vi "UHR-Fleezers Control (host) - 10.8MV_trial5.vi"() -> ()   [LabVIEW 2012]
uses:
  <vilib>/Utility/miscctls.llb/LVPoint32TypeDef.ctl
  <vilib>/Utility/miscctls.llb/LVMinMaxIncTypeDef.ctl
  <vilib>/userdefined/High Color/nirio_resource_hc.ctl
  <vilib>/Platform/TimedLoop/XDataNode/timing_clust.ctl
  <vilib>/Platform/TimedLoop/XDataNode/nitl_modes.ctl
  <vilib>/Platform/TimedLoop/XDataNode/wakeup.ctl
  <vilib>/FPGAPlugInAG/PCIe-7852R/niLvFpga_Open_PCIe-7852R.vi
  <vilib>/FPGAPlugInAG/PCIe-7852R/niLvFpga_Reset_PCIe-7852R.vi
  <vilib>/Utility/error.llb/Error Cluster From Error Code.vi
  <vilib>/rvi/errors/niLvFpgaAdjustHostInterfaceError.vi
  <vilib>/FPGAPlugInAG/PCIe-7852R/niLvFpga_Run_PCIe-7852R.vi
  <vilib>/Analysis/baseanly.llb/Mean (DBL).vi
  <vilib>/express/express analysis/Spectral/Block/exnSpectralBlock spectral measurements PSD poly.vi
  <vilib>/express/express analysis/Spectral/Block/exnSpectralBlock spectral measurements PSD WFM.vi
  <vilib>/Waveform/WDTOps.llb/WDT Append Waveforms DBL.vi
  <vilib>/FPGAPlugInAG/PCIe-7852R/niLvFpga_Abort_PCIe-7852R.vi
  <vilib>/FPGAPlugInAG/PCIe-7852R/niLvFpga_Close_PCIe-7852R.vi
  openfpgaref.8.6.ctl
  <vilib>/Platform/TimedLoop/XDataNode/XDataNode.xnode
  <vilib>/rvi/interface/nirviOpenFPGA/nirviOpenFPGA.xnode
  FPGA Bitfiles/UHR-FleezersInst_FPGATarget_UHR-FleezersCont_0F5B06C4.lvbitx
  UHR-Fleezers Control (fpga) - 10.3.vi
  <vilib>/rvi/interface/nirviMethod/nirviMethod.xnode
  <vilib>/rvi/interface/nirviReadWriteControl/nirviReadWriteControl.xnode
  <vilib>/express/express analysis/Spectral/XNode/ExpressSpectralMeasurementsBlockNode.xnode
  <vilib>/rvi/interface/nirviCloseFPGA/nirviCloseFPGA.xnode
  <vilib>/Analysis/NI_AALBase.lvlib
  <vilib>/Platform/TimedLoop/XDataNode/XDNodeRunTimeDep.lvlib
  <vilib>/vision/NI_Vision_Development_Module.lvlib
  NiFpgaLv.dll
  <vilib>/FPGAPlugInAG/PCIe-7852R/niLvFpga_ConfigureFifo_PCIe-7852R.vi
  <vilib>/rvi/errors/niLvFpgaMergeErrorWithErrorCode.vi
  <vilib>/FPGAPlugInAG/PCIe-7852R/niLvFpga_ReadFifo_PCIe-7852R.vi
panel:
  out "Location path":path=path "D:/UnifiedHighRes_VIs/Locations.txt"
  out "Location Matrix":string[][](array[string])=[["N.D.\r\n", "N.D.\r\n", "N.D.\r\n"], ["0.19233\r\n", "0.00156\r\n", "0.20615\r\n"], ["N.D.\r\n", "N.D.\r\n", "N.D.\r\n"], ["N.D.\r\n", "N.D.\r\n", "N.D.\r\n"]]
  in  "radius":i32=10 min=1 max=20
  in  "clear markers":bool
  in  "trap\nmarkers?":bool
  in  "Sample Channel Flow":bool
  in  "Pump 3 contents":string="Bottom: ADig beads" caption="contents"
  in  "Pump 1 contents":string="Top: DNA beads" caption="contents"
  in  "Scripts":T1(tab)
  in  "Take Stepping Data":bool
  in  "Got DNA bead":bool
  in  "Got ADig bead":bool
  in  "Cap 1 Flow ON":bool=TRUE
  in  "Move Cap. 1 (DNA Top)":bool
  in  "Cal/Data Acq. Spot":bool
  in  "Dump Beads":bool
  in  "Cap 1 T ON":bool=TRUE
  in  "Cap 1 Samp Flow ON":bool=TRUE
  in  "Offset 2 Set":dbl=2.0
  in  "Offset 1 Set":dbl=1.0
  in  "Cal @ (MHz)":dbl=20.0
  in  "W/ Offset 1":bool=TRUE
  in  "Offset 1 Start (MHz)":dbl=13.0
  in  "W/ Offset 2":bool
  in  "Offset 2 Start (MHz)":dbl=16.0
  in  "Pause at Closest Delta (s)":dbl
  in  "Move to Delta 2 (MHz)":dbl=41.0
  in  "Attempt Limit":dbl=30.0 caption="Limit"
  out "Attempts":dbl=1.0
  in  "Wait Before Save (s)":u32=1
  in  "Fish for Tether":bool
  in  "Closest Delta (MHz)":dbl=13.0 step=0.25
  in  "Stop F (pN)":dbl=10.0
  in  "Then...":string(combo)="2"
  in  "Move to Delta 1 (MHz)":dbl=15.0
  in  "Tether Alarm?":bool=TRUE
  out "Tether":bool
  in  "TA Cancel Save?":bool=TRUE
  in  "TA Green Off?":bool=TRUE
  in  "Raster Set Upon Tether":u32=1
  in  "Save at end (5, 6)":bool
  in  "N Steps":dbl=20.0
  in  "Step Size (nm)":dbl=0.34
  in  "Save ave factor":dbl=1.0
  in  "Dip Trap Delta 1 (MHz)":dbl=15.0
  in  "Move Trap Before?":bool
  in  "Save Data After?":bool
  in  "Green ON After?":bool
  in  "Dip Trap Delta 2 (MHz)":dbl=15.0
  in  "Move Trap After?":bool
  in  "Duration (s)":dbl=1.0
  in  "Dip for Protein":bool
  in  "APD to Watch":bool
  out "Duration (s)":dbl
  in  "Action":string(combo)="Yank"
  in  "Fl. Triggered...":bool
  in  "Fl. Delta Thresh. (kHz)":dbl=0.6
  out "Waiting":bool
  out "Fl. High":bool
  in  "N pts to average":u16=6
  in  "Yank Delay (s)":dbl=3.5
  in  "Yank to Delta Array (MHz)":dbl[](array[numeric])=[16.3, 15.85, 14.85]
  in  "N Array El":u8=3 min=1 step=1
  in  "Random Choice":bool=TRUE
  in  "Force Yank":bool
  in  "Force Reset":bool
  in  "Y change (mm)":dbl
  in  "Profile":bool
  out "Sigma/Mean 2":dbl=nan caption="Sigma/Mean" format="%#_2g"
  out "Rate sigma (Hz) 2":dbl caption="Sigma (Hz)" format="%0.2f"
  out "APD 2 Rate (Hz)":dbl format="%#_3p"
  out "Primary Video Display":T2(plugin-control)
  out "Waveform Graph":dbl[](graph) caption="APD Line Scan"
  in  "Inject Top":bool caption="Inject Pump 3"
  in  "Inject Bottom":bool caption="Inject Pump 1"
  out "Messages":string="7:59 AM\tUHR-Fleezers ready.\r"
  in  "APD Ave N":dbl=10.0
  out "Int. Time (s)":dbl=3.0
  in  "Stop All":bool=TRUE
  out "Sigma/Mean":dbl=nan format="%#_2g"
  out "Rate sigma (Hz)":dbl caption="Sigma (Hz)" format="%0.2f"
  in  "Tab Control 6":T3(tab)
  in  "APD 2 Offset":dbl
  in  "APD 1 Offset":dbl
  out "RMS (Ang)":dbl=nan format="%_2g"
  in  "Bead Sep. Int. Time (s)":dbl=5.0 caption="Int. Time (s)"
  in  "Below (kHz)":dbl=0.5
  in  "Above (kHz)":dbl=2.0
  in  "Adjust Scale\nto Mean":bool
  in  "Rescale on Mean":bool
  in  "Offset (nm)":dbl
  out "Mean":dbl=nan caption="Mean (V)" format="%#_3g"
  out "Force":waveform(dbl)[](graph)=[{"t0"=timestamp(12.90000000000001 s since 1904-01-01), "dt"=0.15, "Y"=[nan, nan], "attributes"=variant("NI_ChannelName"=variant(string "T1 X"))}, {"t0"=timestamp(12.90000000000001 s since 1904-01-01), "dt"=0.15, "Y"=[nan, nan], "attributes"=variant("NI_ChannelName"=variant(string "T2 X"))}]
  out "APD Chart":waveform(dbl)[](graph)=[{"t0"=timestamp(12.90000000000001 s since 1904-01-01), "dt"=0.02, "Y"=[0.0, 0.0, 0.0, 0.0, 0.0, 0.0, 0.0, 0.0, 0.0, 0.0, 0.0, 0.0, 0.0, 0.0, 0.0], "attributes"=variant("NI_ChannelName"=variant(string "APD 1"))}, {"t0"=timestamp(12.90000000000001 s since 1904-01-01), "dt"=0.02, "Y"=[0.0, 0.0, 0.0, 0.0, 0.0, 0.0, 0.0, 0.0, 0.0, 0.0, 0.0, 0.0, 0.0, 0.0, 0.0], "attributes"=variant("NI_ChannelName"=variant(string "APD 2"))}]
  in  "Calibration":u16(ring) items=["None", "Position", "Force"]
  out "T1 X":dbl=nan caption="T1 X (V)" format="%0.2f"
  out "T2 X":dbl=nan caption="T2 X (V)" format="%0.2f"
  out "Bead Separation":waveform(dbl)(graph)={"t0"=timestamp(12.90000000000001 s since 1904-01-01), "dt"=0.15, "Y"=[nan, nan], "attributes"=variant("NI_ChannelName"=variant(string "T1 X"))}
  in  "Amplitude (nm)":dbl=3.0
  out "Bead Mean (nm)":dbl=nan caption="Mean (nm)" format="%0.2f"
  out "Difference":dbl=nan caption="Difference (V)" format="%.2g"
  in  "Take Detection Laser\nImage":bool
  out "APD 2":T2(plugin-control) caption="APD 2 (Cy5)"
  in  "Flip Green Filter":bool
  in  "Set X Only":bool
  in  "Set Y Only":bool
  out "APD 1":T2(plugin-control) caption="APD 1 (Cy3)"
  out "Detection Laser Y":T2(plugin-control)
  out "Pointer Y (V)":dbl format="%_3g"
  out "Pointer X (V)":dbl format="%_3g"
  in  "Set Confocal Spot (X-Y)":bool
  out "Detection Laser X":T2(plugin-control)
  out "Saved APD":dbl[][](graph) caption="Most Recent Time Trace"
  out "Trap Delta Graph":dbl[](graph) caption="Most Recent Time Trace"
  out "Save APD Deriv":dbl[][](graph) caption="Most Recent Time Trace"
  out "Delta Fl. 1":dbl
  out "Delta Fl. 2":dbl
  out "All Signals":waveform(dbl)[](graph)=[{"t0"=timestamp(12.90000000000001 s since 1904-01-01), "dt"=0.02, "Y"=[0.0, 0.0, 0.0, 0.0, 0.0, 0.0, 0.0, 0.0, 0.0, 0.0, 0.0, 0.0, 0.0, 0.0, 0.0], "attributes"=variant("NI_ChannelName"=variant(string "APD 1"))}, {"t0"=timestamp(12.90000000000001 s since 1904-01-01), "dt"=0.02, "Y"=[0.0, 0.0, 0.0, 0.0, 0.0, 0.0, 0.0, 0.0, 0.0, 0.0, 0.0, 0.0, 0.0, 0.0, 0.0], "attributes"=variant("NI_ChannelName"=variant(string "APD 2"))}, {"t0"=timestamp(12.90000000000001 s since 1904-01-01), "dt"=0.15, "Y"=[nan, nan], "attributes"=variant("NI_ChannelName"=variant(string "T1 Y"))}, {"t0"=timestamp(12.90000000000001 s since 1904-01-01), "dt"=0.15, "Y"=[nan, nan], "attributes"=variant("NI_ChannelName"=variant(string "T1 X"))}, {"t0"=timestamp(12.90000000000001 s since 1904-01-01), "dt"=0.15, "Y"=[-0.0004235663930173644, -0.0004722739341410556], "attributes"=variant("NI_ChannelName"=variant(string "T1 Sum"))}, {"t0"=timestamp(12.90000000000001 s since 1904-01-01), "dt"=0.15, "Y"=[nan, nan], "attributes"=variant("NI_ChannelName"=variant(string "T2 Y"))}, {"t0"=timestamp(12.90000000000001 s since 1904-01-01), "dt"=0.15, "Y"=[nan, nan], "attributes"=variant("NI_ChannelName"=variant(string "T2 X"))}, {"t0"=timestamp(12.90000000000001 s since 1904-01-01), "dt"=0.15, "Y"=[-0.0005883053071687949, -0.0006281319620349712], "attributes"=variant("NI_ChannelName"=variant(string "T2 Sum"))}, {"t0"=timestamp(12.90000000000001 s since 1904-01-01), "dt"=0.15, "Y"=[nan, nan], "attributes"=variant("NI_ChannelName"=variant(string "T1 FB X"))}, {"t0"=timestamp(12.90000000000001 s since 1904-01-01), "dt"=0.15, "Y"=[-0.0004680013428144157, -0.0005167699209570592], "attributes"=variant("NI_ChannelName"=variant(string "T2 FB Sum"))}, {"t0"=timestamp(12.90000000000001 s since 1904-01-01), "dt"=0.15, "Y"=[nan, nan], "attributes"=variant("NI_ChannelName"=variant(string "T2 FB X"))}, {"t0"=timestamp(12.90000000000001 s since 1904-01-01), "dt"=0.15, "Y"=[-0.0006226691488387671, -0.0006504715109714008], "attributes"=variant("NI_ChannelName"=variant(string "T2 FB Sum"))}, {"t0"=timestamp(12.90000000000001 s since 1904-01-01), "dt"=0.15, "Y"=[-0.0007901852473525123, -0.0008601641895809732], "attributes"=variant("NI_ChannelName"=variant(string "PSD Y"))}, {"t0"=timestamp(12.90000000000001 s since 1904-01-01), "dt"=0.15, "Y"=[0.00031556138798181086, 0.0002525101474044007], "attributes"=variant("NI_ChannelName"=variant(string "PSD X"))}, {"t0"=timestamp(12.90000000000001 s since 1904-01-01), "dt"=0.15, "Y"=[-0.00019678334910122974, -0.0002453993346964931], "attributes"=variant("NI_ChannelName"=variant(string "PSD Sum"))}]
  in  "Signals to Plot":i32(listbox)
  out "Trap Disp. Freq. (Hz)":dbl=6.666666666666667 caption="Freq. (Hz)" format="%#_6p"
  out "Display Period (s)":dbl=0.15 caption="Period (s)" format="%#_6p"
  in  "Trap Disp. Downsample":dbl=10000.0 caption="Downsample" max=20000.0
  in  "APD Disp. Scale":dbl=0.1 caption="Scale (Divide,\nfor above plot only)"
  in  "APD Disp. Downsample":dbl=2.0 caption="Integrate" min=1.0 max=30.0 step=1.0
  out "APD Display Freq. (Hz)":dbl=50.0 caption="Freq. (Hz)"
  out "APD Display Period (s)":dbl=0.02 caption="Period (s)"
  out "FFT 1":cluster{"f0":dbl, "df":dbl, "magnitude":dbl[]}[](graph)=[{"f0"=0.0, "df"=16.666666666666668, "magnitude"=[-331.1367572010275, -79.05506245821404, -86.61411242440559, -88.4728176091699, -90.3181253945935, -94.12566333707997, -92.52740723119955, -94.92192587982518, -99.60936585245742, -96.87568627870715, -94.02570383337763, -83.8058550151726, -97.57441397235512, -101.59968530846606, -101.523049255742, -103.35038532190343, -101.58594091014982, -102.96098031851216, -91.39759462745924, -103.75019963279499, -104.45030075054324, -103.04245334279298, -104.0720279134107, -106.06482372394834, -103.69131867828104, -104.40395035115309, -105.96420043276396, -107.6735556337804, -106.673030006608, -107.34889066208132, -108.05626565233933, -106.25659018850432, -105.29934513380842, -105.43096056709592, -108.3728498841465, -106.0555440144992, -105.78001282181421, -107.48741857324953, -108.67624970548897, -105.39976667156175, -105.91413119232612, -109.4222808198164, -107.0898971593174, -107.91164191890915, -108.26032038855709, -107.58332347164534, -108.23559688234297, -108.01271040303237, -107.66511723652701, -106.51901583170391, -109.27249501469946, -108.55647681594805, -107.93499259231463, -107.05068166453935, -109.13641475410455, -109.29679733781423, -108.19360835527803, -109.57747591546632, -109.58364591011674, -110.47061433372711, -109.8144340420426, -108.79067462293897, -107.54887553357234, -107.99559866705923, -108.85023923652685, -109.68733225238618, -108.51101278437793, -108.51620475114115, -108.22212402200637, -104.63726950302143, -110.2989919678048, -107.61796444414897, -108.68882962798736, -104.79193983043893, -103.59504263746938, -93.64633660288543, -101.9191640501395, -105.73717393151816, -108.92572458793902, -107.43962662800902, -107.79595323081325, -107.0923101993207, -108.17603277205289, -107.87074270713183, -109.20899066381877, -108.61832060412445, -109.10072003106593, -105.76480632823524, -108.60877649218978, -109.67541158970121, -110.2286232768028, -109.84952155309578, -109.33772024076384, -109.95251642394683, -110.14777282585466, -109.13825677905699, -110.05989365698167, -109.39359990189426, -110.56255614635295, -109.66477183197163, -108.9397158528824, -110.26529907650465, -109.20049464984628, -108.20183857013548, -109.09752250184418, -108.00440442238454, -108.35465963524055, -111.16774134451799, -110.34812550238405, -108.94506763426756, -108.72845542102493, -109.41512344014713, -112.44661664432377, -110.35437330889101, -111.32939440655925, -109.42989530434981, -110.98084669076195, -111.92160561143541, -108.57755551751093, -111.40042616180912, -110.15284955891853, -112.21455132279115, -111.40787773511747, -108.82949641635288, -110.13442122547907, -111.42229298204664, -112.06314940885191, -110.6015308813694, -109.51144097251623, -111.15989713761475, -110.25535755335385, -109.65868178057926, -110.51649885452997, -109.77194745285269, -108.4234206864394, -109.50892632093968, -109.46471287444389, -107.92241289271415, -109.72283805386196, -108.63426821579918, -110.37316681536255, -111.09713996884652, -110.32903619589223, -105.32012665515045, -107.36858557554393, -108.00382215905725, -110.06430686942338, -108.81666625979916, -110.01277074453823, -110.94194741225512, -109.65934609082873, -107.80979136006962, -112.81333866824724, -111.61474300955487, -109.83998277184975, -109.45953946904639, -109.79640584952526, -108.19172301667324, -109.28894656674316, -107.61471301278785, -108.83814006090513, -109.08866847726084, -108.20250571862371, -107.96222236861584, -107.03811197900873, -108.93533000393974, -107.74482548035408, -110.79811544577694, -111.1387476496877, -107.42970105883512, -109.18442281176472, -108.73546184641192, -108.71800246690864, -108.51945944378063, -108.06825856571285, -107.27210712368412, -108.12304695877637, -107.84933283677306, -109.73682373154998, -109.32284761503395, -109.31328817453769, -106.68762108642842, -109.79203616876461, -109.9020278896408, -110.27080024357275, -108.54152101558762, -111.00464391726017, -112.42244020766577, -110.82707315747889, -111.00344011890857, -109.90461839395674, -109.42877207451863, -109.73549298167016, -111.67494793393293, -108.85799077901427, -108.5348443278263, -109.803781083881, -108.30644755543659, -108.5079527456017, -111.2055351312823, -108.53089994340155, -108.01739789012176, -108.70360662855235, -107.95873456794631, -109.58297170693093, -108.9372401694271, -110.15921663527153, -109.22399119911955, -110.89883651739237, -108.92840112258382, -110.0545300523626, -109.05961065387005, -109.45831398589371, -108.61239387653227, -110.13001256174265, -108.80060224137931, -109.46327400696283, -108.0177965824709, -109.29727944627197, -110.3237255895986, -109.03258262543821, -110.97880178489321, -109.70034895077919, -111.16405638194153, -109.17324451464711, -109.65698250854277, -108.96750235822178, -112.00534231585624, -108.69274607723942, -108.98110446396657, -108.40723795464795, -111.44459094807324, -111.74799245277113, -111.1601960491512, -108.92048232753773, -110.30506377784799, -111.33145973979093, -110.91850998672503, -110.33684985776448, -108.90206518366908, -109.28458878227542, -108.98773986023751, -110.85813863075646, -109.00041591105906, -110.84543686681204, -109.84382395806176, -109.69722434763266, -108.50915601095721, -107.80829925826895, -110.59736107582401, -109.75377770317087, -109.3992084496136, -110.51151565846742, -112.49753959826434, -109.7299632589479, -109.54070743868353, -109.90314341132164, -111.05974202976806, -109.03766862152392, -109.46667095459878, -109.52800799036197, -111.3163121356807, -110.07817134522178, -108.69251657453547, -109.40472158898045, -109.71400709815576, -110.60534468715097, -109.46937396724682, -107.70342491418788, -109.86331122597839, -108.64971387994616, -110.90117371097081, -108.34928840565928, -110.04172889660904, -111.52979926554961, -110.34759300823305, -109.62712781837159, -109.24131154553284, -110.23196152450447, -108.68509612326807, -108.0246905483419, -106.61876139289784, -101.5519630114271, -80.57695480953835, -102.03744443354402, -107.1449217193017, -110.0695213407169, -106.61597783999268, -110.79221011808191, -109.58974545931426, -109.1149802216988, -109.20993813088597, -109.63768480465863, -110.10428394219181, -109.08445084271477, -108.83472375362581, -109.69508502050168, -108.05588796178941, -110.62586360101581, -109.95315261676905, -107.52208264977473, -108.80708007514875, -110.43484881098874, -110.45942171588936, -107.83804717866751, -109.98973910294193, -109.3496496054193, -108.425252911127, -110.94579264380809, -108.54181722177951, -108.67696070083541, -108.4150202151644, -109.24973583101504, -112.0454922608961, -111.29046597340738, -110.75018248960077, -109.38326363603683, -109.2033340336957, -109.45076170874889, -109.52878049853727, -109.32340869724774, -110.98123395128233, -110.75736340635505, -109.7218385823809, -107.97422606064993, -109.77313701758703, -110.95948744392717, -110.08996774172691, -108.51011830110778, -109.78063140243836, -110.65996628628228, -109.83684298615616, -110.33329049188029, -110.13755118968292, -110.3717925645783, -108.55302219178951, -106.86811628734195, -108.6302156589162, -108.75341391045045, -108.32589578384841, -108.70061474734084, -112.30742263527534, -109.16842570592085, -109.29767035534508, -108.87829025017463, -108.2255616391397, -108.4316108616088, -108.82995906929271, -110.40135575415563, -109.51623498946435, -109.79409808792403, -107.03832759632121, -108.36534528684132, -109.72010868372905, -107.90933028179892, -106.95643597294047, -111.29929166165778, -110.23001135794706, -108.98838015381585, -109.79115357104436, -108.18627479511115, -108.14988122174307, -109.12074063466532, -109.41904850488358, -111.40409873721113, -108.83156790193294, -108.77032248953847, -108.88363158686694, -108.47515048290681, -105.94172147874599, -109.38146940214403, -109.21277078848794, -108.11309390545507, -110.70840012427504, -109.5504457849329, -109.52330684534209, -110.06776026911132, -108.21949434182314, -111.21266686269992, -108.78581501170974, -108.43115799297222, -109.63260325780062, -109.84070220619535, -109.72041980780126, -110.29615941882527, -110.60316734262464, -108.79165446414692, -110.95840439895592, -109.64926233107009, -109.16526769544322, -108.65292362430982, -109.56113898129935, -109.85693046339026, -108.92316027325207, -109.79492493553914, -109.38157962945887, -110.24545136266825, -109.30031463492487, -109.0795429936869, -111.4091719525013, -108.63499083917162, -108.43863465339358, -109.23207864880891, -111.21947487191643, -109.24525201480154, -109.56842406077318, -109.46711940800672, -111.91389548262572, -108.15655736690546, -108.71882059966947, -111.26328503478568, -110.95027143873176, -108.4853106242357, -110.36902802777546, -109.9314203579182, -108.77686164101732, -108.71871020068312, -111.04829661168574, -109.95072655339462, -109.88221342875462, -109.53241732756136, -108.2625005404823, -108.00677030040697, -110.19659317581693, -108.93858924796267, -109.46817875483995, -110.78063992017232, -111.11066570318451, -110.78774336696706, -109.19199744617812, -108.54914256407436, -109.28414960420909, -110.64143585101183, -110.5855350821307, -109.47578632252726, -108.89705360836223, -109.89214013612292, -107.93271261027171, -109.32631601340563, -108.60274611341092, -109.40110159872573, -110.889237682208, -110.01391165813328, -109.99747108785071, -108.65542819213674, -110.37211847668736, -110.44656500845738, -110.8128133834973, -108.8909299260433, -110.19551227077532, -111.37647266643523, -110.83802189730321, -109.98519377913681, -110.52378970770522, -108.16970420057817, -110.70974729773344, -110.76836765494402, -110.26884275594577, -109.22041044268806, -109.87809744746195, -107.76823252107832, -109.12119474042969, -110.28066108731146, -108.55000033509207, -110.18152097767907, -110.73030521152278, -111.49470908029893, -110.2320929919509, -110.03370979233021, -109.79181668155233, -108.6673501209991, -109.86695766650877, -107.88926518046961, -110.95525003776572, -109.18130359755742, -110.42618009658618, -107.90341931158893, -111.44736855661769, -110.72634267386593, -109.29945988519303, -107.67889101961411, -108.81148059987765, -109.13375212757057, -109.8122873383549, -109.80176697684155, -109.96342275204768, -109.90406635707086, -108.75674342748256, -110.12362902701081, -109.82151095527837, -108.62543344241836, -110.09171852771195, -110.21434637862887, -109.97254504855631, -109.27043209093468, -111.35149588204125, -110.12399876776051, -111.65983675538546, -109.28788875768564, -110.86554069990251, -111.26990906470603, -108.60956517491746, -111.49613890850938, -111.79685722966795, -109.26269485364045, -110.38555615546439, -109.40641023162068, -110.966136593156, -108.78892524584494, -110.29340727375603, -111.44032043281035, -109.95212021173755, -109.79233511584334, -112.41184021118175, -109.73687851881148, -108.65493879781806, -110.76132988919045, -108.43230346094671, -110.32968175895853, -110.29890782023821, -108.77609076424456, -110.3298662333555, -109.47734504217333, -108.2677295732245, -109.21234363352882, -107.83278941978479, -108.85136784424789, -108.43241251530755, -109.76609391460555, -108.53204373005357, -110.9660641972934, -110.3152512161094, -110.72570499399905, -109.23877906286317, -111.72407743101837, -109.20311421918561, -108.06021800233717, -109.29288625761943, -108.78395253409145, -111.85250172876302, -108.78827588901797, -109.79775055719482, -109.12089297455859, -109.49896359356035, -110.34432647103819, -107.94700097960238, -109.30489238477631, -108.89170290869342, -108.82574563272509, -110.11024077194833, -107.37946433552314, -109.60167933458756, -107.80625057819019, -110.11489057210264, -107.35436859378505, -105.69819484613895, -109.11280625683739, -109.27770293057978, -107.7053735252589, -109.75022444894368, -109.3310543596577, -107.87683693707739, -108.19931495338068, -109.26462246191564, -106.71885779297867, -100.00018022217961, -92.54434511397295, -107.20472143807373, -107.39203415155283, -110.04461177268398, -108.48860496315312, -109.0057168110333, -108.37627790492552, -108.4108380728248, -109.65509454313073, -109.64243000632982, -97.04219069306761, -109.0928856629964, -107.9760697315632, -107.52611064047497, -108.87702814778996, -109.08437599027614, -110.70097118837974, -109.00969860961283, -110.38275386163214, -110.0699155421545, -106.91498895181175, -106.22178738309017, -109.36827866896039, -107.59953130968307, -109.19516217272808, -108.31502495393616, -109.384158926223, -107.11670654202719, -108.09436312738853, -110.14559230873704, -109.84997663447679, -107.83465335309926, -108.60947100624459, -108.9932479423645, -109.17174810371898, -108.79457339828916, -109.40909327982367, -109.6328723628302, -109.51081854476179, -107.63054408568418, -109.63728404010122, -108.51163794839918, -107.55002282725216, -108.97796212764939, -107.24648164623483, -112.21470452291085, -108.74294024554423, -109.62070777514892, -108.05768666239368, -109.8224946685739, -109.34575507446003, -108.53536952609525, -109.60789300457671, -107.56681538208278, -109.22777325016398, -108.79047910308894, -110.10332477250668, -108.00206387955672, -108.45604004720035, -109.00645795765472, -109.81039564269616, -108.92785144634745, -108.3978471520567, -107.94411095685999, -110.53486519304262, -108.8773780319227, -109.03345093296107, -107.30746693745031, -108.54277704832029, -108.77629108166091, -108.91111762599647, -107.74965195880401, -109.97375370738439, -109.76326492689246, -107.91717581777407, -109.0730556927617, -107.66804873204664, -110.40438871064791, -108.05794247751498, -108.80206615156494, -107.51329354700796, -108.83687012994949, -107.57713176895379, -107.94774159581414, -109.41894615439651, -107.10869425078764, -110.51480854078629, -108.92221367099775, -109.91358786461535, -110.1744263092835, -109.30795472883494, -107.91359710691006, -109.77888185049835, -109.52060975706438, -108.66686651982212, -108.71041801553639, -110.13619546359467, -108.87957097273856, -109.72150387215271, -109.00776068810654, -109.70251113927438, -110.75769213896399, -108.53234896741436, -109.69439526582246, -110.15412541604617, -108.25183374628219, -107.97402569656481, -110.34920156998648, -108.45106995186384, -108.82031145748209, -111.38690005057539, -107.01968459818563, -110.3044500039584, -110.8755481852125, -111.08915057663255, -107.94824988655199, -110.21669144934839, -109.90539774633154, -109.58985438756767, -110.12258796623348, -109.41689951612143, -109.31128210476795, -109.00258476567323, -109.11093063041056, -108.83347064311234, -108.32685287566952, -109.44770946560935, -108.40145063144861, -109.68448193892085, -108.76525439243828, -107.62837139034596, -107.39300298848994, -109.36993934990318, -109.2465218489418, -106.66307369796812, -110.15891092764934, -109.57151745419041, -108.92425698310808, -109.8036704717834, -108.79751146756549, -109.25926431818017, -108.46260574057584, -109.1967554647261, -110.63319560262356, -109.02343067385144, -111.22073171487528, -109.4731095097105, -109.69335000085164, -109.48782989577005, -107.95204227683271, -108.19468255763758, -111.36195112053247, -109.55696116543685, -110.3130767640534, -108.9621824253354, -109.99735074896789, -109.20198058456344, -108.12100614259485, -111.27227490807289, -110.09248554008288, -109.14395535060149, -110.80882692379708, -109.22632926901655, -108.64497210802793, -111.00030482190711, -111.1317849358033, -107.43140429257826, -107.9783302193555, -109.2639893652291, -108.97008485446163, -108.66556668859064, -108.12995785876932, -109.73001061107855, -108.09691302413727, -110.68391499215569, -112.78583642012705, -108.7093037763389, -110.67868795924797, -109.0190959349128, -108.36247198231372, -109.82829353258869, -108.24916379311045, -109.84154533905823, -108.55470160833775, -109.75438989348815, -108.82865632118325, -107.63622268162582, -111.00943492886312, -110.81824358463759, -109.46028423652966, -107.52479398900992, -108.99087806823736, -109.94494831750349, -110.26788355564504, -109.8954055022304, -106.9478122391182, -108.91705388158901, -107.76095584490312, -109.28456723055147, -109.7982307261767, -108.98552661346622, -109.98937979783426, -110.57907422426224, -108.68113463944836, -108.06257240208589, -110.0707224529617, -109.19515280354733, -109.35868842818849, -110.37311467065695, -109.0404734478992, -108.16686395270187, -108.61859220485148, -109.19986437876149, -108.19707189725302, -110.06564239663074, -108.87850403465154, -110.63824157544798, -107.36918104067212, -108.7008736325543, -110.9359398265406, -111.08529123080929, -108.44209934821818, -109.79529621208783, -108.38917887958179, -108.169117639508, -109.24332926356216, -110.50584058811704, -109.63592524002665, -109.32261039377495, -109.16720880524552, -109.3084314664462, -109.5812223978583, -107.70213196487856, -108.0557884982431, -110.67058020007828, -111.68459781023608, -109.66270627185824, -110.52536245663693, -109.70208409132103, -108.78645420809342, -109.23122088059863, -109.24601474121832, -111.25604763816514, -109.50225851581177, -107.32434217163818, -109.28548556764925, -107.59972621660836, -110.46928774723048, -109.25950101547609, -110.32016453935465, -107.78482761561703, -107.89462895091089, -107.51366154391481, -108.08036891159172, -109.53371809947035, -101.2452927166745, -109.32763325689056, -107.52166868423687, -109.89648659445174, -109.11350200980485, -109.81336712738089, -110.02799517445062, -108.02767143538516, -107.97850220501483, -109.50772934896838, -109.31069875721964, -108.49991657749598, -105.60880911233095, -109.79128597340213, -106.91084537903113, -107.84880087118997, -109.63628170511824, -109.03203967193224, -110.64186113413658, -110.98027990365594, -112.33841002907062, -111.01793075565425, -108.58025797022215, -110.4259296883756, -110.38643255981424, -108.93051671115133, -110.97544177116494, -108.63883100482677, -108.37581711765226, -108.90240163126536, -107.94688047875466, -109.9482937437732, -110.09097112364414, -110.09805032265376, -111.44307114024532, -109.15483789122554, -110.9713708217832, -107.8548737634672, -111.41418477109195, -109.45699779859628, -97.03595099331734, -109.16746744169623, -109.66209204485918, -112.57048704774604, -109.73989735035725, -108.16252575067017, -110.7546980664636, -108.91536673403449, -109.20509151422344, -111.0260632167785, -109.62924582406518, -110.45466277291722, -110.2973970018937, -109.67550222925419, -108.84481022020094, -107.23686414357573, -111.79004633370906, -109.85453094194085, -109.45617270081004, -110.73920606732504, -108.90879956851099, -109.67774425528265, -109.4745715721361, -110.18080454693559, -109.26079184315502, -109.41692499885505, -109.02240975088358, -107.80833423058168, -109.32657361431549, -107.87138278655101, -110.910364670719, -109.70067156846706, -108.55301754282077, -109.4243252157005, -109.77567725161107, -107.83737232063925, -110.36509412773016, -109.6371048811367, -109.49430894422814, -108.55509251499753, -108.03996302911446, -110.4385715838736, -110.08864436068788, -109.48922484379962, -109.90865554258562, -109.7491963238264, -110.04796094537969, -107.413043439116, -108.54229076126079, -108.2522516728666, -109.75464941327974, -110.26795832300996, -109.28073673851144, -108.62990200974927, -109.89408067552287, -109.09160284731726, -109.90740624925795, -109.92534708896517, -109.79578862362752, -109.97278346890566, -107.80679350393824, -112.81728446281548, -108.09689504419987, -109.89549991422173, -108.43930976031248, -109.95153099843282, -108.18277483720716, -111.89607792605433, -109.52567003805, -109.17125106979698, -109.64300739407085, -108.21045178846524, -109.64036472149706, -109.02324448538845, -109.039163008889, -110.41006510134076, -109.50289952116489, -110.4732620447796, -110.08777181504614, -110.15589511434341, -109.55705089158471, -109.2547682932589, -110.86823885471617, -109.96330502176939, -109.85995369810554, -110.63211290903473, -112.08007783432191, -110.24725218052279, -107.62861148917592, -110.08691795849435, -108.89793794632287, -111.07702220466341, -109.46946126482341, -109.19747345337464, -110.70018609416007, -109.66366205691908, -110.78032312133551, -108.05724200456513, -108.195661625627, -110.90724508408255, -110.08307674771669, -110.76863516643007, -110.46620425061583, -109.16986788877276, -109.61921294239114, -108.51159432329543, -109.96308336765689, -107.38178944242856, -111.95930944846394, -109.3329826827624, -109.59119636368249, -108.83148571828912, -110.46194288788257, -105.87694286145472, -107.985886302892, -109.2975019660806, -111.05138725716857, -109.60005889204612, -110.92871351729086, -110.73480546964537, -108.41587420326718, -109.84275465824477, -108.8249071047676, -107.65358887817105, -108.3254150042995, -111.47362100321767, -112.7287536850025, -108.8217125660507, -109.50232320231771, -110.29587061625348, -109.30644535112089, -107.69178032077258, -110.84522325672016, -109.3735891463141, -109.12506388923123, -109.65582307934665, -111.11427272192576, -112.19827973435466, -109.11306367925813, -108.19203577968261, -107.89831568266465, -108.85805249169313, -109.51100049661844, -111.71546684086955, -109.53880495724334, -107.07739286222231, -110.66836728754211, -111.5415170557177, -110.16051267940297, -110.6107546662698, -111.36389129556191, -107.77888179117923, -110.34160392509817, -109.61287125994414, -110.23791773883013, -111.00669159903549, -110.97165069538953, -109.43965413392434, -110.6813161690388, -110.31441293654314, -111.96129906273796, -108.15998218707462, -110.08095912053633, -109.41084567452768, -109.28774416263552, -110.80159950384204, -110.41956747809755, -108.85005186267244, -107.9069227847757, -108.84249369063123, -109.92569208845894, -109.34109797584448, -109.41334788055491, -108.76462023086997, -108.22069272136177, -107.0786679601274, -108.30206755098202, -108.57613406368954, -110.83330887636482, -111.93966942736989, -109.76373713473264, -108.25782074884941, -108.16490627215555, -109.93351470267982, -110.75525684428368, -108.22814762283093, -109.73442331991602, -107.53145627482685, -108.27195221226805, -110.33032779278457, -109.48951857415828, -108.12599093700939, -107.97627415508097, -108.81426859968796, -111.21764717894752, -109.80856212352333, -110.92658779118501, -109.71551885834796, -110.38682741010847, -108.87671328341361, -109.68368600774755, -108.35359806351899, -111.7519400010676, -109.89407081573103, -108.24301180922755, -110.00646944788126, -108.6685299083706, -107.52856885980722, -111.7622363038509, -111.0025144494897, -108.64719599357296, -110.62968467177518, -108.821509935539, -107.94915453463719, -111.53070432277694, -109.87282048586256, -110.71167589371663, -109.79225006081626, -109.96203471712074, -110.29921092232489, -110.10644439440416, -111.28815007382043, -111.19165661703703, -108.46024117100558, -110.22528296512183, -110.32184972386672, -110.05120383416072, -109.78792549362107, -109.00355659956696, -108.85989369286315, -113.00899556732638, -110.91756826567867, -111.25016866167897, -111.84225040552181, -110.54451635944174, -110.72722829912917, -109.60759702177283, -110.49362602516815, -108.74419542915284, -110.3379671069179, -109.66259088220754, -110.45956400953156, -109.13956157147233, -109.27130155486806, -110.83015602667983, -109.17970724944131, -109.09662765889193, -108.0447366108107, -108.9536269357457, -110.35663108940085, -108.73418835472056, -113.42965806805827, -111.81270536656905, -110.06155590173537, -108.76582224646269, -106.7488061675813, -108.5700320158723, -111.11038264410035, -110.41435767488723, -109.12763443489911, -109.30517580756394, -111.61251165371237, -109.8116632664339, -109.36845864976851, -109.00390009629231, -110.54359197165573, -109.52629258465976, -110.75932197632896, -109.50903215359567, -107.42652056246085, -107.81146496533543, -103.22224383145215, -108.53803076819163, -109.78623360072066, -109.66306634612869, -110.80245829141279, -111.87835085452016, -102.27372781471168, -111.27763038431458, -108.45838423437681, -108.79077917058028, -109.31951755762685, -110.05415097017186, -109.5535934823387, -111.62732254641111, -110.73478247119641, -109.9468722686683, -110.39698367573979, -109.30612942398305, -109.7578384694043, -109.34817295524313, -105.56944757301993, -110.1940418750125, -109.27076023513962, -111.03491935225027, -112.2980497521063, -110.65725497955563, -109.0567530102422, -110.31700596563523, -109.64508026365678, -109.6190471404421, -110.52566833759428, -109.68595899227789, -109.7431160985074, -110.4798230300751, -109.45506977604765, -110.69504157940786, -110.63067849573177, -108.06456949500138, -107.99354148885966, -108.11349194720599, -109.15944121207349, -110.61766925164031, -110.14145801314527, -110.67420842201165, -111.91532881806512, -112.15901550030345, -109.94774413630104, -109.2819568305201, -110.94623189179737, -110.17685430287735, -110.39082916961016, -109.53953238698966, -110.76940623620611, -109.89327922318515, -109.10275695043765, -110.21445972656734, -110.58968777252528, -110.57016757660259, -109.59208496373341, -109.07946946465374, -109.10762003745964, -110.36892993974607, -109.81864495218393, -112.12972189864566, -109.26185849434863, -111.56305819991357, -111.36019621828058, -110.3397604159226, -109.58675612753163, -110.58041217474447, -106.34739062044932, -108.6722699609389, -110.03906060709869, -109.16794717548382, -109.65012481802809, -109.35377624077988, -110.51889143862303, -110.03397458059777, -110.7981307056636, -110.56653507062292, -107.61367005067231, -109.99279736988825, -111.79875182878175, -108.60382315996031, -109.71381533228038, -108.60388131505613, -107.0933685540362, -107.86037690830757, -108.40980028847238, -108.83869602763895, -110.76921375395764, -109.96766364716046, -110.8256171465781, -110.13805084291067, -108.5349140035878, -110.57158437465219, -110.8920694413417, -108.71646695477324, -108.33274238445665, -108.96152108305608, -111.03750932994224, -109.48915027983756, -110.29725207211165, -110.79527247268442, -109.47969936716117, -109.79306701834035, -110.16840035577498, -110.29840230783668, -109.15306387075587, -110.72651274964761, -109.08881658764956, -110.8349724030761, -110.64653625576447, -111.40392562616867, -109.94581588927414, -108.85136340231294, -109.77228546607624, -111.48297395390018, -109.7334001251941, -109.30537415590783, -109.63937411233408, -109.69785848648013, -109.3523781030017, -112.04667421182404, -111.56311816195343, -108.18548447362308, -110.63388993686104, -111.39768634137992, -109.87157345395542, -108.6734208287271, -109.46213300216168, -111.75774769437145, -110.10245994173216, -109.52385139033495, -110.96513097775451, -111.8709319163154, -111.54948269614047, -110.29760900080463, -108.52168175904663, -111.09033925738258, -111.14752744054172, -108.83074523709202, -109.05704141259113, -111.74377805749482, -109.57200906899736, -108.84121318623825, -110.86657990204343, -109.54363603755047, -110.89448416316372, -109.58965570570145, -110.21012263847972, -110.4063470702923, -109.5021950342969, -110.33648801598177, -110.90551031296536, -109.69205870504638, -109.8648503154861, -110.28183391384131, -109.65970942950766, -108.43615680946908, -111.11790511866548, -110.89043476451553, -113.64898442872548, -113.08004494963895, -110.81525412051718, -113.91009875719509, -110.95802128672312, -110.40944585634135, -110.33464695414992, -109.98984645778987, -110.18795067005652, -110.62364351231234, -110.44029833291248, -109.01598585569788, -110.95430216511514, -109.77987141110621, -108.54452361812068, -111.41780266439777, -110.47172771858405, -109.06084635984516, -109.30794593246578, -108.8764083815745, -108.18222749506985, -110.31330487887435, -109.04176821738014, -108.8558386035048, -109.47888284507395, -110.01459604573937, -110.48596659065309, -112.6781342298378, -109.85522803775775, -109.0569534499285, -109.08991286548698, -110.89485727880403, -109.18715778948663, -111.50381433568144, -111.3545424730884, -110.07710926239977, -111.99977850157067, -109.47444853853723, -109.81605328527645, -110.74995213151195, -112.56834665925544, -108.52052472391404, -110.89121213995557, -112.02004142355113, -108.66413739656008, -111.10053848695652, -110.41241079991636, -111.80152991764473, -110.21746151515111, -110.63265128607344, -109.483042128511, -112.78639954059729, -109.47114195846122, -109.23309637902875, -108.97133643967169, -110.08909147812822, -111.01105271457081, -111.18602432128249, -110.04633990216801, -109.53453538673071, -108.81939452082017, -111.13486114285661, -111.65877073200598, -111.63763706753498, -112.14107810664572, -113.6231865196724, -109.31743865878806, -109.18551713085722, -108.74951309653638, -109.28206426212142, -112.36687029711229, -110.10933061193728, -111.29501093502684, -108.19021080564794, -109.34497312126749, -110.37228033937312, -108.63277512903049, -110.61033993911002, -111.2975761598062, -111.49780004751436, -109.91019436685814, -109.32789992989028, -111.4482538110117, -110.1538439123475, -110.66347034043578, -110.05055133068794, -108.53002033538341, -111.7522199783972, -113.49108651193104, -108.03793940563418, -110.07108694011555, -110.83958739865201, -109.62805629409038, -112.69637731014087, -109.57996950503268, -110.104850643722, -108.83376203949506, -108.69400304840181, -110.59434352922563, -110.69121011800921, -110.18694553784364, -111.90598571547098, -110.30230802494223, -109.66810649416752, -112.6017099000434, -111.00296745333219, -110.64462650261785, -111.4775358707403, -111.98753241268494, -112.26574909791167, -112.04796822399412, -110.65853064447325, -109.6623218025264, -109.40559579075378, -110.42174451813142, -109.18991987957241, -111.02050178263048, -112.77950487440032, -110.42443751566815, -111.35440372400903, -108.5263524245987, -105.07498063939795, -107.15444425741984, -110.4508720018025, -110.25163264819463, -111.1383261104107, -109.91171620173931, -110.52200560606038, -110.5299174299573, -109.34628087255733, -110.26101817411786, -109.65071853372183, -109.66953335961068, -110.83590602054682, -110.980546313788, -109.4110066989163, -111.47223607390256, -110.00281523859483, -109.4088722967626, -109.00401922839337, -109.59655302543185, -109.7359970854586, -111.46016206343049, -110.23478747568004, -109.29441275295858, -109.82941912510167, -110.43088525283673, -108.21649744751299, -108.70220592702613, -105.2334473604296, -110.60620657984927, -107.97533820921146, -110.7664079806058, -110.56406610911355, -111.76465470250328, -108.84172809688911, -111.03661078143631, -109.85351980370237, -110.70091167176791, -109.52380717508088, -108.4356492672842, -112.25498760397127, -110.69648730540193, -110.36748838594507, -109.99090797924349, -111.2678642544111, -110.42541694325627, -111.4575545259775, -109.3211175669008, -112.7465573314208, -109.56208667784249, -111.59733497772172, -109.42295730962105, -108.55804089331346, -108.71397903286748, -110.09188290952392, -108.90810063278326, -110.31333217069538, -109.69794714542728, -109.06210020835357, -112.42465112160288, -111.74630553904855, -109.99304310093493, -108.93867687355595, -113.1669287525049, -109.09193568851137, -109.27500368450697, -108.99643325722404, -110.53962759110647, -111.2052088429852, -110.05855563908841, -110.30763723153481, -110.03411001268613, -109.6161415052669, -110.6304714466923, -110.17116005754627, -109.0753171640551, -110.92564270851628, -109.60831770517053, -110.25913363817017, -107.76644895378317, -109.2619309023068, -107.64198246311884, -107.37056168314048, -107.31978563121643, -107.68171928702894, -104.57515288104209, -104.75187637758803, -105.27246893266054, -106.96524396060869, -105.93920355631757, -103.66449995825586, -104.08476660009461, -104.53081578265315, -103.0148493379086, -106.74751670818362, -104.92309629919443, -103.98320340724693, -104.81633219413234, -105.77996356028235, -107.12559309216644, -107.28196039053535, -108.84583578337953, -109.4494696919565, -109.15525441177898, -109.7634811359225, -110.79433338587495, -108.44440079452527, -108.79597700117748, -109.98590735173822, -110.72144284267539, -109.30550753718086, -109.70072152916897, -109.65801130162137, -109.65949265997646, -109.82238573025273, -110.30669821947491, -109.83394128869384, -108.90433312205332, -110.664046708231, -110.39926453734134, -110.37725911098757, -112.12508639032839, -110.26795666332589, -108.98741993218054, -107.76168841100478, -109.82334992872889, -110.83516363498563, -112.60649745671253, -111.1960726449926, -111.03919163866381, -112.05129034965563, -108.83187987662883, -109.57240688505179, -109.32857861150738, -109.54934849013647, -108.29359879300195, -111.5179112931669, -109.52702486426027, -109.95429980789645, -110.7011078611564, -109.43204524997455, -105.56031249677113, -107.70609254346495, -108.78303653454363, -108.11457060956113, -110.44215460317537, -110.78267897406572, -110.33119812901934, -109.34449539666907, -108.82636558484161, -107.1834151347969, -108.83808254322192, -108.2542825327446, -108.80298057862501, -107.59922121598055, -108.9131916496929, -109.51519107961856, -107.7704986323755, -108.79678029009878, -111.13791068210752, -110.402746275919, -111.31702623823912, -108.49812727557243, -110.63723264798182, -109.32890666586829, -110.29721723278237, -111.66560929315017, -111.04227698307153, -111.36927505376269, -112.5203298417673, -109.93967930487354, -110.14533835678606, -110.3868348991775, -110.85413569165249, -108.44519725537315, -107.93391978795047, -109.82778679299085, -109.79311153223738, -109.25261055399044, -111.47738679135526, -111.11775495397512, -108.65898844492045, -110.26505495390529, -111.02017977446526, -110.34817965403467, -107.55161094495372, -110.21667403085983, -112.43970497917284, -110.70535338255132, -110.79438078890512, -109.81809822502822, -108.99167960596515, -106.5556893069368, -97.51736665041192, -105.29926513345109, -108.72453297392224, -108.23203912463346, -109.50324111400698, -110.9939986929772, -108.05367524487318, -108.37339392211176, -109.8553291283933, -110.46179639493138, -112.48795697163695, -111.88145079973545, -110.8678969738583, -110.62677605624849, -111.83824818603244, -109.76798658735359, -109.6654742351465, -112.58543522753767, -110.3406716250781, -109.55013159400883, -108.00481229232405, -109.90793236599207, -111.28597960985334, -110.54144527494444, -110.14704702870655, -111.2652554338908, -110.97520848958668, -108.63647576273343, -110.52472680617548, -113.16137826273847, -109.62457037485827, -109.53869420402964, -110.71399284283449, -108.55435337782664, -108.09492728294455, -112.2373886856363, -110.3693019226993, -111.65116752865308, -111.3223986412311, -109.67734725401074, -111.36420709226297, -109.14293108556625, -110.5982939020188, -110.29596476096043, -112.69847120697035, -108.39052787054206, -109.06205229490357, -110.00045399262885, -110.71775009467346, -110.69530760167493, -112.54144940754935, -109.55755373438097, -107.88943697845929, -109.98578587243783, -110.14202980613851, -110.80051915904802, -109.11327182471621, -109.50637030500913, -109.77023677605327, -109.98552825925917, -110.40235854896, -109.37603004890141, -111.36989177909379, -110.8399811877331, -109.30394670937987, -112.2769814990538, -109.10893172594731, -109.17733972841754, -108.35968166480572, -112.64492569586005, -110.13779257328873, -110.64439690778532, -108.45446935516622, -108.97325006911116, -110.54637968933774, -110.66412364132371, -111.38627695224784, -109.8942998516069, -110.36392017322382, -109.92355133054227, -109.61886697310419, -109.71969465343778, -109.85627196259388, -112.1407808286419, -111.1013489416651, -110.70428953307596, -109.3454280179969, -110.22984684615578, -109.53826801613613, -107.83673208330934, -108.72742563398342, -109.5745872123195, -108.83031823548816, -110.89059911076627, -109.87842545384129, -109.21980161063786, -109.07140273870678, -109.04628915564135, -108.79255665097845, -105.20875397856382, -110.0838008881032, -109.68293832806683, -111.24644641302518, -110.01257579497496, -110.99281477454484, -108.99296184719546, -110.96495665514604, -110.70404386182749, -108.25078498739035, -100.77667501455139, -107.61479263900088, -110.06600976399395, -110.02035637581871, -111.45524052052504, -109.975541184397, -111.07333860975358, -108.4808974233161, -109.59513524582242, -110.74711589861774, -109.50005300854993, -105.23071652566294, -111.81094849223531, -109.0168079712372, -111.89029991620679, -109.90672274216391, -109.30959446424889, -108.23718655264584, -110.10868108588909, -109.21139771899594, -110.33333323577992, -110.25792318324204, -110.67825932924109, -112.33148517950511, -108.9724848367048, -110.78371843797613, -111.40913868573313, -110.2930522718577, -111.9538408094371, -108.63639312641844, -112.4462941079034, -110.40266356498321, -108.66617580940074, -109.44306834729083, -111.08962916641603, -110.52132608161017, -110.53757698855654, -111.5587344449704, -109.77722315102946, -110.40060629757771, -109.45395807961631, -108.77558572395142, -109.0151938598724, -109.80739619986889, -108.9332873172888, -112.49933978358132, -111.28667321897437, -110.40629082858706, -109.9829216820938, -108.85102919990373, -110.84179127037925, -110.27309817549309, -109.88857884367955, -112.24517967927224, -110.23377125710859, -111.26951227953063, -110.09782138347559, -109.77508406986834, -110.55359722398646, -110.09534729906368, -109.96333904888587, -110.29372855476366, -111.36651812163072, -109.97141184588116, -110.16701683369045, -112.8562627359291, -110.66651146857079, -108.78873821095968, -108.59208174618087, -110.31784275318834, -109.43177042415276, -112.80272887161644, -111.79874205007107, -111.08216899537892, -110.73699224045636, -111.04738767291953, -110.43395896705012, -111.62106163510778, -111.32599933330843, -110.29360981749807, -109.66562228449096, -109.21316193790335, -110.06363162177448, -110.54480468587292, -109.31791670875509, -112.65386492377107, -109.91857609999171, -110.57233605624137, -110.7597333064856, -111.49767138733276, -109.36548654843229, -112.34145274183716, -110.52831153822652, -111.55802243871352, -111.81399803046556, -110.17680125962372, -111.23811621944807, -110.48042049674514, -112.43786993562033, -109.56507357271987, -110.67030752598993, -110.86377249100713, -109.06001892813467, -111.37023727930494, -109.52881096984436, -112.95107295160436, -110.49467818026214, -109.29804210589607, -109.89270706931751, -109.46354468058833, -112.10350702955014, -111.06083529077077, -110.49996587015904, -111.1617248913634, -108.84725633199014, -111.42852695852422, -110.01433866707184, -109.11616968390972, -110.76961079765468, -111.80403513904453, -109.84442686379181, -109.65447921666167, -111.3378640555306, -110.8882647652338, -112.58014202075226, -109.67128881545659, -111.73429980763389, -110.82258070774773, -110.71895931098041, -112.5117489008152, -109.16182299471309, -109.71651258790612, -109.7770618808562, -111.94294809571427, -111.1629115541574, -109.57489224865171, -109.8402445779754, -111.17931450307283, -110.09045865447595, -109.23658206733491, -112.54929616847242, -110.5150381158864, -111.32296447909377, -111.64472156295191, -111.65832771066007, -111.03359562742956, -110.85303206770837, -110.80655337650862, -109.3712696310075, -110.57313454785879, -111.18525355670417, -111.67423695430561, -112.00829831274282, -111.08915434609605, -110.3298290221436, -108.68552957386795, -112.11377370993225, -110.80288297661977, -110.33640536217185, -109.5907971201988, -107.9195263775506, -108.50223113159429, -111.91191347156142, -110.29585599512956, -109.50902788911351, -110.76819145749467, -108.86899533416589, -112.09963049260891, -110.13374376572433, -110.15881393584463, -110.87392107947531, -109.18658540731009, -109.72734703956934, -110.18732487568724, -108.76554115185057, -109.94122289815374, -110.39583285609643, -111.09540935727229, -110.6618176357367, -111.6281345666718, -109.69686483639367, -110.31633402076315, -110.61246951748903, -111.73300235294965, -111.34221378834899, -109.46708370903485, -110.70412671997354, -110.7007891485379, -110.31685483435038, -111.03016917417074, -110.94517365625376, -109.46580797053619, -111.20935248224806, -109.20661126636224, -109.50147037097533, -110.14241781654353, -109.8510950344643, -111.3794198224028, -111.28966889207122, -110.43347441663424, -109.86759980279523, -111.92101892013198, -109.31594011390644, -112.92253433794441, -110.74000829597605, -110.3690783911604, -111.9386136764295, -111.04196305034188, -110.41800427558245, -110.94287511448232, -111.66035388807579, -107.53723747644062, -110.68014818358719, -111.86628806511304, -110.12097497430523, -109.69880468221378, -111.4312783987915, -109.18240866486639, -111.45649839248873, -110.1242345454651, -113.75911576151633, -112.71747598882953, -110.9614554157337, -110.92294419716129, -110.87229098694876, -111.09943759113875, -109.48107247947176, -108.62783006742795, -110.8108025857779, -111.63342408317932, -112.0221522906341, -109.96411229549527, -111.29821085030613, -110.04566676239914, -108.41674583097112, -107.50256474992416, -108.68086611003493, -110.3738906060137, -108.86763212826641, -109.81681043446049, -111.04539822346567, -111.73290882980949, -109.75238769150758, -110.55268275367449, -110.48423701377924, -112.1116140908134, -109.53952175199518, -108.538611608547, -111.3788321484912, -110.36378736224961, -110.37712171023523, -109.82150687920334, -109.17046632238393, -105.1169578108227, -110.84067642540583, -112.91626789016587, -111.32030958133453, -108.93375913686056, -112.44450956563915, -111.1596840012794, -110.17380444915341, -109.634859036508, -110.68819277718731, -110.0648098825346, -108.87385575091399, -111.99676414571755, -111.32585405719519, -110.59892045991457, -110.32589048340424, -111.1172696292077, -109.79946399891651, -110.10030723919304, -110.71841081343656, -112.23013150012054, -108.94400401141407, -109.71044551701596, -111.77560214164039, -109.68779520039777, -110.96119601299907, -113.66477058855787, -110.17794649102234, -110.30159876509862, -110.11953836266514]}, ...(2 in all)]
  out "FFT 2":cluster{"f0":dbl, "df":dbl, "magnitude":dbl[]}[](graph)=[{"f0"=0.0, "df"=16.666666666666668, "magnitude"=[-324.19011195451765, -78.1272953812706, -85.85545438627958, -89.30587144190069, -92.90590394398903, -93.63083388385274, -91.8644929119412, -95.26924857401164, -97.0710469181336, -98.01148078956652, -99.33043660296804, -95.58776817681839, -99.9570097527269, -101.45494093095093, -101.51838334751548, -101.00386616525799, -103.01963069818913, -103.20223925731209, -103.53783076500916, -103.48065647812659, -103.97797518531912, -104.58942778240602, -104.46991277190502, -104.59813972158683, -104.56685024229951, -104.69893799348945, -105.05669000016238, -106.17061117835001, -106.43303821862656, -107.39468286383597, -106.2899368267905, -105.7863846168199, -105.17170638885071, -104.53818172761852, -106.70340956723133, -106.55444321137247, -106.67654843051936, -107.79888413750199, -107.86424326005849, -106.09722609215336, -107.71648639013972, -107.79500725395155, -106.17330953637067, -105.43663624517525, -108.04970689199158, -109.92106271611999, -106.2505251183406, -110.60221373795562, -107.11377887451098, -108.4126937286195, -108.37794745021417, -113.22457316369011, -106.38281814065472, -107.55385617652075, -108.93026538982782, -106.19334142366085, -108.90462602264525, -107.63084712174981, -109.12192537022624, -107.90627042480016, -109.44472079190832, -108.91731458372392, -105.74102972706788, -105.74407510394178, -107.5989477192235, -106.2838630137392, -107.46190542725505, -107.38881299750702, -109.08024783239452, -104.97871836903269, -106.65424712290651, -107.04966019632134, -106.16202578092883, -102.98374199247179, -99.1568704142098, -87.07383781389657, -96.41471411313154, -102.65176579899618, -107.65674867775193, -102.85397890306213, -107.58658613411464, -104.79044898833125, -106.65282019869865, -108.65027966345534, -109.46169054950127, -108.69969979291741, -110.4048706652988, -108.81020193837274, -109.42808902484134, -108.85398463561398, -108.3849716744813, -109.1844457168716, -109.32787859535676, -111.01992124870878, -106.64843449415699, -108.9926343573667, -111.59837822080355, -110.57121677672183, -111.17280164669164, -110.68901970586144, -111.69013245592781, -109.90200577018311, -109.3554172126163, -110.7515368822992, -109.2863324212524, -109.66209701262974, -108.50795548698007, -110.58126481096504, -112.36093896766921, -109.78612141282203, -108.85120530917233, -109.91424431080952, -109.84698632196245, -110.93960894966105, -109.77214706089354, -110.30762971422381, -108.77791302937449, -110.79522659679036, -108.47242514643455, -111.20629758187835, -109.05996769621125, -111.13574821570619, -107.79388178889101, -111.5768481279296, -110.52058839597171, -111.58729762739313, -108.99000864386126, -111.6585121505227, -110.50715371958135, -108.87151956974363, -110.30486244367107, -108.32392040018144, -108.1769507919999, -110.43198471512189, -109.81454097966842, -110.26717009815644, -110.82924135076777, -110.34103661156989, -110.0692667126265, -109.34555682020833, -109.1694484721415, -109.9940980324044, -110.81940616215803, -108.21162003366862, -107.97087538330561, -107.55312461506225, -110.60339321606872, -110.09004629292225, -109.05860430198882, -113.1412749514818, -109.81628200948371, -108.62343219429849, -109.48172424209761, -110.85978755785311, -109.47778611557064, -108.81728552967951, -107.47864241666747, -107.61735128422292, -109.62511618983821, -110.32417726356636, -108.24287897478176, -108.60460879530194, -110.2181558494026, -107.95550802888957, -110.80234484950323, -111.09955733353904, -109.43923052503506, -108.98949130235951, -110.05778199870154, -110.36224432927585, -108.13523430027999, -110.681114579241, -110.49106131529867, -108.73493328004297, -110.07663907252234, -109.9968931372618, -112.10715231091008, -108.80994125105168, -111.63774865669372, -111.54355694032755, -111.64024217585788, -109.34986300492378, -108.88053713185408, -111.14370830146245, -111.17327416167232, -110.36311492990576, -109.99414559884396, -112.96912007380595, -111.43191437097785, -111.71327312809349, -108.77202323682606, -110.25970374932486, -112.59574277180732, -109.77247894866957, -110.09219852365874, -111.7197662726775, -109.85454092697009, -110.06789440397942, -110.38055758638309, -111.04251386932805, -111.54279434240568, -109.74385329575985, -110.98924544863415, -111.17898077762852, -110.98364252730245, -110.75024385843372, -109.24766708578407, -109.67753987004863, -110.6537235844391, -111.84436313010086, -109.12654337292446, -109.65519521121124, -111.1845162935778, -110.5009101465602, -110.22980642268818, -110.88540043278346, -110.29249073109453, -108.80459864528464, -107.49372141121728, -108.50353962704821, -110.00730069533373, -112.012876492648, -109.01283702976382, -109.07442203290057, -108.2961442983685, -111.60962842680907, -108.84312815413224, -108.6276642979969, -108.75132871638827, -109.30004903844721, -107.20359872252604, -109.12175943862074, -110.43914247337625, -109.55954680842791, -110.37116786618797, -108.55907813251434, -110.19249995041955, -106.95269845697632, -111.07027929458712, -110.1073996792702, -110.61729280468039, -109.6419175310234, -109.47995019876329, -109.66602827275211, -110.01953864498805, -108.45989120418268, -109.79778555296474, -109.94663827736616, -109.52410616839379, -110.58014441463794, -110.09182359045897, -111.0487262011397, -110.49609187214915, -110.6114701312941, -111.17752423063314, -109.74965389041003, -108.58973724447526, -108.84292130035902, -108.90689510645983, -110.69840140049361, -111.30494362640982, -111.00224390075273, -110.50848328538423, -111.59232911931113, -109.30826761863756, -108.44510893127558, -109.63744704504391, -108.95037574307332, -111.36486409910674, -112.74508631930381, -111.03952454593811, -110.57133212903979, -110.59969855145111, -108.25570461975128, -110.44617635200193, -110.32190307214704, -110.95204704643322, -112.0595421753479, -110.45342552693265, -112.50183987758867, -110.08217804938009, -108.90353583389084, -107.02032313792242, -88.3334978919524, -107.92027625495886, -109.83148570028482, -110.30427997450572, -110.92855407802753, -109.67404674397338, -111.03606345823586, -110.58277018943096, -109.77692362669393, -109.39170901729935, -110.20711662408928, -109.41601946806779, -110.34213214925832, -111.2283900972803, -111.51682597931386, -110.47069117801351, -110.93808974285523, -111.11277478000933, -112.50698886748012, -112.12918507523611, -110.46316790252011, -109.9387334819968, -109.78723249688426, -107.13037722044297, -108.16132376075751, -109.07255491017162, -108.85068428558272, -110.28038153100799, -107.77611023481016, -110.69754506886444, -110.09495581837979, -109.21214884561816, -112.62718526248648, -109.22048725312992, -109.17793923163308, -110.87372121410577, -109.71902632604333, -112.61041177225496, -109.6374750969677, -110.74738952366951, -108.93404661877067, -109.84938675700889, -112.25316361679832, -110.30788094875312, -109.26929069321925, -111.20853536783942, -110.05212566057608, -111.72448131932816, -111.55474439772887, -111.81988954424324, -108.44452452934028, -109.21897824914645, -109.55634869894358, -111.36318572800242, -110.05777399011298, -109.64458567712875, -108.73315084760529, -108.93332091319675, -108.4816455312154, -108.80120578498936, -108.1804470361839, -109.7177707524778, -109.31977709844544, -109.33603116022124, -111.46120546572519, -111.7480378245176, -109.17907150677627, -110.47970652472505, -109.73718750984082, -109.7935026884937, -110.40458408612054, -110.91781389491092, -108.39352075861481, -108.27512197925346, -109.59155075404814, -110.40183121737397, -109.25423373270381, -108.37769008625712, -107.91335995938509, -109.5576520703013, -107.27392145737491, -110.98592762117059, -108.41809950647861, -111.48163889400448, -109.70961684769624, -109.22952568656495, -109.76504719131209, -108.86928627177666, -107.97855299877004, -109.8412204399902, -109.6690048999326, -112.28329030175193, -111.54977099314607, -109.55689540119126, -107.93716711232997, -109.84247640855929, -111.5098351445789, -109.14317615215809, -110.28319116384824, -110.57901069942578, -107.2890252845352, -109.66754569546274, -110.15708115946433, -108.83782190109405, -111.60783857760667, -111.46884385151185, -109.21985333366634, -109.63605494317056, -110.87999187262697, -112.26992029775087, -111.05491095860552, -109.22795442529183, -108.99135781712076, -110.46475190704264, -109.35746113713218, -109.29125989270668, -107.40922407684049, -109.24391685563656, -110.41554602144217, -110.68952735085914, -110.62457364102458, -110.39856310555466, -108.84256124354566, -110.01614601335088, -109.8071306678428, -110.2804500736802, -108.76205061238203, -110.3962440297242, -108.98253716257014, -109.32990745926702, -111.17276766165281, -110.41113652364085, -110.36616199963426, -112.09767002991742, -108.43599666470733, -110.91876588140981, -109.05329272502944, -107.07198690769708, -108.72934463903034, -108.6666471996132, -108.97529973794413, -109.68895260146817, -109.2658844652487, -109.75690097249196, -109.38585024123027, -110.17593039468063, -107.87223111061134, -108.15261097418302, -110.09277437980633, -110.8665497655964, -108.43061614348413, -110.3052458526819, -109.22446919161898, -110.51909692711594, -110.06620699121913, -109.53439413051383, -110.31952463872884, -111.4732125902982, -110.41443606663168, -109.9579358088152, -109.930778061577, -108.5473214465574, -109.34719220288939, -109.16964653934396, -110.04824158176345, -109.42616539603762, -108.3556027482992, -110.62331917617789, -111.3652147859356, -110.12362012120938, -110.13175448595814, -111.20110099151856, -111.50643914621541, -108.11659117128028, -111.06037600347967, -109.03822892917451, -108.25678204604324, -110.82608024151122, -109.15887945314851, -109.88255674562845, -111.18322672526185, -110.95836040044516, -107.91535345885436, -110.66285812468733, -109.61906549925033, -109.58059721670746, -109.65198009505977, -109.65950565672951, -108.95264505276342, -109.23343669003113, -110.74308548011575, -106.39170014998685, -109.61471203101753, -108.24258770956924, -109.84609566640096, -107.83834185503922, -108.93052854090027, -107.55568820082641, -109.758551082242, -110.65892780872205, -111.99907420485852, -110.71043004141137, -110.62257237494617, -109.15610413532767, -106.87403836327807, -108.19175324576331, -110.27819583792918, -110.23918003777561, -108.29703377268754, -110.07182881114713, -109.60256111108491, -111.00394752430006, -110.30750337485472, -108.78309624082331, -109.24103013025798, -108.76979253891403, -109.91618737478264, -108.83915940855513, -110.92536150834754, -109.72250903746432, -108.96533939688658, -111.08949280651164, -109.20335070860871, -109.37826578362439, -109.77953166722301, -110.1867310744785, -110.07114559821346, -110.7003631567182, -107.86455899696074, -108.94113264174617, -109.35999427135138, -109.33627364788704, -108.96588828808375, -109.08716536982254, -108.73575375369026, -109.47770132070654, -109.83726171472907, -110.73516506891792, -110.56827134787686, -107.65667508354096, -109.30200115708924, -109.28406803847896, -110.55374624323233, -111.2017766725333, -108.50851279608973, -109.79494403619485, -109.08320018013063, -110.21850624918747, -108.4652936555984, -108.74837610538873, -108.81326140648238, -108.83830180036702, -108.785270477003, -110.01845876259073, -108.76030368637825, -108.57879884880157, -110.6610608456059, -108.74669367794318, -111.55956030460833, -110.22906685783455, -110.48411613865359, -109.48060880085136, -112.77556331479562, -108.2676071206087, -108.8571136162698, -108.56944905160177, -109.16406757131058, -111.42259299295839, -108.25216316582294, -110.48487127684025, -109.69532331373831, -108.13992755196784, -109.2987762526628, -109.82536192480795, -111.28650061088359, -109.12820736404241, -109.37960655471406, -108.96014976926716, -107.97535047619023, -112.31953123574708, -109.06198330523004, -107.52722515967098, -107.31555373665437, -99.89671790804692, -107.44442600896275, -110.6549218761941, -108.02265794322076, -109.63582761762919, -110.00574746987859, -109.51565124961209, -109.3550083591902, -110.4541529175301, -107.85799722437162, -105.1197113090786, -110.25038075579738, -110.39710812865657, -109.3618876098789, -107.6131301952152, -109.21529527621463, -108.7995754403799, -108.48347353145697, -106.45678488065816, -109.60427918561142, -110.81194387812535, -109.52215044127382, -109.88751598659705, -109.30205143590227, -110.74984456751768, -109.03952092986351, -110.69170786328897, -110.39236248162467, -108.65456161733339, -107.60439764386904, -109.97367926606955, -110.2754359970249, -108.81546418006434, -106.99691398176165, -108.42047325825182, -107.24499915944605, -109.28116135603187, -108.70650358781573, -108.05516916105047, -107.20893100196241, -112.07029265690055, -109.38099990478445, -111.53461820465232, -108.11312509555277, -108.76714028655223, -109.89565008459624, -107.71879172001115, -108.08434857420214, -108.79142773619792, -107.25153085963885, -110.05595039449301, -109.31604222314259, -109.94405791565286, -109.04715370361387, -108.89278831045846, -108.84682466376424, -110.0067927716526, -107.63768959294084, -108.98109382020348, -111.4720219575084, -110.76023788797733, -108.78599647633777, -106.59726674064618, -108.66715709719243, -107.99134359630926, -110.11396713841884, -107.21091759882775, -108.08576824949941, -108.80217666857972, -111.72949572713338, -107.33126296136014, -107.33731660097102, -108.04470462977443, -109.42963925921418, -111.03517778720736, -109.55293581015796, -107.99948151285162, -106.59480934999681, -107.63777243313498, -108.96490626068824, -108.8948210299064, -108.30870516747477, -109.13612869658097, -109.59971429402015, -110.2571461001396, -108.7655464686992, -109.81144209568883, -109.80796806645141, -109.20948481699544, -108.68653880881129, -109.26329796696166, -109.22428132233863, -110.12571678351438, -109.14615461144786, -107.08261621308327, -109.11338327144382, -107.75421565039201, -107.45291780756361, -109.00477000647248, -107.41031480478154, -109.98948062864928, -107.45953654921264, -106.37522884807879, -107.7786128523167, -108.03610987358499, -108.05926797128022, -108.59400205554164, -109.89620453365603, -109.03811240487515, -109.96909236705363, -109.28212981785472, -109.6772152101994, -108.26493868190678, -110.55558039199732, -106.6252818398841, -110.19075011176416, -109.56520012524705, -109.8023423576176, -111.2697570480663, -108.26752571816566, -112.00337375484828, -109.85709226796116, -109.36922081321148, -108.8424844298318, -111.2512302139209, -110.61775974680471, -110.22501328999012, -107.76874906708105, -110.71023653476604, -109.4025656165291, -107.66667684986125, -107.59759854092948, -107.94763263251238, -107.3888591871119, -108.62692803125044, -109.18012867988286, -107.78662871481455, -108.5072814073944, -109.50348958982907, -109.95177634938378, -107.78756251182895, -108.03865042797304, -110.1814993556385, -109.34937567548833, -109.52162025123161, -109.50819015441117, -108.20953105254624, -110.52154040214435, -109.3324404469266, -109.2696617050831, -109.54675609195674, -108.5940367000989, -109.40184828664549, -108.2518305610941, -108.55972691669434, -109.03647225394408, -108.48166656251695, -107.42023429066523, -109.42453054302521, -110.09532345960083, -108.78315822119662, -109.97508586102265, -108.22687406536997, -109.17110028890058, -110.15390449992647, -107.88577458651508, -108.28851074361447, -108.52030295163331, -110.03496861709483, -109.40014319167584, -107.73048113044877, -108.17571683963915, -110.34839852994926, -108.55894048192191, -108.74107339998285, -111.17734138993401, -110.22946440841412, -109.45511941802884, -108.0657300641843, -109.33797363184166, -106.95974095511333, -107.93068343723691, -109.78867669512647, -107.2087297624043, -109.542665021243, -110.05035859052961, -110.30235238883523, -109.20586170783808, -109.2796396673401, -109.14260673746566, -108.22019460542734, -109.99011886871159, -109.89103038547285, -110.36964772493243, -108.62340319923602, -109.06779821699769, -109.21830861066148, -107.7402395759509, -107.7178850938205, -113.45665085929117, -109.24039191621704, -109.30387033426037, -107.61849760982835, -109.41430582703529, -109.11482836392241, -111.89328423764577, -111.84653367963301, -109.00674896486915, -109.84488648739638, -109.41914760797953, -108.53442910169935, -109.66883322968232, -107.68762956301386, -109.82583101109167, -107.83405397804887, -108.78052031141966, -107.37842078941692, -105.40843158543845, -108.81430898189338, -109.57374640194516, -109.41111270322058, -108.82621700188898, -110.2552502368822, -110.23903890097205, -110.52171662278697, -108.21249857906324, -109.97268479379733, -108.20088823960992, -108.85682002802234, -110.11642849164285, -109.94087886999255, -111.63180946270296, -108.20899499456195, -106.73341567332112, -109.90003508676807, -110.14688274481229, -109.62259307329889, -107.57811196819495, -106.88584597822792, -109.16132624528932, -109.78677836397806, -108.59319344451784, -108.55877448618652, -109.46883711353044, -108.47309455543844, -108.09487065732198, -109.82219079158135, -109.63780237877428, -109.28348848877269, -107.62893405379826, -109.46986737961593, -108.03089712610223, -110.3931917410696, -106.06970126043262, -109.41866550703786, -105.31710372440419, -109.20218082282653, -108.28467118008108, -108.80026326744611, -107.40729224715713, -111.07322915141532, -107.1057186510818, -107.98286374205958, -108.51298722989311, -108.69632670891366, -107.96509231988331, -108.15882223414738, -106.85862416470376, -109.70705792539056, -108.64519930633055, -106.78708421443504, -109.43552377900174, -109.4474526498122, -109.10135248755788, -111.43316642580763, -109.33457343739448, -110.23547887071898, -108.95690647379442, -109.21159903769149, -108.12969562680841, -110.82751409340537, -108.55724349027832, -109.8796329603075, -108.50369978374582, -107.43145467247209, -108.60003323209516, -108.77155705999647, -109.33806063660796, -108.37500858898439, -109.65641721611547, -109.81905873737344, -108.03483220769625, -110.48028107566635, -108.60527372219985, -109.28768201151478, -99.8804125587218, -108.8913334544964, -108.23534920737794, -111.07646463287153, -108.59029790589766, -110.3405916586831, -107.66387718565608, -108.73793152614131, -110.61440166477816, -108.76211382544581, -110.23236978486065, -109.10669297094852, -109.15247609779597, -109.00539004923506, -110.14424353412238, -110.55445060661157, -109.48721312920799, -108.17040942305823, -108.77592227268228, -108.77130256578067, -107.82494496098512, -109.57266989523707, -108.75767497229612, -108.13688624150026, -107.8280716764963, -105.676279602552, -107.6370316684844, -109.73508547021689, -109.25365178573009, -108.86767843317584, -109.70969944273735, -108.91917504090888, -109.97734866522867, -112.17308993943783, -110.28356299479682, -110.7927103729386, -110.30837645846702, -107.56364161860179, -109.50188349731121, -109.36065627483853, -109.75389877587511, -109.81713476007774, -108.14524057525358, -109.43832376796216, -110.89342891210596, -108.15657882822792, -106.84106061627887, -107.83091759905821, -108.61794662682962, -109.57142366843581, -109.85402645528154, -110.12877022469837, -109.19414429724044, -110.56168468006764, -108.74720588273881, -107.90448559921305, -108.54421401507743, -105.06700039841249, -109.17937358052484, -108.94317576365822, -107.79410219455083, -109.24955437598658, -108.23334395173994, -108.98759227946937, -107.05986359444529, -107.20956512998849, -109.00295831471958, -109.43119556916457, -108.93348410522628, -108.99932477701081, -106.6448790859128, -109.06877251308666, -107.67053918439544, -109.15052780608639, -110.16878033319385, -106.55101141640301, -108.02811045752685, -111.52173447126572, -110.16854119242062, -110.93164036911654, -111.25979320890855, -108.82629030379024, -108.52004501839738, -107.09697056562636, -108.94233383169858, -107.37962568194772, -109.1239201710643, -108.93949898577122, -110.62573772949195, -110.09592372075662, -107.56136391005947, -110.45600430869621, -108.79481000016084, -109.41462449554598, -109.30248158488335, -108.70735295493108, -109.9174743694956, -109.94232543385962, -110.71725446170196, -110.0346196158573, -110.34814317845934, -110.6651078322521, -107.55409880424479, -108.71734776861287, -109.50902203986271, -110.40207542979611, -108.7847687630861, -111.10599488129682, -109.30824728923263, -108.20134064331717, -110.55959112431609, -107.77099734327174, -110.23862843385446, -108.48520797666865, -108.54205896654946, -107.79288769037599, -109.84022250170581, -108.02758364115576, -109.35132492327935, -108.87009749667932, -109.86905123364855, -109.19826752168308, -106.835240323691, -109.37910022114056, -110.80633973102931, -109.12703823829597, -111.07432699570984, -111.8064506085314, -110.09349947650527, -108.66467295777367, -108.75119108236053, -112.63983351316729, -110.90940743670113, -110.27973159222081, -109.57141664526549, -108.61645363771719, -109.31742355616147, -109.5839599160637, -110.01188998365383, -110.01923429741011, -108.94779759137936, -108.26169431000017, -109.24553201026085, -109.95709526422822, -110.68677343596859, -108.7678734483002, -110.47090469179284, -110.31604700116512, -110.10256600741997, -109.76634647265719, -110.8830805828562, -109.94609564072982, -109.20662382740542, -108.12492970530919, -110.5274435478767, -108.02351960398035, -110.6264936805739, -107.14559226383577, -109.13821777857531, -111.05324489472586, -110.15190797512811, -107.96366234783144, -110.03950681967147, -109.17476300510336, -110.41251816187909, -111.39219865477246, -111.32530426869943, -109.97369363558423, -108.98666403063845, -109.62049358645565, -109.58130494498671, -111.72738873188874, -110.39825891106616, -108.57430325757545, -111.28625510212446, -108.77421250595326, -109.75025415031793, -109.51948456745635, -108.82129398637998, -109.81362137198361, -107.86292494316123, -107.49318292857053, -109.66948564589373, -109.54288390056654, -107.99912445612077, -110.3497559614379, -108.00549349666127, -110.01361420523357, -108.4977916421456, -109.67078387286976, -109.85678367732866, -112.01237658746248, -108.4855625950998, -110.84880875737286, -110.9178674382154, -110.44187536727453, -108.75076921971127, -110.04946286646651, -109.99780941000827, -110.14242932305507, -109.56343773672316, -109.6278993388131, -108.77419573790174, -109.10543670530926, -109.7801848627463, -110.30733124104881, -113.13440550301436, -109.32709134514755, -109.74136656933283, -110.01525283266193, -109.43924662938396, -110.25325289253, -107.75460576671303, -110.60057027395933, -110.71458404922404, -110.15788509050662, -110.69167485018224, -110.96006652476157, -111.01156633983031, -111.6058448010008, -109.51364005052672, -109.76058205940885, -108.43421621088261, -109.47973949170208, -109.25533250208288, -109.47422603921065, -111.36411644613841, -107.27566171102698, -110.45098686173688, -109.93589296291184, -109.03803734663714, -110.53118128434016, -110.2408872254969, -110.0532234862915, -109.94185495614619, -110.2662004220774, -109.51094016962288, -108.5210104215432, -108.13691752270934, -110.18460088390265, -108.32609309150783, -109.89652230508281, -109.80923900768477, -109.01917388968883, -110.01248300968739, -109.43415605440147, -108.09823485138017, -107.40637725320931, -109.40632232658412, -111.97981999127656, -111.16609811629485, -111.64500793960192, -110.99793748693381, -109.55531276386903, -110.2535662621666, -108.17429802469516, -109.09425673355422, -110.23187110421917, -110.55358397926925, -109.93461124753053, -109.55604345832225, -109.44569510408274, -109.72185151080762, -109.52963702944834, -109.2303630328152, -109.74819502244243, -109.3932530349457, -109.17096788339686, -110.46153727064616, -113.1073731246639, -109.43753070459397, -108.13332547768168, -109.42294574929969, -108.45798401969856, -110.29453435046327, -112.66249403705643, -108.78314667434937, -105.9634478773668, -109.14327524669528, -108.50645190860273, -100.81571594994128, -104.4482859840643, -110.68926237051092, -109.12362553230196, -109.45234390564677, -107.91461416156068, -110.67788819353727, -110.05744935668449, -111.78333392154664, -106.83628914455993, -110.11115457346548, -109.13434608275826, -110.80006861194663, -110.35323502651462, -112.29149906501372, -109.01656376530778, -109.30871662948859, -109.79736315392456, -109.17848983603582, -108.09752397056482, -111.6039030763455, -109.27008844877828, -110.84475733314184, -109.72393917557073, -111.31060762894991, -110.78858793807466, -107.12841545099752, -109.54510865218204, -105.2805426080281, -106.28514149354733, -109.50656759582803, -110.14700878401054, -110.49737016725709, -109.19811547071924, -109.92527399676051, -110.7961615015146, -109.7447227818197, -109.49432012009893, -108.714081576733, -110.09766801550917, -109.08448507943001, -110.36154838733857, -109.86328656267403, -109.21144237434696, -112.4145136888034, -108.57567151011159, -109.66748589540896, -109.72985837578446, -109.29989238126763, -109.85868902806475, -111.01778182304162, -111.23625326328558, -110.01270868104203, -109.27067928081415, -109.71171312410247, -109.28697459293629, -110.67868067201007, -110.91353786857455, -111.21479955051575, -109.11315965407708, -109.40418681804496, -107.80511819596003, -107.37201025889816, -111.81969609169838, -109.89875624306032, -110.29328043898657, -109.74853280072202, -111.39527865400605, -109.47746221101964, -111.75141177452517, -109.31325306583483, -109.30117448911659, -109.3997781364162, -109.45356931295724, -109.60585285774386, -111.33951689512735, -107.74187210470228, -109.62706021606415, -108.72139655505221, -109.79552836110567, -110.64354037499807, -110.96138240913136, -110.02215059889615, -110.92978442698893, -110.0620778287114, -110.85019647293322, -111.77397403227091, -109.81257196800128, -109.15643451383403, -110.72777566469594, -108.7463769025616, -109.80959395914073, -111.24500986151126, -110.48863498350322, -110.30863780110901, -109.79331354195703, -110.34087081762074, -109.45183222569266, -109.6440990067103, -111.15034876658994, -112.14912485578341, -111.8886180186196, -110.57054820211916, -111.07556239924551, -110.5872832735073, -110.28912501038172, -108.91501133754849, -111.44575118962761, -109.90799859177967, -109.74421995550023, -108.70941446115883, -110.28822893097275, -109.70039554000401, -110.33701797570251, -110.79445894683306, -109.57694314608153, -108.816904416038, -109.66517126767175, -109.39501469321644, -110.85775022889956, -109.3689402795614, -112.09107318723095, -110.67985626248422, -110.32971146814747, -112.08166943494875, -109.93955548712543, -109.31722953035252, -110.2062913031861, -108.22565380081006, -110.680898028151, -111.95386604441454, -110.83354130587097, -108.5873626748948, -111.97536144124408, -109.23944159551515, -111.57859477689586, -110.80135186615524, -110.4800953731021, -110.14040729648133, -109.25873050390551, -108.87000960474569, -110.97091597211167, -110.15787270199012, -111.62434537618091, -108.5421625277294, -110.42258666403919, -110.96896115868603, -108.98253068925274, -109.54245055160168, -110.28051096122468, -109.48060498658319, -109.77618362117276, -111.64513838754992, -111.13945484239875, -110.18094280356001, -110.43757222770748, -110.81588360154201, -110.11656805555333, -108.47936291282355, -109.16476249859961, -109.3549985917136, -110.77753190334253, -111.46065694661178, -110.40387985996301, -109.95673803226478, -111.58660981285446, -108.59894875229345, -109.37333363882607, -110.26849699991793, -109.30500469266264, -109.23789020998296, -110.82000706486865, -109.25927538839868, -111.03285659417519, -111.08899832832414, -110.69361682858042, -109.45187168573815, -109.9614018482838, -109.70209527974106, -112.11903952100165, -109.59713611623246, -110.70292028698111, -110.12743849746808, -110.63315585514292, -108.60450276298175, -109.32832664986026, -109.99753023477764, -109.46644696130294, -109.1781290160558, -111.58830180575129, -111.67229040267557, -111.3750024136205, -108.33616679452298, -109.99797067800029, -110.50892429124391, -108.66074740829372, -111.17094662568759, -109.87538933985836, -109.152526628291, -110.44623159817101, -110.21603106403009, -110.64376935639365, -109.36897426842583, -108.67303022227141, -109.89327693080823, -111.50442955563923, -111.37532237834381, -109.38132821290205, -109.73509680539144, -110.53918379735906, -111.22869870340647, -109.39977573957616, -110.3674665334106, -110.5366125953241, -109.99025356764304, -109.97300035646616, -109.87631077033762, -109.64608829594286, -113.02486102973394, -108.26250283140733, -109.62234918138763, -111.18766216512655, -110.33666026406992, -110.5808115327039, -108.2971671321189, -110.10964334161903, -110.61254021379767, -109.89852549557533, -110.16562049054073, -109.41433790018287, -111.2453823439446, -110.45554802599901, -113.11454453784393, -110.7333866145056, -110.00858191882439, -108.54745315874294, -110.08430415376903, -111.9006972727596, -110.3031506154679, -110.26331790366497, -109.36797925566673, -109.04860552478912, -111.83514212681175, -111.38960737633833, -109.01429665187288, -110.96404839103826, -108.95488871107163, -109.09652004914592, -111.884304581971, -110.57566691021339, -111.95113404442795, -110.13677174050159, -108.10078686353354, -107.69442565416006, -112.42676605669463, -109.12681161784135, -109.23120766087519, -110.57649395555585, -110.22143082743162, -108.40065951773644, -109.46923168308618, -111.39095086729745, -110.46375658526013, -111.45145283328486, -112.22610823637353, -110.61090190564383, -112.22250292674809, -111.7379343196361, -110.18530386733481, -108.93867365671692, -111.89304844956082, -109.06146134986984, -110.98405731832798, -109.76366821333497, -108.08326795663608, -109.95041147835065, -112.94140614324155, -111.79814935135965, -108.07337559063119, -109.13733403265212, -111.74906646037496, -111.12228668433455, -110.02899450462209, -110.22237716929811, -109.0224776891049, -110.18135850497721, -113.32516073881047, -111.3576490243877, -110.60510094465171, -109.6935518470342, -110.36313473154901, -111.95933240129618, -109.49625308071019, -109.18827910216122, -110.54311407822692, -108.4811035913567, -112.81280225723607, -108.86530665787413, -110.85796435061886, -110.40059714639627, -108.19250716343407, -108.96956521802292, -108.61281798886506, -109.78061525370413, -111.58885511891798, -109.06279169160345, -111.43043988466789, -111.63169336321079, -109.54702536206447, -109.62860636296405, -109.47865811135546, -108.02265793654806, -109.97461304995515, -110.72549884050886, -111.57309413919933, -110.03317891949746, -110.39570411598524, -110.27606115470397, -110.63294457306095, -110.71821689302902, -110.38076268941819, -111.51223508887897, -110.40703572670697, -112.24933273737743, -109.74954300082398, -108.46020292937696, -111.05315219575881, -110.38635148390118, -109.58268303790976, -112.34211536832117, -108.45894118755307, -108.96463982695337, -110.56040438523046, -110.67803313671729, -111.07349872375121, -110.42184162876096, -111.82081126435692, -108.85923651136297, -112.57723799596502, -113.65690874668172, -112.62314325834605, -110.70357529341362, -110.959925221544, -111.26336183001875, -108.1350700630152, -107.94545932312926, -111.17610778209841, -110.20386728310686, -108.55646511121591, -109.8400922569145, -111.73466587035968, -110.47272877573613, -108.33011124048193, -107.93042857580332, -108.60928277989103, -109.25240966798974, -108.96403833602028, -106.94222615757475, -109.37086694261907, -106.72743097285155, -109.03160193412796, -107.3549903889451, -106.8543848510082, -107.83503929060929, -106.30745467433752, -108.36915807168845, -107.13065938379303, -107.84769200880969, -106.08004345082777, -108.15244601930225, -108.37254117816573, -106.57863034819223, -108.1283698227614, -108.19776505569902, -107.58283412238643, -108.17365133196301, -108.6794309781181, -107.91552140588759, -111.60122989270022, -107.04360635941174, -111.55535949001795, -109.39870426166594, -109.55937904851662, -111.81389508925734, -109.88957041098786, -110.84764586896561, -110.59130246272693, -111.15944135223884, -110.19496154041607, -111.51861903129362, -110.74798816525838, -111.37312965175558, -110.10842817220238, -110.73198099204856, -111.36708667993291, -110.30840247819665, -110.11744489669044, -110.55237850846444, -108.2073528237766, -112.70750856801911, -110.99917956040802, -109.84949484779976, -111.3403161887679, -110.08924435263565, -110.17749213365616, -112.10849123224503, -110.94270741299202, -109.29350963424746, -110.33477486966507, -112.19620157705627, -111.45484078395934, -111.86858843505124, -110.22491147345858, -108.96177661263177, -108.67862820579893, -107.55155410582937, -108.27984439169573, -108.72682528077233, -110.64231212183269, -109.32873093119183, -112.98564364754564, -110.78933114228725, -108.50921025910479, -107.91087245586935, -112.57350030929283, -111.75871577457525, -108.42095298945462, -112.31266064114303, -110.1295657579673, -109.67444664474456, -110.33749884929306, -109.16098218724147, -109.63554874360221, -109.15892392675141, -111.90580809179818, -108.81196712336858, -111.42223552606656, -109.90571484965518, -109.99739812086352, -111.64103850263211, -111.31463957090885, -110.61247447444549, -110.20960333715526, -110.1707327818923, -109.70412636554525, -110.97278093107532, -110.24386747740314, -109.81378546061525, -110.83784085086458, -109.77357954318757, -111.22663832948885, -111.14563050139252, -110.87152231402447, -110.34246044319893, -109.97174570657546, -110.23599592972218, -111.08206161770731, -110.0073315341242, -111.11748366902188, -112.04005964728601, -109.81290191679287, -109.68543639040858, -112.01143296194752, -110.13641850530031, -108.19348942447623, -109.7534468948808, -109.36697824644176, -97.56454580435337, -104.97829040517887, -108.1539132982256, -110.048991273122, -107.46172505860011, -110.49269280640675, -109.94209901400029, -109.38576869679022, -111.43699124347364, -110.89973083498887, -111.2994445418276, -109.25144782032437, -113.25676258473536, -110.82078737428088, -109.97779571182073, -113.36294799183014, -111.38584551238931, -112.17267897274873, -108.56430946159155, -112.06841286528645, -110.36822473102735, -109.54758527532016, -110.48190506674653, -110.03535695860182, -109.3951469796576, -112.41910682256774, -111.38124138857238, -109.37850389100952, -111.65544568836181, -111.55876881606889, -109.3029209617236, -109.20030046194076, -108.82610577621037, -110.53329453526098, -109.96090595542142, -109.67834229432077, -110.62303603007352, -109.8388817181171, -109.22430039793213, -108.92749786663613, -110.05794249283548, -109.58534943218437, -110.50493887507297, -109.96373022997366, -111.0645036323456, -111.28501675364454, -109.77386932343008, -108.8952247140968, -110.09242801628717, -112.90943444063141, -110.72299296247249, -109.39094335967056, -110.95165384057718, -109.59809519359453, -110.4978602309597, -109.67109981692639, -111.2489619905986, -110.0937750887109, -109.76771021128954, -108.32976315018955, -111.3058145792439, -111.09464974601362, -110.99797900696136, -109.174315000222, -109.630351559617, -110.26289147175856, -110.22688407202517, -109.96748050100612, -112.13247633583758, -110.59994952890855, -110.93023020153811, -109.22457750926695, -110.26162558926984, -110.09713110375579, -111.73858994918328, -109.78183160058515, -109.7603471824367, -110.96016892586911, -111.23309626937036, -109.83093663960678, -114.05354944347246, -111.58202863059464, -110.42281828744524, -110.9521484732059, -112.5120328206343, -111.614891937737, -109.84428787405484, -111.61119567831453, -110.43095563229411, -111.71833448430398, -110.01132196809407, -109.37558169247951, -109.14091380022785, -110.42663661754088, -110.3598013572826, -109.78207135281417, -109.94058843992468, -109.88210328447205, -108.6217811850147, -107.17834387173707, -110.6447226986756, -111.10704778101115, -111.24396771977769, -110.47849395539598, -110.75150631628034, -109.67662689396347, -109.23145032835053, -108.83780193265358, -109.43468321661163, -102.22521103859944, -106.90009867479111, -108.91580608784525, -109.58671397003187, -110.56692028436989, -108.75103142680105, -111.00795573084157, -110.75039085328763, -109.48222099288613, -111.8621134816908, -110.26507966786443, -108.885924716389, -109.30841399453053, -112.3188631425597, -111.05677697153163, -108.8268571902449, -109.63028152237679, -114.82339015806369, -107.03435216376964, -111.34847692589166, -109.61354114874855, -112.32687758049907, -109.59816404231358, -111.64248480241805, -111.84075757907273, -110.44017657636552, -110.15181635726277, -111.93813663582833, -109.11826378836209, -109.99779889778326, -109.927119030584, -109.4389650887841, -111.52448814187727, -111.38736268499642, -110.51920914917922, -108.64230614681055, -108.90307263595304, -110.57246891832371, -109.65575340646116, -109.80359672370373, -108.83368585528197, -111.09385004343437, -108.83430005497769, -112.37784208819113, -109.50005381621696, -109.67421750136593, -111.39664088797532, -109.70867599669316, -109.52498993629875, -111.12341349673187, -110.0484037026941, -109.55138667646308, -111.06614422098669, -109.4785941493091, -110.25724082617013, -110.93950616855716, -110.53487953881397, -111.45722057988401, -110.32393446412904, -110.34361936710438, -108.6610336097813, -109.53631603696368, -108.06930707969195, -107.68056561368934, -108.73860971027449, -108.87111384617579, -108.40433837098611, -110.55999576884835, -106.83832061167207, -108.28786975902513, -109.18482905697472, -107.81071696594883, -107.91047268802457, -108.79613111673706, -111.05361322310213, -109.97897453479862, -109.12920563729425, -111.20538391490288, -109.26286135293664, -111.31400407177502, -109.92167984752287, -110.70854322826071, -108.59406515713611, -109.69371333227458, -109.36664873267313, -110.35521729513704, -110.40667924006368, -112.0181844636846, -111.01529188207431, -110.59246505728431, -109.95068312717868, -110.75807466894047, -109.58596443762707, -111.12127793384956, -109.59041634463125, -111.56255571372793, -110.43405578864342, -108.39660324329928, -111.1420710307505, -113.64788483868595, -111.67645688353934, -111.36878760365944, -109.68523694561108, -110.11608766310304, -109.25670490330123, -110.73546181099229, -111.77855039399805, -107.9662794718261, -109.67483334602832, -109.891258579519, -110.24757768183042, -109.50202895993814, -110.07763831916637, -109.96891925839451, -110.97268925927641, -109.31698133827767, -112.27933593506792, -110.36206721075725, -109.47379463718867, -110.27836850941338, -110.63738280998388, -111.3611682777485, -110.72689155959884, -111.55480904927032, -111.16689658479412, -110.35555645743601, -111.56609319131051, -110.88279459952174, -114.73607246523177, -109.95813757295693, -107.64639932425493, -111.26486783320321, -112.03946356928121, -111.8915972448334, -110.35245920812773, -110.83155104803564, -110.67437747473863, -110.9959682920065, -110.7815352345103, -111.13722283763049, -112.54797265493127, -110.06894780898469, -111.65186554925783, -111.83545188116254, -110.65894756123697, -108.48458025065264, -112.43760714427981, -114.1368408201927, -110.40065777895025, -110.1066998945526, -108.60654239598591, -110.5716060205154, -110.74257357180736, -111.1136089342442, -111.53539811075092, -113.2559601458872, -109.2003227548348, -110.42285840441025, -111.4086884998834, -111.61503050693868, -110.8194303494779, -108.9701587059964, -112.58521089509063, -110.10873915265242, -112.43440038319561, -110.03468788439882, -111.57896603236308, -110.21939233582523, -109.03614470500777, -110.11738923539659, -109.55359574898291, -110.416473622654, -109.4626868574157, -111.17164025076731, -110.3579689035081, -109.04338716157822, -112.36157114517567, -109.32125615922843, -112.71105693789394, -110.11019129547768, -108.96439402555632, -111.107663418839, -111.48306369859839, -110.9317530461794, -107.98628540532181, -111.1636972328743, -110.47837837583148, -109.04649309175733, -110.27110334963734, -111.35803630614352, -110.77259078859605, -111.46352820533895, -111.16789261049541, -109.2376344776325, -111.6795794983659, -111.74292205167644, -109.40835022991612, -111.02163652600731, -108.79482078001607, -110.6718658416566, -111.08747067599332, -112.15383726791498, -109.47049126158717, -109.061574046483, -111.23993049318979, -111.02521156588335, -109.46012868444186, -110.13918914826291, -112.08180381836377, -110.61929875223015, -111.4424805369965, -111.43420275069585, -109.71347556238717, -110.24726273025648, -109.7860268673935, -109.94126895018422, -111.41948668868926, -108.90555991781676, -110.81242861886172, -109.65007052722677, -112.12672329335953, -110.01123170946096, -111.13980448279096, -113.92013682657084, -108.6000853867411, -110.66793592761913, -110.61237681642844, -110.00839105230496, -109.38083187034974, -109.46119372195675, -110.3708067287448, -108.55518656223285, -113.33935987443276, -111.92184778392033, -111.80820718236087, -107.36852757311246, -109.51077803361602, -110.066791721019, -108.756710558672, -107.91391289865918, -110.72851430959301, -111.39074956442978, -112.928843679455, -109.87348280521556, -112.21371750380071, -110.82495902297394, -109.94006136010094, -110.58757785050143, -110.2790091349881, -111.43884888223081, -108.09540986530712, -109.63783244641691, -110.19577975613292, -110.01690033746098, -112.75938920157155, -109.27158857362184, -111.19519821680541, -110.14381902425255, -110.45955291199236, -111.55660330002316, -110.75604254261134, -111.02122553784838, -111.6490091060193, -110.93362819419399, -110.49033159684308, -110.70789549836027, -110.41991882034145, -110.0264093421208, -109.18432746063652, -110.15292268755287, -112.40733942236504, -111.32869665965416, -110.95418667871114, -111.14291568823575, -111.75555369152653, -112.98146297069803, -109.73870744292117, -111.33806139459435, -110.18838799491355, -112.60408243005732, -110.26112648646833, -110.58257045107274, -109.75155437454112]}, ...(2 in all)]
  in  "FFT 1 Choice 1":u16(ring) items=["T1 Y", "T1 X", "T1 Sum", "T2 Y", "T2 X", "T2 Sum", "T1 FB X", "T1 FB Sum", "T2 FB X", "T2 FB Sum", "PSD Y", "PSD X", "PSD Y Sum", "none"]
  in  "FFT 2 Choice 1":u16(ring)=3 items=["T1 Y", "T1 X", "T1 Sum", "T2 Y", "T2 X", "T2 Sum", "T1 FB X", "T1 FB Sum", "T2 FB X", "T2 FB Sum", "PSD Y", "PSD X", "PSD Y Sum", "none"]
  in  "FFT 1 Choice 2":u16(ring)=1 items=["T1 Y", "T1 X", "T1 Sum", "T2 Y", "T2 X", "T2 Sum", "T1 FB X", "T1 FB Sum", "T2 FB X", "T2 FB Sum", "PSD Y", "PSD X", "PSD Y Sum", "none"]
  in  "FFT 2 Choice 2":u16(ring)=4 items=["T1 Y", "T1 X", "T1 Sum", "T2 Y", "T2 X", "T2 Sum", "T1 FB X", "T1 FB Sum", "T2 FB X", "T2 FB Sum", "PSD Y", "PSD X", "PSD Y Sum", "none"]
  in  "Compute FFT":bool
  in  "Reset FFT":bool
  in  "# Spectra to Ave.":dbl=25.0
  out "Ave. Time (s)":dbl=1.5
  out "1 Channel":waveform(dbl)(graph)={"t0"=timestamp(0 s since 1904-01-01), "dt"=1.4999999999999999e-05, "Y"=array[20000 elements], "attributes"=variant("NI_ChannelName"=variant(string "T1 Y"))}
  out "Slow mean":dbl=nan format="%0.2f"
  in  "Slow mean N ave.":dbl=1.0 min=1.0 step=1.0
  out "Mean Intensity":dbl=nan
  out "Sigma":dbl=nan
  out "Sigma/Mean":dbl=nan
  in  "Subtract mean":bool
  in  "High Res. Display":u16(ring) items=["T1 Y", "T1 X", "T1 Sum", "T2 Y", "T2 X", "T2 Sum", "T1 FB X", "T1 FB Sum", "T2 FB X", "T2 FB Sum", "PSD Y", "PSD X", "PSD Y Sum"]
  out "APD 1 Rate (Hz)":dbl format="%#_3p"
  in  "Tab Control":T4(tab)=enum."Sample Stage"
  out "Stage Moving":bool
  in  "Read Cal":bool
  in  "Confocal Linescan":bool
  in  "Speed (nm/s)":dbl=100.0
  in  "Furthest Withdraw (MHz)":dbl=15.0
  in  "Confocal Image":bool
  in  "Round T1 X":bool caption="Round"
  in  "T1 offset_x (mV)":dbl=nan format="%#_2g"
  in  "T1 kappa_x (pN/nm)":dbl=nan min=0.0 step=0.001 format="%#_2g"
  out "Time (s)":dbl=6.12
  out "Total Time (s)":dbl=60.0
  in  "Start Saving":bool
  in  "Cal sets to save":u32=50 min=1 step=1
  in  "Comment (data description)":string="testing confocal setup"
  out "Calibrating Trap...":bool
  in  "Trap 2 (ON/OFF)":bool=TRUE
  in  "Trap 1 (ON/OFF)":bool=TRUE
  in  "Save Calibration":bool
  in  "N sets to save":u32=200 caption="N Sets"
  in  "Save N Sets":bool
  out "Save file name":path=path "C:/Data/110526/110526_022.dat"
  in  "Save ave N":dbl=500.0 caption="Averaging Factor"
  out "Saving...":bool
  in  "Stop Saving":bool
  out "Progress":u16(slide) scale=0.0..100.0
  out "Manipulating Trap":bool
  out "Buffer Status":dbl(slide) scale=0.0..1.0
  out "Overflow (data lost)":bool
  in  "Reset":bool
  out "Data Rate (Hz)":dbl=66666.66666666667 caption="Trap Data Rate (Hz)" format="%#_3p"
  out "Data Period (s)":dbl=1.4999999999999999e-05 caption="Trap Data Period (s)" format="%#_6p"
  out "Save Data Rate (Hz)":dbl=133.33333333333334 caption="Rate (Hz)" format="%#_6p"
  out "Save Data Period (s)":dbl=0.0075 caption="Period (s)" format="%#_6p"
  in  "T1 alpha_x (nm/V)":dbl=nan step=10.0 format="%#_3g"
  in  "T2 alpha_x (nm/V)":dbl=nan step=10.0 format="%#_3g"
  in  "T2 kappa_x (pN/nm)":dbl=nan min=0.0 step=0.001 format="%#_2g"
  in  "T2 offset_x (mV)":dbl=nan format="%#_2g"
  in  "BD 1 Frequency 2 (MHz)":dbl=80.0 caption="T2 X (MHz)" min=50.0 max=100.0 step=1.0 format="%#_6p"
  in  "Green Laser ON/Interlacing":bool=TRUE
  in  "Round T2 X":bool caption="Round"
  in  "AO1":dbl(slide)=5.0 caption="Confocal Y (V)" min=0.0 max=10.0 step=0.01 scale=0.0..10.0 scale format="%_1f"
  in  "AO2":dbl(slide)=5.0 caption="Confocal X (V)" min=0.0 max=10.0 step=0.01 scale=0.0..10.0 scale format="%_1f"
  in  "Trap Raster Scan":bool
  out "Raster Scanning...":bool
  in  "Trap Delta (MHz)":dbl=20.0 step=1.0
  in  "Trap Intensity\nSetpoints (V)":cluster{"Set 1":dbl, "Set 2":dbl}={"Set 1"=5.2, "Set 2"=6.6}
  in  "Index":dbl=1.0 caption="Save File Index" min=1.0 step=1.0
  in  "BD 1 Frequency 1 (MHz)":dbl=65.0 caption="T1 X (MHz)" min=50.0 max=100.0 step=1.0 format="%#_6p"
  out "Current Position":dbl[](array[numeric])=[4.2944, 4.91027471, 2.9278058] format="%7_7g"
  in  "Position Label 5":string="upper flow spot" caption="5"
  in  "Position 1 Label":string="Top capillary (SA beads)" caption="1"
  in  "Position 2 Label":string="Bottom capillary (AD) beads)" caption="2"
  in  "Position 3 Label":string="lower flow spot (ATP)" caption="3"
  in  "Position 4 Label":string="Dump beads" caption="4"
  out "Pump 3 cont disp":string="Left: ADig beads"
  out "Pump 1 cont disp":string="Right: DNA beads "
  in  "Ch 1 Inject Rate (ul/h)":dbl=50.0
  in  "Pump write delay (ms)":dbl=300.0
  in  "All Pump Parameters":T5={"Pump 1"={"Diameter (mm)"=4.61, "Units"=4.0, "Volume"=100.0, "Rate"=50.0}, "Pump 2"={"Diameter (mm)"=4.61, "Units"=3.0, "Volume"=0.0, "Rate"=0.0}, "Pump 3"={"Diameter (mm)"=4.61, "Units"=4.0, "Volume"=100.0, "Rate"=250.0}}
  in  "Ch 2 Inject Volume (uL)":dbl=100.0
  in  "Pump pause delay (ms)":u32
  in  "Ch 3 Inject Volume (uL)":dbl=100.0
  in  "Ch 3 Inject Rate (ul/h)":dbl=250.0
  in  "Flush Center Ch Volume (uL)":dbl=15.0
  in  "Flush Center Ch Rate (ul/m)":dbl=100.0
  in  "Inject Valve B":bool caption="Inject Pump 2\n(Flush Center)"
  in  "Total Volume\nFlushed (uL)":dbl
  in  "Tab Control 2":T6(tab)=enum."Feedback on Trap Intensity"
  in  "Restart RF":bool
  out "Total Counts (ticks)":u32=600
  in  "Trap ON/OFF X or Y Amp?":bool=TRUE
  in  "Oscillate Set 2":bool
  in  "Trap 1 ON":bool=TRUE
  in  "Number Interlace Sets":u8=3 min=1 max=3
  in  "DIO count 3 (ticks)":u32=200
  in  "DIO count 2 (ticks)":u32=200
  in  "DIO count 1 (ticks)":u32=200
  in  "BD 2 Amplitude 3 (%)":dbl min=0.0 max=75.0 step=1.0
  in  "BD 2 Amplitude 2 (%)":dbl min=0.0 max=75.0 step=1.0
  in  "BD 2 Amplitude 1 (%)":dbl min=0.0 max=75.0 step=1.0
  in  "BD 1 Amplitude 3 (%)":dbl min=0.0 max=75.0 step=1.0
  in  "BD 1 Amplitude 2 (%)":dbl=30.0 min=0.0 max=75.0 step=1.0
  in  "BD 1 Amplitude 1 (%)":dbl=30.0 min=0.0 max=75.0 step=1.0
  in  "BD 2 Frequency 3 (MHz)":dbl=26.0 min=50.0 max=100.0 step=1.0 format="%#_6p"
  in  "BD 1 Frequency 3 (MHz)":dbl=70.0 min=50.0 max=100.0 step=1.0 format="%#_6p"
  in  "BD 2 Frequency 2 (MHz)":dbl=26.0 min=50.0 max=100.0 step=1.0 format="%#_6p"
  in  "BD 2 Frequency 1 (MHz)":dbl=26.0 min=50.0 max=100.0 step=1.0 format="%#_6p"
  in  "Not-Interlacing Set":enum32{"Set 1", "Set 2", "Set 3"}(radio)
  in  "Interlace":bool=TRUE
  in  "Trap 2 ON":bool=TRUE
  in  "Trap 3 ON":bool
  in  "Scan axis 2":bool=TRUE
  in  "Osc. freq. (Hz)":dbl=0.25
  in  "Osc. amp. (MHz)":dbl=2.0 format="%1_3g"
  out "Coords":T7
  in  "Manipulation Scaling":cluster{"Horizontal":dbl, "Vertical":dbl}={"Horizontal"=0.075, "Vertical"=0.01}
  in  "Freq or Amp switch first":bool=TRUE
  in  "Swap F1 and F2":bool
  in  "Freq switch delay":u16
  in  "Amp switch delay":u16=5
  in  "Period":i64=2
  in  "MCL Step Increment (V_int)":dbl=3.0
  out "Time to Finish All (min)":dbl=0.122877 format="%#_2p"
  in  "Scan Speed (nm/s)":dbl=100.0
  in  "Scan Range (nm)":dbl=369.00000000000034
  in  "Step Size (nm)":dbl=1.0
  in  "MCL/AOM Scale Tweak":dbl=1.0
  in  "MCL Step Position Ratio":dbl=0.5
  in  "Move MCL Also?":bool=TRUE
  out "Final sep (nm)":dbl=4587.0
  out "Initial sep (nm)":dbl=4218.0
  out "Save index":dbl=22.0
  out "Final delta (MHz)":dbl=44.0
  out "Initial delta (MHz)":dbl=41.0
  out "Final freq. (MHz)":dbl=50.0
  out "Initial freq. (MHz)":dbl=53.0
  in  "Saved AOD Raster Scan Parameter Sets":T8(array[cluster])=[{"Scan Range AOD (nm) 2"=500.0, "Step Size AOD (nm) 2"=1.0, "Scan Speed AOD (nm/s) 2"=100.0, "Number of scans (AOD) 2"=1, "Label"="offset curve"}, {"Scan Range AOD (nm) 2"=420.0, "Step Size AOD (nm) 2"=1.0, "Scan Speed AOD (nm/s) 2"=100.0, "Number of scans (AOD) 2"=1, "Label"="hp raster check"}, {"Scan Range AOD (nm) 2"=6.8, "Step Size AOD (nm) 2"=0.34, "Scan Speed AOD (nm/s) 2"=0.34, "Number of scans (AOD) 2"=1, "Label"="3.4 kbp - 1 bp steps"}]
  in  "Load parameters":bool
  out "Scan Range (MHz)":dbl=-3.0000000000000027
  in  "Restart DMA? (AOD)":bool=TRUE caption="Restart DMA?"
  out "Incr. int (AOD)":i64=-7759651845
  out "Time/Scan (s) (AOD)":dbl=3.68631 format="%#_2p"
  out "Data points/scans":dbl=491508.0
  out "Data points/scan (f/b)":dbl=491508.0
  in  "Save scans":bool=TRUE
  out "AOD Scan I":u64 caption="Scan I"
  in  "Continuous AOD Scanning":bool caption="Continuous Scanning"
  in  "Abort AOD Scan":bool caption="Abort Scan"
  in  "Scan BD":bool=TRUE
  out "Cycles/step (AOD)":u64=666 format="%.3p"
  in  "Number of F/B Scans (AOD)":u16=1 min=1
  out "Scan steps (AOD)":u64=369
  out "Scan Increment (MHz)":dbl=-0.008152173913043485
  out "AOD Scanning":bool caption="Scanning"
  in  "Start AOD Scan":bool caption="Start Scan"
  out "N sets should be saved":dbl=24.5754
  out "Progress 2":u16(slide) caption="Progress" scale=0.0..100.0
  in  "Abort save 2":bool caption="Abort save"
  in  "Trap 1 Bead Size (nm)":dbl=2100.0
  in  "Trap 2 Bead Size (nm)":dbl=2100.0
  out "MCL Count":dbl=230502201.82069838
  in  "All FB On/Off":bool
  in  "AI2 to Setpoint":cluster{"Set 1":bool, "Set 2":bool}
  out "AI2 (V)":cluster{"Set 1":dbl, "Set 2":dbl}={"Set 1"=-0.0012207403790398877, "Set 2"=0.004577776421399579}
  in  "Reset Feedback":cluster{"Set 1":bool, "Set 2":bool}
  in  "PID Gains":T9={"Set 1"={"proportional gain (Kc)"=0, "integral gain (Kc*Ts/Ti)"=5, "derivative gain (Kc*Td/Ts)"=0}, "Set 2"={"proportional gain (Kc)"=0, "integral gain (Kc*Ts/Ti)"=5, "derivative gain (Kc*Td/Ts)"=0}}
  in  "Feedback On/Off":cluster{"Set 1":bool, "Set 2":bool}={"Set 1"=TRUE, "Set 2"=TRUE}
  in  "Set SP to Reading":bool
  out "Trap X (AI1)":T10={"Trap 1"=-1.0, "Trap 2"=0.899993896484375}
  in  "Trap Pos FB SP":fxp<+/-,16,1>=-0.092803955078125 caption="Setpoint"
  in  "Trap Pos. FB ON":bool
  in  "Reset Trap Pos. FB":bool
  out "Trap Positions":waveform(dbl)[](graph)=[{"t0"=timestamp(12.90000000000001 s since 1904-01-01), "dt"=0.15, "Y"=[-1.7479351299698465e-12, -1.7479351299698465e-12], "attributes"=variant("NI_ChannelName"=variant(string "Trap 1 Pos."))}, {"t0"=timestamp(12.90000000000001 s since 1904-01-01), "dt"=0.15, "Y"=[6.991740519879386e-12, 6.991740519879386e-12], "attributes"=variant("NI_ChannelName"=variant(string "Trap 2 Pos."))}]
  in  "Tab Control 8":enum32{"Main Setting", "Details"}(tab)
  in  "Trap Pos FB Int Count":u16=100
  in  "Trap Pos. FB Gains":T11={"proportional gain (Kc)"=10.0, "integral gain (Kc*Ts/Ti)"=10.0, "derivative gain (Kc*Td/Ts)"=0.0} {"proportional gain (Kc)" format="%.11g"; "integral gain (Kc*Ts/Ti)" format="%.11g"; "derivative gain (Kc*Td/Ts)" format="%.11g"}
  in  "Trap Pos. FB Offset Factor":i64
  in  "Trap Pos FB Negate Action":bool
  in  "Trap Pos. FB Mult Factor":i64=33554432
  in  "Trap Pos. AI1 X Pre-scale":u16
  in  "Trap Pos. FB Range":T12={"output high"=0.999969482421875, "output low"=-1.0}
  out "Trap Pos FB Int Signal":fxp<+/-,24,9> format="%.18g"
  out "Trap Pos FB Int-Norm Signal":fxp<+/-,16,1> format="%.16g"
  in  "Set SP Using...":bool
  in  "Trap Pos FB Monitor\nT1 or T2":bool
  out "Trap X AI1 (DMA)":T13={"Set 1"=0.999969482421875, "Set 2"=0.999969482421875}
  in  "N El. to Ave.":dbl=10000.0
  out "Trap Pos FB Action":i64
  out "Action (%)":dbl(knob) scale=-100.0..100.0
  in  "Trap Pos. FB Out Scale 2^n":u8=23 caption="Action Scale"
  out "Mean T1 Position (nm)":dbl=-1.7479351299698465e-12 caption="Mean T1 (nm)" format="%0.2f"
  out "Trap 1 Position RMS (A)":dbl caption="RMS (Ang)"
  in  "Tab Control 3":enum32{"Timing", "MCL Scan", "Analog Out"}(tab)
  out "APD 2 Gate Late Counter":u32
  out "APD 2 Gate Relative Phase":i16
  in  "Phase Adj. (APD 2 Gate)":i16=20
  in  "Initial Phase Adjustment (APD 2 Gate)":i16=55
  out "APD 1 Gate Late Counter":u32
  in  "- phase (APD 1 Gate)":bool
  in  "+ phase (APD 1 Gate)":bool
  out "APD 1 Gate Relative Phase":i16
  in  "Phase Adj. (APD 1 Gate)":i16=20
  in  "Initial Phase Adjustment (APD 1 Gate)":i16=60
  in  "Save APD Data\nwith Trap Data":bool=TRUE
  out "APD FIFO Elements Remaining":u32
  in  "- phase (APD Acq)":bool
  in  "+ phase (APD Acq)":bool
  out "APD Acq Late Counter":u32
  out "APD Acq Relative Phase":i16
  in  "Phase Adj. (APD Acq)":i16=20
  in  "Initial Phase Adjustment (APD Acq)":i16
  in  "Invert APD Gate":bool caption="Invert Gate"
  in  "APD Gate OFF Count":u32=450 caption="Gate OFF Count"
  in  "APD Gate ON Count":u32=150 caption="Gate ON Count"
  in  "APD Gate":enum32{"ON", "OFF", "Interlace"}(radio)=enum."Interlace"
  in  "APD Integration Time (s)":dbl=0.01 caption="Integration Time (s)"
  out "APD Acq Rate (Hz)":dbl=100.0 caption="Rate (Hz)"
  out "APD Samples/FIFO Acq.":dbl=30.0
  out "APD Elements/DMA read":u32=60
  out "APD Int. Count":u32=400000 format="%.0p"
  in  "+ phase (APD 2 Gate)":bool
  in  "- phase (APD 2 Gate)":bool
  in  "Tab Control 5":enum32{"PSD X", "PSD Y", "Other Data Channel"}(tab)
  out "Data map":dbl[][](graph)
  in  "Channel":i32=4
  in  "Abort MCL Scan":bool
  out "MCL Scan I":u64
  out "MCL Scanning":bool
  in  "Start MCL Scan":bool
  out "wait to reset values":bool
  in  "Tab Control 4":enum32{"Scan Settings", "MCL FPGA Loop Timing"}(tab)
  out "Total Time (s)":dbl=48.0
  in  "Scan lines (y)":u64=20
  in  "Fast Scan Dir":bool=TRUE
  in  "2D or 1D Scan":bool=TRUE
  out "Initial X":dbl
  out "Initial Y":dbl
  out "Time/f+b scan (s) (MCL)":dbl=2.4 caption="Time/scan (s)"
  in  "Number of scans (MCL)":u64=1 caption="Scans"
  in  "Scan steps (MCL)":u64=40 caption="Scan steps (x)"
  in  "N APD Samp/step":dbl=3.0
  in  "Scan Range (V)\n(of steps)":dbl=3.5
  in  "Restart DMA? (MCL)":bool=TRUE caption="Restart DMA?"
  in  "Continuous MCL Scanning":bool caption="Cont. Scanning"
  in  "Center Scan":bool=TRUE
  in  "Save Data (MCL)":bool=TRUE caption="Save Data"
  out "Actual Incr. int (MCL)":i16=294 caption="Incr. int"
  out "Desired incr (int)":dbl=294.0628205128205
  out "Desired Scan Incr (V)":dbl=0.08974358974358974
  out "N sets should be saved (MCL)":dbl=160.0 caption="N sets should be saved"
  out "Data points/scans (MCL)":dbl=4800.0 caption="Data points/scans"
  out "Data points/scan (f+b)":dbl=240.0 caption="points/scan (f+b)"
  out "Cycles/step (MCL)":u64=2000 caption="Cycles/step" format="%.0p"
  out "Actual MCL Inc (V)":dbl=0.08972441785943175
  in  "Phase adjust (MCL)":i16 caption="Phase adjust"
  out "Relative Phase (MCL)":i16 caption="Relative Phase"
  in  "Initial Phase Adj. (MCL)":i16 caption="Initial Phase Adj."
  in  "Update Count (MCL)":u32=600
  in  "+ phase (MCL)":bool
  in  "- phase (MCL)":bool
  out "MCL Late Counter":u32
  in  "APD 1 AO Mult.":i16=1 min=1
  in  "APD 2 AO Mult.":i16=1 min=1
  in  "Tab Control 7":enum32{"Green FB Signals", "Slow MCL Scan"}(tab)
  out "Green FB Plot":dbl(graph)=10.0
  out "MCL Scan 2":cluster{"Begin (V)":dbl, dbl, dbl[]}(graph)
  out "MCL Scan":cluster{"Begin (V)":dbl, dbl, dbl[]}(graph)
  in  "Green laser mode":enum32{"Laser ON", "Laser OFF", "Interlace"}(radio)
  in  "GI Frequency, ON count":u32=150 min=1 step=1
  in  "Invert GI":bool
  out "GI Late Counter":u32
  in  "Phase adj. (GI)":i16=5
  out "GI relative phase":i16
  in  "+ phase (GI)":bool
  in  "Initial Phase Adjustment (GI)":i16=19
  in  "GI Frequency, OFF count":u32=450 min=1 step=1
  in  "- phase (GI)":bool
  out "Green FB Signals (V)":cluster{"Y":dbl, "X":dbl, "Sum":dbl}={"Y"=1.0, "X"=1.0, "Sum"=10.0}
  out "Relative phase (Green FB)":i16
  in  "+ phase (Green FB)":bool
  in  "- phase (Green FB)":bool
  in  "Green FB Count":u32=600
  in  "Phase adj. (Green FB)":i16=10
  in  "Initial Phase Adjustment (Green FB)":i16=50
  in  "Green FB On/Off":bool
  in  "Current When FB OFF (%)":dbl=10.0 min=0.0 max=100.0 step=1.0
  in  "Green int current ON count adj":u32=150
  in  "Green FB Gains":T14={"proportional gain (Kc)"=10, "integral gain (Kc*Ts/Ti)"=5, "derivative gain (Kc*Td/Ts)"=0}
  in  "Green FB Setpoint (mV)":dbl=100.0
  in  "- phase (GI) 2":bool
  in  "Initial Phase Adjustment (GI) 2":i16=-100
  in  "+ phase (GI) 2":bool
  out "GI relative phase 2":i16
  in  "Phase adj. (GI) 2":i16=20
  out "GI Late Counter 2":u32
  in  "Trap Position FIFO Depth":u32=300000 format="%.0p"
  in  "# Samples/trap":u32=20000 format="%.0p"
  out "Trap AI Elements/DMA read":u32=320000 format="%.0p"
  out "Ave. Rate (Hz)":dbl=200000.0 format="%#_6p"
  out "Trap AI FIFO El. Rem.":u32 format="%.0p"
  in  "Phase adj. (AI1)":i16
  out "Relative phase (AI1)":i16
  in  "+ phase (AI1)":bool
  in  "- phase (AI1)":bool
  out "Late Counter (AI1)":u32
  in  "Initial Phase Adjustment (AI1)":i16=180
  out "AI rate (Hz)":dbl=200000.0 format="%#_6p"
  in  "AI Count (ticks)":u32=200
  out "# Samples/channel":u32=40000 format="%.0p"
  in  "Trap AI FIFO Depth":u32=340000 format="%.0p"
  in  "Detector Type":string(combo)="UCB Fleezers 052511"
  in  "N Acq Sets (Traps + Fl.)":i16=3
  in  "Sets to FIFO (Traps)":T15={"Set 1"=TRUE, "Set 2"=TRUE, "Set 3"=FALSE}
  in  "FPGA Ave.":dbl=1.0 min=1.0 step=1.0
  out "Ave. Period (s)":dbl=5e-06 format="%#_6p"
  out "DMA Update Period (s)":dbl=0.3
  out "FPGA Averaging":bool
  out "Trap Sets":u32=2
  out "Counts/DMA":dbl=12000000.0 format="%#_6p"
  out "Trap Pos FIFO El Remaining":u32=141
  out "Trap Pos Elements/DMA read":u32=120000 format="%.0p"
  out "Trap AI FIFO Timeout":u16
  out "Trap Pos FIFO Timeout":u16
  out "Waveform Chart":i32(graph)=320000
  out "error out 2":errorcluster
  in  "Lost Tether Alarm Threshold (pN)":dbl=0.5
  in  "AOM X Cal (nm/MHz)":dbl=168.33
  in  "MCL X Cal (nm/V)":dbl=1070.0
  out "X RF Amplitude Limits (%)":T16={"Minimum"=0.0, "Maximum"=50.0, "Increment"=1.0}
  out "X RF Frequency Limits (MHz)":T16={"Minimum"=50.0, "Maximum"=100.0, "Increment"=1.0}
  out "Y RF Frequency Limits (MHz)":T16={"Minimum"=50.0, "Maximum"=100.0, "Increment"=1.0}
  out "Y RF Amplitude Limits (%)":T16={"Minimum"=0.0, "Maximum"=50.0, "Increment"=1.0}
  in  "Manip. X?":bool=TRUE
  in  "Manip. Y?":bool
  in  "Force Manip Abort":bool
  out "Read cal error":errorcluster
  in  "DAQ Delay (ms)":u32=1000
  in  "Start Scan":bool
  in  "Scan axis":bool
  in  "Osc. amp. (V)":dbl=5.0
  in  "Osc. center (V)":dbl=5.0
  in  "Osc. freq. (Hz) 2":dbl=1.0
  in  "MCL Mode":u16(ring) items=["Manual Positioning", "Sinusoidal Wave", "Linear Scan"]
  in  "Begin (V)":dbl
  in  "End (V)":dbl=10.0
  in  "N Points":dbl=20.0
  in  "Delay to Interlace (s)":dbl
  in  "Delayed Interlace Start":bool
  in  "Read Lateness and Rel Phase":bool
  out "Vec Mean of T1 T2":dbl[](array[numeric])=[nan, nan]
  in  "Cal read wait (s)":u32=5
  out "Time tether formed":timestamp=timestamp(3371146929.513132 s since 1904-01-01)
  in  "Chemyx Syringe Pump Serial Port":refnum<visa-resource-name>="ASRL3::INSTR"
  in  "Limit Min (MHz)":dbl=10.0 caption="Min (MHz)"
  in  "Limit Max (MHz)":dbl=16.0 caption="Max (MHz)"
  in  "Limits Enable":bool=TRUE caption="Enable"
  out "AI labels":string[](array[string])=["T1 Y", "T1 X", "T1 Sum", "T2 Y", "T2 X", "T2 Sum", "T1 FB X", "T2 FB Sum", "T2 FB X", "T2 FB Sum", "PSD Y", "PSD X", "PSD Sum"]
  in  "Save Trap Pos. Data":bool=TRUE
  in  "ESP Port":refnum<visa-resource-name>="COM22"
  in  "Locations":i32(listbox)=1
  out "Selected Location":cluster{"x":string, "y":string, "z":string}={"x"="0.19233\r\n", "y"="0.00156\r\n", "z"="0.20615\r\n"}
  in  "Capture":bool
  in  "Save":bool
  in  "Goto Top (F6)":bool
  in  "Goto Exp (F8)":bool
  in  "Goto Bottom (F7)":bool
  in  "Axis 3":string="0.00500\r\n"
  in  "Axis 2":string="0.00500\r\n"
  in  "Axis 1":string="0.00500\r\n"
  in  "Axis 3":string="0.20000\r\n"
  in  "Axis 2":string="0.20000\r\n"
  in  "Axis 1":string="0.20000\r\n"
  in  "Activate Joystick":bool
  in  "ESP ZL-Limit":string="-0.09900"
  in  "ESP ZR-Limit":string="0.09900"
  out "Z Pos Pos":string="0.21899\r\n"
  out "Y Pos":string="0.00713\r\n"
  out "X Pos":string="0.20503\r\n"
  in  "error in":errorcluster
  out "error out":errorcluster
  # "After"
  # "During"
  # "Trap On?"
  # "BD Flow ON?"
  # "Samp Flow ON?"
  # "1"
  # "2"
  # "Trap Display:"
  # "APD Display:"
  # "originally 10k"
  # "Trap Manipulation"
  # "DAQ"
  # "Data Saving"
  # "F9"
  # "Bead Calibration"
  # "F10"
  # "F4"
  # "Press F12 to move stage\nwith the mouse. F12 to cancel."
  # "F5"
  # "F6"
  # "F7"
  # "F8"
  # "Harvard Pump\n(sample channel for flow exp)"
  # "Chemyx Pump 2"
  # "Units: \n1 = ml/m\n2 = ml/h\n3 = ul/m\n4 = ul/h"
  # "Rate param is ul/h\nVolume param is ul"
  # "X"
  # "Y"
  # "Oscillate Set 2 freq. (debugging)"
  # "BD 1"
  # "BD 2"
  # "AOD Raster Scan"
  # "Approx. trap separations"
  # "X"
  # "Y"
  # "DON'T TURN ON\nUNTIL YOU CLOSE\nTHE LOOP"
  # "FPGA\nreading"
  # "DMA\ntransfer"
  # "APD Gates"
  # "APD 2"
  # "APD 1"
  # "X"
  # "2D"
  # "Y"
  # "1D"
  # "Green Laser Interlacing"
  # "Green FB Measurement"
  # "Digital Gate"
  # "Current Analog Control"
  # "was 87"
  # "originally 600k"
  # "Total AI Rates (NOT rates/trap)"
  # "originally 20k"
  # "(Samples/trap x Trap Sets)"
  # "(Samples/channel x\n8 if averaging (8 channels)\n4 if no averaging)"
  # "Trap 1"
  # "Trap 2"
  # "Flour./Trap 3"
  # "External Video Window"
  # "MCL Position Debugging"
  # "Temporary Control Storage\n(these used to be somewhere else, still want to keep them)"
  # "Y"
  # "X"
  # "Trap Position Difference Limits"
  # "Joystick Control"
  # "Setting Limit for the z-axis"
  # "Current Location"
  # "Save Positions of Cambers"
  # "Errors detected in determing Current Location"
  # "High Jog Velocity"
  # "Low Jog Velocity"
  # "Select the chamber to go to"
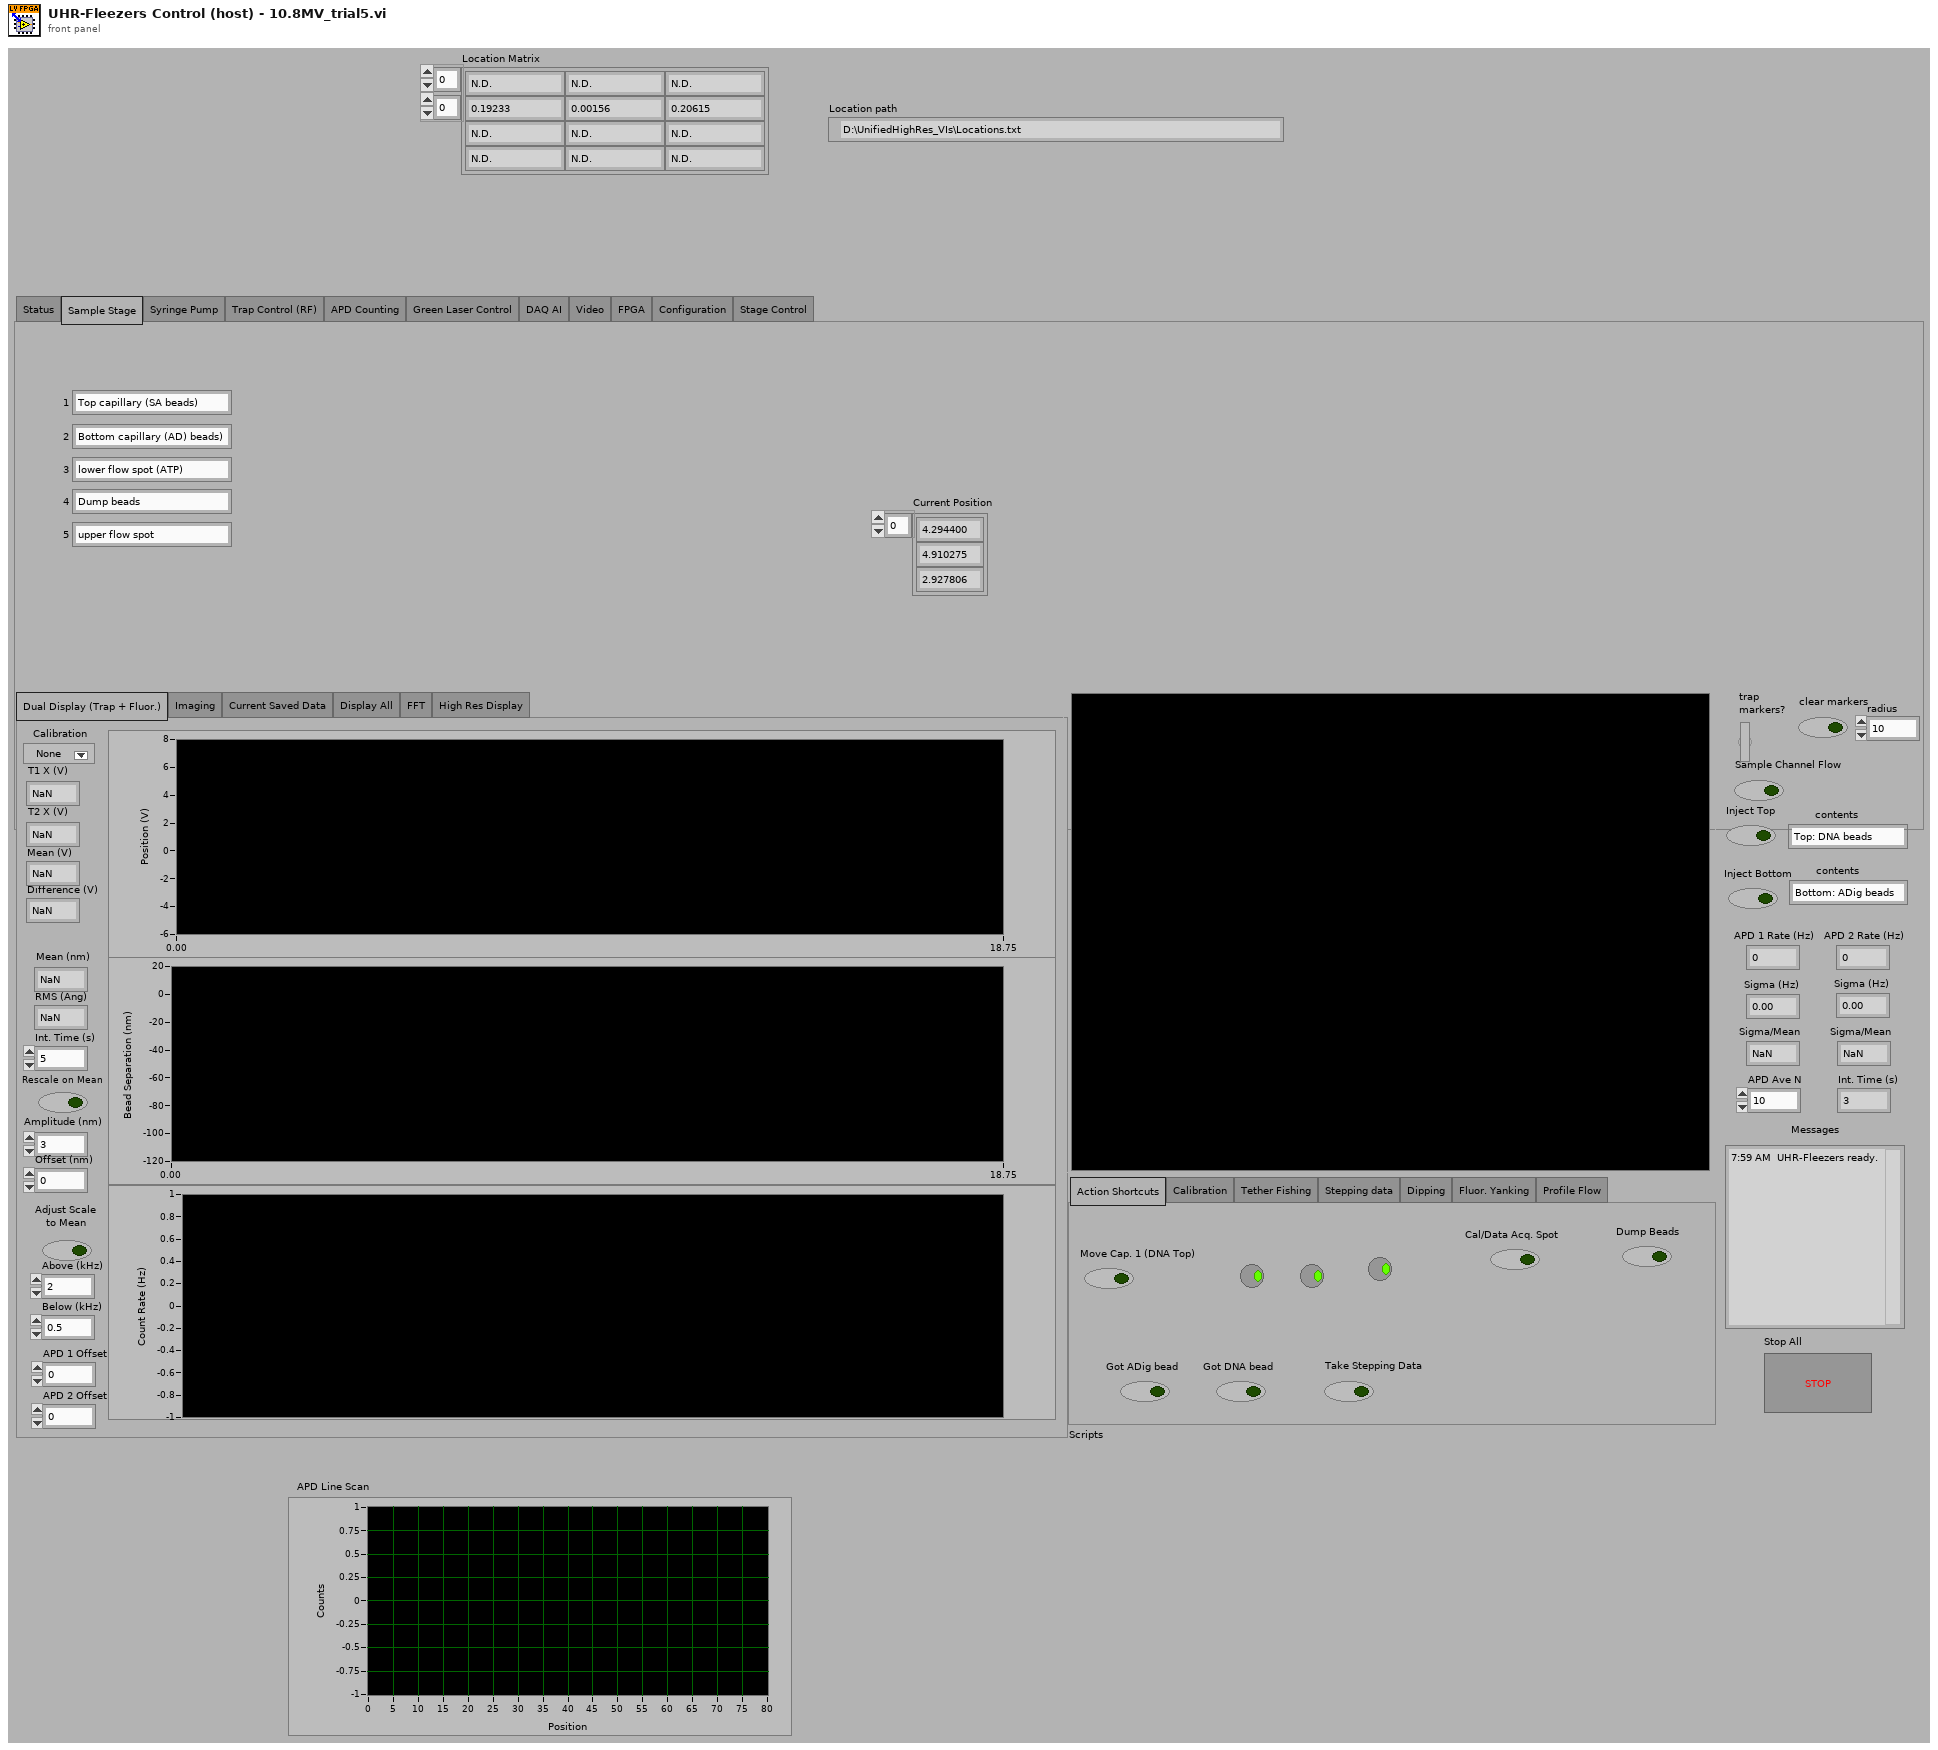
[diagram p1: front panel]
types:
  T1 = enum32{"Action Shortcuts", "Calibration", "Tether Fishing", "Stepping data", "Dipping", "Fluor. Yanking", "Profile Flow"}
  T2 = typedef "IMAQ Image.ctl" = refnum<image>
  T3 = enum32{"Dual Display (Trap + Fluor.)", "Imaging", "Current Saved Data", "Display All", "FFT", "High Res Display"}
  T4 = enum32{"Status", "Sample Stage", "Syringe Pump", "Trap Control (RF)", "APD Counting", "Green Laser Control", "DAQ AI", "Video", "FPGA", "Configuration", "Stage Control"}
  T5 = cluster{"Pump 1":cluster{"Diameter (mm)":dbl, "Units":dbl, "Volume":dbl, "Rate":dbl}, "Pump 2":cluster{"Diameter (mm)":dbl, "Units":dbl, "Volume":dbl, "Rate":dbl}, "Pump 3":cluster{"Diameter (mm)":dbl, "Units":dbl, "Volume":dbl, "Rate":dbl}}
  T6 = enum32{"IR Laser Interlacing (Direct RF Board Control Method)", "AOD Raster Scan", "Feedback on Trap Intensity", "Feedback on Trap Position"}
  T7 = typedef "LVPoint32TypeDef.ctl" = cluster{"Horizontal":i32, "Vertical":i32}
  T8 = cluster{"Scan Range AOD (nm) 2":dbl, "Step Size AOD (nm) 2":dbl, "Scan Speed AOD (nm/s) 2":dbl, "Number of scans (AOD) 2":u16, "Label":string}[]
  T9 = cluster{"Set 1":cluster{"proportional gain (Kc)":i16, "integral gain (Kc*Ts/Ti)":i16, "derivative gain (Kc*Td/Ts)":i16}, "Set 2":cluster{"proportional gain (Kc)":i16, "integral gain (Kc*Ts/Ti)":i16, "derivative gain (Kc*Td/Ts)":i16}}
  T10 = cluster{"Trap 1":fxp<+/-,16,1>, "Trap 2":fxp<+/-,16,1>}
  T11 = cluster{"proportional gain (Kc)":fxp<+/-,16,8>, "integral gain (Kc*Ts/Ti)":fxp<+/-,16,8>, "derivative gain (Kc*Td/Ts)":fxp<+/-,16,8>}
  T12 = cluster{"output high":fxp<+/-,16,1>, "output low":fxp<+/-,16,1>}
  T13 = cluster{"Set 1":fxp<+/-,16,1>, "Set 2":fxp<+/-,16,1>}
  T14 = cluster{"proportional gain (Kc)":i16, "integral gain (Kc*Ts/Ti)":i16, "derivative gain (Kc*Td/Ts)":i16}
  T15 = cluster{"Set 1":bool, "Set 2":bool, "Set 3":bool}
  T16 = typedef "LVMinMaxIncTypeDef.ctl" = cluster{"Minimum":dbl, "Maximum":dbl, "Increment":dbl}
  T17 = typedef "Image Type" = u32
  T18 = typedef "nirio_resource_hc.ctl" = tag
  T19 = typedef "openfpgaref.8.6.ctl" = refnum<k20>
  T20 = enum16{"CONNECT", "INITIALIZE VALVES", "DISCONNECT", "MOVE VALVE"}
  T21 = cluster{"New Image":T2, "New Image":T2, "New Image":T2, "New Image":T2}
  T22 = cluster{"Location Matrix[0]":string, "Location Matrix[1]":string, "Location Matrix[2]":string}
  T23 = enum16{"open", "replace", "create", "open or create", "replace or create", "replace or create with confirmation"}
  T24 = typedef "XDNodeRunTimeDep.lvlib/timing_clust.ctl" = cluster{"Expected End [f-1]":u64, "Actual End [f-1]":u64, "Finished Late? [f-1]":bool, "Expected End [i-1]":u64, "Actual End [i-1]":u64, "Finished Late? [i-1]":bool, "Expected Start [i]":u64, "Actual Start [i]":u64, "Expected Start [f]":u64, "Actual Start [f]":u64, "Source Name":string, "Structure Name":string, "Period":i64, "Deadline":i64, "Offset":i64, "Start":i64, "Priority":i32, "Timeout":i32, "Mode":T25, "Wakeup Reason":T26, "Error":errorcluster, "Source Type":string, "Secondary Source Type":string, "Global End Time":u64, "Global Start Time":u64, "Frame Duration":u64, "Iteration Duration":u64, "Assigned CPU":i32, "I/O Scan Engine Mode":u32}
  T25 = typedef "XDNodeRunTimeDep.lvlib/nitl_modes.ctl" = enum32{"No Change", "Process missed periods, maintain original phase", "Discard missed periods, maintain original phase", "Process missed periods, ignore original phase", "Discard missed periods, ignore original phase"}
  T26 = typedef "XDNodeRunTimeDep.lvlib/wakeup.ctl" = enum32{"Normal", "Aborted", "Asynchronous wakeup", "Timing source error", "Timed loop error", "Timeout"}
  T27 = cluster{"[0]":i32, "[1]":i32, "[2]":i32, "[3]":i32}
  T28 = cluster{"[0]":i32, "[1]":i32, "[2]":i32, "[3]":i32}[]
  T29 = enum16{"big-endian, network order", "native, host order", "little-endian"}
  T30 = cluster{"Scan Range AOD (nm) 2":dbl, "Step Size AOD (nm) 2":dbl, "Scan Speed AOD (nm/s) 2":dbl, "Number of scans (AOD) 2":u16, "Label":string}
  T31 = cluster{"[0]":dbl, "[1]":dbl, "[2]":dbl, "[3]":dbl, "[4]":dbl, "[5]":dbl}
  T32 = cluster{"Diameter (mm)":dbl, "Units":dbl, "Volume":dbl, "Rate":dbl}
  T33 = cluster{"Left":i32, "Top":i32, "Width":u32, "Height":u32}
  T34 = cluster{cluster{"Left":i32, "Top":i32, "Width":u32, "Height":u32}}[]
  T35 = enum32{"Normal Display", "Dual Display (APD)", "FFT", "High Res Display"}
  T36 = cluster{"Origin Pixel":cluster{"X":sgl, "Y":sgl}, "Angle Relative to Horizontal (deg)":sgl, "Axis Reference":u32}
  T37 = typedef "Simple Grid Descriptor" = cluster{"X Step":sgl, "Y Step":sgl, "Unit":T38}
  T38 = typedef "Image Unit" = enum32{"Undefined", "Angström", "Micrometer", "Millimeter", "Centimeter", "Meter", "Kilometer", "Microinch", "Inch", "Feet", "Nautical miles", "Standard miles", "Steps"}
  T39 = cluster{"averaging mode":u16, "weighting mode":u16, "number of averages":u32}
  T40 = cluster{"dB On (F)":bool, "unwrap phase (F)":bool, "convert to degree (F)":bool}
  T41 = cluster{string, string, string, string, string, string, string, string}
  T42 = cluster{string, string, string, string, string, string, string, string, string, string, string, string}
  T43 = cluster{string, string, string, string, string, string, string, string, string, string, string, string, string}
  T44 = cluster{string, string, string, string, string, string, string, string, string, string, string, string, string, string}
  T45 = cluster{"BD 1 Frequency 1 (MHz)":dbl, "BD 1 Frequency 2 (MHz)":dbl}
  T46 = cluster{"f0":dbl, "df":dbl, "magnitude":dbl[]}[][]
  T47 = cluster{"Green FB Ch 0":i16, "Green FB Ch 1":i16, "Green FB Ch 2":i16}
  T48 = cluster{"Green FB Ch 0":dbl, "Green FB Ch 1":dbl, "Green FB Ch 2":dbl}
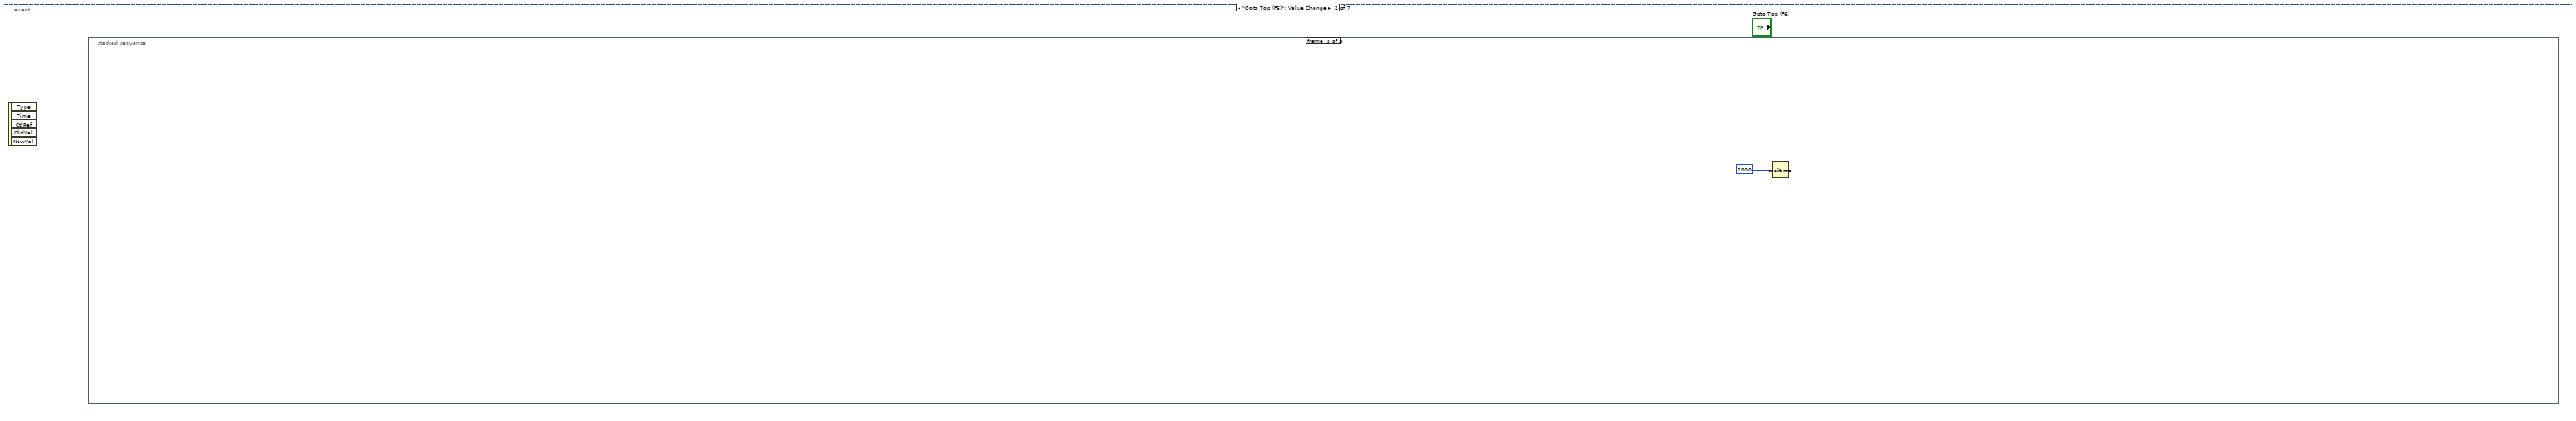
[diagram p4: hidden frame]
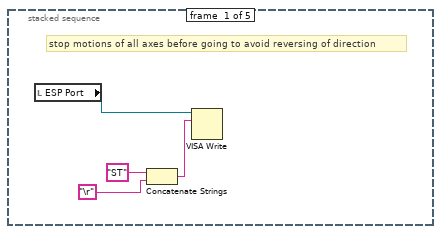
[diagram p5: hidden frame]
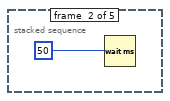
[diagram p6: hidden frame]
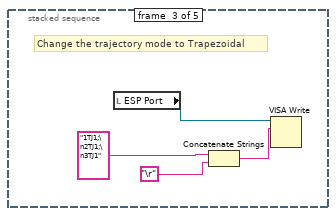
[diagram p7: hidden frame]
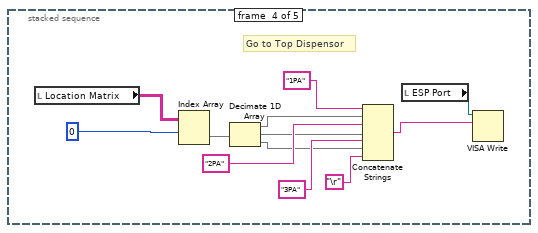
[diagram p8: hidden frame]
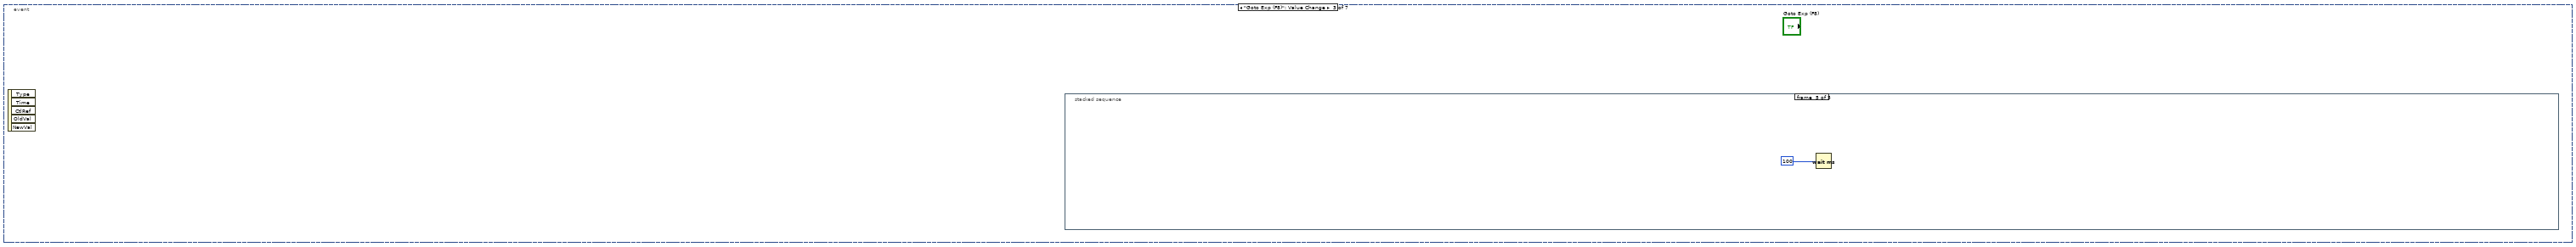
[diagram p9: hidden frame]
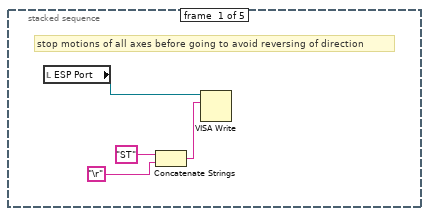
[diagram p10: hidden frame]
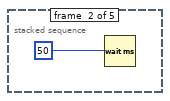
[diagram p11: hidden frame]
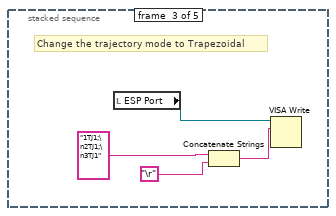
[diagram p12: hidden frame]
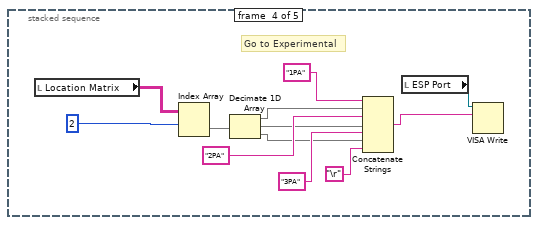
[diagram p13: hidden frame]
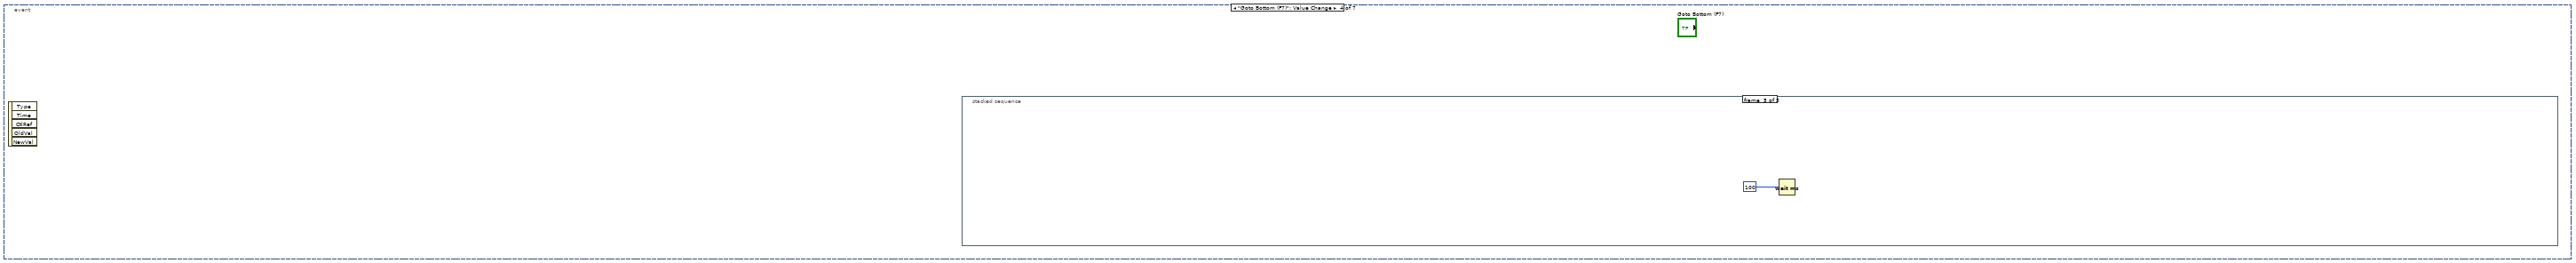
[diagram p14: hidden frame]
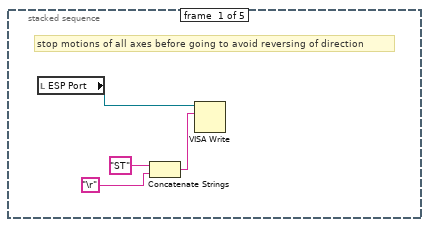
[diagram p15: hidden frame]
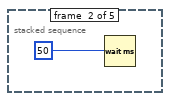
[diagram p16: hidden frame]
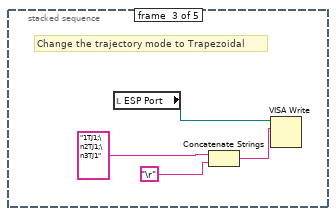
[diagram p17: hidden frame]
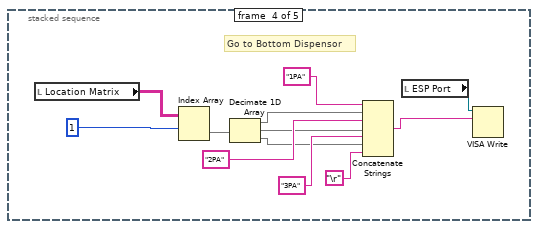
[diagram p18: hidden frame]
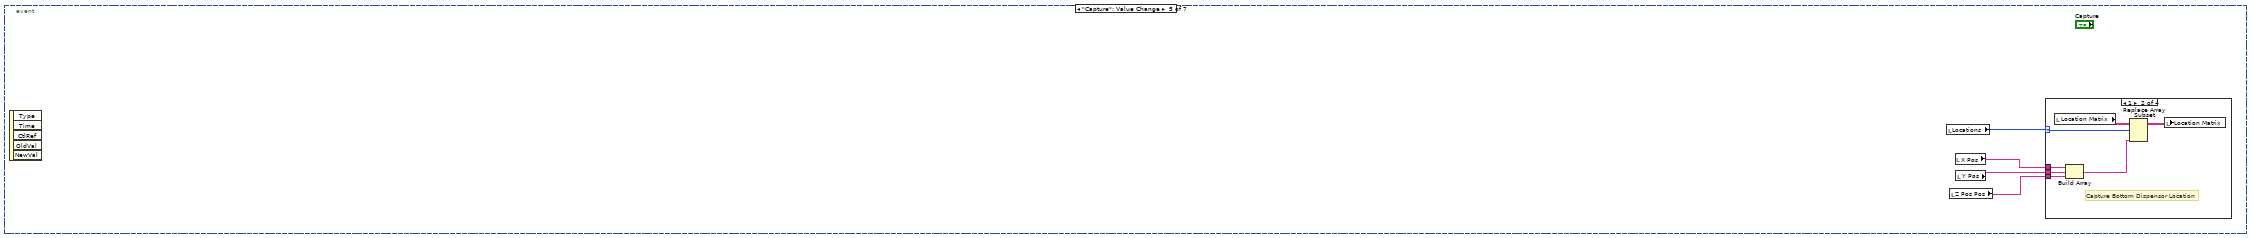
[diagram p19: hidden frame]
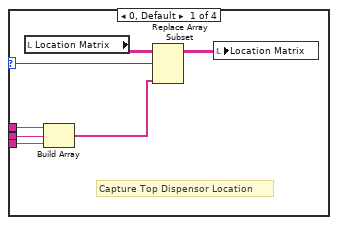
[diagram p20: hidden frame]
diagram:
  w64 = T17 2 items=["Grayscale (U8)", "Grayscale (I16)", "Grayscale (SGL)", "Complex (CSG)", "RGB (U32)", "HSL (U32)", "RGB (U64)", "Grayscale (U16)"] ("Image Type")
  w121 = cluster{"output high":i16, "output low":i16} {"output high"=3000, "output low"=0} ("FB output range 1")
  w196 = 10.0 ("y")
  w195 = 32767.0 ("y")
  w211 = 6.0  # clock mult.
  w212 = 49152000.0  # TCXO frequ.
  # "Initialize location matrix"
  n1 = Build Array("DIO count 1 (ticks)", "DIO count 2 (ticks)", "DIO count 3 (ticks)") -> (w110:u32[])
  n2 = Multiply(x="APD Integration Time (s)", y=40000000.0) -> (x*y=w128:dbl)
  n3 = Reciprocal(x="APD Integration Time (s)") -> (1/x=w125:dbl)
  n4 = local write "APD Acq Rate (Hz)"(w125) -> ()
  n5 = local read "AO1"() -> (w190:dbl)
  n6 = local read "AO2"() -> (w189:dbl)
  n7 = To Unsigned Long Integer(number=w128) -> (unsigned 32bit integer=w127:u32)
  "APD Int. Count" <- w127
  n8 = local read "Scan Increment (MHz)"() -> (w207:dbl)
  n9 = local read "Continuous MCL Scanning"() -> (w177:bool)
  n10 = local read "Fast Scan Dir"() -> (w176:bool)
  n11 = local read "Trap Intensity\nSetpoints (V)"() -> (w226:cluster{"Set 1":dbl, "Set 2":dbl})
  n12 = local read "Number of scans (MCL)"() -> (w178:u64)
  n13 = Multiply(x=w190, y=w195) -> (x*y=w192:dbl)
  n14 = Multiply(x=w189, y=w195) -> (x*y=w194:dbl)
  n15 = Divide(x=w192, y=w196) -> (x/y=w191:dbl)
  n16 = Divide(x=w194, y=w196) -> (x/y=w193:dbl)
  n17 = To Word Integer(number=w191) -> (16bit integer=w188:i16)
  n18 = To Word Integer(number=w193) -> (16bit integer=w187:i16)
  n19 = Not(x=w176) -> (.not. x?=w171:bool)
  n20 = local read "Cycles/step (MCL)"() -> (w179:u64)
  n21 = Multiply(x=w207, y=1000.0) -> (x*y=w214:dbl)
  n22 = local read "Scan steps (MCL)"() -> (w180:u64)
  n23 = local write "Trap Pos FIFO Timeout"(u16 0 ("Trap Pos FIFO Timeout")) -> ()
  n24 = local read "Desired Scan Incr (V)"() -> (w182:dbl)
  n25 = Scale By Power Of 2(n=48, x=w214) -> (x*2^n=w215:dbl)
  n26 = Multiply(x=w212, y=w211) -> (x*y=w210:dbl)
  n27 = Divide(x=w215, y=w210) -> (x/y=w209:dbl)
  n28 = local read "Number Interlace Sets"() -> (w103:u8)
  n29 = Split 1D Array(array=w110, index=w103) -> (first subarray=w112:u32[])  [unwired: 1 out]
  n30 = Add Array Elements(numeric array=w112) -> (sum=w111:u32)
  n31 = property on="AI Count (ticks)" class="DigNum (strict)"("Val(Sgnl)"="AI Count (ticks)") -> ()  [unwired: 2 in, 2 out]
  n32 = local read "# Samples/channel"() -> (w199:u32)
  n33 = local read "Number of F/B Scans (AOD)"() -> (w200:u16)
  n34 = To Quad Integer(1:w209) -> (0:w206:i64)
  n35 = local read "Not-Interlacing Set"() -> (w102:enum32{"Set 1", "Set 2", "Set 3"})
  n36 = To Unsigned Byte Integer(number=w102) -> (unsigned 8bit integer=w108:u8)
  n37 = Index Array(array=w110, index=w108) -> (element=w109:u32)
  n38 = local read "Feedback On/Off"() -> (w229:cluster{"Set 1":bool, "Set 2":bool})
  n39 = local read "PID Gains"() -> (w221:T9)
  n40 = Divide(x=40000000.0, y="AI Count (ticks)") -> (x/y=w168:dbl)
  n41 = Multiply(x=w182, y=32767.0) -> (x*y=w184:dbl)
  n42 = local read "Scan steps (AOD)"() -> (w205:u64)
  n43 = local read "All FB On/Off"() -> (w230:bool)
  n44 = local read "Cycles/step (AOD)"() -> (w204:u64)
  n45 = local write "AI rate (Hz)"(w168) -> ()
  n46 = Divide(x=w184, y=10.0) -> (x/y=w183:dbl)
  n47 = Multiply(x=w205, y=w204) -> (x*y=w203:u64)
  n48 = Multiply(x=3276.7, y=w226) -> (x*y=w225:cluster{"Set 1":dbl, "Set 2":dbl})
  n49 = To Word Integer(number=w183) -> (16bit integer=w181:i16)
  n50 = Multiply(x=w203, y=u64 2) -> (x*y=w201:u64)
  n51 = local read "Sets to FIFO (Traps)"() -> (w233:T15)
  n52 = Divide(x=w168, y="FPGA Ave.") -> (x/y=w169:dbl)
  n53 = To Word Integer(number=w225) -> (16bit integer=w224:cluster{"Set 1":i16, "Set 2":i16})
  n54 = xnode "Open FPGA VI Reference"("resource name"=T18 "750kHzDAQ") -> ("FPGA VI Reference Out"=w218:T19)  [unwired: 1 in, 1 out]
  n55 = Unbundle By Name(w221) -> ("Set 1"=w220:T14, "Set 2"=w219:T14)
  n56 = Multiply(x=w201, y=w200) -> (x*y=w198:u64)
  n57 = local write "Ave. Rate (Hz)"(w169) -> ()
  n58 = Divide(x=w198, y=w199) -> (x/y=w197:dbl)
  n59 = Unbundle By Name(w224) -> ("Set 1"=w223:i16, "Set 2"=w222:i16)
  n60 = local read "2D or 1D Scan"() -> (w122:bool)
  n61 = local write "Data points/scans"(w198) -> ()
  n62 = local read "Scan BD"() -> (w216:bool)
  n63 = And(x=w229, y=w230) -> (x .and. y?=w228:cluster{"Set 1":bool, "Set 2":bool})
  n64 = local write "Data points/scan (f/b)"(w201) -> ()
  n65 = Reciprocal(x=w169) -> (1/x=w170:dbl)
  n66 = local read "N Acq Sets (Traps + Fl.)"() -> (w161:i16)
  n67 = local write "N sets should be saved"(w197) -> ()
  n68 = Unbundle By Name(w228) -> ("Set 1"=w232:bool, "Set 2"=w231:bool)
  n69 = local read "Interlace"() -> (w104:bool)
  n70 = Select(t=w111, s=w104, f=w109) -> (s? t:f=w101:u32)
  n71 = local write "Update Count (MCL)"(w101) -> ()
  n72 = local write "Total Counts (ticks)"(w101) -> ()
  n73 = xnode "Invoke Method"("FPGA VI Reference In"=w218) -> ("FPGA VI Reference Out"=w120:T19, "error out"=w139:errorcluster)  [unwired: 1 in]
  n74 = local write "Ave. Period (s)"(w170) -> ()
  n75 = property on="2D or 1D Scan" class="Bool (strict)"("Val(Sgnl)"=w122) -> ()  [unwired: 2 in, 2 out]
  n76 = xnode "Read/Write Control"("FPGA VI Reference In"=w119, "error in"=w139, "ai count"="AI Count (ticks)", "Interlace ON/OFF"=w104, "Number Interlace Cycles"=w103, "AI1 Sets to FIFO"=w233, "FB On/Off Set 1"=w232, "FB On/Off Set 2"=w231, "Interlace Off Parameters"=w102, "FB Setpoint Set 1"=w223, "FB Setpoint Set 2"=w222, "FB Gains Set 1"=w220, "FB Gains Set 2"=w219, "FB output range 1"=w121, "FB output range 2"=w121, "Cycles per step"=w204, "Scan BD"=w216, "Number of scans"=w200, "Scan steps"=w205, "Scan freq.  increment"=w206, "AO1"=w188, "AO2"=w187, "Scan freq.  increment (MCL)"=w181, "Scan steps (MCL)"=w180, "Cycles per step (MCL)"=w179, "Number of scans (MCL)"=w178, "MCL count"=w101, "Cont. Scan (MCL)"=w177, "MCL Scan Axis"=w171, "1D or 2D Scan?"=w122, "N of AI1 Int Acq Sets"=w161, "Freq or Amp switch first"="Freq or Amp switch first", "Freq switch delay"="Freq switch delay", "Amp switch delay"="Amp switch delay", "Swap F1 and F2"="Swap F1 and F2", "APD Acq Rate Count"=w127, "APD to FIFO"=FALSE, "APD Gate Operating Mode"="APD Gate", "APD Gate ON Count"="APD Gate ON Count", "APD Gate OFF Count"="APD Gate OFF Count", "Invert APD Gate"="Invert APD Gate", "DIO count 1 (ticks)"="DIO count 1 (ticks)", "DIO count 2 (ticks)"="DIO count 2 (ticks)", "DIO count 3 (ticks)"="DIO count 3 (ticks)", "APD 1 AO scale factor"="APD 1 AO Mult.", "APD 2 AO scale factor"="APD 2 AO Mult.") -> ("FPGA VI Reference Out"=w96:T19, "error out"=w98:errorcluster)  [unwired: 1 in]
  n77 = local read "Green Laser ON/Interlacing"() -> (w99:bool)
  n78 = local read "Green laser mode"() -> (w100:enum32{"Laser ON", "Laser OFF", "Interlace"})
  n79 = local read "GI Frequency, OFF count"() -> (w92:u32)
  n80 = local read "GI Frequency, ON count"() -> (w91:u32)
  n81 = Multiply(x="Current When FB OFF (%)", y=655.35) -> (x*y=w82:dbl)
  n82 = local read "Green FB Count"() -> (w90:u32)
  n83 = Multiply(x="Green FB Setpoint (mV)", y=3.2767) -> (x*y=w79:dbl)
  n84 = To Unsigned Word Integer(number=w82) -> (unsigned 16bit integer=w80:u16)
  n85 = local read "Invert GI"() -> (w94:bool)
  n86 = To Word Integer(number=w79) -> (16bit integer=w77:i16)
  n87 = case shown="True" w99 {
    tunnel: w100 -> [_ w253]
    tunnel: [enum32{"Laser ON", "Laser OFF", "Interlace"}."Laser OFF" ("Green laser mode") w253] -> w93
    frame False {
    }
    frame True {
    }
  }
  n88 = local read "Trap Pos. AI1 X Pre-scale"() -> (w48:u16)
  n89 = local read "Trap Pos FB Monitor\nT1 or T2"() -> (w55:bool)
  n90 = local read "Trap Pos FB Int Count"() -> (w43:u16)
  n91 = local read "Trap Pos FB Negate Action"() -> (w54:bool)
  n92 = local read "Trap Pos. FB Offset Factor"() -> (w53:i64)
  n93 = local read "Trap Pos. FB Mult Factor"() -> (w52:i64)
  n94 = local read "Trap Pos. FB Gains"() -> (w50:T11)
  n95 = local read "Trap Pos. FB Range"() -> (w51:T12)
  n96 = xnode "Read/Write Control"("FPGA VI Reference In"=w96, "error in"=w98, "Green interlace ON count 2"=w91, "Green interlace OFF count 2"=w92, "Invert GI 2"=w94, "Operating Mode 2"=w93, "Green FB Gains"="Green FB Gains", "Green FB Setpoint"=w77, "Green FB On/Off"="Green FB On/Off", "Current Out"=w80, "Green int current ON count adj"="Green int current ON count adj", "Green FB Count"=w90, "Operating Mode"=w93, "Green interlace OFF count"=w92, "Green interlace ON count"=w91, "Invert GI"=w94, "Trap Pos FB Monitor T1 or T2"=w55, "Trap Pos FB Negate Action"=w54, "Trap Pos. FB Offset Factor"=w53, "Trap Pos. FB Mult Factor"=w52, "Trap Pos. FB Range"=w51, "Trap Pos. FB Gains"=w50, "Force feedback"=FALSE, "AI1 X Scale"=w48, "Trap Pos to FIFO"=TRUE, "Trap Pos FB Int Count"=w43) -> ("FPGA VI Reference Out"=w95:T19, "error out"=w97:errorcluster)
  n97 = xnode "Invoke Method"("FPGA VI Reference In"=w95, "error in"=w97, "Requested Depth"="Trap AI FIFO Depth") -> ("FPGA VI Reference Out"=w58:T19, "error out"=w57:errorcluster)  [unwired: 1 out]
  n98 = xnode "Invoke Method"("FPGA VI Reference In"=w58, "error in"=w57, "Requested Depth"="Trap Position FIFO Depth") -> ("FPGA VI Reference Out"=w45:T19, "error out"=w44:errorcluster)  [unwired: 1 out]
  n99 = flat-sequence {
    tunnel: w120 -> [w258]
    tunnel: [w258] -> w119
    tunnel: [w257] -> w118
    tunnel: [w256] -> w117
    tunnel: [w254] -> w115
    tunnel: [w255] -> w116
    frame #0 {
      w255 = T16 {"Minimum"=50.0, "Maximum"=100.0, "Increment"=1.0} ("Min Max Inc")
      w254 = T16 {"Minimum"=0.0, "Maximum"=75.0, "Increment"=1.0} ("Data Entry Limits")
      w257 = T16 {"Minimum"=50.0, "Maximum"=100.0, "Increment"=1.0} ("Min Max Inc")
      w256 = T16 {"Minimum"=0.0, "Maximum"=75.0, "Increment"=1.0} ("Data Entry Limits")
      n100 = property on="BD 2 Frequency 1 (MHz)" class="DigNum (strict)"("Data Range"=w255) -> ()  [unwired: 2 in, 2 out]
      n101 = property on="BD 2 Frequency 3 (MHz)" class="DigNum (strict)"("Data Range"=w255) -> ()  [unwired: 2 in, 2 out]
      n102 = property on="BD 2 Frequency 2 (MHz)" class="DigNum (strict)"("Data Range"=w255) -> ()  [unwired: 2 in, 2 out]
      n103 = property on="BD 1 Frequency 1 (MHz)" class="DigNum (strict)"("Data Range"=w257) -> ()  [unwired: 2 in, 2 out]
      n104 = property on="BD 1 Frequency 2 (MHz)" class="DigNum (strict)"("Data Range"=w257) -> ()  [unwired: 2 in, 2 out]
      n105 = property on="BD 1 Frequency 3 (MHz)" class="DigNum (strict)"("Data Range"=w257) -> ()  [unwired: 2 in, 2 out]
      n106 = property on="BD 2 Amplitude 1 (%)" class="DigNum (strict)"("Data Range"=w254) -> ()  [unwired: 2 in, 2 out]
      n107 = property on="BD 2 Amplitude 2 (%)" class="DigNum (strict)"("Data Range"=w254) -> ()  [unwired: 2 in, 2 out]
      n108 = property on="BD 2 Amplitude 3 (%)" class="DigNum (strict)"("Data Range"=w254) -> ()  [unwired: 2 in, 2 out]
      n109 = property on="BD 1 Amplitude 3 (%)" class="DigNum (strict)"("Data Range"=w256) -> ()  [unwired: 2 in, 2 out]
      n110 = property on="BD 1 Amplitude 2 (%)" class="DigNum (strict)"("Data Range"=w256) -> ()  [unwired: 2 in, 2 out]
      n111 = property on="BD 1 Amplitude 1 (%)" class="DigNum (strict)"("Data Range"=w256) -> ()  [unwired: 2 in, 2 out]
      "X RF Frequency Limits (MHz)" <- w257
      "X RF Amplitude Limits (%)" <- w256
      "Y RF Amplitude Limits (%)" <- w254
      "Y RF Frequency Limits (MHz)" <- w255
    }
  }
  n112 = xnode "Invoke Method"("FPGA VI Reference In"=w45, "error in"=w44) -> ("FPGA VI Reference Out"=w22:T19, "error out"=w21:errorcluster)  [unwired: 1 in]
  n113 = flat-sequence "Initial FPGA Loop Relative Phase Adjustment" {
    tunnel: "Initial Phase Adjustment (APD 2 Gate)" -> [w260]
    tunnel: "Initial Phase Adjustment (GI) 2" -> [w261]
    tunnel: "Initial Phase Adj. (MCL)" -> [w262]
    tunnel: w21 -> [w263]
    tunnel: w22 -> [w264]
    tunnel: "Initial Phase Adjustment (GI)" -> [w265]
    tunnel: "Initial Phase Adjustment (AI1)" -> [w266]
    tunnel: [w266] -> w31
    tunnel: [w265] -> w30
    tunnel: [w264] -> w29
    tunnel: [w263] -> w28
    tunnel: [w262] -> w27
    tunnel: [w261] -> w26
    tunnel: [w260] -> w25
    tunnel: [w278] -> w145
    tunnel: [w272] -> w143
    tunnel: "Initial Phase Adjustment (APD Acq)" -> [w271]
    tunnel: "Initial Phase Adjustment (APD 1 Gate)" -> [w270]
    tunnel: "Initial Phase Adjustment (Green FB)" -> [w269]
    tunnel: w31 -> [w277]
    tunnel: w30 -> [w276]
    tunnel: w29 -> [w275]
    tunnel: w28 -> [w274]
    tunnel: w27 -> [w273]
    tunnel: w26 -> [w268]
    tunnel: w25 -> [w267]
    tunnel: w145 -> [w280]
    tunnel: [w281] -> w144
    tunnel: w143 -> [w281]
    tunnel: [w280] -> w142
    tunnel: w144 -> [w284]
    tunnel: w142 -> [w283]
    tunnel: [w286] -> w141
    tunnel: [w285] -> w140
    tunnel: [w288] -> w20
    tunnel: [w289] -> w23
    tunnel: w141 -> [w289]
    tunnel: w140 -> [w288]
    frame #0 {
      n114 = Wait (ms)(milliseconds to wait=u32 1000) -> ()  [unwired: 1 out]
    }
    frame #1 {
      n115 = xnode "Read/Write Control"("FPGA VI Reference In"=w275, "error in"=w274, "Phase count adjustment"=w277, "Phase count adjustment (GI)"=w276, "Phase count adjustment (MCL)"=w273, "Phase Count Adjustment (APD Acq)"=w271, "Phase count adjustment (APD 1 Gate)"=w270, "Phase count adjustment (APD 2 Gate)"=w267, "Phase count adjustment (Green FB)"=w269, "Phase count adjustment (GI) 2"=w268) -> ("FPGA VI Reference Out"=w272:T19, "error out"=w278:errorcluster)
    }
    frame #2 {
      n116 = Wait (ms)(milliseconds to wait=u32 1000) -> ()  [unwired: 1 out]
    }
    frame #3 {
      w282 = TRUE
      n117 = xnode "Read/Write Control"("FPGA VI Reference In"=w284, "error in"=w283, "+ phase"=w282, "+ phase (GI)"=w282, "+ phase (MCL)"=w282, "+ phase (APD Acq)"=w282, "+ phase (APD 1 Gate)"=w282, "+ phase (APD 2 Gate)"=w282, "+ phase (Green FB)"=w282, "+ phase (GI) 2"=w282) -> ("FPGA VI Reference Out"=w285:T19, "error out"=w286:errorcluster)
    }
    frame #4 {
      n118 = Wait (ms)(milliseconds to wait=u32 1000) -> ()  [unwired: 1 out]
    }
  }
  n119 = local read "Phase adj. (Green FB)"() -> (w113:i16)
  n120 = local read "Phase adj. (GI) 2"() -> (w83:i16)
  n121 = local read "Phase adjust (MCL)"() -> (w172:i16)
  n122 = local read "Phase adj. (AI1)"() -> (w174:i16)
  n123 = local read "Phase adj. (GI)"() -> (w173:i16)
  n124 = xnode "Read/Write Control"("FPGA VI Reference In"=w20, "error in"=w23, "Phase count adjustment"=w174, "Phase count adjustment (GI)"=w173, "Phase count adjustment (MCL)"=w172, "Phase Count Adjustment (APD Acq)"="Phase Adj. (APD Acq)", "Phase count adjustment (APD 1 Gate)"="Phase Adj. (APD 1 Gate)", "Phase count adjustment (APD 2 Gate)"="Phase Adj. (APD 2 Gate)", "Phase count adjustment (Green FB)"=w113, "Phase count adjustment (GI) 2"=w83) -> ("FPGA VI Reference Out"=w19:T19, "error out"=w18:errorcluster)
  n125 = call "Initialize RF boards - interlace 3.vi"("error in"=w18, "FPGA VI Reference In"=w19) -> ("FPGA VI Reference Out"=w150:T19)  [unwired: 1 out]
  n126 = call "set RF board frequency - interlace.vi"("Board 2 Frequency Limits"=w116, "Board 1 Frequency Limits"=w118, "FPGA VI Reference In"=w150, "Board 2 Frequency 3 (MHz)"="BD 2 Frequency 3 (MHz)", "Board 1 Frequency 3 (MHz)"="BD 1 Frequency 3 (MHz)", "Board 2 Frequency 2 (MHz)"="BD 2 Frequency 2 (MHz)", "Board 2 Frequency 1 (MHz)"="BD 2 Frequency 1 (MHz)", "Board 1 Frequency 2 (MHz)"="BD 1 Frequency 2 (MHz)", "Board 1 Frequency 1  (MHz)"="BD 1 Frequency 1 (MHz)") -> ("error out"=w244:errorcluster, "FPGA VI Reference Out"=w245:T19)  [unwired: 1 in]
  n127 = call "set RF board amplitude - interlace.vi"("Board 2 Amplitude Limits"=w115, "Board 1 Amplitude Limits"=w117, "error in"=w244, "FPGA VI Reference In"=w245, "Board 2 Amplitude 3 (%)"="BD 2 Amplitude 3 (%)", "Board 1 Amplitude 3 (%)"="BD 1 Amplitude 3 (%)", "Board 2 Amplitude 2 (%)"="BD 2 Amplitude 2 (%)", "Board 2 Amplitude 1 (%)"="BD 2 Amplitude 1 (%)", "Board 1 Amplitude 2 (%)"="BD 1 Amplitude 2 (%)", "Board 1 Amplitude 1 (%)"="BD 1 Amplitude 1 (%)") -> ("error out"=w16:errorcluster, "FPGA VI Reference Out"=w17:T19)
  n128 = flat-sequence {
    tunnel: w17 -> [w298]
    tunnel: w16 -> [w297]
    tunnel: [w296] -> w237
    tunnel: [w295] -> w236
    tunnel: [w302] -> w235
    tunnel: w237 -> [w302]
    tunnel: [w301] -> w234
    tunnel: w236 -> [w301]
    tunnel: w235 -> [w311]
    tunnel: w234 -> [w310]
    tunnel: [w309] -> w12
    tunnel: [w304] -> w11
    tunnel: [w314] -> w40
    tunnel: [w318] -> w24
    tunnel: w12 -> [w318]
    tunnel: w11 -> [w313]
    frame #0 {
      n129 = local read "Trap 1 (ON/OFF)"() -> (w290:bool)
      n130 = xnode "Read/Write Control"("FPGA VI Reference In"=w298, "error in"=w297, "Direct RF Box  Communication"=FALSE) -> ("FPGA VI Reference Out"=w296:T19, "error out"=w295:errorcluster)
      n131 = local write "Saving..."(FALSE ("Saving Data")) -> ()
      n132 = local write "Stop All"(FALSE ("Stop All")) -> ()
      n133 = local write "Index"(1.0 ("Index")) -> ()
      n134 = property on="Trap 1 ON" class="Bool (strict)"("Value"=w290) -> ()  [unwired: 2 in, 2 out]
      "Manipulating Trap" <- FALSE ("Manipulating Trap")
    }
    frame #1 {
      n135 = local read "Trap 2 (ON/OFF)"() -> (w300:bool)
      n136 = Wait (ms)(milliseconds to wait=u32 50) -> ()  [unwired: 1 out]
      n137 = property on="Trap 2 ON" class="Bool (strict)"("Val(Sgnl)"=w300) -> ()  [unwired: 2 in, 2 out]
    }
    frame #2 {
      n138 = local read "Scan Range (nm)"() -> (w305:dbl)
      n139 = xnode "Read/Write Control"("FPGA VI Reference In"=w311, "error in"=w310, "FPGA Controls  RF Box"=TRUE ("Direct RF Box  Communication")) -> ("FPGA VI Reference Out"=w309:T19, "error out"=w304:errorcluster)
      n140 = call "Update messages.vi"("Message to add"="UHR-Fleezers ready.", "Old message string"="") -> ("New message string"=w308:string)
      n141 = local write "Messages"(w308) -> ()
      n142 = property on="Scan Range (nm)" class="DigNum (strict)"("Val(Sgnl)"=w305) -> ()  [unwired: 2 in, 2 out]
    }
    frame #3 {
      n143 = call "hamilton_controller.vi"("error in"=w313, "action"=T20."CONNECT") -> ("error out"=w315:errorcluster)  [unwired: 9 in]
      n144 = call "hamilton_controller.vi"("error in"=w315, "action"=T20."INITIALIZE VALVES") -> ("error out"=w314:errorcluster)  [unwired: 9 in]
    }
  }
  n145 = Subtract(x="BD 1 Frequency 1 (MHz)", y="BD 1 Frequency 2 (MHz)") -> (x-y=w160:dbl)
  n146 = Subtract(x="BD 2 Frequency 1 (MHz)", y="BD 2 Frequency 2 (MHz)") -> (x-y=w159:dbl)
  n147 = Square(x=w159) -> (x^2=w157:dbl)
  n148 = Square(x=w160) -> (x^2=w158:dbl)
  n149 = Add(x=w158, y=w157) -> (x+y=w156:dbl)
  n150 = Square Root(x=w156) -> (sqrt(x)=w155:dbl)
  n151 = local write "Trap Delta (MHz)"(w155) -> ()
  n152 = Current VI's Path() -> (path=w1:path)
  n153 = Strip Path(path=w1) -> (stripped path=w2:path)  [unwired: 1 out]
  n154 = Build Path(base path=w2, name or relative path="Locations.txt") -> (appended path=→"Location path":path)
  n155 = Concatenate Strings("N.D.", "\r\n") -> (w5:string)
  n156 = Initialize Array(w5, 4, 3) -> (w8:string[][])
  n157 = local write "Location Matrix"(w8) -> ()
  n158 = call "IMAQ Create"("Image Name"="APD 1 Image", "Image Type"=w64) -> ("New Image"=w63:T2)  [unwired: 3 in, 1 out]
  n159 = call "IMAQ Create"("Image Name"="APD 2 Image", "Image Type"=w64) -> ("New Image"=w62:T2)  [unwired: 3 in, 1 out]
  n160 = call "IMAQ Create"("Image Name"="Det. X Image", "Image Type"=w64) -> ("New Image"=w61:T2)  [unwired: 3 in, 1 out]
  n161 = call "IMAQ Create"("Image Name"="Det. Y Image", "Image Type"=w64) -> ("New Image"=w60:T2)  [unwired: 3 in, 1 out]
  n162 = Bundle("New Image"=w63, "New Image"=w62, "New Image"=w61, "New Image"=w60) -> (w59:T21)  [unwired: 1 in]
  n163 = while {
    stop <- w319 stop-if-true
    n164 = event shown="[0] Timeout" {
      selector: _ -> [_ _ _ _ _ _ _]
      dyn-events: _ -> [_ _ _ _ _ _ _]
      timeout: 10 -> [_ _ _ _ _ _ _]
      tunnel: [FALSE _ _ _ _ _ _] -> w319
      event Timeout {
        # "Query and display stage positions"
        # "Setting ESP300 left and right limits for Z-axis, input in mm"
        # "Display Selected Location"
        n165 = event-data() -> ()  [unwired: 1 in, 2 out]
        n166 = local read "ESP Port"() -> (w336:refnum<visa-resource-name>)
        n167 = Concatenate Strings("3SL" ("Substring"), "ESP ZL-Limit", ";3SR", "ESP ZR-Limit", "\r") -> (w335:string)
        n168 = VISA Write(VISA resource name=w336, write buffer=w335) -> ()  [unwired: 1 in, 3 out]
        n169 = disable-structure shown="Disabled" {
          frame Disabled {
            # "Change Low Jog Velocity"
            # "Change High Jog Velocity"
            n170 = Concatenate Strings("1JH" ("Substring"), "Axis 1", "2JH" ("Substring"), "Axis 2", "3JH" ("Substring"), "Axis 3", "\r") -> (w359:string)
            n171 = local read "ESP Port"() -> (w358:refnum<visa-resource-name>)
            n172 = VISA Write(VISA resource name=w358, write buffer=w359) -> ()  [unwired: 1 in, 3 out]
            n173 = Concatenate Strings("1JW" ("Substring"), "Axis 1", "2JW" ("Substring"), "Axis 2", "3JW" ("Substring"), "Axis 3", "\r") -> (w350:string)
            n174 = local read "ESP Port"() -> (w349:refnum<visa-resource-name>)
            n175 = VISA Write(VISA resource name=w349, write buffer=w350) -> ()  [unwired: 1 in, 3 out]
          }
          frame Enabled {
          }
        }
        n176 = local read "Location Matrix"() -> (w341:string[][])
        n177 = local read "Locations"() -> (w340:i32)
        n178 = Index Array(array=w341, index (row)=w340) -> (element=w339:string[])  [unwired: 1 in]
        n179 = Array To Cluster(array=w339) -> (cluster=w338:T22)
        n180 = local write "Selected Location"(w338) -> ()
        n181 = Concatenate Strings("1TP\n\n;2TP\n\n;3TP\n" ("Substring"), "\r") -> (w324:string)
        n182 = local read "ESP Port"() -> (w327:refnum<visa-resource-name>)
        n183 = VISA Write(VISA resource name=w327, write buffer=w324, error in (no error)="error in") -> (VISA resource name out=w325:refnum<visa-resource-name>, error out=w323:errorcluster)  [unwired: 1 out]
        n184 = case shown="True" TRUE ("Case Constant\n(See Context Help)") {
          tunnel: w325 -> [_ w370]
          tunnel: w323 -> [w360 w369]
          tunnel: [w360 w361] -> w329
          frame False {
          }
          frame True {
            w363 = u16 10 items=["1.0"=10, "1.5"=15, "2.0"=20] ("Serial Settings:Stop Bits")
            w364 = u16 0 items=["None", "Odd", "Even", "Mark", "Space"] ("Serial Settings:Parity")
            n185 = property class="Instr"(reference=w370, error in=w369, "Baud"=u32 921600 ("Serial Settings:Baud Rate"), "Data Bits"=u16 8 ("Serial Settings:Data Bits"), "Parity"=w364, "Stop Bits"=w363) -> (reference out=w368:refnum<visa-resource-name>, error out=w367:errorcluster, "Bytes at Port"=w362:u32)
            n186 = Wait (ms)(milliseconds to wait=u32 10) -> ()  [unwired: 1 out]
            n187 = VISA Read(VISA resource name=w368, byte count=w362, error in (no error)=w367) -> (VISA resource name out=w376:refnum<visa-resource-name>, read buffer=→"X Pos":string, error out=w377:errorcluster)  [unwired: 1 out]
            n188 = VISA Read(VISA resource name=w376, byte count=w362, error in (no error)=w377) -> (VISA resource name out=w374:refnum<visa-resource-name>, read buffer=→"Y Pos":string, error out=w375:errorcluster)  [unwired: 1 out]
            n189 = VISA Read(VISA resource name=w374, byte count=w362, error in (no error)=w375) -> (read buffer=→"Z Pos Pos":string, error out=w361:errorcluster)  [unwired: 2 out]
          }
        }
        "error out" <- w329
      }
      event "Goto Top (F6)": Value Change {
        n190 = event-data() -> ()  [unwired: 1 in, 5 out]
        n191 = stacked-sequence {
          frame #0 {
            # "stop motions of all axes before going to avoid reversing of direction"
            n192 = local read "ESP Port"() -> (w382:refnum<visa-resource-name>)
            n193 = Concatenate Strings("ST" ("Substring"), "\r") -> (w379:string)
            n194 = VISA Write(VISA resource name=w382, write buffer=w379) -> ()  [unwired: 1 in, 3 out]
          }
          frame #1 {
            n195 = Wait (ms)(milliseconds to wait=u32 50) -> ()  [unwired: 1 out]
          }
          frame #2 {
            # "Change the trajectory mode to Trapezoidal"
            n196 = local read "ESP Port"() -> (w387:refnum<visa-resource-name>)
            n197 = Concatenate Strings("1TJ1;\n2TJ1;\n3TJ1" ("Substring"), "\r") -> (w384:string)
            n198 = VISA Write(VISA resource name=w387, write buffer=w384) -> ()  [unwired: 1 in, 3 out]
          }
          frame #3 {
            # "Go to Top Dispensor"
            n199 = local read "Location Matrix"() -> (w399:string[][])
            n200 = Index Array(array=w399, index (row)=0) -> (element=w395:string[])  [unwired: 1 in]
            n201 = Decimate 1D Array(w395) -> (w393:string[], w391:string[], w389:string[])
            n202 = Concatenate Strings("1PA" ("Substring"), w393, "2PA" ("Substring"), w391, "3PA" ("Substring"), w389, "\r") -> (w397:string)
            n203 = local read "ESP Port"() -> (w396:refnum<visa-resource-name>)
            n204 = VISA Write(VISA resource name=w396, write buffer=w397) -> ()  [unwired: 1 in, 3 out]
          }
          frame #4 {
            n205 = Wait (ms)(milliseconds to wait=u32 2000) -> ()  [unwired: 1 out]
          }
        }
      }
      event "Goto Exp (F8)": Value Change {
        n206 = event-data() -> ()  [unwired: 1 in, 5 out]
        n207 = stacked-sequence {
          frame #0 {
            # "stop motions of all axes before going to avoid reversing of direction"
            n208 = local read "ESP Port"() -> (w404:refnum<visa-resource-name>)
            n209 = Concatenate Strings("ST" ("Substring"), "\r") -> (w401:string)
            n210 = VISA Write(VISA resource name=w404, write buffer=w401) -> ()  [unwired: 1 in, 3 out]
          }
          frame #1 {
            n211 = Wait (ms)(milliseconds to wait=u32 50) -> ()  [unwired: 1 out]
          }
          frame #2 {
            # "Change the trajectory mode to Trapezoidal"
            n212 = local read "ESP Port"() -> (w409:refnum<visa-resource-name>)
            n213 = Concatenate Strings("1TJ1;\n2TJ1;\n3TJ1" ("Substring"), "\r") -> (w406:string)
            n214 = VISA Write(VISA resource name=w409, write buffer=w406) -> ()  [unwired: 1 in, 3 out]
          }
          frame #3 {
            # "Go to Experimental"
            n215 = local read "Location Matrix"() -> (w421:string[][])
            n216 = Index Array(array=w421, index (row)=2) -> (element=w417:string[])  [unwired: 1 in]
            n217 = Decimate 1D Array(w417) -> (w415:string[], w413:string[], w411:string[])
            n218 = Concatenate Strings("1PA" ("Substring"), w415, "2PA" ("Substring"), w413, "3PA" ("Substring"), w411, "\r") -> (w419:string)
            n219 = local read "ESP Port"() -> (w418:refnum<visa-resource-name>)
            n220 = VISA Write(VISA resource name=w418, write buffer=w419) -> ()  [unwired: 1 in, 3 out]
          }
          frame #4 {
            n221 = Wait (ms)(milliseconds to wait=u32 100) -> ()  [unwired: 1 out]
          }
        }
      }
      event "Goto Bottom (F7)": Value Change {
        n222 = event-data() -> ()  [unwired: 1 in, 5 out]
        n223 = stacked-sequence {
          frame #0 {
            # "stop motions of all axes before going to avoid reversing of direction"
            n224 = local read "ESP Port"() -> (w426:refnum<visa-resource-name>)
            n225 = Concatenate Strings("ST" ("Substring"), "\r") -> (w423:string)
            n226 = VISA Write(VISA resource name=w426, write buffer=w423) -> ()  [unwired: 1 in, 3 out]
          }
          frame #1 {
            n227 = Wait (ms)(milliseconds to wait=u32 50) -> ()  [unwired: 1 out]
          }
          frame #2 {
            # "Change the trajectory mode to Trapezoidal"
            n228 = local read "ESP Port"() -> (w431:refnum<visa-resource-name>)
            n229 = Concatenate Strings("1TJ1;\n2TJ1;\n3TJ1" ("Substring"), "\r") -> (w428:string)
            n230 = VISA Write(VISA resource name=w431, write buffer=w428) -> ()  [unwired: 1 in, 3 out]
          }
          frame #3 {
            # "Go to Bottom Dispensor"
            n231 = local read "Location Matrix"() -> (w443:string[][])
            n232 = Index Array(array=w443, index (row)=1) -> (element=w439:string[])  [unwired: 1 in]
            n233 = Decimate 1D Array(w439) -> (w437:string[], w435:string[], w433:string[])
            n234 = Concatenate Strings("1PA" ("Substring"), w437, "2PA" ("Substring"), w435, "3PA" ("Substring"), w433, "\r") -> (w441:string)
            n235 = local read "ESP Port"() -> (w440:refnum<visa-resource-name>)
            n236 = VISA Write(VISA resource name=w440, write buffer=w441) -> ()  [unwired: 1 in, 3 out]
          }
          frame #4 {
            n237 = Wait (ms)(milliseconds to wait=u32 100) -> ()  [unwired: 1 out]
          }
        }
      }
      event "Capture": Value Change {
        n238 = event-data() -> ()  [unwired: 1 in, 5 out]
        n239 = local read "Locations"() -> (w445:i32)
        n240 = local read "Z Pos Pos"() -> (w446:string)
        n241 = local read "X Pos"() -> (w448:string)
        n242 = local read "Y Pos"() -> (w447:string)
        n243 = case shown="1" w445 {
          selector: w445 -> [w452 w459 w466 w473]
          tunnel: w448 -> [w455 w462 w469 w476]
          tunnel: w447 -> [w454 w461 w468 w475]
          tunnel: w446 -> [w453 w460 w467 w474]
          frame 0, Default {
            # "Capture Top Dispensor Location"
            n244 = local read "Location Matrix"() -> (w451:string[][])
            n245 = Build Array(w455, w454, w453) -> (w450:string[])
            n246 = Replace Array Subset(array=w451, new element=w450, index (row)=w452) -> (w449:string[][])  [unwired: 1 in]
            n247 = local write "Location Matrix"(w449) -> ()
          }
          frame 1 {
            # "Capture Bottom Dispensor Location"
            n248 = local read "Location Matrix"() -> (w458:string[][])
            n249 = Build Array(w462, w461, w460) -> (w457:string[])
            n250 = Replace Array Subset(array=w458, new element=w457, index (row)=w459) -> (w456:string[][])  [unwired: 1 in]
            n251 = local write "Location Matrix"(w456) -> ()
          }
          frame 2 {
            # "Capture Experimental Region Location"
            n252 = local read "Location Matrix"() -> (w465:string[][])
            n253 = Build Array(w469, w468, w467) -> (w464:string[])
            n254 = Replace Array Subset(array=w465, new element=w464, index (row)=w466) -> (w463:string[][])  [unwired: 1 in]
            n255 = local write "Location Matrix"(w463) -> ()
          }
          frame 3 {
            # "Capture Other Location"
            n256 = local read "Location Matrix"() -> (w472:string[][])
            n257 = Build Array(w476, w475, w474) -> (w471:string[])
            n258 = Replace Array Subset(array=w472, new element=w471, index (row)=w473) -> (w470:string[][])  [unwired: 1 in]
            n259 = local write "Location Matrix"(w470) -> ()
          }
        }
      }
      event "Save": Value Change {
        # "reshape Location Matrix to 1-D array to write"
        n260 = event-data() -> ()  [unwired: 1 in, 5 out]
        n261 = local read "Location Matrix"() -> (w480:string[][])
        n262 = local read "Location path"() -> (w477:path)
        n263 = Reshape Array(w480, 12) -> (w478:string[])
        n264 = Write to Text File(file (use dialog)=w477, text=w478) -> ()  [unwired: 2 in, 3 out]
      }
      event "Activate Joystick": Value Change {
        n265 = event-data() -> ()  [unwired: 1 in, 5 out]
        n266 = case shown="True" "Activate Joystick" {
          frame False {
          }
          frame True {
            # "Change the trajectory mode to Jog"
            n267 = local read "ESP Port"() -> (w485:refnum<visa-resource-name>)
            n268 = Concatenate Strings("1TJ3;\n2TJ3;\n3TJ3" ("Substring"), "\r") -> (w482:string)
            n269 = VISA Write(VISA resource name=w485, write buffer=w482) -> ()  [unwired: 1 in, 3 out]
          }
        }
      }
    }
  }
  n270 = disable-structure shown="Disabled" {
    disable-tunnel: w24 -> [w514 _]
    frame Disabled {
      w509 = T17 0 items=["Grayscale (U8)", "Grayscale (I16)", "Grayscale (SGL)", "Complex (CSG)", "RGB (U32)", "HSL (U32)", "RGB (U64)", "Grayscale (U16)"] ("Image Type")
      n271 = call <vilib>:"IMAQ Init.vi"("Interface Name"="img0") -> ("error out"=w511:errorcluster, "IMAQ Session Out"=w513:refnum<k11>)  [unwired: 9 in]
      n272 = call <vilib>:"IMAQ Grab Setup.vi"("error in (no error)"=w511, "IMAQ Session In"=w513) -> ("error out"=w507:errorcluster, "IMAQ Session Out"=w508:refnum<k11>)  [unwired: 8 in]
      n273 = call "IMAQ Create"("Image Name"="untitled", "Image Type"=w509) -> ("New Image"=w506:T2)  [unwired: 3 in, 1 out]
      n274 = call <vilib>:"Application Directory.vi"() -> ("Application Directory"=w493:path)
      n275 = Build Path(base path=w493, name or relative path="_trap_screen_positions") -> (appended path=w501:path)
      n276 = Open/Create/Replace File(file path (use dialog)=w501, operation (0:open)=T23."open or create", access (0:read/write)=enum16{"read/write", "read-only", "write-only"}."read/write") -> (refnum out=w503:refnum<file>)  [unwired: 3 in, 2 out]
      n277 = local read "Trap Sets"() -> (w495:u32)
      n278 = for "Load trap positions on video screen from file." {
        N: w495 -> [_]
        tunnel: [w521] -> w496
        tunnel: w503 -> [w520]
        tunnel: [w517] -> w492 mode=indexing
        w519 = 4
        n279 = for {
          N: w519 -> [_]
          tunnel: [w525] -> w521
          tunnel: w520 -> [w524]
          tunnel: w519 -> [w523]
          tunnel: [w522] -> w518 mode=indexing
          n280 = Read from Binary File(5:w523, 11:w524) -> (2:w522:i32, 3:w525:refnum<file>)  [unwired: 4 in, 2 out]
        }
        n281 = Array To Cluster(array=w518) -> (cluster=w517:T27)
      }
      n282 = node-c288() -> (w516:T24)  [unwired: 4 in]
      n283 = timed-loop "acquire video and stage position" {
        timing: w516 -> [_]
        timing-out: [_] -> w515
        tunnel: w508 -> [w544]
        tunnel: w507 -> [w543]
        tunnel: w506 -> [w542]
        tunnel: [w541] -> w488
        tunnel: [w538] -> w489
        tunnel: [w539] -> w487
        tunnel: w514 -> [_]
        shift-right: [w535] -> w505
        shift-left: w492 -> [w536]
        tunnel: w495 -> [w533]
        stop <- w540 stop-if-true
        n284 = node-c288() -> ()  [unwired: 1 in, 1 out]
        n285 = event shown="[2] \"Primary Video Display\": Mouse Down" {
          selector: _ -> [_ _ _ _]
          dyn-events: _ -> [_ _ _ _]
          timeout: 10 -> [_ _ _ _]
          tunnel: w544 -> [w555 w570 w579 w598]
          tunnel: w543 -> [w554 w572 w577 w600]
          tunnel: w542 -> [w553 w571 w578 w599]
          tunnel: [w552 w570 w579 w598] -> w541
          tunnel: [w545 w574 FALSE FALSE] -> w540
          tunnel: [w549 w572 w577 w600] -> w539
          tunnel: [w548 w571 w578 w599] -> w538
          tunnel: "radius" -> [_ _ w584 _]
          tunnel: w536 -> [w546 w573 w582 _]
          tunnel: [w546 w573 w583 cluster{i32, i32, i32, i32}[] []] -> w535
          tunnel: w533 -> [_ _ w575 _]
          event Timeout {
            n286 = event-data() -> ()  [unwired: 1 in, 2 out]
            n287 = call <vilib>:"IMAQ Grab Acquire.vi"("error in (no error)"=w554, "Image In"=w553, "IMAQ Session In"=w555) -> ("error out"=w550:errorcluster, "Image Out"=w551:T2, "IMAQ Session Out"=w552:refnum<k11>)  [unwired: 5 in, 1 out]
            n288 = case shown="True" "trap\nmarkers?" {
              tunnel: w546 -> [_ w563]
              tunnel: w551 -> [w557 w562]
              tunnel: w550 -> [w556 w561]
              tunnel: [w556 w560] -> w549
              tunnel: [w557 w558] -> w548
              frame False {
              }
              frame True {
                n289 = for {
                  tunnel: w563 -> [w569] mode=indexing
                  shift-right: [w567] -> w558
                  shift-left: w562 -> [w568]
                  tunnel: w561 -> [w566]
                  tunnel: [w565] -> w560
                  tunnel: u32 16711680 ("Color") -> [w564]
                  n290 = call "IMAQ Overlay Oval"("Color"=w564, "error in (no error)"=w566, "Bounding Rectangle"=w569, "Image"=w568) -> ("error out"=w565:errorcluster, "Image Out"=w567:T2)  [unwired: 6 in]
                }
              }
            }
            "Primary Video Display" <- w548
            n291 = Unbundle By Name(w550) -> ("status"=w545:bool)
          }
          event "Stop All": Value Change {
            n292 = event-data() -> ()  [unwired: 1 in, 5 out]
            n293 = local read "Stop All"() -> (w574:bool)
          }
          event "Primary Video Display": Mouse Down {
            n294 = event-data() -> ()  [unwired: 1 in, 7 out]
            n295 = Array Size(array=w582) -> (size(s)=w581:i32)
            n296 = Less?(x=w581, y=w575) -> (x < y?=w580:bool)
            n297 = case shown="True" w580 {
              tunnel: w584 -> [_ w594]
              tunnel: w582 -> [w585 w588]
              tunnel: [w585 w587] -> w583
              frame False {
              }
              frame True {
                n298 = property on="Primary Video Display" class="ImageControl"() -> ("Last Mouse Position"=w586:cluster{"X":i32, "Y":i32})  [unwired: 2 in, 2 out]
                n299 = Unbundle By Name(w586) -> ("X"=w596:i32, "Y"=w595:i32)
                n300 = Add(x=w595, y=w594) -> (x+y=w592:i32)
                n301 = Subtract(x=w595, y=w594) -> (x-y=w590:i32)
                n302 = Add(x=w596, y=w594) -> (x+y=w591:i32)
                n303 = Subtract(x=w596, y=w594) -> (x-y=w593:i32)
                n304 = Bundle(w593, w592, w591, w590) -> (w589:cluster{i32, i32, i32, i32})  [unwired: 1 in]
                n305 = Build Array (concatenate)(w588, w589) -> (w587:T28)
              }
            }
          }
          event "clear markers": Value Change {
            n306 = event-data() -> ()  [unwired: 1 in, 5 out]
          }
        }
        n307 = node-c288() -> ()  [unwired: 1 in, 1 out]
      }
      n308 = node-c288(w515) -> ()  [unwired: 1 out]
      n309 = Set File Position(offset (in bytes) (0)=i64 0, refnum=w496, from (0:start)=enum16{"start", "end", "current"}."start") -> (refnum out=w497:refnum<file>)  [unwired: 1 in, 1 out]
      n310 = for "Write trap positions to file so they can be remembered\nwhen program is removed from memory" {
        tunnel: w505 -> [w529] mode=indexing
        tunnel: [w527] -> w504
        tunnel: w497 -> [w526]
        n311 = Cluster To Array(cluster=w529) -> (array=w528:i32[])
        n312 = for {
          tunnel: w528 -> [w532] mode=indexing
          tunnel: [w531] -> w527
          tunnel: w526 -> [w530]
          n313 = Write to Binary File(file (use dialog)=w530, data=w532) -> (refnum out=w531:refnum<file>)  [unwired: 4 in, 2 out]
        }
      }
      n314 = Close File(refnum=w504) -> ()  [unwired: 1 in, 2 out]
      n315 = call "IMAQ Dispose"("Image"=w489, "error in (no error)"=w487) -> ("error out"=w486:errorcluster)  [unwired: 4 in]
      n316 = call <vilib>:"IMAQ Stop.vi"("error in (no error)"=w486, "IMAQ Session In"=w488) -> ("error out"=w490:errorcluster, "IMAQ Session Out"=w491:refnum<k11>)  [unwired: 8 in]
      n317 = call <vilib>:"IMAQ Close.vi"("error in (no error)"=w490, "IMAQ Session In"=w491) -> ()  [unwired: 9 in, 1 out]
    }
    frame Enabled {
    }
  }
  n318 = node-c288(2 ("Processor")) -> (w15:T24)  [unwired: 3 in]
  n319 = node-c288() -> (w69:T24)  [unwired: 4 in]
  n320 = disable-structure shown="Enabled" {
    disable-tunnel: [w607 _] -> w35
    disable-tunnel: w24 -> [w606 _]
    frame Enabled {
      n321 = node-c288() -> (w609:T24)  [unwired: 4 out]
      n322 = timed-loop "Rough control of MCL mirror stage (debugging)" {
        tunnel: w606 -> [w612]
        tunnel: [w611] -> w607
        timing: w609 -> [_]
        timing-out: [_] -> w608
        stop <- w611 stop-if-true
        n323 = node-c288() -> ()  [unwired: 2 out]
        n324 = case shown="1" "MCL Mode" {
          tunnel: w612 -> [_ w615 w662]
          frame 0, Default {
            # "manual positioning"
          }
          frame 1 {
            # "sinusoidal wave"
            n325 = node-c288() -> (w617:T24)  [unwired: 4 out]
            n326 = timed-loop "Oscillate MCL mirror" {
              timing: w617 -> [_]
              timing-out: [_] -> w616
              tunnel: w615 -> [w656]
              i -> [w655]
              stop <- w618 stop-if-true
              n327 = node-c288() -> (w654:i64)  [unwired: 1 out]
              n328 = Multiply(x="AO1", y=32767.0) -> (x*y=w650:dbl)
              n329 = Multiply(x="AO2", y=32767.0) -> (x*y=w645:dbl)
              n330 = Divide(x=w650, y=10.0) -> (x/y=w651:dbl)
              n331 = Divide(x=w645, y=10.0) -> (x/y=w646:dbl)
              n332 = To Word Integer(number=w651) -> (16bit integer=w643:i16)
              n333 = To Word Integer(number=w646) -> (16bit integer=w642:i16)
              n334 = Divide(x=w654, y=i64 1000) -> (x/y=w625:dbl)
              n335 = Multiply(x=w625, y=w655) -> (x*y=w636:dbl)
              n336 = Multiply(x="Osc. freq. (Hz) 2", y=6.283185307179586) -> (x*y=w637:dbl)
              n337 = Multiply(x=w637, y=w636) -> (x*y=w635:dbl)
              n338 = Sine(x=w635) -> (sin(x)=w634:dbl)
              n339 = Multiply(x=w634, y="Osc. amp. (V)") -> (x*y=w632:dbl)
              n340 = Add(x=w632, y="Osc. center (V)") -> (x+y=w630:dbl)
              n341 = Divide(x=w630, y=10.0) -> (x/y=w628:dbl)
              n342 = Multiply(x=w628, y=32767.0) -> (x*y=w623:dbl)
              n343 = Select(t=w623, s="Scan axis", f=w643) -> (s? t:f=w641:dbl)
              n344 = Select(t=w642, s="Scan axis", f=w623) -> (s? t:f=w640:dbl)
              n345 = local read "MCL Mode"() -> (w622:u16)
              n346 = Not Equal?(x=w622, y=u16 1) -> (x != y?=w619:bool)
              n347 = local read "Stop All"() -> (w620:bool)
              n348 = xnode "Read/Write Control"("FPGA VI Reference In"=w656, "AO1"=w641, "AO2"=w640) -> ()  [unwired: 1 in, 2 out]
              n349 = Compound Arithmetic op=OR(w620, w619) -> (w618:bool)
              n350 = node-c288() -> ()  [unwired: 2 out]
            }
            n351 = node-c288(w616) -> ()  [unwired: 1 out]
          }
          frame 2 {
            # "linear scan"
            n352 = case shown="True" "Start Scan" {
              tunnel: w662 -> [_ w674]
              frame False {
              }
              frame True {
                n353 = Subtract(x="End (V)", y="Begin (V)") -> (x-y=w670:dbl)
                n354 = Decrement(x="N Points") -> (x-1=w669:dbl)
                n355 = Divide(x=w670, y=w669) -> (x/y=w667:dbl)
                n356 = for {
                  N: "N Points" -> [_]
                  tunnel: "Begin (V)" -> [w687]
                  tunnel: w674 -> [w679]
                  tunnel: [w678] -> w673 mode=indexing
                  tunnel: w667 -> [w677]
                  tunnel: [w675] -> w666 mode=indexing
                  i -> [w686]
                  n357 = Multiply(x=w677, y=w686) -> (x*y=w685:dbl)
                  n358 = Add(x=w687, y=w685) -> (x+y=w682:dbl)
                  n359 = local read "Scan axis"() -> (w676:bool)
                  n360 = local read "AO1"() -> (w684:dbl)
                  n361 = local read "AO2"() -> (w683:dbl)
                  n362 = Select(t=w682, s=w676, f=w684) -> (s? t:f=w681:dbl)
                  n363 = Select(t=w683, s=w676, f=w682) -> (s? t:f=w680:dbl)
                  n364 = flat-sequence {
                    tunnel: w681 -> [w691]
                    tunnel: w680 -> [w690]
                    tunnel: w679 -> [w688]
                    tunnel: [w701] -> w678
                    tunnel: [w700] -> w675
                    frame #0 {
                      w694 = 10.0 ("y")
                      w689 = 32767.0 ("y")
                      n365 = Multiply(x=w691, y=w689) -> (x*y=w697:dbl)
                      n366 = Multiply(x=w690, y=w689) -> (x*y=w695:dbl)
                      n367 = Divide(x=w697, y=w694) -> (x/y=w698:dbl)
                      n368 = Divide(x=w695, y=w694) -> (x/y=w696:dbl)
                      n369 = To Word Integer(number=w698) -> (16bit integer=w692:i16)
                      n370 = To Word Integer(number=w696) -> (16bit integer=w693:i16)
                      n371 = xnode "Read/Write Control"("FPGA VI Reference In"=w688, "AO1"=w692, "AO2"=w693) -> ()  [unwired: 1 in, 2 out]
                    }
                    frame #1 {
                      n372 = Wait (ms)(milliseconds to wait="DAQ Delay (ms)") -> ()  [unwired: 1 out]
                    }
                    frame #2 {
                      n373 = local read "Slow mean"() -> (w701:dbl)
                      n374 = local read "Sigma"() -> (w700:dbl)
                    }
                  }
                }
                n375 = Bundle("Begin (V)"="Begin (V)", w667, w673) -> (→"MCL Scan":cluster{"Begin (V)":dbl, dbl, dbl[]})  [unwired: 1 out]
                n376 = Bundle("Begin (V)"="Begin (V)", w667, w666) -> (→"MCL Scan 2":cluster{"Begin (V)":dbl, dbl, dbl[]})  [unwired: 1 out]
              }
            }
          }
        }
        n377 = local read "Stop All"() -> (w611:bool)
        n378 = node-c288() -> ()  [unwired: 2 out]
      }
      n379 = node-c288(w608) -> ()  [unwired: 1 out]
    }
    frame Disabled {
    }
  }
  n380 = timed-loop "Control parameters (event loop)" {
    tunnel: w24 -> [w707]
    shift-right: [w706] -> _
    shift-left: errorcluster {"status"=FALSE, "code"=0, "source"=""} ("error out") -> [w705]
    tunnel: [w704] -> w37
    timing: w15 -> [_]
    timing-out: [_] -> w14
    stop <- w704 stop-if-true
    n381 = node-c288() -> ()  [unwired: 1 in, 1 out]
    n382 = event shown="[6] \"BD 1 Frequency 1 (MHz)\", \"BD 1 Frequency 2 (MHz)\", \"BD 1 Frequency 3 (MHz)\", \"BD 2 Frequency 1 (MHz)\", \"BD 2 Frequency 2 (MHz)\", \"BD 2 Frequency 3 (MHz)\", \"Trap Delta (MHz)\": Value Change" {
      selector: _ -> [_ _ _ _ _ _ _ _ _ _ _ _ _ _ _ _ _ _ _ _ _ _ _ _ _ _ _ _ _ _ _ _ _ _ _ _ _ _ _ _ _ _ _ _ _ _ _ _ _ _ _ _ _ _ _]
      dyn-events: _ -> [_ _ _ _ _ _ _ _ _ _ _ _ _ _ _ _ _ _ _ _ _ _ _ _ _ _ _ _ _ _ _ _ _ _ _ _ _ _ _ _ _ _ _ _ _ _ _ _ _ _ _ _ _ _ _]
      timeout: _ -> [_ _ _ _ _ _ _ _ _ _ _ _ _ _ _ _ _ _ _ _ _ _ _ _ _ _ _ _ _ _ _ _ _ _ _ _ _ _ _ _ _ _ _ _ _ _ _ _ _ _ _ _ _ _ _]
      tunnel: w707 -> [w745 _ _ _ w782 _ w804 _ w868 _ _ _ w911 _ _ w954 w960 w965 w971 w1007 w1025 w1032 w1050 w1061 w1072 w1083 w1094 w1105 w1123 w1129 w1223 _ w1232 w1270 _ w1305 w1309 w1320 w1324 w1328 _ w1336 _ _ _ _ w1470 _ w1487 w1490 w1499 w1502 w1506 _ w1523]
      tunnel: [w744 _ _ _ w772 _ w803 _ w831 _ w876 _ w890 _ _ w953 w956 w962 w968 w1006 w1023 w1031 w1044 w1055 w1066 w1077 w1088 w1099 w1121 w1128 w1221 _ w1230 w1268 _ w1303 w1307 w1310 w1322 w1326 _ w1334 _ _ _ _ w1468 _ _ _ _ _ _ _ _] -> w706
      tunnel: w705 -> [w743 _ _ _ w781 _ w802 _ w863 _ w876 _ w910 _ _ w952 w955 w961 w967 w1005 w1024 w1030 w1049 w1060 w1071 w1082 w1093 w1104 w1122 w1127 w1222 _ w1231 w1269 _ w1304 w1308 w1319 w1323 w1327 _ w1335 _ _ _ _ w1469 _ w1486 w1489 w1498 w1501 w1505 _ w1522]
      tunnel: [_ _ _ _ _ _ _ _ _ _ w875 _ _ _ _ _ _ _ _ _ _ _ _ _ _ _ _ _ _ _ _ _ _ _ _ _ _ _ _ _ _ _ _ _ _ _ _ _ _ _ _ _ _ _ _] -> w704
      tunnel: [_ _ _ _ _ _ _ "Round T1 X" _ _ _ _ _ _ _ _ _ _ _ _ _ _ _ _ _ _ _ _ _ _ _ _ _ _ _ _ _ _ _ _ _ _ _ _ _ _ _ _ _ _ _ _ _ _ _] -> _
      tunnel: [_ _ _ "Adjust Scale\nto Mean" _ _ _ _ _ _ _ _ _ _ _ _ _ _ _ _ _ _ _ _ _ _ _ _ _ _ _ _ _ _ _ _ _ _ _ _ _ _ _ _ _ _ _ _ _ _ _ _ "Set SP to Reading" _ _] -> _
      tunnel: [_ _ _ _ _ _ _ _ _ "Round T2 X" _ "Delayed Interlace Start" _ _ _ _ _ _ _ _ _ _ _ _ _ _ _ _ _ _ _ _ _ _ _ _ _ _ _ _ _ _ _ _ _ _ _ _ _ _ _ _ _ _ _] -> _
      event "AI Count (ticks)", "Sets to FIFO (Traps)", "Save ave N", "FPGA Ave.", "# Samples/channel", "N sets to save": Value Change {
        # "So that if 'Save ave N' is updated, the AOD scanning code updates too."
        n383 = event-data() -> ()  [unwired: 6 out]
        n384 = local read "AI Count (ticks)"() -> (w725:u32)
        n385 = Boolean To (0,1)(Boolean="Sets to FIFO (Traps)") -> (0, 1=w735:cluster{"Set 1":i16, "Set 2":i16, "Set 3":i16})
        n386 = xnode "Read/Write Control"("FPGA VI Reference In"=w745, "error in"=w743, "ai count"=w725, "AI1 Sets to FIFO"="Sets to FIFO (Traps)", "N of AI1 Int Acq Sets"="N Acq Sets (Traps + Fl.)") -> ("error out"=w744:errorcluster)  [unwired: 1 out]
        n387 = Cluster To Array(cluster=w735) -> (array=w734:i16[])
        n388 = To Unsigned Long Integer(number=w734) -> (unsigned 32bit integer=w714:u32[])
        n389 = local read "Scan steps (AOD)"() -> (w736:u64)
        n390 = Multiply(x=w725, y="N Acq Sets (Traps + Fl.)") -> (x*y=w723:u32)
        n391 = Divide(x=40000000.0, y=w725) -> (x/y=w717:dbl)
        "AI rate (Hz)" <- w717
        "Ave. Rate (Hz)" <- w717
        n392 = Add Array Elements(numeric array=w714) -> (sum=w726:u32)
        "Trap Sets" <- w726
        n393 = Reciprocal(x=w717) -> (1/x=→"Ave. Period (s)":dbl)
        n394 = property on="Scan steps (AOD)" class="DigNum (strict)"("Val(Sgnl)"=w736) -> ()  [unwired: 2 in, 2 out]
        n395 = Divide(x=w717, y="N Acq Sets (Traps + Fl.)") -> (x/y=w740:dbl)
        "Data Rate (Hz)" <- w740
        n396 = Reciprocal(x=w740) -> (1/x=→"Data Period (s)":dbl)
        n397 = local read "Save ave N"() -> (w739:dbl)
        n398 = Divide(x=w740, y=w739) -> (x/y=w738:dbl)
        "Save Data Rate (Hz)" <- w738
        n399 = Reciprocal(x=w738) -> (1/x=→"Save Data Period (s)":dbl)
        n400 = Multiply(x=w723, y="# Samples/trap") -> (x*y=w721:u32)
        "Counts/DMA" <- w721
        n401 = property on="Trap Disp. Downsample" class="DigNum (strict)"("Maximum"="# Samples/trap") -> ()  [unwired: 2 in, 2 out]
        n402 = Multiply(x=w726, y="# Samples/trap") -> (x*y=w715:u32)
        "# Samples/channel" <- w715
        n403 = Multiply(x=w715, y=u32 8) -> (x*y=→"Trap AI Elements/DMA read":u32)
        n404 = local read "APD Int. Count"() -> (w722:u32)
        n405 = Multiply(x=w715, y=u32 3) -> (x*y=→"Trap Pos Elements/DMA read":u32)
        n406 = Divide(x=w721, y=w722) -> (x/y=w712:dbl)
        "APD Samples/FIFO Acq." <- w712
        n407 = Divide(x=w721, y=40000000.0) -> (x/y=w719:dbl)
        "DMA Update Period (s)" <- w719
        n408 = Multiply(x=2.0, y=w712) -> (x*y=→"APD Elements/DMA read":dbl)
        n409 = property on="APD Disp. Downsample" class="DigNum (strict)"("Maximum"=w712) -> ()  [unwired: 2 in, 2 out]
        n410 = local read "N sets to save"() -> (w732:u32)
        n411 = Multiply(x=w719, y=w732) -> (x*y=→"Total Time (s)":dbl)
        "FPGA Averaging" <- FALSE ("FPGA Averaging")
      }
      event "Rescale on Mean": Value Change {
        n412 = event-data() -> ()  [unwired: 7 out]
        n413 = And(x=FALSE, y="Rescale on Mean") -> (x .and. y?=w747:bool)
        n414 = local write "Rescale on Mean"(w747) -> ()
        n415 = local read "Bead Mean (nm)"() -> (w752:dbl)
        n416 = Add(x="Amplitude (nm)", y=w752) -> (x+y=w750:dbl)
        n417 = Subtract(x=w752, y="Amplitude (nm)") -> (x-y=w749:dbl)
        n418 = property on="Bead Separation" class="WFChart (strict)"("YScale.Minimum"=w749) -> ()  [unwired: 2 in, 2 out]
        n419 = property on="Bead Separation" class="WFChart (strict)"("YScale.Maximum"=w750) -> ()  [unwired: 2 in, 2 out]
      }
      event "Detector Type": Value Change {
        n420 = event-data() -> ()  [unwired: 7 out]
        n421 = local read "AI labels"() -> (w753:string[])
        n422 = property on="High Res. Display" class="Ring (strict)"("Strings []"=w753) -> ()  [unwired: 2 in, 2 out]
        n423 = Build Array (concatenate)(w753, "none") -> (w754:string[])
        n424 = property on="FFT 1 Choice 1" class="Ring (strict)"("Strings []"=w754) -> ()  [unwired: 2 in, 2 out]
        n425 = property on="FFT 1 Choice 2" class="Ring (strict)"("Strings []"=w754) -> ()  [unwired: 2 in, 2 out]
        n426 = property on="FFT 2 Choice 1" class="Ring (strict)"("Strings []"=w754) -> ()  [unwired: 2 in, 2 out]
        n427 = property on="FFT 2 Choice 2" class="Ring (strict)"("Strings []"=w754) -> ()  [unwired: 2 in, 2 out]
        n428 = Bundle("APD 1", "APD 2") -> (w757:cluster{string, string})  [unwired: 1 out]
        n429 = Cluster To Array(cluster=w757) -> (array=w755:string[])
        n430 = Build Array (concatenate)(w755, w754) -> (w759:string[])
        n431 = Array Size(array=w759) -> (size(s)=w760:i32)
        n432 = property on="Signals to Plot" class="LstBox (strict)"("Item Names"=w759) -> ()  [unwired: 2 in, 2 out]
        n433 = property on="Signals to Plot" class="LstBox (strict)"("Number of Rows"=w760) -> ()  [unwired: 2 in, 2 out]
        n434 = property on="All Signals" class="WFChart (strict)"("LegNumRows"=w760) -> ()  [unwired: 2 in, 2 out]
      }
      event "Adjust Scale\nto Mean": Value Change {
        n435 = event-data() -> ()  [unwired: 7 out]
        n436 = local read "APD 1 Rate (Hz)"() -> (w769:dbl)
        n437 = Multiply(x=1000.0, y="Above (kHz)") -> (x*y=w767:dbl)
        n438 = Multiply(x=1000.0, y="Below (kHz)") -> (x*y=w765:dbl)
        n439 = Add(x=w767, y=w769) -> (x+y=w762:dbl)
        n440 = Subtract(x=w769, y=w765) -> (x-y=w763:dbl)
        n441 = property on="APD Chart" class="WFChart (strict)"("YScale.Minimum"=w763) -> ()  [unwired: 2 in, 2 out]
        n442 = property on="APD Chart" class="WFChart (strict)"("YScale.Maximum"=w762) -> ()  [unwired: 2 in, 2 out]
      }
      event "Phase adj. (AI1)", "+ phase (AI1)", "- phase (AI1)": Value Change {
        n443 = event-data() -> ()  [unwired: 7 out]
        n444 = Negate(x="Phase adj. (AI1)") -> (-x=w779:i16)
        n445 = Select(t=w779, s="- phase (AI1)", f="Phase adj. (AI1)") -> (s? t:f=w778:i16)
        n446 = xnode "Read/Write Control"("FPGA VI Reference In"=w782, "error in"=w781, "Phase count adjustment"=w778) -> ("FPGA VI Reference Out"=w777:T19, "error out"=w776:errorcluster)
        n447 = Or(x="- phase (AI1)", y="+ phase (AI1)") -> (x .or. y?=w773:bool)
        n448 = xnode "Read/Write Control"("FPGA VI Reference In"=w777, "error in"=w776, "+ phase"=w773) -> ("error out"=w772:errorcluster)  [unwired: 1 out]
      }
      event "Signals to Plot": Double Click {
        w785 = u32 9868950 ("Color Box")
        n449 = event-data() -> ("Row"=w787:i32)  [unwired: 9 out]
        n450 = property on="All Signals" class="WFChart (strict)"("Active Plot"=w787) -> (error out=w798:errorcluster)  [unwired: 2 in, 1 out]
        n451 = property on="All Signals" class="WFChart (strict)" props=["Plot", "Visible?", "Plot", "Plot Color"](error in=w798) -> (error out=w797:errorcluster, "Plot.Visible?"=w796:bool)  [unwired: 1 in, 2 out]
        n452 = Select(t=FALSE ("Plot.Visible"), s=w796, f=TRUE ("Plot.Visible")) -> (s? t:f=w791:bool)
        n453 = property on="All Signals" class="WFChart (strict)"(error in=w797, "Plot.Visible?"=w791) -> (error out=w793:errorcluster)  [unwired: 1 in, 1 out]
        n454 = property on="All Signals" class="WFChart (strict)"(error in=w793) -> (error out=w788:errorcluster, "Plot.Plot Color"=w792:u32)  [unwired: 1 in, 1 out]
        n455 = property on="Signals to Plot" class="LstBox (strict)"(error in=w788, "Active Row"=w787) -> (error out=w786:errorcluster)  [unwired: 1 in, 1 out]
        n456 = Select(t=w792, s=w791, f=u32 0) -> (s? t:f=w789:u32)
        n457 = property on="Signals to Plot" class="LstBox (strict)"(error in=w786, "CellFontColor"=w789, "SelColor"=w785, "CellBG"=w785, "CellFontSize"=u32 20 ("Active Row:Cell Font:Size"), "CellFontBold"=TRUE ("Active Row:Cell Font:Bold")) -> ()  [unwired: 1 in, 2 out]
      }
      event "BD 1 Frequency 1 (MHz)", "BD 1 Frequency 2 (MHz)", "BD 1 Frequency 3 (MHz)", "BD 2 Frequency 1 (MHz)", "BD 2 Frequency 2 (MHz)", "BD 2 Frequency 3 (MHz)", "Trap Delta (MHz)": Value Change {
        # "anytime one of the frequencies is changed, write it to the RF board UNLESS Set 2 is being oscillated. The oscillation\nscript writes the frequencies to the RF board."
        n458 = event-data() -> ("CtlRef"=w801:refnum<vi>)  [unwired: 6 out]
        n459 = control-ref of="Trap Delta (MHz)"() -> (w800:refnum<vi>)
        n460 = Equal?(x=w800, y=w801) -> (x = y?=w799:bool)
        n461 = case shown="False" "Oscillate Set 2" {
          tunnel: w804 -> [w824 _]
          tunnel: [w823 w827] -> w803
          tunnel: w802 -> [w822 w827]
          tunnel: w799 -> [w808 _]
          frame False {
            n462 = local read "BD 1 Frequency 1 (MHz)"() -> (w806:dbl)
            n463 = local read "BD 1 Frequency 2 (MHz)"() -> (w810:dbl)
            n464 = Add(x=w806, y="Trap Delta (MHz)") -> (x+y=w809:dbl)
            n465 = Select(t=w809, s=w808, f=w810) -> (s? t:f=w807:dbl)
            n466 = local read "Y RF Frequency Limits (MHz)"() -> (w812:T16)
            n467 = local read "X RF Frequency Limits (MHz)"() -> (w813:T16)
            n468 = local read "BD 1 Frequency 3 (MHz)"() -> (w825:dbl)
            n469 = local write "BD 1 Frequency 2 (MHz)"(w807) -> ()
            n470 = local read "BD 2 Frequency 1 (MHz)"() -> (w816:dbl)
            n471 = local read "BD 2 Frequency 2 (MHz)"() -> (w815:dbl)
            n472 = local read "BD 2 Frequency 3 (MHz)"() -> (w826:dbl)
            n473 = call "set RF board frequency - interlace.vi"("Board 2 Frequency Limits"=w812, "Board 1 Frequency Limits"=w813, "error in"=w822, "FPGA VI Reference In"=w824, "Board 2 Frequency 3 (MHz)"=w826, "Board 1 Frequency 3 (MHz)"=w825, "Board 2 Frequency 2 (MHz)"=w815, "Board 2 Frequency 1 (MHz)"=w816, "Board 1 Frequency 2 (MHz)"=w807, "Board 1 Frequency 1  (MHz)"=w806) -> ("error out"=w823:errorcluster)  [unwired: 1 out]
            n474 = Subtract(x=w816, y=w815) -> (x-y=w820:dbl)
            n475 = Subtract(x=w807, y=w806) -> (x-y=w821:dbl)
            n476 = Square(x=w820) -> (x^2=w818:dbl)
            n477 = Square(x=w821) -> (x^2=w819:dbl)
            n478 = Add(x=w819, y=w818) -> (x+y=w817:dbl)
            n479 = Square Root(x=w817) -> (sqrt(x)=w814:dbl)
            n480 = local write "Trap Delta (MHz)"(w814) -> ()
            n481 = property on="Initial delta (MHz)" class="DigNum (strict)"("Val(Sgnl)"=w814) -> ()  [unwired: 2 in, 2 out]
          }
          frame True {
          }
        }
      }
      event "Round T1 X": Value Change {
        n482 = event-data() -> ()  [unwired: 7 out]
        n483 = local read "BD 1 Frequency 1 (MHz)"() -> (w830:dbl)
        n484 = Round To Nearest(number=w830) -> (nearest integer value=w829:dbl)
        n485 = property on="BD 1 Frequency 1 (MHz)" class="DigNum (strict)"("Val(Sgnl)"=w829) -> ()  [unwired: 2 in, 2 out]
      }
      event "Restart RF": Value Change {
        n486 = event-data() -> ()  [unwired: 7 out]
        n487 = xnode "Read/Write Control"("FPGA VI Reference In"=w868, "error in"=w863, "FPGA Controls  RF Box"=FALSE) -> ("FPGA VI Reference Out"=w867:T19, "error out"=w862:errorcluster)
        n488 = local read "Y RF Amplitude Limits (%)"() -> (w843:T16)
        n489 = local read "X RF Amplitude Limits (%)"() -> (w844:T16)
        n490 = local read "X RF Frequency Limits (MHz)"() -> (w846:T16)
        n491 = local read "Y RF Frequency Limits (MHz)"() -> (w845:T16)
        n492 = xnode "Read/Write Control"("FPGA VI Reference In"=w867, "error in"=w862, "Direct RF Box  Communication"=TRUE) -> ("FPGA VI Reference Out"=w866:T19, "error out"=w861:errorcluster)
        n493 = local read "BD 2 Frequency 3 (MHz)"() -> (w853:dbl)
        n494 = local read "BD 2 Frequency 2 (MHz)"() -> (w854:dbl)
        n495 = local read "BD 1 Frequency 3 (MHz)"() -> (w857:dbl)
        n496 = local read "BD 1 Frequency 1 (MHz)"() -> (w858:dbl)
        n497 = local read "BD 2 Frequency 1 (MHz)"() -> (w855:dbl)
        n498 = local read "BD 1 Frequency 2 (MHz)"() -> (w856:dbl)
        n499 = call "Initialize RF boards - interlace 3.vi"("error in"=w861, "FPGA VI Reference In"=w866) -> ("error out"=w860:errorcluster, "FPGA VI Reference Out"=w865:T19)
        n500 = local read "BD 2 Amplitude 2 (%)"() -> (w848:dbl)
        n501 = local read "BD 2 Amplitude 1 (%)"() -> (w849:dbl)
        n502 = local read "BD 2 Amplitude 3 (%)"() -> (w847:dbl)
        n503 = local read "BD 1 Amplitude 3 (%)"() -> (w852:dbl)
        n504 = local read "BD 1 Amplitude 1 (%)"() -> (w851:dbl)
        n505 = local read "BD 1 Amplitude 2 (%)"() -> (w850:dbl)
        n506 = call "set RF board frequency - interlace.vi"("Board 2 Frequency Limits"=w845, "Board 1 Frequency Limits"=w846, "error in"=w860, "FPGA VI Reference In"=w865, "Board 2 Frequency 3 (MHz)"=w853, "Board 1 Frequency 3 (MHz)"=w857, "Board 2 Frequency 2 (MHz)"=w854, "Board 2 Frequency 1 (MHz)"=w855, "Board 1 Frequency 2 (MHz)"=w856, "Board 1 Frequency 1  (MHz)"=w858) -> ("error out"=w859:errorcluster, "FPGA VI Reference Out"=w864:T19)
        n507 = call "set RF board amplitude - interlace.vi"("Board 2 Amplitude Limits"=w843, "Board 1 Amplitude Limits"=w844, "error in"=w859, "FPGA VI Reference In"=w864, "Board 2 Amplitude 3 (%)"=w847, "Board 1 Amplitude 3 (%)"=w852, "Board 2 Amplitude 2 (%)"=w848, "Board 2 Amplitude 1 (%)"=w849, "Board 1 Amplitude 2 (%)"=w850, "Board 1 Amplitude 1 (%)"=w851) -> ("error out"=w836:errorcluster, "FPGA VI Reference Out"=w840:T19)
        n508 = xnode "Read/Write Control"("FPGA VI Reference In"=w840, "error in"=w836, "Direct RF Box  Communication"=FALSE) -> ("FPGA VI Reference Out"=w839:T19, "error out"=w838:errorcluster)
        n509 = flat-sequence {
          tunnel: w838 -> [w869]
          tunnel: [w869] -> w837
          frame #0 {
            n510 = Wait (ms)(milliseconds to wait=u32 50) -> ()  [unwired: 1 out]
          }
        }
        n511 = xnode "Read/Write Control"("FPGA VI Reference In"=w839, "error in"=w837, "FPGA Controls  RF Box"=TRUE) -> ("error out"=w832:errorcluster)  [unwired: 1 out]
        n512 = property on="Restart RF" class="Bool (strict)"(error in=w832, "Value"=FALSE ("Restart RF")) -> (error out=w831:errorcluster)  [unwired: 1 in, 1 out]
      }
      event "Round T2 X": Value Change {
        n513 = event-data() -> ()  [unwired: 7 out]
        n514 = local read "BD 1 Frequency 2 (MHz)"() -> (w872:dbl)
        n515 = Round To Nearest(number=w872) -> (nearest integer value=w871:dbl)
        n516 = property on="BD 1 Frequency 2 (MHz)" class="DigNum (strict)"("Val(Sgnl)"=w871) -> ()  [unwired: 2 in, 2 out]
      }
      event "Stop All": Value Change {
        n517 = event-data() -> ()  [unwired: 7 out]
        n518 = call "hamilton_controller.vi"("action"=T20."DISCONNECT") -> ()  [unwired: 10 in, 1 out]
        n519 = local read "Stop All"() -> (w875:bool)
      }
      event "Delayed Interlace Start": Value Change {
        n520 = event-data() -> ()  [unwired: 7 out]
        n521 = flat-sequence {
          frame #0 {
            n522 = Multiply(x="Delay to Interlace (s)", y=1000.0) -> (x*y=w878:dbl)
            n523 = Wait (ms)(milliseconds to wait=w878) -> ()  [unwired: 1 out]
          }
          frame #1 {
            n524 = property on="Green laser mode" class="RadioBtnsControl (strict)"("Val(Sgnl)"=enum32{"Laser ON", "Laser OFF", "Interlace"}."Interlace" ("Value (Signaling)")) -> ()  [unwired: 2 in, 2 out]
          }
        }
      }
      event "BD 1 Amplitude 1 (%)", "BD 1 Amplitude 2 (%)", "BD 1 Amplitude 3 (%)", "BD 2 Amplitude 1 (%)", "BD 2 Amplitude 2 (%)", "BD 2 Amplitude 3 (%)", "Trap 1 ON", "Trap 2 ON", "Trap 3 ON", "Feedback On/Off", "All FB On/Off": Value Change {
        w902 = i16 1 ("f")
        n525 = event-data() -> ()  [unwired: 7 out]
        n526 = local write "Trap 1 (ON/OFF)"("Trap 1 ON") -> ()
        n527 = local write "Trap 2 (ON/OFF)"("Trap 2 ON") -> ()
        n528 = Boolean To (0,1)(Boolean="Trap 3 ON") -> (0, 1=w903:i16)
        n529 = Boolean To (0,1)(Boolean="Trap 1 ON") -> (0, 1=w904:i16)
        n530 = Boolean To (0,1)(Boolean="Trap 2 ON") -> (0, 1=w905:i16)
        n531 = Select(t=w905, s="Trap ON/OFF X or Y Amp?", f=w902) -> (s? t:f=w900:i16)
        n532 = Select(t=w904, s="Trap ON/OFF X or Y Amp?", f=w902) -> (s? t:f=w901:i16)
        n533 = Select(t=w903, s="Trap ON/OFF X or Y Amp?", f=w902) -> (s? t:f=w899:i16)
        n534 = Select(t=w902, s="Trap ON/OFF X or Y Amp?", f=w905) -> (s? t:f=w897:i16)
        n535 = Select(t=w902, s="Trap ON/OFF X or Y Amp?", f=w904) -> (s? t:f=w898:i16)
        n536 = Select(t=w902, s="Trap ON/OFF X or Y Amp?", f=w903) -> (s? t:f=w896:i16)
        n537 = And(x="All FB On/Off", y="Feedback On/Off") -> (x .and. y?=w894:cluster{"Set 1":bool, "Set 2":bool})
        n538 = local read "BD 1 Amplitude 1 (%)"() -> (w914:dbl)
        n539 = local read "BD 1 Amplitude 2 (%)"() -> (w913:dbl)
        n540 = local read "BD 1 Amplitude 3 (%)"() -> (w912:dbl)
        n541 = Unbundle By Name(w894) -> ("Set 1"=w889:bool, "Set 2"=w886:bool)
        n542 = local read "Y RF Amplitude Limits (%)"() -> (w882:T16)
        n543 = local read "X RF Amplitude Limits (%)"() -> (w883:T16)
        n544 = local read "BD 2 Amplitude 1 (%)"() -> (w915:dbl)
        n545 = local read "BD 2 Amplitude 2 (%)"() -> (w916:dbl)
        n546 = local read "BD 2 Amplitude 3 (%)"() -> (w917:dbl)
        n547 = And(x="Trap 2 ON", y=w886) -> (x .and. y?=w884:bool)
        n548 = And(x="Trap 1 ON", y=w889) -> (x .and. y?=w887:bool)
        n549 = Multiply(x=w901, y=w914) -> (x*y=w909:dbl)
        n550 = Multiply(x=w913, y=w900) -> (x*y=w907:dbl)
        n551 = Multiply(x=w912, y=w899) -> (x*y=w908:dbl)
        n552 = Multiply(x=w915, y=w898) -> (x*y=w918:dbl)
        n553 = Multiply(x=w916, y=w897) -> (x*y=w919:dbl)
        n554 = Multiply(x=w917, y=w896) -> (x*y=w920:dbl)
        n555 = call "set RF board amplitude - interlace.vi"("Board 2 Amplitude Limits"=w882, "Board 1 Amplitude Limits"=w883, "error in"=w910, "FPGA VI Reference In"=w911, "Board 2 Amplitude 3 (%)"=w920, "Board 1 Amplitude 3 (%)"=w908, "Board 2 Amplitude 2 (%)"=w919, "Board 2 Amplitude 1 (%)"=w918, "Board 1 Amplitude 2 (%)"=w907, "Board 1 Amplitude 1 (%)"=w909) -> ("error out"=w891:errorcluster, "FPGA VI Reference Out"=w892:T19)
        n556 = xnode "Read/Write Control"("FPGA VI Reference In"=w892, "error in"=w891, "FB On/Off Set 1"=w887, "FB On/Off Set 2"=w884) -> ("error out"=w890:errorcluster)  [unwired: 1 out]
      }
      event "Load parameters": Value Change {
        n557 = event-data() -> ()  [unwired: 7 out]
        n558 = property on="Saved AOD Raster Scan Parameter Sets" class="Arr (strict)"() -> ("Index Values"=w931:u32[])  [unwired: 2 in, 2 out]
        n559 = Index Array(array=w931, index=0) -> (element=w928:u32)
        n560 = local write "Load parameters"(FALSE ("Load parameters")) -> ()
        n561 = Index Array(array="Saved AOD Raster Scan Parameter Sets", index=w928) -> (element=w927:T30)
        n562 = Unbundle By Name(w927) -> ("Scan Range AOD (nm) 2"=w926:dbl, "Step Size AOD (nm) 2"=w925:dbl, "Scan Speed AOD (nm/s) 2"=w924:dbl, "Number of scans (AOD) 2"=w923:u16)
        n563 = flat-sequence {
          tunnel: w926 -> [w934]
          tunnel: w925 -> [w933]
          tunnel: w924 -> [w932]
          tunnel: w923 -> [w935]
          frame #0 {
            n564 = local write "Scan Speed (nm/s)"(w932) -> ()
            n565 = local write "Scan Range (nm)"(w934) -> ()
            n566 = local write "Step Size (nm)"(w933) -> ()
          }
          frame #1 {
            n567 = property on="Number of F/B Scans (AOD)" class="DigNum (strict)"("Val(Sgnl)"=w935) -> ()  [unwired: 2 in, 2 out]
          }
        }
      }
      event "Trap 1 (ON/OFF)", "Trap 2 (ON/OFF)": Value Change {
        n568 = event-data() -> ()  [unwired: 7 out]
        n569 = property on="Trap 2 ON" class="Bool (strict)"("Val(Sgnl)"="Trap 2 (ON/OFF)") -> ()  [unwired: 2 in, 2 out]
        n570 = property on="Trap 1 ON" class="Bool (strict)"("Val(Sgnl)"="Trap 1 (ON/OFF)") -> ()  [unwired: 2 in, 2 out]
      }
      event "DIO count 1 (ticks)", "DIO count 2 (ticks)", "DIO count 3 (ticks)", "Interlace", "Number Interlace Sets", "Not-Interlacing Set": Value Change {
        n571 = event-data() -> ()  [unwired: 7 out]
        n572 = local read "DIO count 3 (ticks)"() -> (w948:u32)
        n573 = local read "DIO count 1 (ticks)"() -> (w950:u32)
        n574 = local read "DIO count 2 (ticks)"() -> (w949:u32)
        n575 = To Unsigned Byte Integer(number="Not-Interlacing Set") -> (unsigned 8bit integer=w939:u8)
        n576 = Add(x=w939, y=u8 1) -> (x+y=w943:u8)
        n577 = xnode "Read/Write Control"("FPGA VI Reference In"=w954, "error in"=w952, "DIO count 1 (ticks)"=w950, "DIO count 2 (ticks)"=w949, "DIO count 3 (ticks)"=w948, "Interlace ON/OFF"="Interlace", "Number Interlace Cycles"="Number Interlace Sets", "Interlace Off Parameters"=w943) -> ("error out"=w953:errorcluster)  [unwired: 1 out]
        n578 = Build Array(w950, w949, w948) -> (w941:u32[])
        n579 = Split 1D Array(array=w941, index="Number Interlace Sets") -> (first subarray=w951:u32[])  [unwired: 1 out]
        n580 = Index Array(array=w941, index=w939) -> (element=w940:u32)
        n581 = Add Array Elements(numeric array=w951) -> (sum=w945:u32)
        n582 = Select(t=w945, s="Interlace", f=w940) -> (s? t:f=→"Total Counts (ticks)":u32)
      }
      event "Reset Feedback": Value Change {
        n583 = event-data() -> ()  [unwired: 7 out]
        n584 = Unbundle By Name("Reset Feedback") -> ("Set 1"=w958:bool, "Set 2"=w957:bool)
        n585 = xnode "Read/Write Control"("FPGA VI Reference In"=w960, "error in"=w955, "FB Reset Set 1"=w958, "FB Reset Set 2"=w957) -> ("error out"=w956:errorcluster)  [unwired: 1 out]
      }
      event "PID Gains": Value Change {
        n586 = event-data() -> ()  [unwired: 7 out]
        n587 = Unbundle By Name("PID Gains") -> ("Set 1"=w964:T14, "Set 2"=w963:T14)
        n588 = xnode "Read/Write Control"("FPGA VI Reference In"=w965, "error in"=w961, "FB Gains Set 1"=w964, "FB Gains Set 2"=w963) -> ("error out"=w962:errorcluster)  [unwired: 1 out]
      }
      event "AI2 to Setpoint", "Trap Intensity\nSetpoints (V)": Value Change {
        n589 = event-data() -> ()  [unwired: 7 out]
        n590 = xnode "Read/Write Control"("FPGA VI Reference In"=w971, "error in"=w967) -> ("FPGA VI Reference Out"=w970:T19, "error out"=w969:errorcluster, "AI2 Y Sum Set 1"=w978:i16, "AI2 Y Sum Set 2"=w977:i16)
        n591 = Cluster To Array(cluster="AI2 to Setpoint") -> (array=w981:bool[])
        n592 = local read "AI2 (V)"() -> (w979:cluster{"Set 1":dbl, "Set 2":dbl})
        n593 = Or Array Elements(Boolean array=w981) -> (logical OR=w982:bool)
        n594 = Bundle By Name(cluster=w979, "Set 1"=w978, "Set 2"=w977) -> (w976:cluster{"Set 1":dbl, "Set 2":dbl})
        n595 = Divide(x=w976, y=3276.7) -> (x/y=w975:cluster{"Set 1":dbl, "Set 2":dbl})
        "AI2 (V)" <- w975
        n596 = case shown="True" w982 {
          tunnel: [w985 w1002] -> w974
          tunnel: "AI2 to Setpoint" -> [_ w998]
          tunnel: "Trap Intensity\nSetpoints (V)" -> [w986 w1001]
          tunnel: w975 -> [_ w995]
          frame False {
            n597 = Multiply(x=3276.7, y=w986) -> (x*y=w987:cluster{"Set 1":dbl, "Set 2":dbl})
            n598 = To Word Integer(number=w987) -> (16bit integer=w985:cluster{"Set 1":i16, "Set 2":i16})
          }
          frame True {
            n599 = Unbundle By Name(w995) -> ("Set 1"=w994:dbl, "Set 2"=w993:dbl)
            n600 = Unbundle By Name(w1001) -> ("Set 1"=w1000:dbl, "Set 2"=w999:dbl)
            n601 = Unbundle By Name(w998) -> ("Set 1"=w997:bool, "Set 2"=w996:bool)
            n602 = Select(t=w994, s=w997, f=w1000) -> (s? t:f=w992:dbl)
            n603 = Select(t=w993, s=w996, f=w999) -> (s? t:f=w991:dbl)
            n604 = Bundle By Name(cluster=w1001, "Set 1"=w992, "Set 2"=w991) -> (w989:cluster{"Set 1":dbl, "Set 2":dbl})
            n605 = local write "Trap Intensity\nSetpoints (V)"(w989) -> ()
            n606 = Multiply(x=3276.7, y=w989) -> (x*y=w990:cluster{"Set 1":dbl, "Set 2":dbl})
            n607 = To Word Integer(number=w990) -> (16bit integer=w1002:cluster{"Set 1":i16, "Set 2":i16})
          }
        }
        n608 = Unbundle By Name(w974) -> ("Set 1"=w973:i16, "Set 2"=w972:i16)
        n609 = xnode "Read/Write Control"("FPGA VI Reference In"=w970, "error in"=w969, "FB Setpoint Set 1"=w973, "FB Setpoint Set 2"=w972) -> ("error out"=w968:errorcluster)  [unwired: 1 out]
      }
      event "Invert GI": Value Change {
        n610 = event-data() -> ()  [unwired: 7 out]
        n611 = xnode "Read/Write Control"("FPGA VI Reference In"=w1007, "error in"=w1005, "Invert GI"="Invert GI", "Invert GI 2"="Invert GI") -> ("error out"=w1006:errorcluster)  [unwired: 1 out]
      }
      event "Green FB Setpoint (mV)", "Green FB Gains", "Green FB On/Off", "Current When FB OFF (%)", "Green int current ON count adj": Value Change {
        n612 = event-data() -> ()  [unwired: 7 out]
        n613 = local read "Green FB Setpoint (mV)"() -> (w1014:dbl)
        n614 = local read "Current When FB OFF (%)"() -> (w1017:dbl)
        n615 = Multiply(x=w1014, y=3.2767) -> (x*y=w1013:dbl)
        n616 = Multiply(x=w1017, y=655.35) -> (x*y=w1018:dbl)
        n617 = To Unsigned Word Integer(number=w1018) -> (unsigned 16bit integer=w1016:u16)
        n618 = local read "Green int current ON count adj"() -> (w1021:u32)
        n619 = local read "Green FB Gains"() -> (w1020:T14)
        n620 = local read "Green Laser ON/Interlacing"() -> (w1011:bool)
        n621 = local read "Green laser mode"() -> (w1010:enum32{"Laser ON", "Laser OFF", "Interlace"})
        n622 = local read "Green FB On/Off"() -> (w1022:bool)
        n623 = Equal?(x=w1010, y=enum32{"Laser ON", "Laser OFF", "Interlace"}."Interlace") -> (x = y?=w1008:bool)
        n624 = Compound Arithmetic op=AND(w1008, w1022, w1011) -> (w1012:bool)
        n625 = xnode "Read/Write Control"("FPGA VI Reference In"=w1025, "error in"=w1024, "Green FB Setpoint"=w1013, "Green FB On/Off"=w1012, "Current Out"=w1016, "Green int current ON count adj"=w1021, "Green FB Gains"=w1020) -> ("error out"=w1023:errorcluster)  [unwired: 1 out]
      }
      event "Green laser mode", "Green Laser ON/Interlacing": Value Change {
        n626 = event-data() -> ()  [unwired: 7 out]
        n627 = case shown="True" "Green Laser ON/Interlacing" {
          tunnel: "Green laser mode" -> [_ w1039]
          tunnel: [enum32{"Laser ON", "Laser OFF", "Interlace"}."Laser OFF" ("Green laser mode") w1039] -> w1027
          tunnel: [FALSE w1035] -> w1026
          frame False {
          }
          frame True {
            n628 = local read "Green FB On/Off"() -> (w1036:bool)
            n629 = Equal?(x=w1039, y=enum32{"Laser ON", "Laser OFF", "Interlace"}."Interlace") -> (x = y?=w1037:bool)
            n630 = And(x=w1037, y=w1036) -> (x .and. y?=w1035:bool)
          }
        }
        n631 = xnode "Read/Write Control"("FPGA VI Reference In"=w1032, "error in"=w1030, "Operating Mode"=w1027, "Operating Mode 2"=w1027, "Green FB On/Off"=w1026) -> ("error out"=w1031:errorcluster)  [unwired: 1 out]
      }
      event "- phase (APD 1 Gate)", "+ phase (APD 1 Gate)": Value Change {
        n632 = event-data() -> ()  [unwired: 7 out]
        n633 = local read "Phase Adj. (APD 1 Gate)"() -> (w1040:i16)
        n634 = Negate(x=w1040) -> (-x=w1048:i16)
        n635 = Select(t=w1048, s="- phase (APD 1 Gate)", f=w1040) -> (s? t:f=w1047:i16)
        n636 = Or(x="- phase (APD 1 Gate)", y="+ phase (APD 1 Gate)") -> (x .or. y?=w1043:bool)
        n637 = xnode "Read/Write Control"("FPGA VI Reference In"=w1050, "error in"=w1049, "Phase count adjustment (APD 1 Gate)"=w1047) -> ("FPGA VI Reference Out"=w1045:T19, "error out"=w1046:errorcluster)
        n638 = xnode "Read/Write Control"("FPGA VI Reference In"=w1045, "error in"=w1046, "+ phase (APD 1 Gate)"=w1043) -> ("error out"=w1044:errorcluster)  [unwired: 1 out]
      }
      event "+ phase (APD 2 Gate)", "- phase (APD 2 Gate)": Value Change {
        n639 = event-data() -> ()  [unwired: 7 out]
        n640 = local read "Phase Adj. (APD 2 Gate)"() -> (w1051:i16)
        n641 = Negate(x=w1051) -> (-x=w1059:i16)
        n642 = Select(t=w1059, s="- phase (APD 2 Gate)", f=w1051) -> (s? t:f=w1058:i16)
        n643 = Or(x="- phase (APD 2 Gate)", y="+ phase (APD 2 Gate)") -> (x .or. y?=w1054:bool)
        n644 = xnode "Read/Write Control"("FPGA VI Reference In"=w1061, "error in"=w1060, "Phase count adjustment (APD 2 Gate)"=w1058) -> ("FPGA VI Reference Out"=w1056:T19, "error out"=w1057:errorcluster)
        n645 = xnode "Read/Write Control"("FPGA VI Reference In"=w1056, "error in"=w1057, "+ phase (APD 2 Gate)"=w1054) -> ("error out"=w1055:errorcluster)  [unwired: 1 out]
      }
      event "Phase Adj. (APD Acq)", "+ phase (APD Acq)", "- phase (APD Acq)": Value Change {
        n646 = event-data() -> ()  [unwired: 7 out]
        n647 = local read "Phase Adj. (APD Acq)"() -> (w1064:i16)
        n648 = Negate(x=w1064) -> (-x=w1070:i16)
        n649 = Select(t=w1070, s="+ phase (APD Acq)", f=w1064) -> (s? t:f=w1069:i16)
        n650 = Or(x="+ phase (APD Acq)", y="- phase (APD Acq)") -> (x .or. y?=w1065:bool)
        n651 = xnode "Read/Write Control"("FPGA VI Reference In"=w1072, "error in"=w1071, "Phase Count Adjustment (APD Acq)"=w1069) -> ("FPGA VI Reference Out"=w1067:T19, "error out"=w1068:errorcluster)
        n652 = xnode "Read/Write Control"("FPGA VI Reference In"=w1067, "error in"=w1068, "+ phase (APD Acq)"=w1065) -> ("error out"=w1066:errorcluster)  [unwired: 1 out]
      }
      event "Phase adj. (GI)", "+ phase (GI)", "- phase (GI)": Value Change {
        n653 = event-data() -> ()  [unwired: 7 out]
        n654 = Negate(x="Phase adj. (GI)") -> (-x=w1081:i16)
        n655 = Select(t=w1081, s="+ phase (GI)", f="Phase adj. (GI)") -> (s? t:f=w1080:i16)
        n656 = Or(x="+ phase (GI)", y="- phase (GI)") -> (x .or. y?=w1076:bool)
        n657 = xnode "Read/Write Control"("FPGA VI Reference In"=w1083, "error in"=w1082, "Phase count adjustment (GI)"=w1080) -> ("FPGA VI Reference Out"=w1078:T19, "error out"=w1079:errorcluster)
        n658 = xnode "Read/Write Control"("FPGA VI Reference In"=w1078, "error in"=w1079, "+ phase (GI)"=w1076) -> ("error out"=w1077:errorcluster)  [unwired: 1 out]
      }
      event "Phase adj. (GI) 2", "+ phase (GI) 2", "- phase (GI) 2": Value Change {
        n659 = event-data() -> ()  [unwired: 7 out]
        n660 = Negate(x="Phase adj. (GI) 2") -> (-x=w1092:i16)
        n661 = Select(t=w1092, s="+ phase (GI) 2", f="Phase adj. (GI) 2") -> (s? t:f=w1091:i16)
        n662 = Or(x="+ phase (GI) 2", y="- phase (GI) 2") -> (x .or. y?=w1087:bool)
        n663 = xnode "Read/Write Control"("FPGA VI Reference In"=w1094, "error in"=w1093, "Phase count adjustment (GI) 2"=w1091) -> ("FPGA VI Reference Out"=w1089:T19, "error out"=w1090:errorcluster)
        n664 = xnode "Read/Write Control"("FPGA VI Reference In"=w1089, "error in"=w1090, "+ phase (GI) 2"=w1087) -> ("error out"=w1088:errorcluster)  [unwired: 1 out]
      }
      event "Phase adj. (Green FB)", "- phase (Green FB)", "+ phase (Green FB)": Value Change {
        n665 = event-data() -> ()  [unwired: 7 out]
        n666 = Negate(x="Phase adj. (Green FB)") -> (-x=w1103:i16)
        n667 = Select(t=w1103, s="+ phase (Green FB)", f="Phase adj. (Green FB)") -> (s? t:f=w1102:i16)
        n668 = Or(x="+ phase (Green FB)", y="- phase (Green FB)") -> (x .or. y?=w1098:bool)
        n669 = xnode "Read/Write Control"("FPGA VI Reference In"=w1105, "error in"=w1104, "Phase count adjustment (Green FB)"=w1102) -> ("FPGA VI Reference Out"=w1100:T19, "error out"=w1101:errorcluster)
        n670 = xnode "Read/Write Control"("FPGA VI Reference In"=w1100, "error in"=w1101, "+ phase (Green FB)"=w1098) -> ("error out"=w1099:errorcluster)  [unwired: 1 out]
      }
      event "Invert APD Gate", "APD Gate ON Count", "APD Gate OFF Count", "APD Gate", "APD Integration Time (s)", "APD 1 AO Mult.", "APD 2 AO Mult.": Value Change {
        n671 = event-data() -> ()  [unwired: 7 out]
        n672 = local read "APD Integration Time (s)"() -> (w1106:dbl)
        n673 = local read "APD Gate ON Count"() -> (w1119:u32)
        n674 = local read "APD Gate OFF Count"() -> (w1118:u32)
        n675 = local read "Invert APD Gate"() -> (w1120:bool)
        n676 = local read "APD Gate"() -> (w1117:enum32{"ON", "OFF", "Interlace"})
        n677 = Multiply(x=w1106, y=40000000.0) -> (x*y=w1115:dbl)
        n678 = Reciprocal(x=w1106) -> (1/x=→"APD Acq Rate (Hz)":dbl)
        n679 = To Unsigned Long Integer(number=w1115) -> (unsigned 32bit integer=w1114:u32)
        n680 = local read "DMA Update Period (s)"() -> (w1107:dbl)
        n681 = Divide(x=w1107, y=w1106) -> (x/y=w1110:dbl)
        n682 = local read "APD 1 AO Mult."() -> (w1112:i16)
        n683 = local read "APD 2 AO Mult."() -> (w1111:i16)
        n684 = Multiply(x=2.0, y=w1110) -> (x*y=w1109:dbl)
        n685 = local write "APD Samples/FIFO Acq."(w1110) -> ()
        n686 = local write "APD Elements/DMA read"(w1109) -> ()
        n687 = xnode "Read/Write Control"("FPGA VI Reference In"=w1123, "error in"=w1122, "Invert APD Gate"=w1120, "APD Gate ON Count"=w1119, "APD Gate OFF Count"=w1118, "APD Acq Rate Count"=w1114, "APD Gate Operating Mode"=w1117, "APD 1 AO scale factor"=w1112, "APD 2 AO scale factor"=w1111) -> ("error out"=w1121:errorcluster)  [unwired: 1 out]
      }
      event "GI Frequency, ON count", "Green FB Count", "GI Frequency, OFF count": Value Change {
        n688 = event-data() -> ()  [unwired: 7 out]
        n689 = xnode "Read/Write Control"("FPGA VI Reference In"=w1129, "error in"=w1127, "Green interlace ON count"="GI Frequency, ON count", "Green interlace OFF count"="GI Frequency, OFF count", "Green interlace ON count 2"="GI Frequency, ON count", "Green interlace OFF count 2"="GI Frequency, OFF count", "Green FB Count"="Green FB Count") -> ("error out"=w1128:errorcluster)  [unwired: 1 out]
      }
      event "Number of F/B Scans (AOD)", "Scan Speed (nm/s)", "Scan BD", "Initial delta (MHz)", "Step Size (nm)", "Scan Range (nm)": Value Change {
        w1191 = 123.0  # AOM cal (nm/MHz)
        n690 = event-data() -> ()  [unwired: 7 out]
        n691 = local read "BD 1 Frequency 1 (MHz)"() -> (w1174:dbl)
        n692 = local read "AOM X Cal (nm/MHz)"() -> (w1166:dbl)
        n693 = local read "X RF Frequency Limits (MHz)"() -> (w1178:T16)
        n694 = local read "Y RF Frequency Limits (MHz)"() -> (w1175:T16)
        n695 = local read "BD 2 Frequency 1 (MHz)"() -> (w1180:dbl)
        n696 = Negate(x="Scan Range (nm)") -> (-x=w1144:dbl)
        n697 = Divide(x=w1144, y=w1166) -> (x/y=w1148:dbl)
        n698 = Select(t=w1178, s="Scan BD", f=w1175) -> (s? t:f=w1177:T16)
        n699 = Select(t=w1174, s="Scan BD", f=w1180) -> (s? t:f=w1179:dbl)
        n700 = Unbundle By Name(w1177) -> ("Maximum"=w1186:dbl, "Minimum"=w1185:dbl)
        n701 = Add(x=w1148, y=w1179) -> (x+y=w1183:dbl)
        n702 = Divide(x=w1144, y="Step Size (nm)") -> (x/y=w1163:dbl)
        n703 = Divide(x="Step Size (nm)", y=w1166) -> (x/y=w1172:dbl)
        n704 = Absolute Value(x=w1163) -> (abs(x)=w1147:dbl)
        n705 = Sign(1:w1144) -> (0:w1145:dbl)
        n706 = In Range and Coerce(upper limit=w1186, x=w1183, lower limit=w1185) -> (coerced(x)=w1182:dbl, In Range?=w1184:bool)
        n707 = To Unsigned Quad Integer(1:w1147) -> (0:w1162:u64)
        "Scan steps (AOD)" <- w1162
        n708 = call "IR AOM freq to word.vi"("Frequency In (MHz)"=w1172) -> ("Frequency Word Out (double)"=w1169:dbl)
        n709 = Multiply(x=w1145, y=w1169) -> (x*y=w1146:dbl)
        n710 = Subtract(x=w1183, y=w1182) -> (x-y=w1181:dbl)
        n711 = To Quad Integer(1:w1146) -> (0:w1168:i64)
        "Incr. int (AOD)" <- w1168
        n712 = Subtract(x=w1148, y=w1181) -> (x-y=w1167:dbl)
        "Scan Range (MHz)" <- w1167
        n713 = Select(t=w1148, s=w1184, f=w1167) -> (s? t:f=w1187:dbl)
        n714 = Multiply(x=w1167, y=w1166) -> (x*y=w1165:dbl)
        n715 = Decrement(x=w1162) -> (x-1=w1215:u64)
        n716 = Negate(x=w1165) -> (-x=w1161:dbl)
        n717 = local write "Scan Range (nm)"(w1161) -> ()
        n718 = Divide(x=w1187, y=w1215) -> (x/y=w1171:dbl)
        "Scan Increment (MHz)" <- w1171
        n719 = call "IR AOM freq to word.vi"("Frequency In (MHz)"=w1171) -> ("Frequency Word Out (double)"=w1170:dbl)
        n720 = Divide(x="Step Size (nm)", y="Scan Speed (nm/s)") -> (x/y=w1158:dbl)
        n721 = To Quad Integer(1:w1170) -> ()  [unwired: 1 out]
        n722 = local read "Number Interlace Sets"() -> (w1142:u8)
        n723 = local read "AI Count (ticks)"() -> (w1143:u32)
        n724 = local read "Total Counts (ticks)"() -> (w1141:u32)
        n725 = local read "# Samples/trap"() -> (w1173:u32)
        n726 = Multiply(x=w1143, y=w1142) -> (x*y=w1140:u32)
        n727 = Divide(x=w1141, y=w1140) -> (x/y=w1139:dbl)
        n728 = Select(t=w1174, s="Scan BD", f=w1180) -> (s? t:f=w1212:dbl)
        "Initial freq. (MHz)" <- w1212
        n729 = Add(x=w1187, y=w1212) -> (x+y=→"Final freq. (MHz)":dbl)
        n730 = Divide(x=w1141, y=40000000.0) -> (x/y=w1157:dbl)
        n731 = Divide(x=w1158, y=w1157) -> (x/y=w1156:dbl)
        n732 = To Unsigned Quad Integer(1:w1156) -> (0:w1131:u64)
        n733 = Quotient & Remainder(x=w1131, y=u64 2) -> (x-y*floor(x/y)=w1135:u64)  [unwired: 1 out]
        n734 = Equal?(x=w1135, y=u64 0) -> (x = y?=w1133:bool)
        n735 = Decrement(x=w1131) -> (x-1=w1132:u64)
        n736 = Select(t=w1131, s=w1133, f=w1132) -> (s? t:f=w1130:u64)
        "Cycles/step (AOD)" <- w1130
        n737 = xnode "Read/Write Control"("FPGA VI Reference In"=w1223, "error in"=w1222, "Scan steps"=w1162, "Number of scans"="Number of F/B Scans (AOD)", "Cycles per step"=w1130, "Scan freq.  increment"=w1168, "Scan BD"="Scan BD") -> ("error out"=w1221:errorcluster)  [unwired: 1 out]
        n738 = Multiply(x=w1162, y=w1130) -> (x*y=w1216:u64)
        n739 = Multiply(x=w1216, y=u64 2) -> (x*y=w1138:u64)
        n740 = Multiply(x=w1139, y=w1138) -> (x*y=w1137:dbl)
        "Data points/scan (f/b)" <- w1137
        n741 = Multiply(x=w1137, y="Number of F/B Scans (AOD)") -> (x*y=w1219:dbl)
        "Data points/scans" <- w1219
        n742 = Divide(x=w1219, y=w1173) -> (x/y=→"N sets should be saved":dbl)
        n743 = Multiply(x=w1216, y=w1157) -> (x*y=w1155:dbl)
        "Time/Scan (s) (AOD)" <- w1155
        n744 = Select(t=w1187, s="Scan BD", f=0.0) -> (s? t:f=w1213:dbl)
        n745 = Select(t=0.0, s="Scan BD", f=w1187) -> (s? t:f=w1209:dbl)
        n746 = local read "BD 2 Frequency 2 (MHz)"() -> (w1205:dbl)
        n747 = local read "BD 1 Frequency 2 (MHz)"() -> (w1208:dbl)
        n748 = Add(x=w1209, y=w1180) -> (x+y=w1206:dbl)
        n749 = Add(x=w1174, y=w1213) -> (x+y=w1207:dbl)
        n750 = Multiply(x=w1155, y=2.0) -> (x*y=w1154:dbl)
        n751 = Multiply(x=w1154, y="Number of F/B Scans (AOD)") -> (x*y=w1151:dbl)
        n752 = Divide(x=w1151, y=60.0) -> (x/y=→"Time to Finish All (min)":dbl)
        n753 = Add(x="Trap 2 Bead Size (nm)", y="Trap 1 Bead Size (nm)") -> (x+y=w1195:dbl)
        n754 = local read "Initial delta (MHz)"() -> (w1192:dbl)
        n755 = Divide(x=w1195, y=2.0) -> (x/y=w1189:dbl)
        n756 = Subtract(x=w1206, y=w1205) -> (x-y=w1203:dbl)
        n757 = Subtract(x=w1207, y=w1208) -> (x-y=w1204:dbl)
        n758 = Square(x=w1203) -> (x^2=w1202:dbl)
        n759 = Square(x=w1204) -> (x^2=w1201:dbl)
        n760 = Add(x=w1201, y=w1202) -> (x+y=w1200:dbl)
        n761 = Square Root(x=w1200) -> (sqrt(x)=w1199:dbl)
        "Final delta (MHz)" <- w1199
        n762 = Multiply(x=w1191, y=w1199) -> (x*y=w1198:dbl)
        n763 = Multiply(x=w1192, y=w1191) -> (x*y=w1190:dbl)
        n764 = Subtract(x=w1190, y=w1189) -> (x-y=→"Initial sep (nm)":dbl)
        n765 = Subtract(x=w1198, y=w1189) -> (x-y=→"Final sep (nm)":dbl)
      }
      event "Raster Scanning...": Value Change {
        n766 = event-data() -> ("NewVal"=w1224:bool)  [unwired: 6 out]
        n767 = case shown="True" w1224 {
          frame False {
          }
          frame True {
            n768 = property on="BD 1 Frequency 1 (MHz)" class="DigNum (strict)"("Val(Sgnl)"=65.0 ("Value (Signaling)")) -> ()  [unwired: 2 in, 2 out]
          }
        }
      }
      event "Freq or Amp switch first", "Swap F1 and F2", "Freq switch delay", "Amp switch delay": Value Change {
        n769 = event-data() -> ()  [unwired: 7 out]
        n770 = local read "Freq or Amp switch first"() -> (w1226:bool)
        n771 = local read "Amp switch delay"() -> (w1227:u16)
        n772 = local read "Freq switch delay"() -> (w1229:u16)
        n773 = local read "Swap F1 and F2"() -> (w1228:bool)
        n774 = xnode "Read/Write Control"("FPGA VI Reference In"=w1232, "error in"=w1231, "Freq switch delay"=w1229, "Swap F1 and F2"=w1228, "Amp switch delay"=w1227, "Freq or Amp switch first"=w1226) -> ("error out"=w1230:errorcluster)  [unwired: 1 out]
      }
      event "Scan steps (MCL)", "Number of scans (MCL)", "Scan Range (V)\n(of steps)", "2D or 1D Scan", "N APD Samp/step", "Fast Scan Dir", "Continuous MCL Scanning", "Scan lines (y)": Value Change {
        w1234 = 32767.0 ("y")
        n775 = event-data() -> ()  [unwired: 7 out]
        n776 = Select(t="Scan lines (y)", s="2D or 1D Scan", f="Number of scans (MCL)") -> (s? t:f=w1239:u64)
        n777 = Decrement(x="Scan steps (MCL)") -> (x-1=w1255:u64)
        n778 = Divide(x="Scan Range (V)\n(of steps)", y=w1255) -> (x/y=w1254:dbl)
        "Desired Scan Incr (V)" <- w1254
        n779 = local read "APD Integration Time (s)"() -> (w1247:dbl)
        n780 = Multiply(x=w1254, y=w1234) -> (x*y=w1263:dbl)
        n781 = Divide(x=w1263, y=10.0) -> (x/y=w1253:dbl)
        "Desired incr (int)" <- w1253
        n782 = local read "Update Count (MCL)"() -> (w1259:u32)
        n783 = Round Toward -Infinity(1:w1253) -> (0:w1262:dbl)
        n784 = To Word Integer(number=w1262) -> (16bit integer=w1237:i16)
        "Actual Incr. int (MCL)" <- w1237
        n785 = Multiply(x=w1247, y=40000000.0) -> (x*y=w1260:dbl)
        n786 = Divide(x=w1260, y=w1259) -> (x/y=w1258:dbl)
        n787 = Multiply(x=i16 10, y=w1237) -> (x*y=w1235:i16)
        n788 = Multiply(x="N APD Samp/step", y=w1258) -> (x*y=w1257:dbl)
        "Cycles/step (MCL)" <- w1257
        n789 = Divide(x=w1235, y=w1234) -> (x/y=→"Actual MCL Inc (V)":dbl)
        n790 = Multiply(x="N APD Samp/step", y="Scan steps (MCL)") -> (x*y=w1249:dbl)
        n791 = local read "APD Samples/FIFO Acq."() -> (w1246:dbl)
        n792 = Multiply(x=w1249, y=u64 2) -> (x*y=w1248:dbl)
        "Data points/scan (f+b)" <- w1248
        n793 = Multiply(x=w1248, y=w1239) -> (x*y=w1266:dbl)
        "Data points/scans (MCL)" <- w1266
        n794 = Multiply(x=w1247, y=w1248) -> (x*y=w1240:dbl)
        "Time/f+b scan (s) (MCL)" <- w1240
        n795 = Divide(x=w1266, y=w1246) -> (x/y=→"N sets should be saved (MCL)":dbl)
        n796 = Multiply(x=w1240, y=w1239) -> (x*y=→"Total Time (s)":dbl)
        n797 = Not(x="Fast Scan Dir") -> (.not. x?=w1244:bool)
        n798 = xnode "Read/Write Control"("FPGA VI Reference In"=w1270, "error in"=w1269, "Scan steps (MCL)"="Scan steps (MCL)", "Number of scans (MCL)"=w1239, "Cycles per step (MCL)"=w1257, "Scan freq.  increment (MCL)"=w1237, "1D or 2D Scan?"="2D or 1D Scan", "MCL Scan Axis"=w1244, "Cont. Scan (MCL)"="Continuous MCL Scanning") -> ("error out"=w1268:errorcluster)  [unwired: 1 out]
      }
      event "Read Cal": Value Change {
        w1272 = 1000.0 ("y")
        n799 = event-data() -> ()  [unwired: 7 out]
        n800 = local read "Save file name"() -> (w1297:path)
        n801 = local write "Read Cal"(FALSE ("Read Cal")) -> ()
        n802 = Strip Path(path=w1297) -> (stripped path=w1296:path)  [unwired: 1 out]
        n803 = Path To String(path=w1296) -> (string=w1295:string)
        n804 = Concatenate Strings(w1295, "\\current.cal" ("string")) -> (w1293:string)
        n805 = String To Path(string=w1293) -> (path=w1292:path)
        n806 = Open/Create/Replace File(file path (use dialog)=w1292, operation (0:open)=T23."open", access (0:read/write)=enum16{"read/write", "read-only", "write-only"}."read-only") -> (refnum out=w1300:refnum<file>, error out=w1286:errorcluster)  [unwired: 1 in, 3 out]
        n807 = Deny Access(4:w1286, 7:w1300) -> (0:w1285:errorcluster, 3:w1291:refnum<file>)  [unwired: 1 out]
        n808 = Read from Binary File(5:0.0, 8:w1285, 9:T29."big-endian, network order" ("byte order (0:big-endian, network order)"), 10:-1 ("count (1)"), 11:w1291) -> (0:w1284:errorcluster, 2:w1282:dbl[], 3:w1287:refnum<file>)  [unwired: 2 out]
        n809 = Array To Cluster(array=w1282) -> (cluster=w1281:T31)
        n810 = Unbundle(w1281) -> ("[0]"=w1280:dbl, "[1]"=w1279:dbl, "[2]"=w1278:dbl, "[3]"=w1277:dbl, "[4]"=w1276:dbl, "[5]"=w1275:dbl)
        n811 = Close File(refnum=w1287, error in=w1284) -> (error out=→"Read cal error":errorcluster)  [unwired: 1 out]
        n812 = Multiply(x=w1275, y=w1272) -> (x*y=w1273:dbl)
        n813 = local write "T2 kappa_x (pN/nm)"(w1277) -> ()
        n814 = local write "T1 kappa_x (pN/nm)"(w1278) -> ()
        n815 = local write "T1 alpha_x (nm/V)"(w1280) -> ()
        n816 = local write "T2 alpha_x (nm/V)"(w1279) -> ()
        n817 = Multiply(x=w1276, y=w1272) -> (x*y=w1274:dbl)
        n818 = local write "T1 offset_x (mV)"(w1274) -> ()
        n819 = local write "T2 offset_x (mV)"(w1273) -> ()
      }
      event "Abort MCL Scan": Value Change {
        n820 = event-data() -> ()  [unwired: 7 out]
        n821 = local write "MCL Scanning"(FALSE ("MCL Scanning")) -> ()
        n822 = xnode "Read/Write Control"("FPGA VI Reference In"=w1305, "error in"=w1304, "Abort scan (MCL)"="Abort MCL Scan") -> ("error out"=w1303:errorcluster)  [unwired: 1 out]
      }
      event "Update Count (MCL)": Value Change {
        n823 = event-data() -> ()  [unwired: 7 out]
        n824 = xnode "Read/Write Control"("FPGA VI Reference In"=w1309, "error in"=w1308, "MCL count"="Update Count (MCL)") -> ("error out"=w1307:errorcluster)  [unwired: 1 out]
      }
      event "Phase adjust (MCL)", "+ phase (MCL)", "- phase (MCL)": Value Change {
        n825 = event-data() -> ()  [unwired: 7 out]
        n826 = Negate(x="Phase adjust (MCL)") -> (-x=w1318:i16)
        n827 = Select(t=w1318, s="- phase (MCL)", f="Phase adjust (MCL)") -> (s? t:f=w1316:i16)
        n828 = Or(x="- phase (MCL)", y="+ phase (MCL)") -> (x .or. y?=w1311:bool)
        n829 = xnode "Read/Write Control"("FPGA VI Reference In"=w1320, "error in"=w1319, "Phase count adjustment (MCL)"=w1316) -> ("FPGA VI Reference Out"=w1312:T19, "error out"=w1313:errorcluster)
        n830 = xnode "Read/Write Control"("FPGA VI Reference In"=w1312, "error in"=w1313, "+ phase (MCL)"=w1311) -> ("error out"=w1310:errorcluster)  [unwired: 1 out]
      }
      event "Abort AOD Scan": Value Change {
        n831 = event-data() -> ()  [unwired: 7 out]
        n832 = xnode "Read/Write Control"("FPGA VI Reference In"=w1324, "error in"=w1323, "Abort scan"="Abort AOD Scan") -> ("error out"=w1322:errorcluster)  [unwired: 1 out]
      }
      event "Continuous AOD Scanning": Value Change {
        n833 = event-data() -> ()  [unwired: 7 out]
        n834 = xnode "Read/Write Control"("FPGA VI Reference In"=w1328, "error in"=w1327, "Cont. Scan"="Continuous AOD Scanning") -> ("error out"=w1326:errorcluster)  [unwired: 1 out]
      }
      event "Index": Value Change {
        n835 = event-data() -> ()  [unwired: 7 out]
        n836 = call "Create new save file.vi"("Insert"="", "Ext"=".dat" ("string"), "Index In"="Index") -> ("Path Out"=→"Save file name":path, "Index Out"=w1329:dbl)
        "Save index" <- w1329
        n837 = local write "Index"(w1329) -> ()
      }
      event "AO1", "AO2": Value Change {
        w1344 = 10.0 ("y")
        w1343 = 32767.0 ("y")
        n838 = event-data() -> ()  [unwired: 7 out]
        n839 = local read "AO2"() -> (w1342:dbl)
        n840 = local read "AO1"() -> (w1339:dbl)
        n841 = Multiply(x=w1339, y=w1343) -> (x*y=w1338:dbl)
        n842 = Multiply(x=w1342, y=w1343) -> (x*y=w1341:dbl)
        n843 = Divide(x=w1338, y=w1344) -> (x/y=w1337:dbl)
        n844 = Divide(x=w1341, y=w1344) -> (x/y=w1340:dbl)
        n845 = To Word Integer(number=w1337) -> (16bit integer=w1345:i16)
        n846 = To Word Integer(number=w1340) -> (16bit integer=w1346:i16)
        n847 = xnode "Read/Write Control"("FPGA VI Reference In"=w1336, "error in"=w1335, "AO1"=w1345, "AO2"=w1346) -> ("error out"=w1334:errorcluster)  [unwired: 1 out]
      }
      event "Inject Bottom": Value Change {
        n848 = event-data() -> ()  [unwired: 7 out]
        n849 = disable-structure shown="Enabled" {
          disable-tunnel: "Inject Bottom" -> [w1348 w1388]
          frame Disabled {
            n850 = local read "Chemyx Syringe Pump Serial Port"() -> (w1349:refnum<visa-resource-name>)
            n851 = local read "Pump write delay (ms)"() -> (w1350:dbl)
            n852 = case shown="True" w1348 {
              tunnel: w1350 -> [w1356 w1370]
              tunnel: w1349 -> [w1353 w1369]
              frame False {
                n853 = flat-sequence {
                  tunnel: w1353 -> [w1357]
                  tunnel: [w1357] -> w1354
                  tunnel: w1356 -> [_]
                  tunnel: [w1360] -> w1355
                  tunnel: w1354 -> [w1360]
                  tunnel: w1355 -> [w1361]
                  tunnel: [w1361] -> w1351
                  tunnel: [w1363] -> w1352
                  tunnel: w1351 -> [w1363]
                  tunnel: w1352 -> [w1365]
                  frame #0 {
                    n854 = call "Write to pump.vi"("string"="enter pump1", "VISA resource name"=w1357) -> ()  [unwired: 1 out]
                  }
                  frame #1 {
                    n855 = Wait (ms)(milliseconds to wait="Pump pause delay (ms)") -> ()  [unwired: 1 out]
                  }
                  frame #2 {
                    n856 = call "Write to pump.vi"("string"="stop", "VISA resource name"=w1361) -> ()  [unwired: 1 out]
                  }
                  frame #3 {
                    n857 = Wait (ms)(milliseconds to wait=u32 500) -> ()  [unwired: 1 out]
                  }
                  frame #4 {
                    n858 = call "Write to pump.vi"("string"="stop", "VISA resource name"=w1365) -> ()  [unwired: 1 out]
                  }
                }
              }
              frame True {
                n859 = flat-sequence {
                  tunnel: w1369 -> [w1379]
                  tunnel: w1370 -> [w1374]
                  tunnel: w1370 -> [w1381]
                  tunnel: w1369 -> [w1382]
                  tunnel: [w1382] -> w1367
                  tunnel: [w1384] -> w1368
                  tunnel: w1367 -> [w1384]
                  tunnel: w1368 -> [w1386]
                  frame #0 {
                    n860 = local read "All Pump Parameters"() -> (w1373:T5)
                    n861 = Unbundle By Name(w1373) -> ("Pump 1"=w1380:T32)
                    n862 = call "Set pump parameters.vi"("Pump write delay (ms)"=w1374, "Volume (uL)"="Ch 2 Inject Volume (uL)", "Rate (uL/h)"="Ch 1 Inject Rate (ul/h)", "Units"=4.0, "Pump #"=1.0, "Pump Parameters In"=w1380, "VISA resource name"=w1379) -> ("Pump Parameters Out"=w1372:T32)  [unwired: 3 in]
                    n863 = Bundle By Name(cluster=w1373, "Pump 1"=w1372) -> (w1371:T5)
                    n864 = local write "All Pump Parameters"(w1371) -> ()
                  }
                  frame #1 {
                    n865 = Wait (ms)(milliseconds to wait=w1381) -> ()  [unwired: 1 out]
                  }
                  frame #2 {
                    n866 = call "Write to pump.vi"("string"="start", "VISA resource name"=w1382) -> ()  [unwired: 1 out]
                  }
                  frame #3 {
                    n867 = Wait (ms)(milliseconds to wait=u32 500) -> ()  [unwired: 1 out]
                  }
                  frame #4 {
                    n868 = call "Write to pump.vi"("string"="start", "VISA resource name"=w1386) -> ()  [unwired: 1 out]
                  }
                }
              }
            }
          }
          frame Enabled {
            n869 = call "hamilton_controller.vi"("Open?"=w1388, "valve"=enum16{"A", "B", "C", "D", "ALL"}."B", "action"=T20."MOVE VALVE") -> ()  [unwired: 8 in, 1 out]
          }
        }
      }
      event "Inject Top": Value Change {
        n870 = event-data() -> ()  [unwired: 7 out]
        n871 = disable-structure shown="Disabled" {
          disable-tunnel: "Inject Top" -> [_ w1432]
          frame Disabled {
            n872 = local read "Pump write delay (ms)"() -> (w1393:dbl)
            n873 = case shown="False" w1394 {
              tunnel: w1393 -> [w1400 w1414]
              tunnel: "Chemyx Syringe Pump Serial Port" -> [w1397 w1413]
              frame False {
                n874 = flat-sequence {
                  tunnel: w1397 -> [w1401]
                  tunnel: [w1401] -> w1398
                  tunnel: w1400 -> [_]
                  tunnel: [w1404] -> w1399
                  tunnel: w1398 -> [w1404]
                  tunnel: w1399 -> [w1405]
                  tunnel: [w1405] -> w1395
                  tunnel: [w1407] -> w1396
                  tunnel: w1395 -> [w1407]
                  tunnel: w1396 -> [w1409]
                  frame #0 {
                    n875 = call "Write to pump.vi"("string"="enter pump3", "VISA resource name"=w1401) -> ()  [unwired: 1 out]
                  }
                  frame #1 {
                    n876 = local read "Pump pause delay (ms)"() -> (w1403:u32)
                    n877 = Wait (ms)(milliseconds to wait=w1403) -> ()  [unwired: 1 out]
                  }
                  frame #2 {
                    n878 = call "Write to pump.vi"("string"="stop", "VISA resource name"=w1405) -> ()  [unwired: 1 out]
                  }
                  frame #3 {
                    n879 = Wait (ms)(milliseconds to wait=u32 0) -> ()  [unwired: 1 out]
                  }
                  frame #4 {
                    n880 = call "Write to pump.vi"("string"="stop", "VISA resource name"=w1409) -> ()  [unwired: 1 out]
                  }
                }
              }
              frame True {
                n881 = flat-sequence {
                  tunnel: w1413 -> [w1423]
                  tunnel: w1414 -> [w1418]
                  tunnel: w1414 -> [w1425]
                  tunnel: w1413 -> [w1426]
                  tunnel: [w1426] -> w1411
                  tunnel: [w1429] -> w1412
                  tunnel: w1411 -> [w1429]
                  tunnel: w1412 -> [w1430]
                  frame #0 {
                    n882 = local read "All Pump Parameters"() -> (w1417:T5)
                    n883 = Unbundle By Name(w1417) -> ("Pump 3"=w1424:T32)
                    n884 = call "Set pump parameters.vi"("Pump write delay (ms)"=w1418, "Volume (uL)"="Ch 3 Inject Volume (uL)", "Rate (uL/h)"="Ch 3 Inject Rate (ul/h)", "Units"=4.0, "Pump #"=3.0, "Pump Parameters In"=w1424, "VISA resource name"=w1423) -> ("Pump Parameters Out"=w1416:T32)  [unwired: 3 in]
                    n885 = Bundle By Name(cluster=w1417, "Pump 3"=w1416) -> (w1415:T5)
                    n886 = local write "All Pump Parameters"(w1415) -> ()
                  }
                  frame #1 {
                    n887 = Wait (ms)(milliseconds to wait=w1425) -> ()  [unwired: 1 out]
                  }
                  frame #2 {
                    n888 = call "Write to pump.vi"("string"="start", "VISA resource name"=w1426) -> ()  [unwired: 1 out]
                  }
                  frame #3 {
                    n889 = Wait (ms)(milliseconds to wait=u32 500) -> ()  [unwired: 1 out]
                  }
                  frame #4 {
                    n890 = call "Write to pump.vi"("string"="start", "VISA resource name"=w1430) -> ()  [unwired: 1 out]
                  }
                }
              }
            }
          }
          frame Enabled {
            n891 = call "hamilton_controller.vi"("Open?"=w1432, "valve"=enum16{"A", "B", "C", "D", "ALL"}."A", "action"=T20."MOVE VALVE") -> ()  [unwired: 8 in, 1 out]
          }
        }
      }
      event "Inject Valve B": Value Change {
        n892 = event-data() -> ()  [unwired: 7 out]
        n893 = disable-structure shown="Enabled" {
          disable-tunnel: "Inject Valve B" -> [w1436 w1456]
          frame Disabled {
            n894 = local read "Pump write delay (ms)"() -> (w1438:dbl)
            n895 = flat-sequence {
              tunnel: w1437 -> [w1451]
              tunnel: w1438 -> [w1447]
              tunnel: w1436 -> [_]
              tunnel: w1438 -> [w1453]
              tunnel: w1437 -> [w1454]
              frame #0 {
                n896 = local read "All Pump Parameters"() -> (w1446:T5)
                n897 = Multiply(x=60.0, y="Flush Center Ch Rate (ul/m)") -> (x*y=w1443:dbl)
                n898 = Unbundle By Name(w1446) -> ("Pump 2"=w1452:T32)
                n899 = call "Set pump parameters.vi"("Pump write delay (ms)"=w1447, "Volume (uL)"="Flush Center Ch Volume (uL)", "Rate (uL/h)"=w1443, "Units"=3.0, "Pump #"=2.0, "Pump Parameters In"=w1452, "VISA resource name"=w1451) -> ("Pump Parameters Out"=w1445:T32)  [unwired: 3 in]
                n900 = Bundle By Name(cluster=w1446, "Pump 2"=w1445) -> (w1444:T5)
                n901 = local write "All Pump Parameters"(w1444) -> ()
                n902 = Add(x="Flush Center Ch Volume (uL)", y="Total Volume\nFlushed (uL)") -> (x+y=w1440:dbl)
                n903 = local write "Total Volume\nFlushed (uL)"(w1440) -> ()
              }
              frame #1 {
                n904 = Wait (ms)(milliseconds to wait=w1453) -> ()  [unwired: 1 out]
              }
              frame #2 {
                n905 = call "Write to pump.vi"("string"="start", "VISA resource name"=w1454) -> ()  [unwired: 1 out]
              }
            }
            n906 = local read "Chemyx Syringe Pump Serial Port"() -> (w1437:refnum<visa-resource-name>)
          }
          frame Enabled {
            n907 = call "hamilton_controller.vi"("Open?"=w1456, "valve"=enum16{"A", "B", "C", "D", "ALL"}."B", "action"=T20."MOVE VALVE") -> ()  [unwired: 8 in, 1 out]
          }
        }
      }
      event "Sample Channel Flow": Value Change {
        n908 = event-data() -> ()  [unwired: 7 out]
        n909 = call "hamilton_controller.vi"("Open?"="Sample Channel Flow", "valve"=enum16{"A", "B", "C", "D", "ALL"}."C", "action"=T20."MOVE VALVE") -> ()  [unwired: 8 in, 1 out]
      }
      event "Flip Green Filter": Value Change {
        n910 = event-data() -> ()  [unwired: 7 out]
        n911 = Not(x="Flip Green Filter") -> (.not. x?=w1462:bool)
        n912 = local write "Flip Green Filter"(w1462) -> ()
        n913 = flat-sequence {
          tunnel: w1470 -> [w1475]
          tunnel: w1469 -> [w1474]
          tunnel: [w1472] -> w1467
          tunnel: [w1471] -> w1466
          tunnel: [w1477] -> w1465
          tunnel: w1467 -> [w1477]
          tunnel: [w1476] -> w1464
          tunnel: w1466 -> [w1476]
          tunnel: w1465 -> [w1481]
          tunnel: w1464 -> [w1480]
          tunnel: [w1479] -> w1468
          frame #0 {
            n914 = xnode "Read/Write Control"("FPGA VI Reference In"=w1475, "error in"=w1474, "Green Filter Flipper"=TRUE) -> ("FPGA VI Reference Out"=w1472:T19, "error out"=w1471:errorcluster)
          }
          frame #1 {
            n915 = Wait (ms)(milliseconds to wait=u32 100) -> ()  [unwired: 1 out]
          }
          frame #2 {
            n916 = xnode "Read/Write Control"("FPGA VI Reference In"=w1481, "error in"=w1480, "Green Filter Flipper"=FALSE) -> ("error out"=w1479:errorcluster)  [unwired: 1 out]
          }
        }
      }
      event "Pump 1 contents", "Pump 3 contents": Value Change {
        n917 = event-data() -> ()  [unwired: 7 out]
        n918 = local read "Pump 1 contents"() -> (→"Pump 1 cont disp":string)
        n919 = local read "Pump 3 contents"() -> (→"Pump 3 cont disp":string)
      }
      event "Reset Trap Pos. FB": Value Change {
        n920 = event-data() -> ()  [unwired: 7 out]
        n921 = xnode "Read/Write Control"("FPGA VI Reference In"=w1487, "error in"=w1486, "Trap Pos. FB Reset"="Reset Trap Pos. FB") -> ()  [unwired: 2 out]
      }
      event "Trap Pos. FB ON": Value Change {
        n922 = event-data() -> ()  [unwired: 7 out]
        n923 = xnode "Read/Write Control"("FPGA VI Reference In"=w1490, "error in"=w1489, "Force feedback"="Trap Pos. FB ON") -> ()  [unwired: 2 out]
      }
      event "Trap Pos. FB Range", "Trap Pos. FB Gains", "Trap Pos. FB Mult Factor", "Trap Pos. FB Offset Factor", "Trap Pos FB Negate Action", "Trap Pos FB Monitor\nT1 or T2": Value Change {
        n924 = event-data() -> ()  [unwired: 7 out]
        n925 = xnode "Read/Write Control"("FPGA VI Reference In"=w1499, "error in"=w1498, "Trap Pos. FB Range"="Trap Pos. FB Range", "Trap Pos. FB Gains"="Trap Pos. FB Gains", "Trap Pos. FB Mult Factor"="Trap Pos. FB Mult Factor", "Trap Pos. FB Offset Factor"="Trap Pos. FB Offset Factor", "Trap Pos FB Negate Action"="Trap Pos FB Negate Action", "Trap Pos FB Monitor T1 or T2"="Trap Pos FB Monitor\nT1 or T2", "AI1 X Scale"="Trap Pos. AI1 X Pre-scale") -> ()  [unwired: 2 out]
      }
      event "Trap Pos FB SP": Value Change {
        n926 = event-data() -> ()  [unwired: 7 out]
        n927 = xnode "Read/Write Control"("FPGA VI Reference In"=w1502, "error in"=w1501, "Trap Pos. FB SP"="Trap Pos FB SP") -> ()  [unwired: 2 out]
      }
      event "Set SP to Reading": Value Change {
        n928 = event-data() -> ()  [unwired: 7 out]
        n929 = local read "Trap Pos FB Monitor\nT1 or T2"() -> (w1510:bool)
        n930 = local read "Trap X AI1 (DMA)"() -> (w1513:T13)
        n931 = local read "Trap X (AI1)"() -> (w1516:T10)
        n932 = Unbundle By Name(w1516) -> ("Trap 1"=w1515:fxp<+/-,16,1>, "Trap 2"=w1514:fxp<+/-,16,1>)
        n933 = Unbundle By Name(w1513) -> ("Set 1"=w1512:fxp<+/-,16,1>, "Set 2"=w1511:fxp<+/-,16,1>)
        n934 = Select(t=w1515, s=w1510, f=w1514) -> (s? t:f=w1509:fxp<+/-,16,1>)
        n935 = Select(t=w1512, s=w1510, f=w1511) -> (s? t:f=w1508:fxp<+/-,16,1>)
        n936 = Not(x="Set SP Using...") -> (.not. x?=w1503:bool)
        n937 = Select(t=w1509, s=w1503, f=w1508) -> (s? t:f=w1504:fxp<+/-,16,1>)
        n938 = xnode "Read/Write Control"("FPGA VI Reference In"=w1506, "error in"=w1505, "Trap Pos. FB SP"=w1504) -> ()  [unwired: 2 out]
        n939 = local write "Trap Pos FB SP"(w1504) -> ()
      }
      event "Trap Pos. FB Out Scale 2^n": Value Change {
        n940 = event-data() -> ()  [unwired: 7 out]
        n941 = Scale By Power Of 2(n="Trap Pos. FB Out Scale 2^n", x=ext 1.0) -> (x*2^n=w1518:ext)
        n942 = property on="Trap Pos. FB Mult Factor" class="DigNum (strict)"("Val(Sgnl)"=w1518) -> ()  [unwired: 2 in, 2 out]
      }
      event "Trap Pos FB Int Count": Value Change {
        n943 = event-data() -> ()  [unwired: 7 out]
        n944 = xnode "Read/Write Control"("FPGA VI Reference In"=w1523, "error in"=w1522, "Trap Pos FB Int Count"="Trap Pos FB Int Count") -> ()  [unwired: 2 out]
      }
    }
    "error out 2" <- w706
    n945 = node-c288() -> ()  [unwired: 1 in, 1 out]
  }
  n946 = timed-loop "Run Scripts, including: stage motion" {
    timing: w69 -> [_]
    timing-out: [_] -> w68
    tunnel: w24 -> [_]
    stop <- w1525 stop-if-true
    n947 = node-c288() -> ()  [unwired: 1 in, 1 out]
    n948 = event shown="[3] \"Dump Beads\": Value Change" {
      selector: _ -> [_ _ _ _ _ _ _ _ _ _ _ _]
      dyn-events: _ -> [_ _ _ _ _ _ _ _ _ _ _ _]
      timeout: 50 -> [_ _ _ _ _ _ _ _ _ _ _ _]
      tunnel: ["Move Cap. 1 (DNA Top)" _ "Cal/Data Acq. Spot" "Dump Beads" "Dip for Protein" _ "Got ADig bead" "Got DNA bead" "Take Stepping Data" _ "Take Detection Laser\nImage" _] -> _
      tunnel: [_ _ _ _ _ _ _ _ _ _ _ w1733] -> w1525
      event "Move Cap. 1 (DNA Top)": Value Change {
        n949 = event-data() -> ()  [unwired: 1 in, 5 out]
        n950 = local write "Move Cap. 1 (DNA Top)"(FALSE ("Move Cap. 1 (DNA Right)")) -> ()
        n951 = flat-sequence {
          tunnel: "Cap 1 Samp Flow ON" -> [w1531]
          frame #0 {
            n952 = local write "Stage Moving"(FALSE ("Stage Moving")) -> ()
            n953 = case "stop flow" shown="True" w1531 {
              frame False {
              }
              frame True {
                n954 = call "hamilton_controller.vi"("Open?"=FALSE, "valve"=enum16{"A", "B", "C", "D", "ALL"}."C", "action"=T20."MOVE VALVE") -> ()  [unwired: 8 in, 1 out]
              }
            }
            n955 = case shown="True" TRUE {
              tunnel: "Cap 1 T ON" -> [w1540 w1541]
              frame False {
                n956 = property on="Trap 1 (ON/OFF)" class="Bool (strict)"("Val(Sgnl)"=w1540) -> ()  [unwired: 2 in, 2 out]
              }
              frame True {
                n957 = property on="Trap 2 (ON/OFF)" class="Bool (strict)"("Val(Sgnl)"=w1541) -> ()  [unwired: 2 in, 2 out]
              }
            }
            n958 = call <vilib>:"Beep.vi"() -> ()  [unwired: 3 in, 9 out]
            n959 = case shown="True" "Cap 1 Flow ON" {
              frame False {
              }
              frame True {
                n960 = property on="Inject Top" class="Bool (strict)"("Val(Sgnl)"=TRUE ("Value (Signaling)")) -> ()  [unwired: 2 in, 2 out]
              }
            }
          }
        }
      }
      event Timeout {
        n961 = event-data() -> ()  [unwired: 1 in, 2 out]
      }
      event "Cal/Data Acq. Spot": Value Change {
        # "wait for calibration file\nto be written"
        # "signal save cal true\nthis tells the data \nacquisition loop to\nstart sending the data\nto a calibration file"
        # "separate traps to\nthe desired trap delta"
        # "move stage to data acquisition spot"
        # "CHANGE FISH FOR TETHER BACK\nTO TRUE VALUE HERE."
        n962 = event-data() -> ()  [unwired: 1 in, 5 out]
        n963 = local write "Cal/Data Acq. Spot"(FALSE ("Cal/Data Acq. Spot")) -> ()
        n964 = flat-sequence {
          tunnel: ["Cal @ (MHz)"] -> w1542
          tunnel: w1542 -> [w1552]
          tunnel: w1542 -> [w1573]
          frame #0 {
            n965 = property on="Trap Delta (MHz)" class="DigNum (strict)"("Val(Sgnl)"="Cal @ (MHz)") -> ()  [unwired: 2 in, 2 out]
            n966 = call <vilib>:"Beep.vi"() -> ()  [unwired: 3 in, 9 out]
          }
          frame #1 {
            n967 = Wait (ms)(milliseconds to wait=u32 100) -> ()  [unwired: 1 out]
          }
          frame #2 {
            n968 = property on="Save Calibration" class="Bool (strict)"("Val(Sgnl)"=TRUE ("Value (Signaling)")) -> ()  [unwired: 2 in, 2 out]
          }
          frame #3 {
            n969 = Wait (ms)(milliseconds to wait=u32 4000) -> ()  [unwired: 1 out]
          }
          frame #4 {
            n970 = while {
              stop <- w1549 stop-if-true
              n971 = local read "Saving..."() -> (w1550:bool)
              n972 = Wait (ms)(milliseconds to wait=u32 100) -> ()  [unwired: 1 out]
              n973 = Not(x=w1550) -> (.not. x?=w1549:bool)
            }
          }
          frame #5 {
            n974 = case shown="True" "W/ Offset 1" {
              tunnel: w1552 -> [_ w1554]
              frame False {
              }
              frame True {
                n975 = stacked-sequence {
                  tunnel: w1554 -> [_ _ _ _ _ _ _ w1571]
                  frame #0 {
                    n976 = Replace Array Subset(array=u32[] [0] ("Index Values"), new element="Offset 1 Set", index=0) -> (w1555:u32[])
                    n977 = property on="Saved AOD Raster Scan Parameter Sets" class="Arr (strict)"("Index Values"=w1555) -> ()  [unwired: 2 in, 2 out]
                    n978 = property on="Trap Delta (MHz)" class="DigNum (strict)"("Val(Sgnl)"="Offset 1 Start (MHz)") -> ()  [unwired: 2 in, 2 out]
                  }
                  frame #1 {
                    n979 = Wait (ms)(milliseconds to wait=u32 200) -> ()  [unwired: 1 out]
                  }
                  frame #2 {
                    n980 = property on="Load parameters" class="Bool (strict)"("Val(Sgnl)"=TRUE ("Value (Signaling)")) -> ()  [unwired: 2 in, 2 out]
                  }
                  frame #3 {
                    n981 = Wait (ms)(milliseconds to wait=u32 200) -> ()  [unwired: 1 out]
                  }
                  frame #4 {
                    n982 = property on="Trap Raster Scan" class="Bool (strict)"("Val(Sgnl)"=TRUE ("Value (Signaling)")) -> ()  [unwired: 2 in, 2 out]
                  }
                  frame #5 {
                    n983 = Wait (ms)(milliseconds to wait=u32 2000) -> ()  [unwired: 1 out]
                  }
                  frame #6 {
                    n984 = while {
                      stop <- w1568 stop-if-true
                      n985 = local read "Raster Scanning..."() -> (w1570:bool)
                      n986 = local read "Saving..."() -> (w1566:bool)
                      n987 = Wait (ms)(milliseconds to wait=u32 100) -> ()  [unwired: 1 out]
                      n988 = Not(x=w1566) -> (.not. x?=w1565:bool)
                      n989 = Not(x=w1570) -> (.not. x?=w1567:bool)
                      n990 = And(x=w1567, y=w1565) -> (x .and. y?=w1568:bool)
                    }
                  }
                  frame #7 {
                    n991 = property on="Trap Delta (MHz)" class="DigNum (strict)"("Val(Sgnl)"=w1571) -> ()  [unwired: 2 in, 2 out]
                  }
                }
              }
            }
          }
          frame #6 {
            n992 = local read "Save ave N"() -> (w1572:dbl)
            n993 = case shown="True" "W/ Offset 2" {
              tunnel: w1573 -> [_ w1579]
              tunnel: w1572 -> [_ w1578]
              frame False {
                n994 = Multiply(x="Cal read wait (s)", y=u32 1000 ("milliseconds to wait")) -> (x*y=w1576:u32)
                n995 = Wait (ms)(milliseconds to wait=w1576) -> ()  [unwired: 1 out]
              }
              frame True {
                n996 = stacked-sequence {
                  tunnel: w1579 -> [_ _ _ _ _ _ _ _ _ w1600 _ _]
                  tunnel: w1578 -> [_ _ _ _ _ _ _ _ _ w1598 _ _]
                  frame #0 {
                    n997 = property on="Save ave N" class="DigNum (strict)"("Val(Sgnl)"=1.0 ("Value (Signaling)")) -> ()  [unwired: 2 in, 2 out]
                  }
                  frame #1 {
                    n998 = Wait (ms)(milliseconds to wait=u32 500) -> ()  [unwired: 1 out]
                  }
                  frame #2 {
                    n999 = property on="Trap Delta (MHz)" class="DigNum (strict)"("Val(Sgnl)"="Offset 2 Start (MHz)") -> ()  [unwired: 2 in, 2 out]
                    n1000 = Replace Array Subset(array=u32[] [0] ("Index Values"), new element="Offset 2 Set", index=0) -> (w1584:u32[])
                    n1001 = property on="Saved AOD Raster Scan Parameter Sets" class="Arr (strict)"("Index Values"=w1584) -> ()  [unwired: 2 in, 2 out]
                  }
                  frame #3 {
                    n1002 = Wait (ms)(milliseconds to wait=u32 500) -> ()  [unwired: 1 out]
                  }
                  frame #4 {
                    n1003 = property on="Load parameters" class="Bool (strict)"("Val(Sgnl)"=TRUE ("Value (Signaling)")) -> ()  [unwired: 2 in, 2 out]
                  }
                  frame #5 {
                    n1004 = Wait (ms)(milliseconds to wait=u32 500) -> ()  [unwired: 1 out]
                  }
                  frame #6 {
                    n1005 = property on="Trap Raster Scan" class="Bool (strict)"("Val(Sgnl)"=TRUE ("Value (Signaling)")) -> ()  [unwired: 2 in, 2 out]
                  }
                  frame #7 {
                    n1006 = Wait (ms)(milliseconds to wait=u32 2000) -> ()  [unwired: 1 out]
                  }
                  frame #8 {
                    n1007 = while {
                      stop <- w1593 stop-if-true
                      n1008 = local read "Raster Scanning..."() -> (w1596:bool)
                      n1009 = local read "Saving..."() -> (w1594:bool)
                      n1010 = Wait (ms)(milliseconds to wait=u32 100) -> ()  [unwired: 1 out]
                      n1011 = Not(x=w1594) -> (.not. x?=w1592:bool)
                      n1012 = Not(x=w1596) -> (.not. x?=w1595:bool)
                      n1013 = And(x=w1595, y=w1592) -> (x .and. y?=w1593:bool)
                    }
                  }
                  frame #9 {
                    n1014 = property on="Trap Delta (MHz)" class="DigNum (strict)"("Val(Sgnl)"=w1600) -> ()  [unwired: 2 in, 2 out]
                    n1015 = property on="Saved AOD Raster Scan Parameter Sets" class="Arr (strict)"("Index Values"=u32[] [0]) -> ()  [unwired: 2 in, 2 out]
                    n1016 = property on="Save ave N" class="DigNum (strict)"("Val(Sgnl)"=w1598) -> ()  [unwired: 2 in, 2 out]
                  }
                  frame #10 {
                    n1017 = Wait (ms)(milliseconds to wait=u32 500) -> ()  [unwired: 1 out]
                  }
                  frame #11 {
                    n1018 = property on="Load parameters" class="Bool (strict)"("Val(Sgnl)"=TRUE ("Value (Signaling)")) -> ()  [unwired: 2 in, 2 out]
                  }
                }
              }
            }
          }
          frame #7 {
            n1019 = property on="Read Cal" class="Bool (strict)"("Val(Sgnl)"=TRUE ("Value (Signaling)")) -> ()  [unwired: 2 in, 2 out]
          }
          frame #8 {
            n1020 = Wait (ms)(milliseconds to wait=u32 500) -> ()  [unwired: 1 out]
          }
          frame #9 {
            n1021 = property on="Fish for Tether" class="Bool (strict)"("Val(Sgnl)"=FALSE ("Value (Signaling)")) -> ()  [unwired: 2 in, 2 out]
          }
        }
      }
      event "Dump Beads": Value Change {
        # "SCRIPT TO REMOVE BOTH BEADS FROM THE TRAPS. TURNS ON LIGHT WHICH INDICATES THAT STAGE IS MOVING. THEN STOPS SAVING DATA. \nSETS Sample Channel Flow TO TRUE. STOPS INTERLACING GREEN FLUORESCENCE. TURNS OFF Tether INDICATOR BECAUSE WE ARE THROWING IT\nAWAY. SHUTS OFF TRAP POSITION FEEDBACK."
        n1022 = event-data() -> ()  [unwired: 1 in, 5 out]
        n1023 = flat-sequence {
          frame #0 {
            w1608 = FALSE ("Fl. Triggered...")
            w1607 = TRUE ("Stage Moving")
            n1024 = local read "Saving..."() -> (w1609:bool)
            n1025 = local write "Fl. Triggered..."(w1608) -> ()
            n1026 = local write "Stage Moving"(w1607) -> ()
            n1027 = local write "Tether"(w1608) -> ()
            n1028 = property on="Green Laser ON/Interlacing" class="Bool (strict)"("Val(Sgnl)"=w1607) -> ()  [unwired: 2 in, 2 out]
            n1029 = property on="Trap Pos. FB ON" class="Bool (strict)"("Val(Sgnl)"=w1608) -> ()  [unwired: 2 in, 2 out]
            n1030 = property on="Sample Channel Flow" class="Bool (strict)"("Val(Sgnl)"=w1607) -> ()  [unwired: 2 in, 2 out]
            n1031 = local write "Stop Saving"(w1609) -> ()
          }
          frame #1 {
            w1610 = FALSE ("Value (Signaling)")
            # "TURNS TRAPS OFF SO THAT\nBEADS REMAIN AT DUMP \nBEADS POSITION"
            n1032 = property on="Trap 1 (ON/OFF)" class="Bool (strict)"("Val(Sgnl)"=w1610) -> ()  [unwired: 2 in, 2 out]
            n1033 = property on="Trap 2 (ON/OFF)" class="Bool (strict)"("Val(Sgnl)"=w1610) -> ()  [unwired: 2 in, 2 out]
            n1034 = call <vilib>:"Beep.vi"() -> ()  [unwired: 3 in, 9 out]
          }
          frame #2 {
            n1035 = property on="Goto Bottom (F7)" class="Bool (strict)"("Val(Sgnl)"=TRUE ("Value (Signaling)")) -> ()  [unwired: 2 in, 2 out]
          }
          frame #3 {
            n1036 = Wait (ms)(milliseconds to wait=u32 8000) -> ()  [unwired: 1 out]
          }
          frame #4 {
            n1037 = property on="Trap Delta (MHz)" class="DigNum (strict)"("Val(Sgnl)"=20.0 ("Value (Signaling)")) -> ()  [unwired: 2 in, 2 out]
          }
          frame #5 {
            n1038 = property on="Trap 2 (ON/OFF)" class="Bool (strict)"("Val(Sgnl)"=TRUE ("Value (Signaling)")) -> ()  [unwired: 2 in, 2 out]
          }
          frame #6 {
            n1039 = property on="Sample Channel Flow" class="Bool (strict)"("Val(Sgnl)"=FALSE ("Value (Signaling)")) -> ()  [unwired: 2 in, 2 out]
          }
        }
      }
      event "Dip for Protein": Value Change {
        n1040 = event-data() -> ()  [unwired: 1 in, 5 out]
        n1041 = flat-sequence {
          frame #0 {
            n1042 = case shown="True" "Move Trap Before?" {
              frame False {
              }
              frame True {
                n1043 = property on="Trap Delta (MHz)" class="DigNum (strict)"("Val(Sgnl)"="Dip Trap Delta 1 (MHz)") -> ()  [unwired: 2 in, 2 out]
              }
            }
          }
          frame #1 {
            n1044 = Multiply(x="Duration (s)", y=1000.0) -> (x*y=w1619:dbl)
            n1045 = Wait (ms)(milliseconds to wait=w1619) -> ()  [unwired: 1 out]
          }
          frame #2 {
            n1046 = case shown="True" "Move Trap After?" {
              frame False {
              }
              frame True {
                n1047 = property on="Trap Delta (MHz)" class="DigNum (strict)"("Val(Sgnl)"="Dip Trap Delta 2 (MHz)") -> ()  [unwired: 2 in, 2 out]
              }
            }
          }
          frame #3 {
            n1048 = case shown="True" "Green ON After?" {
              frame False {
              }
              frame True {
                n1049 = property on="Green Laser ON/Interlacing" class="Bool (strict)"("Val(Sgnl)"=TRUE ("Value (Signaling)")) -> ()  [unwired: 2 in, 2 out]
              }
            }
          }
          frame #4 {
            n1050 = Wait (ms)(milliseconds to wait=u32 500) -> ()  [unwired: 1 out]
          }
          frame #5 {
            n1051 = case shown="True" "Save Data After?" {
              frame False {
              }
              frame True {
                n1052 = property on="Start Saving" class="Bool (strict)"("Val(Sgnl)"=TRUE ("Value (Signaling)")) -> ()  [unwired: 2 in, 2 out]
              }
            }
          }
        }
      }
      event "Profile": Value Change {
        n1053 = event-data() -> ()  [unwired: 1 in, 5 out]
        n1054 = flat-sequence {
          frame #0 {
            w1629 = 0.0 ("element")
            n1055 = Build Array(w1629, "Y change (mm)", w1629) -> ()  [unwired: 1 out]
          }
          frame #1 {
            # "stop saving"
            n1056 = local write "Stop Saving"(TRUE ("Stop Saving")) -> ()
            n1057 = local write "Stage Moving"(FALSE ("Stage Moving")) -> ()
          }
        }
      }
      event "Got ADig bead": Value Change {
        n1058 = event-data() -> ()  [unwired: 1 in, 5 out]
        n1059 = property on="Move Cap. 1 (DNA Top)" class="Bool (strict)"("Val(Sgnl)"=TRUE ("Value (Signaling)")) -> ()  [unwired: 2 in, 2 out]
        n1060 = property on="Inject Bottom" class="Bool (strict)"("Val(Sgnl)"=FALSE ("Value (Signaling)")) -> ()  [unwired: 2 in, 2 out]
      }
      event "Got DNA bead": Value Change {
        n1061 = event-data() -> ()  [unwired: 1 in, 5 out]
        n1062 = property on="Cal/Data Acq. Spot" class="Bool (strict)"("Val(Sgnl)"=TRUE ("Value (Signaling)")) -> ()  [unwired: 2 in, 2 out]
        n1063 = property on="Inject Top" class="Bool (strict)"("Val(Sgnl)"=FALSE ("Value (Signaling)")) -> ()  [unwired: 2 in, 2 out]
      }
      event "Take Stepping Data": Value Change {
        n1064 = event-data() -> ()  [unwired: 1 in, 5 out]
        n1065 = local read "Save ave N"() -> (w1647:dbl)
        n1066 = flat-sequence {
          tunnel: w1647 -> [w1649]
          tunnel: [w1649] -> w1642
          tunnel: [w1651] -> w1643
          tunnel: w1642 -> [w1651]
          tunnel: [w1653] -> w1644
          tunnel: w1643 -> [w1653]
          tunnel: [w1656] -> w1645
          tunnel: w1644 -> [w1656]
          tunnel: [w1658] -> w1646
          tunnel: w1645 -> [w1658]
          tunnel: [w1660] -> w1640
          tunnel: w1646 -> [w1660]
          tunnel: w1640 -> [w1663]
          tunnel: [w1663] -> w1639
          tunnel: w1639 -> [w1664]
          tunnel: [w1664] -> w1641
          tunnel: w1641 -> [w1670]
          frame #0 {
            n1067 = property on="Save ave N" class="DigNum (strict)"("Val(Sgnl)"="Save ave factor") -> ()  [unwired: 2 in, 2 out]
          }
          frame #1 {
            n1068 = Wait (ms)(milliseconds to wait=u32 100) -> ()  [unwired: 1 out]
          }
          frame #2 {
            n1069 = local read "Offset 2 Start (MHz)"() -> (w1655:dbl)
            n1070 = property on="Saved AOD Raster Scan Parameter Sets" class="Arr (strict)"("Index Values"=u32[] [2]) -> ()  [unwired: 2 in, 2 out]
            n1071 = property on="Trap Delta (MHz)" class="DigNum (strict)"("Val(Sgnl)"=w1655) -> ()  [unwired: 2 in, 2 out]
          }
          frame #3 {
            n1072 = property on="Load parameters" class="Bool (strict)"("Val(Sgnl)"=TRUE ("Value (Signaling)")) -> ()  [unwired: 2 in, 2 out]
          }
          frame #4 {
            n1073 = Wait (ms)(milliseconds to wait=u32 100) -> ()  [unwired: 1 out]
          }
          frame #5 {
            n1074 = property on="Trap Raster Scan" class="Bool (strict)"("Val(Sgnl)"=TRUE ("Value (Signaling)")) -> ()  [unwired: 2 in, 2 out]
          }
          frame #6 {
            n1075 = Wait (ms)(milliseconds to wait=u32 1000) -> ()  [unwired: 1 out]
          }
          frame #7 {
            n1076 = while {
              stop <- w1667 stop-if-true
              n1077 = local read "Raster Scanning..."() -> (w1669:bool)
              n1078 = local read "Saving..."() -> (w1668:bool)
              n1079 = Not(x=w1668) -> (.not. x?=w1665:bool)
              n1080 = Not(x=w1669) -> (.not. x?=w1666:bool)
              n1081 = And(x=w1666, y=w1665) -> (x .and. y?=w1667:bool)
            }
          }
          frame #8 {
            n1082 = property on="Save ave N" class="DigNum (strict)"("Val(Sgnl)"=w1670) -> ()  [unwired: 2 in, 2 out]
          }
        }
      }
      event "Step Size (nm)": Value Change {
        n1083 = event-data() -> ()  [unwired: 1 in, 5 out]
        n1084 = flat-sequence {
          frame #0 {
            n1085 = property on="Saved AOD Raster Scan Parameter Sets" class="Arr (strict)"("Index Values"=u32[] [1]) -> ()  [unwired: 2 in, 2 out]
          }
          frame #1 {
            n1086 = Multiply(x="N Steps", y="Step Size (nm)") -> (x*y=w1672:dbl)
            n1087 = property on="Scan Speed AOD (nm/s) 2" class="DigNum (strict)"("Value"="Step Size (nm)") -> ()  [unwired: 2 in, 2 out]
            n1088 = property on="Step Size AOD (nm) 2" class="DigNum (strict)"("Value"="Step Size (nm)") -> ()  [unwired: 2 in, 2 out]
            n1089 = property on="Scan Range AOD (nm) 2" class="DigNum (strict)"("Value"=w1672) -> ()  [unwired: 2 in, 2 out]
          }
        }
      }
      event "Take Detection Laser\nImage": Value Change {
        n1090 = event-data() -> ()  [unwired: 1 in, 5 out]
        n1091 = flat-sequence {
          tunnel: [w1700] -> w1690
          tunnel: [w1699] -> w1683
          tunnel: [w1698] -> w1675
          tunnel: [w1703] -> w1691
          tunnel: w1690 -> [w1703]
          tunnel: [w1702] -> w1684
          tunnel: w1683 -> [w1702]
          tunnel: [w1701] -> w1676
          tunnel: w1675 -> [w1701]
          tunnel: [w1707] -> w1692
          tunnel: w1691 -> [w1707]
          tunnel: [w1706] -> w1685
          tunnel: w1684 -> [w1706]
          tunnel: [w1705] -> w1677
          tunnel: w1676 -> [w1705]
          tunnel: [w1713] -> w1693
          tunnel: w1692 -> [w1713]
          tunnel: [w1712] -> w1686
          tunnel: w1685 -> [w1712]
          tunnel: [w1711] -> w1678
          tunnel: w1677 -> [w1711]
          tunnel: [w1717] -> w1694
          tunnel: w1693 -> [w1717]
          tunnel: [w1716] -> w1687
          tunnel: w1686 -> [w1716]
          tunnel: [w1715] -> w1679
          tunnel: w1678 -> [w1715]
          tunnel: [w1721] -> w1695
          tunnel: w1694 -> [w1721]
          tunnel: [w1720] -> w1688
          tunnel: w1687 -> [w1720]
          tunnel: [w1719] -> w1680
          tunnel: w1679 -> [w1719]
          tunnel: [w1725] -> w1696
          tunnel: w1695 -> [w1725]
          tunnel: [w1724] -> w1689
          tunnel: w1688 -> [w1724]
          tunnel: [w1723] -> w1681
          tunnel: w1680 -> [w1723]
          tunnel: w1696 -> [w1731]
          tunnel: w1689 -> [w1730]
          tunnel: [w1728] -> w1682
          tunnel: w1681 -> [w1728]
          tunnel: w1682 -> [w1732]
          frame #0 {
            n1092 = local read "Green Laser ON/Interlacing"() -> (w1700:bool)
            n1093 = local read "Green laser mode"() -> (w1699:enum32{"Laser ON", "Laser OFF", "Interlace"})
            n1094 = local read "Green FB On/Off"() -> (w1698:bool)
          }
          frame #1 {
            n1095 = property on="Green FB On/Off" class="Bool (strict)"("Val(Sgnl)"=FALSE ("Value (Signaling)")) -> ()  [unwired: 2 in, 2 out]
          }
          frame #2 {
            n1096 = property on="Green Laser ON/Interlacing" class="Bool (strict)"("Val(Sgnl)"=TRUE ("Value (Signaling)")) -> ()  [unwired: 2 in, 2 out]
            n1097 = property on="Flip Green Filter" class="Bool (strict)"("Val(Sgnl)"=TRUE ("Value (Signaling)")) -> ()  [unwired: 2 in, 2 out]
            n1098 = property on="Green laser mode" class="RadioBtnsControl (strict)"("Val(Sgnl)"=enum32{"Laser ON", "Laser OFF", "Interlace"}."Laser ON" ("Value (Signaling)")) -> ()  [unwired: 2 in, 2 out]
          }
          frame #3 {
            n1099 = Wait (ms)(milliseconds to wait=u32 500) -> ()  [unwired: 1 out]
          }
          frame #4 {
            n1100 = property on="Confocal Image" class="Bool (strict)"("Val(Sgnl)"=TRUE ("Value (Signaling)")) -> ()  [unwired: 2 in, 2 out]
          }
          frame #5 {
            n1101 = Wait (ms)(milliseconds to wait=u32 2000) -> ()  [unwired: 1 out]
          }
          frame #6 {
            n1102 = while {
              stop <- w1726 stop-if-true
              n1103 = local read "Saving..."() -> (w1727:bool)
              n1104 = Not(x=w1727) -> (.not. x?=w1726:bool)
            }
          }
          frame #7 {
            n1105 = property on="Flip Green Filter" class="Bool (strict)"("Val(Sgnl)"=TRUE ("Value (Signaling)")) -> ()  [unwired: 2 in, 2 out]
            n1106 = property on="Green Laser ON/Interlacing" class="Bool (strict)"("Val(Sgnl)"=w1731) -> ()  [unwired: 2 in, 2 out]
            n1107 = property on="Green laser mode" class="RadioBtnsControl (strict)"("Val(Sgnl)"=w1730) -> ()  [unwired: 2 in, 2 out]
          }
          frame #8 {
            n1108 = property on="Green FB On/Off" class="Bool (strict)"("Val(Sgnl)"=w1732) -> ()  [unwired: 2 in, 2 out]
          }
        }
      }
      event "Stop All": Value Change {
        n1109 = event-data() -> ()  [unwired: 1 in, 5 out]
        n1110 = local read "Stop All"() -> (w1733:bool)
      }
    }
    n1111 = node-c288() -> ()  [unwired: 1 in, 1 out]
  }
  n1112 = node-c288() -> (w76:T24)  [unwired: 4 out]
  n1113 = timed-loop "Mouse control: trap position (AOM deflection), set confocal spot from image" {
    tunnel: [w1735] -> w34
    tunnel: w24 -> [w1734]
    timing: w76 -> [_]
    timing-out: [_] -> w75
    stop <- w1735 stop-if-true
    n1114 = node-c288() -> ()  [unwired: 2 out]
    n1115 = event shown="[0] \"Pane\": Mouse Down" {
      selector: _ -> [_ _]
      dyn-events: _ -> [_ _]
      timeout: _ -> [_ _]
      tunnel: w1734 -> [w1738 _]
      event Mouse Down {
        n1116 = event-data() -> ("Time"=w1740:u32, "Coords"=w1739:T7, "Button"=w1741:u16)  [unwired: 6 out]
        n1117 = case shown="1" w1741 {
          tunnel: w1740 -> [_ _ w1844]
          tunnel: w1739 -> [_ w1778 w1842]
          tunnel: w1738 -> [_ _ w1840]
          frame 0, Default {
          }
          frame 1 {
            n1118 = property on="APD 2" class="ImageControl"() -> ("Displayed Image Position"=w1748:cluster{"Left":i32, "Top":i32})  [unwired: 2 in, 2 out]
            n1119 = property on="APD 1" class="ImageControl"() -> ("Displayed Image Position"=w1777:cluster{"Left":i32, "Top":i32})  [unwired: 2 in, 2 out]
            n1120 = property on="Detection Laser X" class="ImageControl"() -> ("Displayed Image Position"=w1774:cluster{"Left":i32, "Top":i32})  [unwired: 2 in, 2 out]
            n1121 = property on="Detection Laser Y" class="ImageControl"() -> ("Displayed Image Position"=w1773:cluster{"Left":i32, "Top":i32})  [unwired: 2 in, 2 out]
            n1122 = property on="APD 2" class="ImageControl"() -> ("Displayed Image Size"=w1747:cluster{"Width":u32, "Height":u32})  [unwired: 2 in, 2 out]
            n1123 = property on="APD 1" class="ImageControl"() -> ("Displayed Image Size"=w1775:cluster{"Width":u32, "Height":u32})  [unwired: 2 in, 2 out]
            n1124 = property on="Detection Laser X" class="ImageControl"() -> ("Displayed Image Size"=w1776:cluster{"Width":u32, "Height":u32})  [unwired: 2 in, 2 out]
            n1125 = property on="Detection Laser Y" class="ImageControl"() -> ("Displayed Image Size"=w1772:cluster{"Width":u32, "Height":u32})  [unwired: 2 in, 2 out]
            n1126 = Unbundle By Name(w1747) -> ("Width"=w1744:u32, "Height"=w1743:u32)
            n1127 = Unbundle By Name(w1748) -> ("Left"=w1746:i32, "Top"=w1745:i32)
            n1128 = Unbundle By Name(w1775) -> ("Width"=w1769:u32, "Height"=w1768:u32)
            n1129 = Unbundle By Name(w1776) -> ("Width"=w1765:u32, "Height"=w1764:u32)
            n1130 = Unbundle By Name(w1772) -> ("Width"=w1761:u32, "Height"=w1760:u32)
            n1131 = Unbundle By Name(w1777) -> ("Left"=w1771:i32, "Top"=w1770:i32)
            n1132 = Unbundle By Name(w1774) -> ("Left"=w1767:i32, "Top"=w1766:i32)
            n1133 = Unbundle By Name(w1773) -> ("Left"=w1763:i32, "Top"=w1762:i32)
            n1134 = Bundle("Left"=w1746, "Top"=w1745, "Width"=w1744, "Height"=w1743) -> (w1742:T33)  [unwired: 1 in]
            n1135 = Bundle("Left"=w1771, "Top"=w1770, "Width"=w1769, "Height"=w1768) -> (w1759:T33)  [unwired: 1 in]
            n1136 = Bundle("Left"=w1767, "Top"=w1766, "Width"=w1765, "Height"=w1764) -> (w1758:T33)  [unwired: 1 in]
            n1137 = Bundle("Left"=w1763, "Top"=w1762, "Width"=w1761, "Height"=w1760) -> (w1757:T33)  [unwired: 1 in]
            n1138 = Build Cluster Array(w1742, w1759, w1758, w1757) -> (w1756:T34)
            n1139 = for {
              tunnel: w1778 -> [w1789]
              tunnel: w1756 -> [w1790] mode=indexing
              shift-right: [w1787] -> w1754
              shift-left: TRUE -> [w1788]
              shift-right: [w1786] -> w1752
              shift-left: _ -> [w1782]
              shift-right: [w1785] -> w1751
              shift-left: _ -> [w1781]
              shift-right: [w1784] -> w1750
              shift-left: _ -> [w1780]
              shift-right: [w1783] -> w1749
              shift-left: _ -> [w1779]
              n1140 = case shown="True" w1788 {
                selector: w1788 -> [w1795 _]
                tunnel: w1790 -> [_ w1804]
                tunnel: w1789 -> [_ w1802]
                tunnel: [w1795 w1800] -> w1787
                tunnel: [w1794 w1799] -> w1786
                tunnel: [w1793 w1798] -> w1785
                tunnel: [w1792 w1797] -> w1784
                tunnel: [w1791 w1796] -> w1783
                tunnel: w1782 -> [w1794 _]
                tunnel: w1781 -> [w1793 _]
                tunnel: w1780 -> [w1792 _]
                tunnel: w1779 -> [w1791 _]
                frame False {
                }
                frame True {
                  n1141 = Unbundle(w1804) -> (w1803:T33)
                  n1142 = call "isclickinwindow.vi"("Image Param"=w1803, "Point32"=w1802) -> ("4 Y"=w1796:i32, "3 Height"=w1797:i32, "2 X"=w1798:i32, "1 Width"=w1799:i32, "In image?"=w1801:bool)  [unwired: 1 in]
                  n1143 = Not(x=w1801) -> (.not. x?=w1800:bool)
                }
              }
            }
            n1144 = Not(x=w1754) -> (.not. x?=w1753:bool)
            n1145 = case shown="True" w1753 {
              tunnel: w1751 -> [_ w1817]
              tunnel: w1749 -> [_ w1816]
              tunnel: w1752 -> [_ w1815]
              tunnel: w1750 -> [_ w1814]
              frame False {
              }
              frame True {
                w1810 = FALSE ("Get Point")
                n1146 = local read "Scan lines (y)"() -> (w1819:u64)
                n1147 = local read "Actual MCL Inc (V)"() -> (w1811:dbl)
                n1148 = local read "Scan steps (MCL)"() -> (w1818:u64)
                n1149 = Divide "Y Pix/step"(x=w1814, y=w1819) -> (x/y=w1826:dbl)
                n1150 = Divide "Y V/pix"(x=w1811, y=w1826) -> (x/y=w1825:dbl)
                n1151 = Divide "Y half step offset"(x=w1811, y=2.0) -> (x/y=w1827:dbl)
                n1152 = Divide "X pix/step"(x=w1815, y=w1818) -> (x/y=w1824:dbl)
                n1153 = Negate(x=w1827) -> (-x=w1828:dbl)
                n1154 = local read "Initial Y"() -> (w1834:dbl)
                n1155 = Multiply(x=w1816, y=w1825) -> (x*y=w1835:dbl)
                n1156 = Divide "X half step offset"(x=w1811, y=2.0) -> (x/y=w1821:dbl)
                n1157 = Divide "X V/pix"(x=w1811, y=w1824) -> (x/y=w1823:dbl)
                n1158 = Multiply(x=w1811, y=w1818) -> (x*y=w1830:dbl)
                n1159 = Compound Arithmetic op=ADD(w1828, w1835, w1834) -> (w1812:dbl)
                "Pointer Y (V)" <- w1812
                n1160 = Multiply(x=w1823, y=w1817) -> (x*y=w1832:dbl)
                n1161 = Negate(x=w1821) -> (-x=w1820:dbl)
                n1162 = local read "Initial X"() -> (w1833:dbl)
                n1163 = Negate(x=w1832) -> (-x=w1831:dbl)
                n1164 = Compound Arithmetic op=ADD(w1820, w1830, w1833, w1831) -> (w1813:dbl)
                "Pointer X (V)" <- w1813
                n1165 = Or(x="Set X Only", y="Set Confocal Spot (X-Y)") -> (x .or. y?=w1806:bool)
                n1166 = Or(x="Set Confocal Spot (X-Y)", y="Set Y Only") -> (x .or. y?=w1805:bool)
                n1167 = case shown="True" w1806 {
                  tunnel: w1813 -> [_ w1836]
                  frame False {
                  }
                  frame True {
                    n1168 = property on="AO2" class="Slide (strict)"("Val(Sgnl)"=w1836) -> ()  [unwired: 2 in, 2 out]
                  }
                }
                n1169 = case shown="True" w1805 {
                  tunnel: w1812 -> [_ w1837]
                  frame False {
                  }
                  frame True {
                    n1170 = property on="AO1" class="Slide (strict)"("Val(Sgnl)"=w1837) -> ()  [unwired: 2 in, 2 out]
                  }
                }
                n1171 = local write "Set Confocal Spot (X-Y)"(w1810) -> ()
                n1172 = local write "Set X Only"(w1810) -> ()
                n1173 = local write "Set Y Only"(w1810) -> ()
              }
            }
          }
          frame 3 {
            n1174 = local read "BD 2 Frequency 1 (MHz)"() -> (w1838:dbl)
            n1175 = local read "BD 1 Frequency 1 (MHz)"() -> (w1839:dbl)
            n1176 = local write "Manipulating Trap"(TRUE ("Manipulating Trap")) -> ()
            n1177 = local write "Coords"(T7 {"Horizontal"=0, "Vertical"=0} ("Coords")) -> ()
            n1178 = while {
              tunnel: w1844 -> [w1849]
              tunnel: w1842 -> [w1848]
              tunnel: w1840 -> [w1847]
              tunnel: w1839 -> [w1846]
              tunnel: w1838 -> [w1845]
              stop <- w1850 stop-if-true
              n1179 = event shown="[0] \"Pane\": Mouse Move" {
                selector: _ -> [_ _]
                dyn-events: _ -> [_ _]
                timeout: _ -> [_ _]
                tunnel: ["Force Manip Abort" w1914] -> w1850
                tunnel: w1849 -> [w1857 _]
                tunnel: w1848 -> [w1855 _]
                tunnel: w1847 -> [w1854 _]
                tunnel: w1846 -> [w1853 _]
                tunnel: w1845 -> [w1852 _]
                event Mouse Move {
                  n1180 = event-data() -> ("Time"=w1858:u32, "Coords"=w1859:T7)  [unwired: 3 out]
                  n1181 = Less?(x=w1858, y=w1857) -> (x < y?=w1856:bool)
                  n1182 = case "Makes sure old motion events prior to mouse click aren't used" shown="False" w1856 {
                    tunnel: w1859 -> [w1901 _]
                    tunnel: w1855 -> [w1902 _]
                    tunnel: w1854 -> [w1879 _]
                    tunnel: w1853 -> [w1875 _]
                    tunnel: w1852 -> [w1874 _]
                    frame False {
                      n1183 = Subtract(x=w1901, y=w1902) -> (x-y=w1900:T7)
                      "Coords" <- w1900
                      n1184 = local read "Y RF Frequency Limits (MHz)"() -> (w1860:T16)
                      n1185 = To Double Precision Float(number=w1900) -> (double precision float=w1899:cluster{"Horizontal":dbl, "Vertical":dbl})
                      n1186 = Multiply(x=cluster{"Horizontal":dbl, "Vertical":dbl} {"Horizontal"=-1.0, "Vertical"=1.0}, y="Manipulation Scaling") -> (x*y=w1895:cluster{"Horizontal":dbl, "Vertical":dbl})
                      n1187 = local read "X RF Frequency Limits (MHz)"() -> (w1861:T16)
                      n1188 = Multiply(x=w1899, y=w1895) -> (x*y=w1897:cluster{"Horizontal":dbl, "Vertical":dbl})
                      n1189 = Unbundle By Name(w1897) -> ("Horizontal"=w1892:dbl, "Vertical"=w1896:dbl)
                      n1190 = Unbundle By Name(w1860) -> ("Maximum"=w1863:dbl, "Minimum"=w1862:dbl)
                      n1191 = Boolean To (0,1)(Boolean="Manip. X?") -> (0, 1=w1890:i16)
                      n1192 = Boolean To (0,1)(Boolean="Manip. Y?") -> (0, 1=w1887:i16)
                      n1193 = local read "BD 1 Frequency 2 (MHz)"() -> (w1877:dbl)
                      n1194 = Multiply(x=w1896, y=w1887) -> (x*y=w1889:dbl)
                      n1195 = Multiply(x=w1890, y=w1892) -> (x*y=w1893:dbl)
                      n1196 = local read "BD 2 Frequency 2 (MHz)"() -> (w1876:dbl)
                      n1197 = Unbundle By Name(w1861) -> ("Maximum"=w1865:dbl, "Minimum"=w1864:dbl)
                      n1198 = Add(x=w1874, y=w1889) -> (x+y=w1867:dbl)
                      n1199 = Add(x=w1875, y=w1893) -> (x+y=w1869:dbl)
                      n1200 = In Range and Coerce(upper limit=w1865, x=w1869, lower limit=w1864) -> (coerced(x)=w1868:dbl)  [unwired: 1 out]
                      n1201 = In Range and Coerce(upper limit=w1863, x=w1867, lower limit=w1862) -> (coerced(x)=w1866:dbl)  [unwired: 1 out]
                      n1202 = Subtract(x=w1868, y=w1877) -> (x-y=w1886:dbl)
                      n1203 = Subtract(x=w1866, y=w1876) -> (x-y=w1885:dbl)
                      n1204 = Square(x=w1886) -> (x^2=w1884:dbl)
                      n1205 = Square(x=w1885) -> (x^2=w1883:dbl)
                      n1206 = Add(x=w1884, y=w1883) -> (x+y=w1882:dbl)
                      n1207 = Square Root(x=w1882) -> (sqrt(x)=w1878:dbl)
                      n1208 = In Range and Coerce(upper limit="Limit Max (MHz)", x=w1878, lower limit="Limit Min (MHz)") -> (In Range?=w1871:bool)  [unwired: 1 out]
                      n1209 = Not(x="Limits Enable") -> (.not. x?=w1870:bool)
                      n1210 = Or(x=w1871, y=w1870) -> (x .or. y?=w1872:bool)
                      n1211 = case shown="True" w1872 {
                        tunnel: w1879 -> [_ w1912]
                        tunnel: w1878 -> [_ w1903]
                        tunnel: w1868 -> [_ w1910]
                        tunnel: w1877 -> [_ w1909]
                        tunnel: w1866 -> [_ w1908]
                        tunnel: w1876 -> [_ w1907]
                        tunnel: w1861 -> [_ w1905]
                        tunnel: w1860 -> [_ w1904]
                        frame False {
                        }
                        frame True {
                          n1212 = local read "BD 1 Frequency 3 (MHz)"() -> (w1911:dbl)
                          n1213 = local read "BD 2 Frequency 3 (MHz)"() -> (w1906:dbl)
                          n1214 = local write "Trap Delta (MHz)"(w1903) -> ()
                          n1215 = property on="Initial delta (MHz)" class="DigNum (strict)"("Val(Sgnl)"=w1903) -> ()  [unwired: 2 in, 2 out]
                          n1216 = call "set RF board frequency - interlace.vi"("Board 2 Frequency Limits"=w1904, "Board 1 Frequency Limits"=w1905, "FPGA VI Reference In"=w1912, "Board 2 Frequency 3 (MHz)"=w1906, "Board 1 Frequency 3 (MHz)"=w1911, "Board 2 Frequency 2 (MHz)"=w1907, "Board 2 Frequency 1 (MHz)"=w1908, "Board 1 Frequency 2 (MHz)"=w1909, "Board 1 Frequency 1  (MHz)"=w1910) -> ()  [unwired: 1 in, 2 out]
                          n1217 = local write "BD 2 Frequency 1 (MHz)"(w1908) -> ()
                          n1218 = local write "BD 1 Frequency 1 (MHz)"(w1910) -> ()
                        }
                      }
                    }
                    frame True {
                    }
                  }
                }
                event Mouse Up {
                  n1219 = event-data() -> ("Button"=w1913:u16)  [unwired: 8 out]
                  n1220 = case shown="3" w1913 {
                    tunnel: [FALSE TRUE] -> w1914
                    frame 0, Default {
                    }
                    frame 3 {
                      n1221 = local write "Manipulating Trap"(FALSE ("Manipulating Trap")) -> ()
                    }
                  }
                }
              }
            }
          }
        }
      }
      event Mouse Move {
        n1222 = event-data() -> ()  [unwired: 6 out]
      }
    }
    n1223 = local read "Stop All"() -> (w1735:bool)
    n1224 = node-c288() -> ()  [unwired: 2 out]
  }
  n1225 = node-c288(i64 1 ("Period"), 1 ("Processor")) -> (w164:T24)  [unwired: 2 out]
  n1226 = timed-loop "Acquire Data" {
    tunnel: w24 -> [w2172]
    tunnel: w40 -> [w2171]
    tunnel: [w2202] -> w33
    tunnel: [w2196] -> w32
    timing: w164 -> [_]
    timing-out: [_] -> w163
    tunnel: w59 -> [w2000]
    stop <- "Stop All" stop-if-true
    (unwired) u32 0 ("Number of Elements")
    w1987 = "NI_ChannelName" ("name")
    n1227 = node-c288() -> ()  [unwired: 2 out]
    n1228 = First Call?() -> (First Call?: T/F=w1953:bool)
    n1229 = Or(x="Reset", y=w1953) -> (x .or. y?=w1954:bool)
    n1230 = case "Reset data stream" shown="True" w1954 {
      tunnel: w2172 -> [w2218 w2226]
      tunnel: w2171 -> [w2217 w2225]
      tunnel: [w2218 w2220] -> w2167
      tunnel: [w2217 w2219] -> w2166
      frame False {
      }
      frame True {
        w2223 = TRUE ("AI to FIFO")
        n1231 = local write "Overflow (data lost)"(FALSE ("Overflow (data lost)")) -> ()
        n1232 = call "reset FPGA DMA.vi"("error in"=w2225, "FPGA VI Reference In"=w2226) -> ("error out"=w2221:errorcluster, "FPGA VI Reference Out"=w2222:T19)
        n1233 = xnode "Read/Write Control"("FPGA VI Reference In"=w2222, "error in"=w2221, "AI to FIFO"=w2223, "APD to FIFO"=w2223) -> ("FPGA VI Reference Out"=w2220:T19, "error out"=w2219:errorcluster)
      }
    }
    n1234 = Or(x="Start AOD Scan", y="Trap Raster Scan") -> (x .or. y?=w2117:bool)
    n1235 = case "Start AOM raster scan" shown="True" w2117 {
      tunnel: w2167 -> [w2955 w2965]
      tunnel: w2166 -> [w2954 w2964]
      tunnel: [w2955 w2958] -> w2165
      tunnel: [w2954 w2957] -> w2164
      frame False {
      }
      frame True {
        n1236 = case shown="True" "Restart DMA? (AOD)" {
          tunnel: [w3003 w3005] -> w2959
          tunnel: [w3002 w3004] -> w2960
          tunnel: w2965 -> [w3003 w3007]
          tunnel: w2964 -> [w3002 w3006]
          frame False {
          }
          frame True {
            n1237 = local write "Overflow (data lost)"(FALSE ("Overflow (data lost)")) -> ()
            n1238 = call "reset FPGA DMA.vi"("error in"=w3006, "FPGA VI Reference In"=w3007) -> ("error out"=w3004:errorcluster, "FPGA VI Reference Out"=w3005:T19)
          }
        }
        n1239 = local write "Trap Raster Scan"(FALSE ("Trap Raster Scan")) -> ()
        n1240 = case shown="False" "Move MCL Also?" {
          tunnel: w2960 -> [w2968 w2997]
          tunnel: w2959 -> [w2969 w2998]
          tunnel: [w2967 w3001] -> w2958
          tunnel: [w2966 w3000] -> w2957
          frame False {
            w2970 = TRUE ("AI to FIFO")
            n1241 = xnode "Read/Write Control"("FPGA VI Reference In"=w2969, "error in"=w2968, "AI to FIFO"=w2970, "APD to FIFO"=w2970, "Start scan"=w2970) -> ("FPGA VI Reference Out"=w2967:T19, "error out"=w2966:errorcluster)
          }
          frame True {
            w2994 = FALSE ("1D or 2D Scan?")
            w2999 = TRUE ("AI to FIFO")
            # "Count for MCL loop"
            # "N total cycles"
            # "N steps"
            # "V_int"
            n1242 = local read "Scan Range (nm)"() -> (w2976:dbl)
            n1243 = local read "Number of F/B Scans (AOD)"() -> (w2993:u16)
            n1244 = Sign(1:w2976) -> (0:w2975:dbl)
            n1245 = Compound Arithmetic op=MULTIPLY(w2976, "MCL Step Position Ratio", "MCL/AOM Scale Tweak") -> (w2980:dbl)
            n1246 = Negate(x=w2975) -> (-x=w2972:dbl)
            n1247 = Multiply(x=w2972, y="MCL Step Increment (V_int)") -> (x*y=w2974:dbl)
            n1248 = Divide(x=w2980, y="MCL X Cal (nm/V)") -> (x/y=w2986:dbl)
            n1249 = Multiply(x=32767.0 ("y"), y=w2986) -> (x*y=w2992:dbl)
            n1250 = local read "Total Counts (ticks)"() -> (w2977:u32)
            n1251 = local read "Cycles/step (AOD)"() -> (w2988:u64)
            n1252 = local read "Scan steps (AOD)"() -> (w2989:u64)
            n1253 = Divide(x=w2992, y=10.0) -> (x/y=w2985:dbl)
            n1254 = Divide(x=w2985, y="MCL Step Increment (V_int)") -> (x/y=w2983:dbl)
            n1255 = Absolute Value(x=w2983) -> (abs(x)=w2971:dbl)
            n1256 = Compound Arithmetic op=MULTIPLY(w2989, w2988, w2977) -> (w2984:u64)
            n1257 = local write "wait to reset values"(w2999) -> ()
            n1258 = local write "MCL Scanning"(w2999) -> ()
            n1259 = Divide(x=w2984, y=w2971) -> (x/y=w2981:dbl)
            "MCL Count" <- w2981
            n1260 = xnode "Read/Write Control"("FPGA VI Reference In"=w2998, "error in"=w2997, "Scan steps (MCL)"=w2971, "Number of scans (MCL)"=w2993, "Cycles per step (MCL)"=u64 1, "Scan freq.  increment (MCL)"=w2974, "1D or 2D Scan?"=w2994, "MCL Scan Axis"=w2994, "Cont. Scan (MCL)"=w2994, "MCL count"=w2981) -> ("FPGA VI Reference Out"=w2996:T19, "error out"=w2995:errorcluster)
            n1261 = xnode "Read/Write Control"("FPGA VI Reference In"=w2996, "error in"=w2995, "AI to FIFO"=w2999, "APD to FIFO"=w2999, "Start scan"=w2999, "Start scan (MCL)"=w2999) -> ("FPGA VI Reference Out"=w3001:T19, "error out"=w3000:errorcluster)
          }
        }
        "Raster Scanning..." <- TRUE ("Scanning...")
      }
    }
    n1262 = And(x="Save scans", y=w2117) -> (x .and. y?=w2163:bool)
    n1263 = Compound Arithmetic op=OR("Start MCL Scan", "Confocal Image", "Confocal Linescan") -> (w2115:bool)
    n1264 = And(x="Save Data (MCL)", y=w2115) -> (x .and. y?=w2162:bool)
    n1265 = case "Start MCL raster scan" shown="True" w2115 {
      tunnel: w2165 -> [w2509 w2524]
      tunnel: w2164 -> [w2508 w2523]
      tunnel: [w2509 w2519] -> w1922
      tunnel: [w2508 w2518] -> w1921
      tunnel: [FALSE w2517] -> w2148
      tunnel: "Start MCL Scan" -> [_ w2512]
      tunnel: "Confocal Image" -> [_ w2511]
      tunnel: "Confocal Linescan" -> [_ _]
      frame False {
      }
      frame True {
        w2517 = TRUE
        n1266 = case shown="True" "Restart DMA? (MCL)" {
          tunnel: [w2569 w2571] -> w2522
          tunnel: [w2568 w2570] -> w2521
          tunnel: w2524 -> [w2569 w2574]
          tunnel: w2523 -> [w2568 w2573]
          frame False {
          }
          frame True {
            n1267 = call "reset FPGA DMA.vi"("error in"=w2573, "FPGA VI Reference In"=w2574) -> ("error out"=w2570:errorcluster, "FPGA VI Reference Out"=w2571:T19)
            n1268 = local write "Overflow (data lost)"(FALSE ("Overflow (data lost)")) -> ()
          }
        }
        n1269 = case shown="False" w2512 {
          selector: w2512 -> [_ w2528]
          tunnel: w2511 -> [w2527 _]
          tunnel: [w2527 w2528] -> w2510
          frame False {
            n1270 = property on="2D or 1D Scan" class="Bool (strict)"("Val(Sgnl)"=w2527) -> ()  [unwired: 2 in, 2 out]
            n1271 = property on="Confocal Image" class="Bool (strict)"("Value"=FALSE ("Start Confocal Map")) -> ()  [unwired: 2 in, 2 out]
          }
          frame True {
          }
        }
        n1272 = local write "MCL Scanning"(w2517) -> ()
        n1273 = local read "AO1"() -> (w2514:dbl)
        n1274 = local read "AO2"() -> (w2513:dbl)
        n1275 = case shown="True" "Center Scan" {
          tunnel: w2522 -> [w2535 w2567]
          tunnel: w2521 -> [w2534 w2566]
          tunnel: [w2533 w2565] -> w2519
          tunnel: [w2532 w2564] -> w2518
          tunnel: [w2530 w2551] -> w2516
          tunnel: [w2529 w2550] -> w2515
          tunnel: w2514 -> [w2530 w2556]
          tunnel: w2513 -> [w2529 w2559]
          tunnel: w2510 -> [_ _]
          frame False {
            w2531 = TRUE ("AI to FIFO")
            n1276 = xnode "Read/Write Control"("FPGA VI Reference In"=w2535, "error in"=w2534, "AI to FIFO"=w2531, "APD to FIFO"=w2531, "Start scan (MCL)"=w2531) -> ("FPGA VI Reference Out"=w2533:T19, "error out"=w2532:errorcluster)
          }
          frame True {
            w2563 = TRUE ("AI to FIFO")
            n1277 = local read "Scan steps (MCL)"() -> (w2542:u64)
            n1278 = local read "Scan lines (y)"() -> (w2538:u64)
            n1279 = local read "Fast Scan Dir"() -> (w2549:bool)
            n1280 = local read "Actual MCL Inc (V)"() -> (w2539:dbl)
            n1281 = Decrement(x=w2538) -> (x-1=w2537:u64)
            n1282 = Decrement(x=w2542) -> (x-1=w2541:u64)
            n1283 = Multiply(x=w2539, y=w2537) -> (x*y=w2536:dbl)
            n1284 = Divide(x=w2536, y=2.0) -> (x/y=w2546:dbl)
            n1285 = Multiply(x=w2539, y=w2541) -> (x*y=w2540:dbl)
            n1286 = Divide(x=w2540, y=2.0) -> (x/y=w2545:dbl)
            n1287 = Select(t=w2545, s=w2549, f=w2546) -> (s? t:f=w2544:dbl)
            n1288 = Select(t=w2546, s=w2549, f=w2545) -> (s? t:f=w2548:dbl)
            n1289 = Subtract(x=w2556, y=w2548) -> (x-y=w2547:dbl)
            n1290 = Subtract(x=w2559, y=w2544) -> (x-y=w2543:dbl)
            n1291 = local read "2D or 1D Scan"() -> (w2561:bool)
            n1292 = Not(x=w2549) -> (.not. x?=w2555:bool)
            n1293 = Not(x=w2561) -> (.not. x?=w2557:bool)
            n1294 = And(x=w2549, y=w2557) -> (x .and. y?=w2558:bool)
            n1295 = And(x=w2557, y=w2555) -> (x .and. y?=w2560:bool)
            n1296 = Select(t=w2559, s=w2560, f=w2543) -> (s? t:f=w2550:dbl)
            n1297 = Select(t=w2556, s=w2558, f=w2547) -> (s? t:f=w2551:dbl)
            n1298 = call "Volt to I16.vi"("Voltage In"=w2551) -> ("I16 Voltage Out"=w2554:i16)
            n1299 = call "Volt to I16.vi"("Voltage In"=w2550) -> ("I16 Voltage Out"=w2553:i16)
            n1300 = xnode "Read/Write Control"("FPGA VI Reference In"=w2567, "error in"=w2566, "AI to FIFO"=w2563, "APD to FIFO"=w2563, "Start scan (MCL)"=w2563, "AO1"=w2554, "AO2"=w2553) -> ("FPGA VI Reference Out"=w2565:T19, "error out"=w2564:errorcluster)
          }
        }
        "Initial Y" <- w2516
        "Initial X" <- w2515
        "wait to reset values" <- w2517
      }
    }
    n1301 = local read "Trap Pos Elements/DMA read"() -> (w1996:u32)
    n1302 = local read "Trap AI Elements/DMA read"() -> (w1920:u32)
    n1303 = local read "APD Elements/DMA read"() -> (w2039:u32)
    n1304 = local read "Trap AI FIFO Depth"() -> (w2212:u32)
    n1305 = xnode "Invoke Method"("FPGA VI Reference In"=w1922, "error in"=w1921, "Number of Elements"=w1996, "Timeout (ms)"=-1) -> ("Data"=w1960:u16[], "Elements Remaining"=→"Trap Pos FIFO El Remaining":u32)  [unwired: 2 out]
    n1306 = xnode "Invoke Method"("FPGA VI Reference In"=w1922, "error in"=w1921, "Number of Elements"=w1920, "Timeout (ms)"=-1 ("Timeout")) -> ("FPGA VI Reference Out"=w1924:T19, "error out"=w1923:errorcluster, "Data"=w1919:i16[], "Elements Remaining"=w1925:u32)
    "Trap AI FIFO El. Rem." <- w1925
    n1307 = xnode "Get APD Data"("FPGA VI Reference In"=w1922, "error in"=w1921, "Number of Elements"=w2039, "Timeout (ms)"=-1) -> ("Data"=w2038:u32[], "Elements Remaining"=→"APD FIFO Elements Remaining":u32)  [unwired: 2 out]
    n1308 = Subtract(x=w2212, y=w1920) -> (x-y=w2211:u32)
    n1309 = Decimate 1D Array(w1960) -> (w1957:u16[], w1959:u16[], w1958:u16[])
    n1310 = Divide(x=w1925, y=w2211) -> (x/y=w2210:dbl)
    "Buffer Status" <- w2210
    n1311 = To Unsigned Long Integer(number=w1957) -> (unsigned 32bit integer=w1956:u32[])
    n1312 = Join Numbers(hi=w1959, lo=w1958) -> ((hi.lo)=w1955:u32[])
    n1313 = Equal?(x=w2210, y=1.0) -> (x = y?=w2208:bool)
    n1314 = Join Numbers(hi=w1956, lo=w1955) -> ((hi.lo)=w1949:u64[])
    n1315 = call "IR AOM word to freq - vec.vi"("Frequency Word In (double vec)"=w1949) -> ("Frequency Out"=w1995:dbl[])
    n1316 = case "Alert buffer overflow" shown="True" w2208 {
      frame False {
      }
      frame True {
        n1317 = call <vilib>:"Beep.vi"() -> ()  [unwired: 3 in, 9 out]
        "Overflow (data lost)" <- TRUE ("Overflow (data lost)")
      }
    }
    n1318 = Decimate 1D Array(w1995) -> (w1994:dbl[], w1993:dbl[])
    n1319 = Array Size(array=w1919) -> (size(s)=→"Waveform Chart":i32)
    n1320 = Build Array(w1994, w1993) -> (w1992:dbl[][])
    n1321 = local read "Trap Sets"() -> (w2076:u32)
    n1322 = case "Deinterlace trap data, average down PSD" shown="2" w2076 {
      tunnel: w1919 -> [w2604 w2669]
      tunnel: [w2601 w2666] -> w2069
      tunnel: [w2604 w2668] -> w1952
      tunnel: "Detector Type" -> [w2603 w2664]
      tunnel: [w2602 w2667] -> w2068
      tunnel: [w2600 w2665] -> w2183
      frame 1, Default {
        n1323 = Divide(x=w2604, y=3276.7) -> (x/y=w2605:dbl[])
        n1324 = Decimate 1D Array(w2605) -> (w2614:dbl[], w2613:dbl[], w2612:dbl[], w2611:dbl[], w2610:dbl[], w2609:dbl[], w2608:dbl[], w2607:dbl[])
        n1325 = case shown="\"IR-QPD + PSD + FB-QPD position\"" w2603 {
          tunnel: w2614 -> [w2638 w2663]
          tunnel: w2613 -> [w2637 w2662]
          tunnel: w2612 -> [w2622 w2640]
          tunnel: w2611 -> [w2623 w2650]
          tunnel: w2610 -> [w2636 w2661]
          tunnel: w2609 -> [w2635 w2660]
          tunnel: w2608 -> [w2619 w2641]
          tunnel: w2607 -> [w2618 w2639]
          tunnel: [w2617 w2647] -> w2602
          tunnel: [w2616 w2646] -> w2601
          tunnel: [w2615 w2645] -> w2600
          frame "IR-QPD + PSD + FB-QPD", Default {
            w2615 = 0  # Channel pattern
            n1326 = Divide(x=w2638, y=w2623) -> (x/y=w2625:dbl[])
            n1327 = Divide(x=w2637, y=w2623) -> (x/y=w2624:dbl[])
            n1328 = Divide(x=w2636, y=w2619) -> (x/y=w2621:dbl[])
            n1329 = Divide(x=w2635, y=w2618) -> (x/y=w2620:dbl[])
            n1330 = Build Array(w2625, w2624, w2623, w2622, w2621, w2620, w2619, w2618) -> (w2616:dbl[][])
            n1331 = Bundle("T1 Y", "T1 X", "T1 Sum", "FB Sum", "PSD Y", "PSD X", "PSD Y Sum", "PSD X Sum") -> (w2634:T41)  [unwired: 1 out]
            n1332 = Cluster To Array(cluster=w2634) -> (array=w2617:string[])
          }
          frame "IR-QPD + PSD + FB-QPD position" {
            w2645 = 3  # Channel pattern
            n1333 = Negate(x=w2641) -> (-x=w2642:dbl[])
            n1334 = Divide(x=w2663, y=w2650) -> (x/y=w2652:dbl[])
            n1335 = Divide(x=w2662, y=w2650) -> (x/y=w2651:dbl[])
            n1336 = Divide(x=w2661, y=w2641) -> (x/y=w2649:dbl[])
            n1337 = Divide(x=w2660, y=w2642) -> (x/y=w2648:dbl[])
            n1338 = Build Array(w2652, w2651, w2650, w2639, w2640, w2649, w2648, w2641) -> (w2646:dbl[][])
            n1339 = Bundle("T1 Y", "T1 X", "T1 Sum", "FB X", "FB Sum", "PSD Y", "PSD X", "PSD Y Sum") -> (w2659:T41)  [unwired: 1 out]
            n1340 = Cluster To Array(cluster=w2659) -> (array=w2647:string[])
          }
        }
      }
      frame 2 {
        n1341 = case shown="\"UCB Fleezers 052511\"" w2664 {
          tunnel: w2669 -> [w2731 w2798 w2826 w2933]
          tunnel: [w2670 w2790 w2821 w2864] -> w2668
          tunnel: [w2697 w2781 w2823 w2911] -> w2667
          tunnel: [w2696 w2745 w2800 w2878] -> w2666
          tunnel: [w2690 w2780 w2863 w2909] -> w2665
          frame "IR-QPD + PSD + FB-QPD", Default {
            w2690 = 1  # Channel pattern
            # "time average x2 the 4th signal and the 4 psd signals (detection laser)"
            # "deinterlace 3 signals from qpd"
            n1342 = Decimate 1D Array(w2731) -> (w2730:i16[], w2729:i16[], w2695:i16[], w2728:i16[], w2718:i16[], w2716:i16[], w2715:i16[], w2713:i16[])
            n1343 = call "downsample 1D array - double.vi"("Ave N"=2.0, "Array In"=w2718) -> ("Array Out"=w2717:dbl[])  [unwired: 1 out]
            n1344 = call "downsample 1D array - double.vi"("Ave N"=2.0, "Array In"=w2713) -> ("Array Out"=w2712:dbl[])  [unwired: 1 out]
            n1345 = call "downsample 1D array - double.vi"("Ave N"=2.0, "Array In"=w2715) -> ("Array Out"=w2714:dbl[])  [unwired: 1 out]
            n1346 = call "downsample 1D array - double.vi"("Ave N"=2.0, "Array In"=w2716) -> ("Array Out"=w2698:dbl[])  [unwired: 1 out]
            n1347 = Decimate 1D Array(w2730) -> (w2727:i16[], w2699:i16[])
            n1348 = Decimate 1D Array(w2729) -> (w2726:i16[], w2724:i16[])
            n1349 = Decimate 1D Array(w2728) -> (w2725:i16[], w2723:i16[])
            n1350 = Decimate 1D Array(w2695) -> (w2694:i16[], w2693:i16[])
            n1351 = Interleave 1D Arrays(w2727, w2726, w2725, w2699, w2724, w2723, w2694, w2693, w2717, w2698, w2714, w2712) -> (w2711:dbl[])
            n1352 = To Word Integer(number=w2711) -> (16bit integer=w2670:i16[])
            n1353 = Divide(x=w2711, y=3276.7) -> (x/y=w2710:dbl[])
            n1354 = Decimate 1D Array(w2710) -> (w2709:dbl[], w2708:dbl[], w2707:dbl[], w2706:dbl[], w2705:dbl[], w2704:dbl[], w2692:dbl[], w2691:dbl[], w2703:dbl[], w2702:dbl[], w2701:dbl[], w2700:dbl[])
            n1355 = Divide(x=w2709, y=w2707) -> (x/y=w2677:dbl[])
            n1356 = Divide(x=w2708, y=w2707) -> (x/y=w2676:dbl[])
            n1357 = Divide(x=w2706, y=w2704) -> (x/y=w2675:dbl[])
            n1358 = Divide(x=w2705, y=w2704) -> (x/y=w2674:dbl[])
            n1359 = Divide(x=w2703, y=w2701) -> (x/y=w2673:dbl[])
            n1360 = Divide(x=w2702, y=w2700) -> (x/y=w2672:dbl[])
            n1361 = Bundle("T1 Y", "T1 X", "T1 Sum", "T2 Y", "T2 X", "T2 Sum", "T1 FB Sum", "T2 FB Sum", "PSD Y", "PSD X", "PSD Y Sum", "PSD X Sum") -> (w2678:T42)  [unwired: 1 out]
            n1362 = Build Array(w2677, w2676, w2707, w2675, w2674, w2704, w2692, w2691, w2673, w2672, w2701, w2700) -> (w2696:dbl[][])
            n1363 = Cluster To Array(cluster=w2678) -> (array=w2697:string[])
          }
          frame "IR-QPD + PSD + FB-QPD X position" {
            w2780 = 2  # Channel pattern
            # "convert\nADC numbers\nto volts"
            # "time average x2 the 3 psd signals (detection laser)"
            # "deinterlace 3 signals from qpds"
            n1364 = Decimate 1D Array(w2798) -> (w2797:i16[], w2796:i16[], w2733:i16[], w2734:i16[], w2743:i16[], w2740:i16[], w2737:i16[], w2768:i16[])
            n1365 = Decimate 1D Array(w2797) -> (w2795:i16[], w2782:i16[])
            n1366 = call "downsample 1D array - I16.vi"("Ave N"=2.0, "Array In"=w2743) -> ("Array Out"=w2741:i16[])  [unwired: 1 in]
            n1367 = call "downsample 1D array - I16.vi"("Ave N"=2.0, "Array In"=w2740) -> ("Array Out"=w2738:i16[])  [unwired: 1 in]
            n1368 = Decimate 1D Array(w2796) -> (w2794:i16[], w2792:i16[])
            n1369 = Decimate 1D Array(w2734) -> (w2793:i16[], w2791:i16[])
            n1370 = Decimate 1D Array(w2768) -> (w2767:i16[], w2765:i16[])
            n1371 = Decimate 1D Array(w2733) -> (w2766:i16[], w2764:i16[])
            n1372 = call "downsample 1D array - I16.vi"("Ave N"=2.0, "Array In"=w2737) -> ("Array Out"=w2735:i16[])  [unwired: 1 in]
            n1373 = Interleave 1D Arrays(w2795, w2794, w2793, w2782, w2792, w2791, w2767, w2766, w2765, w2764, w2741, w2738, w2735) -> (w2790:i16[])
            n1374 = Divide(x=w2790, y=3276.7) -> (x/y=w2789:dbl[])
            n1375 = Decimate 1D Array(w2789) -> (w2788:dbl[], w2787:dbl[], w2786:dbl[], w2785:dbl[], w2784:dbl[], w2783:dbl[], w2756:dbl[], w2754:dbl[], w2753:dbl[], w2751:dbl[], w2750:dbl[], w2749:dbl[], w2746:dbl[])
            n1376 = Divide(x=w2788, y=w2786) -> (x/y=w2772:dbl[])
            n1377 = Divide(x=w2787, y=w2786) -> (x/y=w2771:dbl[])
            n1378 = Divide(x=w2785, y=w2783) -> (x/y=w2770:dbl[])
            n1379 = Divide(x=w2784, y=w2783) -> (x/y=w2769:dbl[])
            n1380 = Divide(x=w2756, y=w2754) -> (x/y=w2755:dbl[])
            n1381 = Divide(x=w2753, y=w2751) -> (x/y=w2752:dbl[])
            n1382 = Divide(x=w2750, y=w2746) -> (x/y=w2748:dbl[])
            n1383 = Negate(x=w2746) -> (-x=w2744:dbl[])
            n1384 = Divide(x=w2749, y=w2744) -> (x/y=w2747:dbl[])
            n1385 = Bundle("T1 Y", "T1 X", "T1 Sum", "T2 Y", "T2 X", "T2 Sum", "T1 FB X", "T1 FB Sum", "T2 FB X", "T2 FB Sum", "PSD Y", "PSD X", "PSD Y Sum") -> (w2773:T43)  [unwired: 1 out]
            n1386 = Build Array(w2772, w2771, w2786, w2770, w2769, w2783, w2755, w2754, w2752, w2751, w2748, w2747, w2746) -> (w2745:dbl[][])
            n1387 = Cluster To Array(cluster=w2773) -> (array=w2781:string[])
          }
          frame "UCB Fleezers 052511" {
            w2863 = 2  # Channel pattern
            n1388 = Decimate 1D Array(w2826) -> (w2861:i16[], w2860:i16[], w2825:i16[], w2824:i16[], w2818:i16[], w2815:i16[], w2814:i16[], w2813:i16[])
            n1389 = Decimate 1D Array(w2861) -> (w2859:i16[], w2844:i16[])
            n1390 = Decimate 1D Array(w2860) -> (w2858:i16[], w2856:i16[])
            n1391 = Decimate 1D Array(w2825) -> (w2857:i16[], w2855:i16[])
            n1392 = Decimate 1D Array(w2824) -> (w2820:i16[], w2819:i16[])
            n1393 = Decimate 1D Array(w2818) -> (w2817:i16[], w2816:i16[])
            n1394 = call "downsample 1D array - I16.vi"("Ave N"=2.0, "Array In"=w2815) -> ("Array Out"=w2812:i16[])  [unwired: 1 in]
            n1395 = call "downsample 1D array - I16.vi"("Ave N"=2.0, "Array In"=w2814) -> ("Array Out"=w2811:i16[])  [unwired: 1 in]
            n1396 = call "downsample 1D array - I16.vi"("Ave N"=2.0, "Array In"=w2813) -> ("Array Out"=w2810:i16[])  [unwired: 1 in]
            n1397 = Interleave 1D Arrays(w2859, w2858, w2857, w2844, w2856, w2855, w2820, w2817, w2819, w2816, w2812, w2811, w2810) -> (w2821:i16[])
            n1398 = Divide(x=w2821, y=3276.7) -> (x/y=w2851:dbl[])
            n1399 = Decimate 1D Array(w2851) -> (w2850:dbl[], w2849:dbl[], w2848:dbl[], w2847:dbl[], w2846:dbl[], w2845:dbl[], w2809:dbl[], w2807:dbl[], w2806:dbl[], w2804:dbl[], w2803:dbl[], w2802:dbl[], w2801:dbl[])
            n1400 = Divide(x=w2850, y=w2848) -> (x/y=w2831:dbl[])
            n1401 = Divide(x=w2849, y=w2848) -> (x/y=w2830:dbl[])
            n1402 = Divide(x=w2847, y=w2845) -> (x/y=w2829:dbl[])
            n1403 = Divide(x=w2846, y=w2845) -> (x/y=w2828:dbl[])
            n1404 = Divide(x=w2809, y=w2807) -> (x/y=w2808:dbl[])
            n1405 = Divide(x=w2806, y=w2804) -> (x/y=w2805:dbl[])
            n1406 = Bundle("T1 Y", "T1 X", "T1 Sum", "T2 Y", "T2 X", "T2 Sum", "T1 FB X", "T2 FB Sum", "T2 FB X", "T2 FB Sum", "PSD Y", "PSD X", "PSD Sum") -> (w2832:T43)  [unwired: 1 out]
            n1407 = Build Array(w2831, w2830, w2848, w2829, w2828, w2845, w2808, w2807, w2805, w2804, w2803, w2802, w2801) -> (w2800:dbl[][])
            n1408 = Cluster To Array(cluster=w2832) -> (array=w2823:string[])
          }
          frame "IR-QPD + PSD + FB-QPD XY positions" {
            w2909 = 4  # Channel pattern
            # "time average x2 the 3 psd signals (detection laser)"
            # "deinterlace 3 signals from qpds"
            n1409 = Decimate 1D Array(w2933) -> (w2932:i16[], w2931:i16[], w2910:i16[], w2930:i16[], w2876:i16[], w2922:i16[], w2921:i16[], w2898:i16[])
            n1410 = Decimate 1D Array "QPD Y"(w2932) -> (w2929:i16[], w2912:i16[])
            n1411 = call "downsample 1D array - double.vi"("Ave N"=2.0, "Array In"=w2922) -> ("Array Out"=w2897:dbl[])  [unwired: 1 out]
            n1412 = call "downsample 1D array - double.vi"("Ave N"=2.0, "Array In"=w2921) -> ("Array Out"=w2896:dbl[])  [unwired: 1 out]
            n1413 = Decimate 1D Array "Feedback Sum"(w2910) -> (w2894:i16[], w2892:i16[])
            n1414 = Decimate 1D Array "Feedback Y"(w2876) -> (w2875:i16[], w2874:i16[])
            n1415 = Decimate 1D Array "Feedback X"(w2898) -> (w2895:i16[], w2893:i16[])
            n1416 = Decimate 1D Array "QPD Sum"(w2930) -> (w2927:i16[], w2925:i16[])
            n1417 = Decimate 1D Array "QPD X"(w2931) -> (w2928:i16[], w2926:i16[])
            n1418 = Interleave 1D Arrays(w2929, w2928, w2927, w2912, w2926, w2925, w2875, w2895, w2894, w2874, w2893, w2892, w2897, w2896) -> (w2920:dbl[])
            n1419 = To Word Integer(number=w2920) -> (16bit integer=w2864:i16[])
            n1420 = Divide(x=w2920, y=3276.7) -> (x/y=w2919:dbl[])
            n1421 = Decimate 1D Array(w2919) -> (w2918:dbl[], w2917:dbl[], w2916:dbl[], w2915:dbl[], w2914:dbl[], w2913:dbl[], w2871:dbl[], w2885:dbl[], w2869:dbl[], w2870:dbl[], w2883:dbl[], w2867:dbl[], w2881:dbl[], w2879:dbl[])
            n1422 = Divide(x=w2918, y=w2916) -> (x/y=w2902:dbl[])
            n1423 = Divide(x=w2917, y=w2916) -> (x/y=w2901:dbl[])
            n1424 = Divide(x=w2915, y=w2913) -> (x/y=w2900:dbl[])
            n1425 = Divide(x=w2914, y=w2913) -> (x/y=w2899:dbl[])
            n1426 = Divide(x=w2871, y=w2869) -> (x/y=w2868:dbl[])
            n1427 = Divide(x=w2885, y=w2869) -> (x/y=w2884:dbl[])
            n1428 = Divide(x=w2870, y=w2867) -> (x/y=w2866:dbl[])
            n1429 = Divide(x=w2883, y=w2867) -> (x/y=w2882:dbl[])
            n1430 = Negate(x=w2879) -> (-x=w2877:dbl[])
            n1431 = Divide(x=w2881, y=w2877) -> (x/y=w2880:dbl[])
            n1432 = Bundle("T1 Y", "T1 X", "T1 Sum", "T2 Y", "T2 X", "T2 Sum", "T1 FB Y", "T1 FB X", "T1 FB Sum", "T2 FB Y", "T2 FB X", "T2 FB Sum", "PSD X", "PSD Y Sum") -> (w2865:T44)  [unwired: 1 out]
            n1433 = Build Array(w2902, w2901, w2916, w2900, w2899, w2913, w2868, w2884, w2869, w2866, w2882, w2867, w2880, w2879) -> (w2878:dbl[][])
            n1434 = Cluster To Array(cluster=w2865) -> (array=w2911:string[])
          }
        }
      }
    }
    "AI labels" <- w2068
    n1435 = Decimate 1D Array(w2038) -> (w2066:u32[], w2002:u32[])
    n1436 = local read "DMA Update Period (s)"() -> (w2077:dbl)
    n1437 = local read "BD 1 Frequency 2 (MHz)"() -> (w1944:dbl)
    n1438 = local read "BD 1 Frequency 1 (MHz)"() -> (w1945:dbl)
    n1439 = Build Array(w2066, w2002) -> (w2145:u32[][])
    n1440 = local read "Data Period (s)"() -> (w2051:dbl)
    n1441 = Decimate 1D Array(w1952) -> (w1975:i16[], w1974:i16[], w1972:i16[], w1971:i16[])  [unwired: 9 out]
    n1442 = To Double Precision Float(number=w2145) -> (double precision float=w2146:dbl[][])
    n1443 = local read "APD Integration Time (s)"() -> (w2015:dbl)
    n1444 = Divide(x=w1975, y=w1974) -> (x/y=w1976:dbl[])
    n1445 = Divide(x=w1972, y=w1971) -> (x/y=w1973:dbl[])
    n1446 = feedback #1(0.0) -> (w1989:dbl)
    n1447 = Add(x=w2077, y=w1989) -> (x+y=w2185:dbl)
    n1448 = feedback-in #1(w2185) -> ()
    n1449 = local read "AOM X Cal (nm/MHz)"() -> (w1942:dbl)
    n1450 = To Time Stamp(1:w1989) -> (0:w1988:timestamp)
    n1451 = Split 1D Array(array=w1976, index="N El. to Ave.") -> (second subarray=w1979:dbl[])  [unwired: 1 out]
    n1452 = Split 1D Array(array=w1973, index="N El. to Ave.") -> (second subarray=w1978:dbl[])  [unwired: 1 out]
    n1453 = local read "Trap X AI1 (DMA)"() -> (w1977:T13)
    n1454 = Multiply(x=w2051, y="Trap Disp. Downsample") -> (x*y=w1990:dbl)
    "Display Period (s)" <- w1990
    n1455 = Bundle("BD 1 Frequency 1 (MHz)"=w1945, "BD 1 Frequency 2 (MHz)"=w1944) -> (w1946:T45)  [unwired: 1 out]
    n1456 = for "Trap AI" {
      tunnel: [w2599] -> w2179 mode=indexing
      tunnel: w1988 -> [w2589]
      tunnel: "Trap Disp. Downsample" -> [w2597]
      tunnel: w2069 -> [w2595] mode=indexing
      tunnel: w2051 -> [w2594]
      tunnel: w2068 -> [w2593] mode=indexing
      tunnel: w1987 -> [w2592]
      tunnel: [w2591] -> w2026 mode=indexing
      tunnel: w1990 -> [w2590]
      n1457 = Bundle By Name("Y"=w2595, "dt"=w2594) -> (w2596:waveform(dbl))  [unwired: 1 out]
      n1458 = Set Waveform Attribute(5:w2593, 6:w2592, 7:w2596) -> (3:w2591:waveform(dbl))  [unwired: 1 in, 2 out]
      n1459 = call "downsample 1D array - double.vi"("Ave N"=w2597, "Array In"=w2595) -> ("Array Out"=w2598:dbl[])  [unwired: 1 out]
      n1460 = Bundle By Name(cluster=w2591, "t0"=w2589, "Y"=w2598, "dt"=w2590) -> (w2599:waveform(dbl))
    }
    n1461 = call-poly <vilib>:"Mean.vi"("X"=w1978) -> ("mean"=w1966:dbl)  [unwired: 1 out]
    n1462 = call-poly <vilib>:"Mean.vi"("X"=w1979) -> ("mean"=w1967:dbl)  [unwired: 1 out]
    n1463 = Cluster To Array(cluster=w1946) -> (array=w1943:dbl[])
    n1464 = Reciprocal(x=w1990) -> (1/x=→"Trap Disp. Freq. (Hz)":dbl)
    n1465 = local read "Data points/scans (MCL)"() -> (w2157:dbl)
    n1466 = To Fixed-Point(number=w1966) -> (fixed-point=w1964:fxp<+/-,16,1>)  [unwired: 1 in]
    n1467 = To Fixed-Point(number=w1967) -> (fixed-point=w1965:fxp<+/-,16,1>)  [unwired: 1 in]
    n1468 = Bundle("Trap 1 Pos.", "Trap 2 Pos.") -> (w1986:cluster{string, string})  [unwired: 1 out]
    n1469 = Bundle By Name(cluster=w1977, "Set 1"=w1965, "Set 2"=w1964) -> (→"Trap X AI1 (DMA)":T13)
    n1470 = Cluster To Array(cluster=w1986) -> (array=w1983:string[])
    n1471 = for "Trap Position" {
      tunnel: w1992 -> [w2239] mode=indexing
      tunnel: "Trap Disp. Downsample" -> [w2238]
      tunnel: w1990 -> [w2236]
      tunnel: w1988 -> [w2235]
      tunnel: w1987 -> [w2233]
      tunnel: w1983 -> [w2232] mode=indexing
      tunnel: [w2231] -> w1941 mode=indexing
      tunnel: w1943 -> [w2229] mode=indexing
      tunnel: w1942 -> [w2227]
      n1472 = call "downsample 1D array - double.vi"("Ave N"=w2238, "Array In"=w2239) -> ("Array Out"=w2237:dbl[])  [unwired: 1 out]
      n1473 = Subtract(x=w2237, y=w2229) -> (x-y=w2230:dbl[])
      n1474 = Multiply(x=w2227, y=w2230) -> (x*y=w2228:dbl[])
      n1475 = Bundle By Name("Y"=w2228, "dt"=w2236, "t0"=w2235) -> (w2234:waveform(dbl))  [unwired: 1 out]
      n1476 = Set Waveform Attribute(5:w2232, 6:w2233, 7:w2234) -> (3:w2231:waveform(dbl))  [unwired: 1 in, 2 out]
    }
    "Trap Positions" <- w1941
    n1477 = Bundle("APD 1", "APD 2") -> (w2178:cluster{string, string})  [unwired: 1 out]
    n1478 = Cluster To Array(cluster=w2178) -> (array=w2175:string[])
    n1479 = for "APD" {
      tunnel: w2146 -> [w2578] mode=indexing
      tunnel: w2015 -> [w2586]
      tunnel: [w2582] -> w2022 mode=indexing
      tunnel: "APD Disp. Scale" -> [w2583]
      tunnel: w1987 -> [w2581]
      tunnel: w2175 -> [w2580] mode=indexing
      tunnel: "APD Disp. Downsample" -> [w2576]
      tunnel: [w2579] -> w2174
      tunnel: w1988 -> [w2575]
      n1480 = call "integrate 1D array interval - double.vi"("Ave N"=w2576, "Array In"=w2578) -> ("Array Out"=w2577:dbl[])  [unwired: 1 out]
      n1481 = Multiply(x=w2586, y=w2576) -> (x*y=w2579:dbl)
      n1482 = Divide(x=w2577, y=w2583) -> (x/y=w2584:dbl[])
      n1483 = Bundle By Name("t0"=w2575, "Y"=w2584, "dt"=w2579) -> (w2585:waveform(dbl))  [unwired: 1 out]
      n1484 = Set Waveform Attribute(5:w2580, 6:w2581, 7:w2585) -> (3:w2582:waveform(dbl))  [unwired: 1 in, 2 out]
    }
    "APD Display Period (s)" <- w2174
    n1485 = Reciprocal(x=w2174) -> (1/x=→"APD Display Freq. (Hz)":dbl)
    n1486 = local read "Display Period (s)"() -> (w2050:dbl)
    n1487 = Increment(x=w2157) -> (x+1=w2158:dbl)
    n1488 = Index Array(array=w1941, index=0) -> (element=w1939:waveform(dbl))
    n1489 = To Double Precision Float(number=w2066) -> (double precision float=w2065:dbl[])
    n1490 = feedback #2(w2158) -> (w2161:dbl)
    n1491 = Select(t=0, s=w2148, f=w2161) -> (s? t:f=w2154:dbl)
    n1492 = Array Size(array=w2065) -> (size(s)=w2160:i32)
    n1493 = Add(x=w2160, y=w2154) -> (x+y=w2155:dbl)
    n1494 = Unbundle By Name(w1939) -> ("Y"=w1937:dbl[])
    n1495 = feedback #3(w2066) -> (w2144:u32[])
    n1496 = Build Array (concatenate)(w2144, w2066) -> (w2141:u32[])
    n1497 = feedback #4(w2002) -> (w2021:u32[])
    n1498 = Divide(x="Bead Sep. Int. Time (s)", y=w2050) -> (x/y=w1935:dbl)
    n1499 = Build Array (concatenate)(w2021, w2002) -> (w2020:u32[])
    n1500 = Greater?(x=w2155, y=w2157) -> (0:w2156:bool)
    n1501 = feedback #5(w1937) -> (w1938:dbl[])
    n1502 = Build Array (concatenate)(w1937, w1938) -> (w1936:dbl[])
    n1503 = Select(t=w2154, s=w2156, f=w2155) -> (s? t:f=w2153:dbl)
    n1504 = feedback-in #2(w2153) -> ()
    n1505 = Array Size(array=w2141) -> (size(s)=w2138:i32)
    n1506 = Array Size(array=w2066) -> (size(s)=w2140:i32)
    n1507 = local read "MCL Scanning"() -> (w2151:bool)
    n1508 = local read "APD Integration Time (s)"() -> (w2029:dbl)
    n1509 = Build Array (concatenate)(w2022, w2179) -> (w2024:waveform(dbl)[])
    "All Signals" <- w2024
    n1510 = Split 1D Array(array=w1936, index=w1935) -> (first subarray=w1929:dbl[])  [unwired: 1 out]
    n1511 = feedback-in #5(w1929) -> ()
    n1512 = Multiply(x=w2140, y="APD Ave N") -> (x*y=w2139:dbl)
    n1513 = Greater?(x=w2138, y=w2139) -> (0:w2142:bool)
    n1514 = Not(x=w2156) -> (.not. x?=w2150:bool)
    n1515 = To Double Precision Float(number=w2002) -> (double precision float=w2001:dbl[])
    n1516 = call-poly <vilib>:"Mean.vi"("X"=w1929) -> ("mean"=w1928:dbl)  [unwired: 1 out]
    "Mean T1 Position (nm)" <- w1928
    n1517 = Subtract(x=w1929, y=w1928) -> (x-y=w1934:dbl[])
    n1518 = Square(x=w1934) -> (x^2=w1933:dbl[])
    n1519 = And(x=w2150, y=w2151) -> (x .and. y?=w2152:bool)
    n1520 = call-poly <vilib>:"Mean.vi"("X"=w1933) -> ("mean"=w1932:dbl)  [unwired: 1 out]
    n1521 = case shown="True" w2142 {
      tunnel: w2141 -> [w2359 w2366]
      tunnel: [w2359 w2364] -> w2082
      tunnel: w2139 -> [_ w2361]
      tunnel: w2138 -> [_ w2365]
      tunnel: w2020 -> [w2358 w2363]
      tunnel: [w2358 w2360] -> w2017
      frame False {
      }
      frame True {
        n1522 = Subtract(x=w2365, y=w2361) -> (x-y=w2362:dbl)
        n1523 = Array Subset(array=w2366, index=w2362, length=w2361) -> (w2364:u32[])
        n1524 = Array Subset(array=w2363, index=w2362, length=w2361) -> (w2360:u32[])
      }
    }
    n1525 = feedback-in #3(w2082) -> ()
    n1526 = feedback-in #4(w2017) -> ()
    n1527 = Or(x=w2152, y=w2148) -> (x .or. y?=w2149:bool)
    n1528 = Square Root(x=w1932) -> (sqrt(x)=w1931:dbl)
    n1529 = Equal?(x="Tab Control 6", y=T35."High Res Display") -> (x = y?=w2072:bool)
    n1530 = Multiply(x="APD Disp. Scale", y=w2022) -> (x*y=w2031:waveform(dbl)[])
    n1531 = Multiply(x="APD Disp. Downsample", y=w2029) -> (x*y=w2027:dbl)
    n1532 = Multiply(x=10.0, y=w1931) -> (x*y=→"Trap 1 Position RMS (A)":dbl)
    n1533 = Divide(x=w2031, y=w2027) -> (x/y=w1999:waveform(dbl)[])
    n1534 = Index Array(array=w1999, index=0) -> (element=w2009:waveform(dbl))
    n1535 = case "For computing FFTs for display" shown="True" "Compute FFT" {
      tunnel: w2026 -> [_ w3036]
      frame False {
      }
      frame True {
        n1536 = Build Array("FFT 1 Choice 1", "FFT 1 Choice 2", "FFT 2 Choice 1", "FFT 2 Choice 2") -> (w3029:u16[])
        n1537 = Array Size(array=w3036) -> (size(s)=w3035:i32)
        n1538 = feedback-in #6(w3029) -> ()
        n1539 = feedback #6(u16[] [100, 100, 100, 100]) -> (w3030:u16[])
        n1540 = feedback-in #7("# Spectra to Ave.") -> ()
        n1541 = feedback #7("# Spectra to Ave.") -> (w3027:dbl)
        n1542 = Not Equal?(x="# Spectra to Ave.", y=w3027) -> (x != y?=w3026:bool)
        n1543 = Not Equal?(x=w3029, y=w3030) -> (x != y?=w3028:bool)
        n1544 = feedback #8(1.0) -> (w3013:dbl)
        n1545 = Compound Arithmetic op=OR("Reset FFT", w3028, w3026) -> (w3011:bool)
        n1546 = Select(t=1.0, s=w3011, f=w3013) -> (s? t:f=w3015:dbl)
        n1547 = Greater?(x=w3015, y="# Spectra to Ave.") -> (0:w3034:bool)
        n1548 = Increment(x=w3015) -> (x+1=w3014:dbl)
        n1549 = feedback-in #8(w3014) -> ()
        n1550 = local read "DMA Update Period (s)"() -> (w3009:dbl)
        n1551 = Multiply(x="# Spectra to Ave.", y=w3009) -> (x*y=→"Ave. Time (s)":dbl)
        n1552 = Build Array(cluster{"f0":dbl, "df":dbl, "magnitude":dbl[]} {"f0"=0.0, "df"=0.0, "magnitude"=[]} ("PSD")) -> (w3018:cluster{"f0":dbl, "df":dbl, "magnitude":dbl[]}[])
        n1553 = Build Array(w3018, w3018, w3018, w3018) -> (w3020:T46)
        n1554 = feedback #9(w3020) -> (w3025:T46)
        n1555 = for {
          N: 4 -> [_]
          tunnel: w3029 -> [w3058] mode=indexing
          tunnel: w3036 -> [w3059]
          tunnel: w3035 -> [w3061]
          tunnel: w3011 -> [w3054]
          tunnel: w3034 -> [w3053]
          tunnel: "# Spectra to Ave." -> [w3052]
          tunnel: [w3051] -> w3024 mode=indexing
          tunnel: w3025 -> [w3056] mode=indexing
          tunnel: [w3055] -> w3012 mode=indexing
          tunnel: w3015 -> [w3050]
          n1556 = Less?(x=w3058, y=w3061) -> (x < y?=w3060:bool)
          n1557 = Index Array(array=w3059, index=w3058) -> (element=w3057:waveform(dbl))
          n1558 = case shown="True" w3060 {
            tunnel: w3057 -> [_ w3078]
            tunnel: w3056 -> [w3063 w3076]
            tunnel: [w3063 w3064] -> w3055
            tunnel: w3054 -> [_ w3075]
            tunnel: w3053 -> [_ w3068]
            tunnel: w3052 -> [_ w3067]
            tunnel: [cluster{"f0":dbl, "df":dbl, "magnitude":dbl[]} {"f0"=0.0, "df"=0.0, "magnitude"=[]} ("PSD") w3069] -> w3051
            tunnel: w3050 -> [_ w3066]
            frame False {
            }
            frame True {
              n1559 = call <vilib>:"Std Deviation and Variance.vi"("X"=w3078) -> ("mean"=w3079:dbl)  [unwired: 1 in, 2 out]
              n1560 = Subtract(x=w3078, y=w3079) -> (x-y=w3077:waveform(dbl))
              n1561 = xnode "Spectral Measurements"("Signals"=w3077) -> ("PSD"=w3071:cluster{"f0":dbl, "df":dbl, "magnitude":dbl[]})  [unwired: 1 in, 1 out]
              n1562 = case shown="False" w3075 {
                tunnel: w3076 -> [w3088 _]
                tunnel: [w3084 w3093] -> w3064
                tunnel: w3071 -> [w3087 w3094]
                tunnel: w3068 -> [w3086 _]
                frame False {
                  n1563 = Build Array (concatenate)(w3088, w3087) -> (w3085:cluster{"f0":dbl, "df":dbl, "magnitude":dbl[]}[])
                  n1564 = case shown="True" w3086 {
                    tunnel: w3085 -> [w3089 w3092]
                    tunnel: [w3089 w3090] -> w3084
                    frame False {
                    }
                    frame True {
                      n1565 = Delete From Array(array=w3092, index=0) -> (array with subset deleted=w3090:cluster{"f0":dbl, "df":dbl, "magnitude":dbl[]}[])  [unwired: 1 in, 1 out]
                    }
                  }
                }
                frame True {
                  n1566 = Build Array(w3094) -> (w3093:cluster{"f0":dbl, "df":dbl, "magnitude":dbl[]}[])
                }
              }
              n1567 = for {
                tunnel: w3064 -> [w3083] mode=indexing
                tunnel: [w3082] -> w3074 mode=indexing
                workers-P: _ -> [_]
                n1568 = Unbundle By Name(w3083) -> ("magnitude"=w3082:dbl[])
              }
              n1569 = Transpose 2D Array(2D array=w3074) -> (transposed array=w3073:dbl[][])
              n1570 = for {
                tunnel: w3073 -> [w3081] mode=indexing
                tunnel: [w3080] -> w3072 mode=indexing
                workers-P: _ -> [_]
                n1571 = Add Array Elements(numeric array=w3081) -> (sum=w3080:dbl)
              }
              n1572 = Select(t=w3067, s=w3068, f=w3066) -> (s? t:f=w3065:dbl)
              n1573 = Divide(x=w3072, y=w3065) -> (x/y=w3070:dbl[])
              n1574 = Bundle By Name(cluster=w3071, "magnitude"=w3070) -> (w3069:cluster{"f0":dbl, "df":dbl, "magnitude":dbl[]})
            }
          }
        }
        n1575 = case shown="True" w3011 {
          tunnel: w3012 -> [w3043 w3049]
          tunnel: [w3043 w3044] -> w3010
          frame False {
          }
          frame True {
            n1576 = Array Subset(array=w3049, index (row)=0 ("index"), length (row)=4 ("length"), index (col)=0 ("index"), length (col)=1 ("length")) -> (w3044:T46)
          }
        }
        n1577 = feedback-in #9(w3010) -> ()
        n1578 = Split 1D Array(array=w3024, index=2) -> (first subarray=→"FFT 1":cluster{"f0":dbl, "df":dbl, "magnitude":dbl[]}[], second subarray=→"FFT 2":cluster{"f0":dbl, "df":dbl, "magnitude":dbl[]}[])
      }
    }
    n1579 = Index Array(array=w1999, index=1) -> (element=w2007:waveform(dbl))
    n1580 = case "For displaying the high resolution display (no downsampling)" shown="True" w2072 {
      tunnel: w2026 -> [_ w2259]
      frame False {
      }
      frame True {
        n1581 = Index Array(array=w2259, index="High Res. Display") -> (element=w2260:waveform(dbl))
        n1582 = call <vilib>:"Std Deviation and Variance.vi"("X"=w2260) -> ("mean"=w2267:dbl, "standard deviation"=w2272:dbl)  [unwired: 1 in, 1 out]
        "Mean Intensity" <- w2267
        "Sigma" <- w2272
        n1583 = Subtract(x=w2260, y=w2267) -> (x-y=w2266:waveform(dbl))
        n1584 = Select(t=w2266, s="Subtract mean", f=w2260) -> (s? t:f=→"1 Channel":waveform(dbl))
        n1585 = Divide(x=w2272, y=w2267) -> (x/y=→"Sigma/Mean":dbl)
        n1586 = feedback #10(1) -> (w2261:i32)
        n1587 = Greater Or Equal?(x=w2261, y="Slow mean N ave.") -> (x >= y?=w2274:bool)
        n1588 = Increment(x=w2261) -> (x+1=w2276:i32)
        n1589 = Select(t=1, s=w2274, f=w2276) -> (s? t:f=w2263:i32)
        n1590 = feedback-in #10(w2263) -> ()
        n1591 = feedback #11() -> (w2264:waveform(dbl))  [unwired: 1 out]
        n1592 = case shown="Default" w2261 {
          tunnel: [w2279 w2282] -> w2265
          tunnel: w2264 -> [w2281 _]
          tunnel: w2260 -> [w2280 w2282]
          frame Default {
            n1593 = call-poly <vilib>:"Append Waveforms.vi"("waveform B"=w2280, "waveform A"=w2281) -> ("waveform out"=w2279:waveform(dbl))  [unwired: 1 in, 8 out]
          }
          frame 1 {
          }
        }
        n1594 = feedback-in #11(w2265) -> ()
        n1595 = case shown="True" w2274 {
          tunnel: w2265 -> [_ w2278]
          frame False {
          }
          frame True {
            n1596 = call-poly <vilib>:"Mean.vi"("X"=w2278) -> ("mean"=→"Slow mean":dbl)  [unwired: 1 out]
          }
        }
      }
    }
    n1597 = case "For plotting results of scanning MCL" shown="True" w2149 {
      tunnel: w2148 -> [_ w2399]
      tunnel: w2065 -> [_ w2495]
      tunnel: w2157 -> [_ _]
      tunnel: w2026 -> [_ w2469]
      tunnel: w2001 -> [_ w2400]
      tunnel: w2000 -> [_ w2373]
      frame False {
      }
      frame True {
        w2380 = u32 0 items=["Horizontal", "Vertical", "Central", "1st Diagonal", "2nd Diagonal"] ("Type of Symmetry")
        w2408 = u32 0 items=["Horizontal", "Vertical", "Central", "1st Diagonal", "2nd Diagonal"] ("Type of Symmetry")
        w2411 = u32 0 items=["Horizontal", "Vertical", "Central", "1st Diagonal", "2nd Diagonal"] ("Type of Symmetry")
        w2440 = u32 0 items=["Horizontal", "Vertical", "Central", "1st Diagonal", "2nd Diagonal"] ("Type of Symmetry")
        n1598 = Index Array(array=w2469, index=10) -> (element=w2475:waveform(dbl))
        n1599 = Index Array(array=w2469, index=11) -> (element=w2472:waveform(dbl))
        n1600 = local read "Cycles/step (MCL)"() -> (w2425:u64)
        n1601 = Index Array(array=w2469, index="Channel") -> (element=w2471:waveform(dbl))
        n1602 = Unbundle(w2373) -> ("New Image"=w2372:T2, "New Image"=w2371:T2, "New Image"=w2370:T2, "New Image"=w2369:T2)
        n1603 = Unbundle By Name(w2475) -> ("Y"=w2427:dbl[])
        n1604 = Unbundle By Name(w2472) -> ("Y"=w2429:dbl[])
        n1605 = Unbundle By Name(w2471) -> ("Y"=w2434:dbl[])
        n1606 = call "downsample 1D array - double.vi"("Ave N"=w2425, "Array In"=w2427) -> ("Array Out"=w2426:dbl[])  [unwired: 1 out]
        n1607 = call "downsample 1D array - double.vi"("Ave N"=w2425, "Array In"=w2429) -> ("Array Out"=w2428:dbl[])  [unwired: 1 out]
        n1608 = call "downsample 1D array - double.vi"("Ave N"=w2425, "Array In"=w2434) -> ("Array Out"=w2433:dbl[])  [unwired: 1 out]
        n1609 = feedback #12(w2495) -> (w2496:dbl[])
        n1610 = Build Array (concatenate)(w2496, w2495) -> (w2477:dbl[])
        n1611 = feedback #13(w2400) -> (w2402:dbl[])
        n1612 = Build Array (concatenate)(w2402, w2400) -> (w2401:dbl[])
        n1613 = local read "Scan steps (MCL)"() -> (w2382:u64)
        n1614 = Select(t=w2495, s=w2399, f=w2477) -> (s? t:f=w2481:dbl[])
        n1615 = feedback-in #12(w2481) -> ()
        n1616 = Select(t=w2400, s=w2399, f=w2401) -> (s? t:f=w2383:dbl[])
        n1617 = feedback-in #13(w2383) -> ()
        n1618 = local read "Scan lines (y)"() -> (w2368:u64)
        n1619 = local read "N APD Samp/step"() -> (w2384:dbl)
        n1620 = feedback #14(w2426) -> (w2483:dbl[])
        n1621 = Build Array (concatenate)(w2483, w2426) -> (w2474:dbl[])
        n1622 = feedback #15(w2433) -> (w2493:dbl[])
        n1623 = Build Array (concatenate)(w2493, w2433) -> (w2492:dbl[])
        n1624 = feedback #16(w2428) -> (w2485:dbl[])
        n1625 = Build Array (concatenate)(w2485, w2428) -> (w2486:dbl[])
        n1626 = Select(t=w2426, s=w2399, f=w2474) -> (s? t:f=w2430:dbl[])
        n1627 = feedback-in #14(w2430) -> ()
        n1628 = Select(t=w2433, s=w2399, f=w2492) -> (s? t:f=w2432:dbl[])
        n1629 = feedback-in #15(w2432) -> ()
        n1630 = Select(t=w2428, s=w2399, f=w2486) -> (s? t:f=w2431:dbl[])
        n1631 = feedback-in #16(w2431) -> ()
        n1632 = Multiply(x=w2382, y=u64 2) -> (x*y=w2367:u64)
        n1633 = call "integrate 1D array interval - double.vi"("Ave N"=w2384, "Array In"=w2383) -> ("Array Out"=w2395:dbl[])  [unwired: 1 out]
        n1634 = call "integrate 1D array interval - double.vi"("Ave N"=w2384, "Array In"=w2481) -> ("Array Out"=w2480:dbl[])  [unwired: 1 out]
        n1635 = Array Size(array=w2395) -> (size(s)=w2396:i32)
        n1636 = Array Size(array=w2480) -> (size(s)=w2482:i32)
        n1637 = Multiply(x=w2368, y=w2367) -> (x*y=w2398:u64)
        n1638 = Multiply(x=w2368, y=w2367) -> (x*y=w2490:u64)
        n1639 = call-poly <vilib>:"Mean.vi"("X"=w2430) -> ("mean"=w2414:dbl)  [unwired: 1 out]
        n1640 = Subtract(x=w2398, y=w2396) -> (x-y=w2389:u64)
        n1641 = call-poly <vilib>:"Mean.vi"("X"=w2432) -> ("mean"=w2419:dbl)  [unwired: 1 out]
        n1642 = call-poly <vilib>:"Mean.vi"("X"=w2431) -> ("mean"=w2417:dbl)  [unwired: 1 out]
        n1643 = call-poly <vilib>:"Mean.vi"("X"=w2395) -> ("mean"=w2386:dbl)  [unwired: 1 out]
        n1644 = Subtract(x=w2490, y=w2482) -> (x-y=w2424:u64)
        n1645 = call-poly <vilib>:"Mean.vi"("X"=w2480) -> ("mean"=w2421:dbl)  [unwired: 1 out]
        n1646 = Initialize Array(1.0 ("element"), w2389) -> (w2385:dbl[])
        n1647 = Initialize Array(1.0 ("element"), w2424) -> (w2415:dbl[])
        n1648 = Multiply(x=w2385, y=w2386) -> (x*y=w2387:dbl[])
        n1649 = Multiply(x=w2415, y=w2417) -> (x*y=w2418:dbl[])
        n1650 = Multiply(x=w2415, y=w2419) -> (x*y=w2420:dbl[])
        n1651 = Multiply(x=w2415, y=w2414) -> (x*y=w2416:dbl[])
        n1652 = Multiply(x=w2415, y=w2421) -> (x*y=w2422:dbl[])
        n1653 = Build Array (concatenate)(w2430, w2416) -> (w2484:dbl[])
        n1654 = Build Array (concatenate)(w2432, w2420) -> (w2488:dbl[])
        n1655 = Build Array (concatenate)(w2431, w2418) -> (w2487:dbl[])
        n1656 = Build Array (concatenate)(w2395, w2387) -> (w2397:dbl[])
        n1657 = Build Array (concatenate)(w2480, w2422) -> (w2489:dbl[])
        n1658 = Reshape Array(w2484, w2368, w2367) -> (w2450:dbl[][])
        n1659 = Reshape Array(w2397, w2368, w2367) -> (w2393:dbl[][])
        n1660 = Reshape Array(w2488, w2368, w2367) -> (w2442:dbl[][])
        n1661 = Reshape Array(w2487, w2368, w2367) -> (w2457:dbl[][])
        n1662 = Reshape Array(w2489, w2368, w2367) -> (w2467:dbl[][])
        n1663 = Array Subset(array=w2457, index (col)=0 ("index"), length (col)=w2382) -> (w2462:dbl[][])  [unwired: 2 in]
        n1664 = Array Subset(array=w2457, index (col)=w2382) -> (w2460:dbl[][])  [unwired: 3 in]
        n1665 = Array Subset(array=w2442, index (col)=0 ("index"), length (col)=w2382) -> (w2448:dbl[][])  [unwired: 2 in]
        n1666 = Array Subset(array=w2442, index (col)=w2382) -> (w2446:dbl[][])  [unwired: 3 in]
        n1667 = Array Subset(array=w2393, index (col)=0 ("index"), length (col)=w2382) -> (w2392:dbl[][])  [unwired: 2 in]
        n1668 = Array Subset(array=w2393, index (col)=w2382) -> (w2390:dbl[][])  [unwired: 3 in]
        n1669 = Array Subset(array=w2467, index (col)=0 ("index"), length (col)=w2382) -> (w2466:dbl[][])  [unwired: 2 in]
        n1670 = Array Subset(array=w2467, index (col)=w2382) -> (w2464:dbl[][])  [unwired: 3 in]
        n1671 = Array Subset(array=w2450, index (col)=0 ("index"), length (col)=w2382) -> (w2455:dbl[][])  [unwired: 2 in]
        n1672 = Array Subset(array=w2450, index (col)=w2382) -> (w2453:dbl[][])  [unwired: 3 in]
        n1673 = for {
          tunnel: w2462 -> [w2504] mode=indexing
          tunnel: [w2503] -> w2461 mode=indexing
          workers-P: _ -> [_]
          n1674 = Reverse 1D Array(array=w2504) -> (reversed array=w2503:dbl[])
        }
        n1675 = for {
          tunnel: w2448 -> [w2500] mode=indexing
          tunnel: [w2499] -> w2447 mode=indexing
          workers-P: _ -> [_]
          n1676 = Reverse 1D Array(array=w2500) -> (reversed array=w2499:dbl[])
        }
        n1677 = for {
          tunnel: w2392 -> [w2498] mode=indexing
          tunnel: [w2497] -> w2391 mode=indexing
          workers-P: _ -> [_]
          n1678 = Reverse 1D Array(array=w2498) -> (reversed array=w2497:dbl[])
        }
        n1679 = for {
          tunnel: w2466 -> [w2506] mode=indexing
          tunnel: [w2505] -> w2465 mode=indexing
          workers-P: _ -> [_]
          n1680 = Reverse 1D Array(array=w2506) -> (reversed array=w2505:dbl[])
        }
        n1681 = for {
          tunnel: w2455 -> [w2502] mode=indexing
          tunnel: [w2501] -> w2454 mode=indexing
          workers-P: _ -> [_]
          n1682 = Reverse 1D Array(array=w2502) -> (reversed array=w2501:dbl[])
        }
        n1683 = Index Array(array=w2467, index (row)=0) -> (element=→"Waveform Graph":dbl[])  [unwired: 1 in]
        n1684 = Add(x=w2461, y=w2460) -> (x+y=w2459:dbl[][])
        n1685 = Add(x=w2447, y=w2446) -> (x+y=w2445:dbl[][])
        n1686 = Add(x=w2391, y=w2390) -> (x+y=w2375:dbl[][])
        n1687 = Add(x=w2465, y=w2464) -> (x+y=w2439:dbl[][])
        n1688 = Add(x=w2454, y=w2453) -> (x+y=w2452:dbl[][])
        n1689 = Divide(x=w2445, y=2) -> (x/y=w2443:dbl[][])
        n1690 = Divide(x=w2459, y=2) -> (x/y=w2404:dbl[][])
        n1691 = Divide(x=w2452, y=2) -> (x/y=w2406:dbl[][])
        n1692 = To Single Precision Float(number=w2439) -> (single precision float=w2438:sgl[][])
        n1693 = Transpose 2D Array(2D array=w2443) -> (transposed array=→"Data map":dbl[][])
        n1694 = To Single Precision Float(number=w2375) -> (single precision float=w2379:sgl[][])
        n1695 = To Single Precision Float(number=w2404) -> (single precision float=w2410:sgl[][])
        n1696 = To Single Precision Float(number=w2406) -> (single precision float=w2407:sgl[][])
        n1697 = call "IMAQ ArrayToImage"("Image Pixels (Float)"=w2438, "Image"=w2372) -> ("Image Out"=w2441:T2)  [unwired: 8 in, 1 out]
        n1698 = call "IMAQ ArrayToImage"("Image Pixels (Float)"=w2379, "Image"=w2371) -> ("Image Out"=w2381:T2)  [unwired: 8 in, 1 out]
        n1699 = call "IMAQ ArrayToImage"("Image Pixels (Float)"=w2410, "Image"=w2370) -> ("Image Out"=w2412:T2)  [unwired: 8 in, 1 out]
        n1700 = call "IMAQ ArrayToImage"("Image Pixels (Float)"=w2407, "Image"=w2369) -> ("Image Out"=w2409:T2)  [unwired: 8 in, 1 out]
        n1701 = call "IMAQ Symmetry"("Type of Symmetry"=w2440, "Image Src"=w2441) -> ("Image Dst Out"=w2436:T2)  [unwired: 3 in, 1 out]
        n1702 = call "IMAQ Symmetry"("Type of Symmetry"=w2380, "Image Src"=w2381) -> ("Image Dst Out"=w2377:T2)  [unwired: 3 in, 1 out]
        n1703 = call "IMAQ Symmetry"("Type of Symmetry"=w2411, "Image Src"=w2412) -> ("Image Dst Out"=→"Detection Laser X":T2)  [unwired: 3 in, 1 out]
        n1704 = call "IMAQ Symmetry"("Type of Symmetry"=w2408, "Image Src"=w2409) -> ("Image Dst Out"=→"Detection Laser Y":T2)  [unwired: 3 in, 1 out]
        n1705 = call "IMAQ Set Simple Calibration"("Calibration Axis Info"=T36 {"Origin Pixel"={"X"=0.0, "Y"=0.0}, "Angle Relative to Horizontal (deg)"=0.0, "Axis Reference"=0}, "Grid Descriptor"=T37 {"X Step"=0.3, "Y Step"=0.3, "Unit"=enum."Undefined"}, "Image"=w2436) -> ("Calibrated Image"=→"APD 1":T2)  [unwired: 7 in, 1 out]
        n1706 = call "IMAQ Set Simple Calibration"("Calibration Axis Info"=T36 {"Origin Pixel"={"X"=0.0, "Y"=0.0}, "Angle Relative to Horizontal (deg)"=0.0, "Axis Reference"=0}, "Grid Descriptor"=T37 {"X Step"=0.3, "Y Step"=0.3, "Unit"=enum."Undefined"}, "Image"=w2377) -> ("Calibrated Image"=→"APD 2":T2)  [unwired: 7 in, 1 out]
      }
    }
    n1707 = Subtract(x=w2007, y="APD 2 Offset") -> (x-y=w2004:waveform(dbl))
    n1708 = Subtract(x=w2009, y="APD 1 Offset") -> (x-y=w2005:waveform(dbl))
    n1709 = Index Array(array=w2024, index=3) -> (element=w2093:waveform(dbl))
    n1710 = Index Array(array=w2024, index=6) -> (element=w2090:waveform(dbl))
    n1711 = Build Array(w2005, w2004) -> (→"APD Chart":waveform(dbl)[])
    n1712 = Array Size(array=w2082) -> (size(s)=w2137:i32)
    n1713 = call <vilib>:"Std Deviation and Variance.vi"("X"=w2017) -> ("standard deviation"=w2016:dbl)  [unwired: 1 in, 2 out]
    n1714 = Add Array Elements(numeric array=w2017) -> (sum=w2019:u32)
    n1715 = Add Array Elements(numeric array=w2082) -> (sum=w2147:u32)
    n1716 = call <vilib>:"Std Deviation and Variance.vi"("X"=w2082) -> ("standard deviation"=w2081:dbl)  [unwired: 1 in, 2 out]
    n1717 = Divide(x="T1 offset_x (mV)", y=1000.0) -> (x/y=w2094:dbl)
    n1718 = Divide(x=w2016, y=w2015) -> (x/y=w2012:dbl)
    "Rate sigma (Hz) 2" <- w2012
    n1719 = Multiply(x=w2015, y=w2137) -> (x*y=w2018:dbl)
    "Int. Time (s)" <- w2018
    n1720 = Divide(x=w2019, y=w2018) -> (x/y=w2013:dbl)
    "APD 2 Rate (Hz)" <- w2013
    n1721 = Divide(x=w2147, y=w2018) -> (x/y=w2079:dbl)
    "APD 1 Rate (Hz)" <- w2079
    n1722 = Divide(x=w2081, y=w2015) -> (x/y=w2080:dbl)
    "Rate sigma (Hz)" <- w2080
    n1723 = Divide(x=w2012, y=w2013) -> (x/y=→"Sigma/Mean 2":dbl)
    n1724 = Divide(x=w2080, y=w2079) -> (x/y=→"Sigma/Mean":dbl)
    n1725 = Divide(x="T2 offset_x (mV)", y=1000.0) -> (x/y=w2092:dbl)
    n1726 = case shown="1" "Calibration" {
      tunnel: "T1 alpha_x (nm/V)" -> [_ w2335 w2356]
      tunnel: "T1 kappa_x (pN/nm)" -> [_ _ w2346]
      tunnel: "T2 alpha_x (nm/V)" -> [_ w2334 w2354]
      tunnel: "T2 kappa_x (pN/nm)" -> [_ _ w2347]
      tunnel: w2093 -> [w2317 w2332 w2352]
      tunnel: w2090 -> [w2316 w2330 w2350]
      tunnel: [w2317 w2329 w2349] -> w2123
      tunnel: [w2316 w2328 w2348] -> w2122
      tunnel: ["T1 X (V)" ("Label.Text") "T1 X (nm)" ("Label.Text") "T1 X (pN)" ("Label.Text")] -> w2111
      tunnel: ["T2 X (V)" ("Label.Text") "T2 X (nm)" ("Label.Text") "T2 X (pN)" ("Label.Text")] -> w2110
      tunnel: ["Position (V)" ("Label.Text") "Position (nm)" ("Label.Text") "Force (pN)" ("Label.Text")] -> w2112
      tunnel: w2092 -> [_ w2320 w2339]
      tunnel: w2094 -> [_ w2323 w2341]
      tunnel: ["Mean (V)" ("Label.Text") "Mean (nm)" ("Label.Text") "Mean (pN)" ("Label.Text")] -> w2107
      tunnel: ["Difference (V)" ("Label.Text") "Difference (nm)" ("Label.Text") "Difference (pN)" ("Label.Text")] -> w2032
      frame 0, Default {
      }
      frame 1 {
        # "position"
        n1727 = Unbundle By Name(w2332) -> ("Y"=w2336:dbl[])
        n1728 = Unbundle By Name(w2330) -> ("Y"=w2321:dbl[])
        n1729 = Subtract(x=w2336, y=w2323) -> (x-y=w2324:dbl[])
        n1730 = Subtract(x=w2321, y=w2320) -> (x-y=w2322:dbl[])
        n1731 = Multiply(x=w2322, y=w2334) -> (x*y=w2331:dbl[])
        n1732 = Multiply(x=w2335, y=w2324) -> (x*y=w2333:dbl[])
        n1733 = Bundle By Name(cluster=w2330, "Y"=w2331) -> (w2328:waveform(dbl))
        n1734 = Bundle By Name(cluster=w2332, "Y"=w2333) -> (w2329:waveform(dbl))
      }
      frame 2 {
        # "force"
        n1735 = Unbundle By Name(w2352) -> ("Y"=w2357:dbl[])
        n1736 = Unbundle By Name(w2350) -> ("Y"=w2355:dbl[])
        n1737 = Subtract(x=w2355, y=w2339) -> (x-y=w2340:dbl[])
        n1738 = Subtract(x=w2357, y=w2341) -> (x-y=w2342:dbl[])
        n1739 = Compound Arithmetic op=MULTIPLY(w2340, w2354, w2347) -> (w2351:dbl[])
        n1740 = Compound Arithmetic op=MULTIPLY(w2346, w2356, w2342) -> (w2353:dbl[])
        n1741 = Bundle By Name(cluster=w2350, "Y"=w2351) -> (w2348:waveform(dbl))
        n1742 = Bundle By Name(cluster=w2352, "Y"=w2353) -> (w2349:waveform(dbl))
      }
    }
    n1743 = feedback-in #17("Calibration") -> ()
    n1744 = feedback #17(u16 1 ("Calibration")) -> (w2114:u16)
    n1745 = Not Equal?(x=w2114, y="Calibration") -> (x != y?=w2070:bool)
    n1746 = Unbundle By Name(w2093) -> ("Y"=w2096:dbl[])
    n1747 = Unbundle By Name(w2090) -> ("Y"=w2099:dbl[])
    n1748 = Subtract(x=w2096, y=w2094) -> (x-y=w2097:dbl[])
    n1749 = Subtract(x=w2099, y=w2092) -> (x-y=w2098:dbl[])
    n1750 = disable-structure shown="Enabled" {
      disable-tunnel: [-1.0 ("y") 1.0] -> w2100
      frame Disabled {
      }
      frame Enabled {
      }
    }
    n1751 = Multiply(x=w2098, y="T2 alpha_x (nm/V)") -> (x*y=w2089:dbl[])
    n1752 = Multiply(x="T1 alpha_x (nm/V)", y=w2097) -> (x*y=w2088:dbl[])
    n1753 = Multiply(x=w2122, y=w2100) -> (x*y=w2101:waveform(dbl))
    n1754 = case shown="True" "Read Lateness and Rel Phase" {
      tunnel: w1924 -> [w2283 w2305]
      tunnel: w1923 -> [w2284 w2304]
      tunnel: [w2283 w2303] -> w2085
      tunnel: [w2284 w2302] -> w2084
      frame False {
      }
      frame True {
        n1755 = xnode "Read/Write Control"("FPGA VI Reference In"=w2305, "error in"=w2304) -> ("FPGA VI Reference Out"=w2303:T19, "error out"=w2302:errorcluster, "GI Relative phase"=→"GI relative phase":i16, "Relative phase"=→"Relative phase (AI1)":i16, "AI Late Counter"=→"Late Counter (AI1)":u16, "GI Late Counter"=→"GI Late Counter":u16, "MCL Late Counter"=→"MCL Late Counter":u16, "MCL Relative Phase"=→"Relative Phase (MCL)":i16, "APD Acq Relative Phase"=→"APD Acq Relative Phase":i16, "APD 1 Gate Relative Phase"=→"APD 1 Gate Relative Phase":i16, "APD 2 Gate Relative Phase"=→"APD 2 Gate Relative Phase":i16, "APD Acq Late Counter"=→"APD Acq Late Counter":u16, "APD 1 Gate Late Counter"=→"APD 1 Gate Late Counter":u16, "APD 2 Gate Late Counter"=→"APD 2 Gate Late Counter":u16, "Green FB Relative Phase"=→"Relative phase (Green FB)":i16, "GI Relative phase 2"=→"GI relative phase 2":i16, "GI Late Counter 2"=→"GI Late Counter 2":u16, "Trap Pos FIFO Timeout"=→"Trap Pos FIFO Timeout":u16, "Trap AI FIFO Timeout"=→"Trap AI FIFO Timeout":u16)
      }
    }
    n1756 = Subtract(x=w2089, y=w2088) -> (x-y=w2087:dbl[])
    n1757 = Unbundle By Name(w2122) -> ("Y"=w2057:dbl[])
    n1758 = Unbundle By Name(w2123) -> ("Y"=w2058:dbl[])
    n1759 = Build Array(w2123, w2101) -> (→"Force":waveform(dbl)[])
    n1760 = Subtract(x=w2087, y="Offset (nm)") -> (x-y=w2055:dbl[])
    n1761 = call-poly <vilib>:"Mean.vi"("X"=w2057) -> ("mean"=w2036:dbl)  [unwired: 1 out]
    "T2 X" <- w2036
    n1762 = Absolute Value(x=w2058) -> (abs(x)=w2059:dbl[])
    n1763 = Absolute Value(x=w2057) -> (abs(x)=w2060:dbl[])
    n1764 = call-poly <vilib>:"Mean.vi"("X"=w2058) -> ("mean"=w2037:dbl)  [unwired: 1 out]
    "T1 X" <- w2037
    n1765 = Add(x=w2059, y=w2060) -> (x+y=w2061:dbl[])
    n1766 = Bundle By Name(cluster=w2093, "Y"=w2055) -> (w2023:waveform(dbl))
    "Bead Separation" <- w2023
    n1767 = Divide(x=w2061, y=2.0) -> (x/y=→"Vec Mean of T1 T2":dbl[])
    n1768 = case shown="True" w2070 {
      tunnel: w2112 -> [_ w2310]
      tunnel: w2111 -> [_ w2309]
      tunnel: w2110 -> [_ w2308]
      tunnel: w2107 -> [_ w2307]
      tunnel: w2032 -> [_ w2306]
      frame False {
      }
      frame True {
        n1769 = property on="Force" class="WFChart (strict)"("YScale.NameLbl.Text"=w2310) -> ()  [unwired: 2 in, 2 out]
        n1770 = property on="T2 X" class="DigNum (strict)"("Caption.Text"=w2308) -> ()  [unwired: 2 in, 2 out]
        n1771 = property on="T1 X" class="DigNum (strict)"("Caption.Text"=w2309) -> ()  [unwired: 2 in, 2 out]
        n1772 = property on="Mean" class="DigNum (strict)"("Caption.Text"=w2307) -> ()  [unwired: 2 in, 2 out]
        n1773 = property on="Difference" class="DigNum (strict)"("Caption.Text"=w2306) -> ()  [unwired: 2 in, 2 out]
      }
    }
    n1774 = local read "Tether"() -> (w2064:bool)
    n1775 = Absolute Value(x=w2037) -> (abs(x)=w2034:dbl)
    n1776 = Absolute Value(x=w2036) -> (abs(x)=w2033:dbl)
    n1777 = Add(x=w2034, y=w2033) -> (x+y=w2109:dbl)
    n1778 = Subtract(x=w2034, y=w2033) -> (x-y=→"Difference":dbl)
    n1779 = feedback #18(w2055) -> (w2054:dbl[])
    n1780 = Divide(x=w2109, y=2.0) -> (x/y=w2063:dbl)
    "Mean" <- w2063
    n1781 = case shown="True" w2064 {
      tunnel: w2063 -> [_ w2242]
      frame False {
      }
      frame True {
        n1782 = Greater?(x="Lost Tether Alarm Threshold (pN)", y=w2242) -> (0:w2240:bool)
        n1783 = case shown="True" w2240 {
          frame False {
          }
          frame True {
            n1784 = flat-sequence {
              frame #0 {
                # "stop only if saving"
                n1785 = local read "Saving..."() -> (w2255:bool)
                n1786 = And(x=w2255, y="TA Cancel Save?") -> (x .and. y?=w2254:bool)
                n1787 = local write "Stop Saving"(w2254) -> ()
              }
              frame #1 {
                n1788 = case shown="True" "TA Green Off?" {
                  frame False {
                  }
                  frame True {
                    w2258 = FALSE ("Fl. Triggered...")
                    n1789 = local write "Fl. Triggered..."(w2258) -> ()
                    n1790 = property on="Green Laser ON/Interlacing" class="Bool (strict)"("Val(Sgnl)"=w2258) -> ()  [unwired: 2 in, 2 out]
                  }
                }
              }
            }
            n1791 = local read "Time tether formed"() -> (w2249:timestamp)
            n1792 = Get Date/Time In Seconds() -> (seconds since 1Jan1904=w2250:timestamp)
            n1793 = Subtract(x=w2250, y=w2249) -> (x-y=w2248:dbl)
            n1794 = Number To Decimal String(number=w2248) -> (decimal integer string=w2245:string)  [unwired: 1 out]
            n1795 = local read "Messages"() -> (w2252:string)
            n1796 = call <vilib>:"Beep.vi"() -> ()  [unwired: 3 in, 9 out]
            n1797 = Concatenate Strings("Lost tether (" ("Message to add"), w2245, " s)." ("string")) -> (w2247:string)
            n1798 = local write "Tether"(FALSE ("Tether")) -> ()
            n1799 = call "Update messages.vi"("Message to add"=w2247, "Old message string"=w2252) -> ("New message string"=w2251:string)
            n1800 = local write "Messages"(w2251) -> ()
            n1801 = property on="Trap Pos. FB ON" class="Bool (strict)"("Val(Sgnl)"=FALSE ("Value (Signaling)")) -> ()  [unwired: 2 in, 2 out]
          }
        }
      }
    }
    n1802 = Build Array (concatenate)(w2055, w2054) -> (w2053:dbl[])
    n1803 = Split 1D Array(array=w2053, index=w1935) -> (first subarray=w2049:dbl[])  [unwired: 1 out]
    n1804 = feedback-in #18(w2049) -> ()
    n1805 = call-poly <vilib>:"Mean.vi"("X"=w2049) -> ("mean"=w2048:dbl)  [unwired: 1 out]
    "Bead Mean (nm)" <- w2048
    n1806 = Subtract(x=w2049, y=w2048) -> (x-y=w2047:dbl[])
    n1807 = Square(x=w2047) -> (x^2=w2046:dbl[])
    n1808 = call-poly <vilib>:"Mean.vi"("X"=w2046) -> ("mean"=w2045:dbl)  [unwired: 1 out]
    n1809 = Square Root(x=w2045) -> (sqrt(x)=w2044:dbl)
    n1810 = Multiply(x=10.0, y=w2044) -> (x*y=→"RMS (Ang)":dbl)
    n1811 = xnode "Read/Write Control"("FPGA VI Reference In"=w2085, "error in"=w2084) -> ("FPGA VI Reference Out"=w2203:T19, "error out"=w2197:errorcluster, "AI2 Y Sum Set 1"=w2193:i16, "AI2 Y Sum Set 2"=w2192:i16, "AI1 X Set 1"=w1969:fxp<+/-,16,1>, "AI1 X Set 2"=w1968:fxp<+/-,16,1>, "Trap Pos FB Int Signal"=→"Trap Pos FB Int Signal":fxp<+/-,24,9>, "Trap Pos FB Int-Norm Signal"=→"Trap Pos FB Int-Norm Signal":fxp<+/-,16,1>, "Trap Pos FB Action"=w1962:i64, "Scanning"=→"AOD Scanning":bool, "Scan I"=→"AOD Scan I":u64, "Scanning MCL"=w2195:bool, "Scan I (MCL)"=→"MCL Scan I":u64, "Green FB Signals"=w2132:T47)  [unwired: 1 out]
    "MCL Scanning" <- w2195
    "Trap Pos FB Action" <- w1962
    n1812 = local read "AI2 (V)"() -> (w2194:cluster{"Set 1":dbl, "Set 2":dbl})
    n1813 = Bundle By Name(cluster=w2194, "Set 1"=w2193, "Set 2"=w2192) -> (w2190:cluster{"Set 1":dbl, "Set 2":dbl})
    n1814 = Divide(x=w1962, y=327.67) -> (x/y=→"Action (%)":dbl)
    n1815 = local read "Trap X (AI1)"() -> (w1982:T10)
    n1816 = Divide(x=w2190, y=3276.7) -> (x/y=w2189:cluster{"Set 1":dbl, "Set 2":dbl})
    n1817 = local write "AI2 (V)"(w2189) -> ()
    n1818 = Bundle(cluster=w1982, "Trap 1"=w1969, "Trap 2"=w1968) -> (→"Trap X (AI1)":T10)
    n1819 = Divide(x=w2132, y=3276.7) -> (x/y=w2128:T48)
    n1820 = Unbundle By Name(w2128) -> ("Green FB Ch 0"=w2131:dbl, "Green FB Ch 1"=w2130:dbl, "Green FB Ch 2"=w2129:dbl)
    n1821 = Divide(x=w2131, y=w2129) -> (x/y=w2127:dbl)
    n1822 = Divide(x=w2130, y=w2129) -> (x/y=w2126:dbl)
    n1823 = flat-sequence "To save data" {
      tunnel: [w3132] -> w2214
      tunnel: [w3133] -> w2213
      tunnel: w2163 -> [w3126]
      tunnel: w2051 -> [w3130]
      tunnel: ["Save Calibration"] -> w2186
      tunnel: w2183 -> [w3129]
      tunnel: [w3122] -> w2182
      tunnel: [w3119] -> w2181
      tunnel: [w3116] -> w2180
      tunnel: w2162 -> [w3118]
      tunnel: w2068 -> [w3112]
      tunnel: [w3112] -> w2067
      tunnel: ["Start Saving"] -> w2025
      tunnel: [w3106] -> w1951
      tunnel: [w3105] -> w1950
      tunnel: w2214 -> [w3367]
      tunnel: w2213 -> [w3366]
      tunnel: w1952 -> [w3365]
      tunnel: w2186 -> [w3364]
      tunnel: w2182 -> [w3362]
      tunnel: w2181 -> [w3361]
      tunnel: w2180 -> [w3360]
      tunnel: w2038 -> [w3359]
      tunnel: w2077 -> [w3358]
      tunnel: w2067 -> [w3357]
      tunnel: w2025 -> [w3356]
      tunnel: w2023 -> [w3355]
      tunnel: w1999 -> [w3354]
      tunnel: w1951 -> [w3353]
      tunnel: w1950 -> [w3352]
      tunnel: w1949 -> [w3351]
      frame #0 {
        n1824 = Or(x="Save N Sets", y="Start Saving") -> (x .or. y?=w3113:bool)
        n1825 = To Double Precision Float(number=w3129) -> (double precision float=w3123:dbl)
        n1826 = Build Array(w3113, "Save Calibration", w3126, w3118) -> (w3128:bool[])
        n1827 = Compound Arithmetic op=OR("Save Calibration", w3126, w3113, w3118) -> (w3131:bool)
        n1828 = Boolean Array To Number(Boolean array=w3128) -> (number=w3125:u32)
        n1829 = feedback #19(FALSE ("Save APD Data\nwith Trap Data")) -> (w3107:bool)
        n1830 = feedback #20(refnum<k0> refnum) -> (w3134:refnum<file>)
        n1831 = feedback #21(refnum<k0> refnum) -> (w3109:refnum<file>)
        n1832 = feedback #22(FALSE ("Save APD Data\nwith Trap Data")) -> (w3117:bool)
        n1833 = feedback #23(refnum<k0> refnum) -> (w3120:refnum<file>)
        n1834 = feedback #24(0) -> (w3136:i32)
        n1835 = feedback #25() -> (w3124:u32)  [unwired: 1 out]
        n1836 = case shown="True" w3131 {
          tunnel: [w3143 1] -> w3132
          tunnel: w3136 -> [w3145 _]
          tunnel: [w3144 w3163] -> w3133
          tunnel: w3134 -> [w3144 _]
          tunnel: w3130 -> [_ w3183]
          tunnel: w3123 -> [_ w3181]
          tunnel: w3125 -> [_ w3184]
          tunnel: [w3142 w3162] -> w3122
          tunnel: w3124 -> [w3142 _]
          tunnel: [w3141 w3160] -> w3119
          tunnel: w3120 -> [w3141 _]
          tunnel: [w3140 w3159] -> w3116
          tunnel: w3117 -> [w3140 _]
          tunnel: "Start Saving" -> [_ w3157]
          tunnel: w3112 -> [_ w3156]
          tunnel: [w3139 w3147] -> w3105
          tunnel: w3109 -> [w3139 _]
          tunnel: [w3138 w3146] -> w3106
          tunnel: w3107 -> [w3138 _]
          frame False {
            n1837 = Increment(x=w3145) -> (x+1=w3143:i32)
          }
          frame True {
            w3153 = FALSE ("Start Saving")
            w3158 = 9.0  # File Version
            w3166 = FALSE ("prepend array or string size? (T)")
            w3164 = T29."big-endian, network order" ("byte order (0:big-endian, network order)")
            # "write file headers"
            n1838 = local read "BD 1 Frequency 1 (MHz)"() -> (w3180:dbl)
            n1839 = local read "BD 2 Frequency 1 (MHz)"() -> (w3179:dbl)
            n1840 = local read "BD 1 Frequency 2 (MHz)"() -> (w3178:dbl)
            n1841 = local read "BD 2 Frequency 2 (MHz)"() -> (w3177:dbl)
            n1842 = local read "BD 1 Frequency 3 (MHz)"() -> (w3176:dbl)
            n1843 = local read "BD 2 Frequency 3 (MHz)"() -> (w3175:dbl)
            n1844 = Array Size(array=w3156) -> (size(s)=w3155:i32)
            n1845 = To Double Precision Float(number=w3155) -> (double precision float=w3154:dbl)
            n1846 = local write "Save Calibration"(w3153) -> ()
            n1847 = local write "Start Saving"(w3153) -> ()
            n1848 = Build Array("Save APD Data\nwith Trap Data", "Save Trap Pos. Data") -> (w3150:bool[])
            n1849 = Boolean Array To Number(Boolean array=w3150) -> (number=w3149:u32)
            n1850 = Build Array(w3180, w3179, w3178, w3177, w3176, w3175) -> (w3174:dbl[])
            n1851 = case shown="4" w3184 {
              tunnel: w3183 -> [w3255 w3275 w3291 w3329]
              tunnel: w3154 -> [w3260 w3282 w3311 w3348]
              tunnel: w3181 -> [w3259 w3281 w3310 w3347]
              tunnel: [w3256 w3277 w3302 w3339] -> w3172
              tunnel: [w3247 "Cal sets to save" w3292 w3330] -> w3162
              tunnel: w3174 -> [w3257 w3278 w3304 w3341]
              tunnel: "Save APD Data\nwith Trap Data" -> [w3254 _ w3288 w3327]
              tunnel: [w3254 w3269 w3288 w3327] -> w3159
              tunnel: w3158 -> [w3250 w3270 w3286 w3325]
              tunnel: w3157 -> [w3249 _ _ _]
              tunnel: [w3240 w3269 w3285 w3315] -> w3146
              tunnel: "Save Trap Pos. Data" -> [w3240 _ w3285 w3315]
              tunnel: w3149 -> [w3239 _ w3284 w3314]
              frame 1, Default {
                # "timeseries"
                n1852 = case shown="True" "Profile" {
                  tunnel: [w3263 w3266] -> w3244
                  tunnel: [w3263 w3265] -> w3243
                  tunnel: [w3263 w3264] -> w3242
                  tunnel: [w3263 w3268] -> w3241
                  frame False {
                    w3263 = 0.0 ("f")
                  }
                  frame True {
                    n1853 = local read "Current Position"() -> (w3267:dbl[])
                    n1854 = local read "Y change (mm)"() -> (w3268:dbl)
                    n1855 = call "subVI_explode3array.vi"("Array"=w3267) -> ("x"=w3266:dbl, "y"=w3265:dbl, "z"=w3264:dbl)  [unwired: 12 in]
                  }
                }
                n1856 = local read "Save ave N"() -> (w3262:dbl)
                n1857 = Multiply(x=w3262, y=w3255) -> (x*y=w3261:dbl)
                n1858 = To Double Precision Float(number=w3239) -> (double precision float=w3253:dbl)
                n1859 = Build Array(w3250, w3255, w3261, w3260, w3259, 0.0 ("f")) -> (w3258:dbl[])
                n1860 = Build Array(w3253, w3244, w3243, w3242, w3241) -> (w3251:dbl[])
                n1861 = Select(t=u32 4000000000, s=w3249, f="N sets to save") -> (s? t:f=w3247:u32)
                n1862 = Build Array (concatenate)(w3258, w3257, w3251) -> (w3256:dbl[])
              }
              frame 2 {
                w3272 = 0.0 ("f")
                w3269 = FALSE ("Save APD Data\nwith Trap Data")
                # "calibration"
                n1863 = Boolean To (0,1)(Boolean=w3269) -> (0, 1=w3274:i16)
                n1864 = To Double Precision Float(number=w3274) -> (double precision float=w3273:dbl)
                n1865 = Build Array(w3273, w3272, w3272, w3272, w3272) -> (w3271:dbl[])
                n1866 = Build Array(w3270, w3275, w3275, w3282, w3281, 1.0 ("t")) -> (w3279:dbl[])
                n1867 = Build Array (concatenate)(w3279, w3278, w3271) -> (w3277:dbl[])
                "Calibrating Trap..." <- TRUE ("Calibrating...")
              }
              frame 4 {
                w3289 = 0.0 ("f")
                # "write file header for a trap \nraster scan"
                # "scan dir (x/y = 0/1)"
                # "cycles/step"
                # "n scans (f/b)"
                # "steps"
                # "freq. range"
                # "AOD raster scan"
                n1868 = local read "Number of F/B Scans (AOD)"() -> (w3296:u16)
                n1869 = local read "Cycles/step (AOD)"() -> (w3298:u64)
                n1870 = local read "Scan Range (MHz)"() -> (w3301:dbl)
                n1871 = local read "Scan steps (AOD)"() -> (w3300:u64)
                n1872 = local read "Scan BD"() -> (w3308:bool)
                n1873 = local read "Save ave N"() -> (w3313:dbl)
                n1874 = Boolean To (0,1)(Boolean=w3308) -> (0, 1=w3307:i16)
                n1875 = To Double Precision Float(number=w3296) -> (double precision float=w3295:dbl)
                n1876 = To Double Precision Float(number=w3300) -> (double precision float=w3299:dbl)
                n1877 = To Double Precision Float(number=w3298) -> (double precision float=w3297:dbl)
                n1878 = To Double Precision Float(number=w3307) -> (double precision float=w3306:dbl)
                n1879 = Multiply(x=w3313, y=w3291) -> (x*y=w3312:dbl)
                n1880 = To Double Precision Float(number=w3284) -> (double precision float=w3290:dbl)
                n1881 = Build Array(w3290, w3289, w3289, w3289, w3289) -> (w3287:dbl[])
                n1882 = local read "N sets should be saved"() -> (w3293:dbl)
                n1883 = Build Array(w3306, w3301, w3299, w3297, w3295) -> (w3303:dbl[])
                n1884 = Build Array(w3286, w3291, w3312, w3311, w3310, 2.0 ("t")) -> (w3305:dbl[])
                n1885 = Round Toward +Infinity(x=w3293) -> (ceil(x): smallest int >= x=w3294:dbl)
                n1886 = Build Array (concatenate)(w3305, w3304, w3287, w3303) -> (w3302:dbl[])
                n1887 = To Unsigned Long Integer(number=w3294) -> (unsigned 32bit integer=w3292:u32)
              }
              frame 8 {
                w3322 = 0.0 ("f")
                # "MCL raster scan"
                n1888 = local read "Number of scans (MCL)"() -> (w3317:u64)
                n1889 = local read "Scan lines (y)"() -> (w3316:u64)
                n1890 = local read "2D or 1D Scan"() -> (w3319:bool)
                n1891 = local read "Scan Range (V)\n(of steps)"() -> (w3338:dbl)
                n1892 = local read "Fast Scan Dir"() -> (w3345:bool)
                n1893 = local read "Cycles/step (MCL)"() -> (w3335:u64)
                n1894 = local read "Scan steps (MCL)"() -> (w3337:u64)
                n1895 = Select(t=w3316, s=w3319, f=w3317) -> (s? t:f=w3318:u64)
                n1896 = Boolean To (0,1)(Boolean=w3319) -> (0, 1=w3321:i16)
                n1897 = local read "Save ave N"() -> (w3350:dbl)
                n1898 = local read "Initial X"() -> (w3324:dbl)
                n1899 = local read "Initial Y"() -> (w3323:dbl)
                n1900 = To Double Precision Float(number=w3321) -> (double precision float=w3320:dbl)
                n1901 = Boolean To (0,1)(Boolean=w3345) -> (0, 1=w3344:i16)
                n1902 = To Double Precision Float(number=w3318) -> (double precision float=w3333:dbl)
                n1903 = To Double Precision Float(number=w3337) -> (double precision float=w3336:dbl)
                n1904 = To Double Precision Float(number=w3335) -> (double precision float=w3334:dbl)
                n1905 = To Double Precision Float(number=w3344) -> (double precision float=w3343:dbl)
                n1906 = Multiply(x=w3350, y=w3329) -> (x*y=w3349:dbl)
                n1907 = To Double Precision Float(number=w3314) -> (double precision float=w3328:dbl)
                n1908 = local read "N sets should be saved (MCL)"() -> (w3331:dbl)
                n1909 = Build Array(w3328, w3320, w3322, w3322, w3322) -> (w3326:dbl[])
                n1910 = Build Array(w3343, w3338, w3336, w3334, w3333, w3324, w3323) -> (w3340:dbl[])
                n1911 = Build Array(w3325, w3329, w3349, w3348, w3347, 3.0 ("t")) -> (w3342:dbl[])
                n1912 = Round Toward +Infinity(x=w3331) -> (ceil(x): smallest int >= x=w3332:dbl)
                n1913 = Build Array (concatenate)(w3342, w3341, w3326, w3340) -> (w3339:dbl[])
                n1914 = To Unsigned Long Integer(number=w3332) -> (unsigned 32bit integer=w3330:u32)
              }
            }
            n1915 = local read "Index"() -> (w3189:dbl)
            n1916 = call "Create new save file.vi"("Insert"="", "Ext"=".dat", "Index In"=w3189) -> ("Path Out"=w3148:path, "Index Out"=w3161:dbl)
            n1917 = local write "Save file name"(w3148) -> ()
            n1918 = local write "Index"(w3161) -> ()
            n1919 = local write "Save index"(w3161) -> ()
            n1920 = Array Size(array=w3172) -> (size(s)=w3173:i32)
            n1921 = Open/Create/Replace File(file path (use dialog)=w3148, operation (0:open)=T23."create", access (0:read/write)=enum16{"read/write", "read-only", "write-only"}."write-only") -> (refnum out=w3186:refnum<file>)  [unwired: 1 in, 4 out]
            n1922 = local write "Saving..."(TRUE ("Saving...")) -> ()
            n1923 = To Double Precision Float(number=w3173) -> (double precision float=w3171:dbl)
            n1924 = String Length(string="Comment (data description)") -> (length=w3169:i32)
            n1925 = To Double Precision Float(number=w3169) -> (double precision float=w3168:dbl)
            n1926 = Deny Access(7:w3186) -> (3:w3185:refnum<file>)  [unwired: 1 in, 2 out]
            n1927 = Build Array (concatenate)(w3171, w3172, w3168) -> (w3170:dbl[])
            n1928 = case "If fluorescence data to be saved" shown="True" w3159 {
              tunnel: w3148 -> [_ w3238]
              tunnel: [refnum<k0> refnum w3218] -> w3160
              frame False {
              }
              frame True {
                w3217 = 0.0
                n1929 = local read "APD Integration Time (s)"() -> (w3223:dbl)
                n1930 = local read "N APD Samp/step"() -> (w3216:dbl)
                n1931 = Path To String(path=w3238) -> (string=w3237:string)
                n1932 = String Length(string=w3237) -> (length=w3236:i32)
                n1933 = Subtract(x=w3236, y=4) -> (x-y=w3234:i32)
                n1934 = String Subset(string=w3237, length (rest)=w3234) -> (substring=w3233:string)  [unwired: 1 out]
                n1935 = Build Array(w3223, w3216, w3217, w3217, w3217, w3217, w3217, w3217) -> (w3220:dbl[])
                n1936 = Concatenate Strings(w3233, "_fl.dat" ("string")) -> (w3231:string)
                n1937 = Array Size(array=w3220) -> (size(s)=w3222:i32)
                n1938 = String To Path(string=w3231) -> (path=w3227:path)
                n1939 = Open/Create/Replace File(file path (use dialog)=w3227, operation (0:open)=T23."create", access (0:read/write)=enum16{"read/write", "read-only", "write-only"}."write-only") -> (refnum out=w3228:refnum<file>)  [unwired: 1 in, 4 out]
                n1940 = Deny Access(7:w3228) -> (3:w3224:refnum<file>)  [unwired: 1 in, 2 out]
                n1941 = To Double Precision Float(number=w3222) -> (double precision float=w3221:dbl)
                n1942 = Build Array (concatenate)(w3221, w3220) -> (w3219:dbl[])
                n1943 = Write to Binary File(file (use dialog)=w3224, data=w3219, 5:FALSE ("prepend array or string size? (T)"), 9:T29."big-endian, network order" ("byte order (0:big-endian, network order)")) -> (refnum out=w3218:refnum<file>)  [unwired: 1 in, 3 out]
              }
            }
            n1944 = case shown="True" w3146 {
              tunnel: w3148 -> [_ w3200]
              tunnel: [refnum<k0> refnum w3199] -> w3147
              frame False {
              }
              frame True {
                w3195 = 0.0 ("element")
                n1945 = Path To String(path=w3200) -> (string=w3214:string)
                n1946 = Build Array(w3195, w3195, w3195, w3195, w3195, w3195, w3195, w3195) -> (w3196:dbl[])
                n1947 = String Length(string=w3214) -> (length=w3213:i32)
                n1948 = Subtract(x=w3213, y=4) -> (x-y=w3211:i32)
                n1949 = Array Size(array=w3196) -> (size(s)=w3198:i32)
                n1950 = String Subset(string=w3214, length (rest)=w3211) -> (substring=w3210:string)  [unwired: 1 out]
                n1951 = To Double Precision Float(number=w3198) -> (double precision float=w3197:dbl)
                n1952 = Concatenate Strings(w3210, "_pos.dat" ("string")) -> (w3208:string)
                n1953 = Build Array (concatenate)(w3197, w3196) -> (w3194:dbl[])
                n1954 = String To Path(string=w3208) -> (path=w3204:path)
                n1955 = Open/Create/Replace File(file path (use dialog)=w3204, operation (0:open)=T23."create", access (0:read/write)=enum16{"read/write", "read-only", "write-only"}."write-only") -> (refnum out=w3205:refnum<file>)  [unwired: 1 in, 4 out]
                n1956 = Deny Access(7:w3205) -> (3:w3201:refnum<file>)  [unwired: 1 in, 2 out]
                n1957 = Write to Binary File(file (use dialog)=w3201, data=w3194, 5:FALSE ("prepend array or string size? (T)"), 9:T29."big-endian, network order" ("byte order (0:big-endian, network order)")) -> (refnum out=w3199:refnum<file>)  [unwired: 1 in, 3 out]
              }
            }
            n1958 = Write to Binary File(file (use dialog)=w3185, data=w3170, 5:w3166, 9:w3164) -> (refnum out=w3167:refnum<file>)  [unwired: 1 in, 3 out]
            n1959 = Write to Binary File(file (use dialog)=w3167, data="Comment (data description)", 5:w3166, 9:w3164) -> (refnum out=w3163:refnum<file>)  [unwired: 1 in, 3 out]
          }
        }
        n1960 = feedback-in #19(w3106) -> ()
        n1961 = feedback-in #20(w3133) -> ()
        n1962 = feedback-in #21(w3105) -> ()
        n1963 = feedback-in #22(w3116) -> ()
        n1964 = feedback-in #23(w3119) -> ()
        n1965 = feedback-in #24(w3132) -> ()
        n1966 = feedback-in #25(w3122) -> ()
      }
      frame #1 {
        n1967 = local read "Saving..."() -> (w3363:bool)
        n1968 = case shown="True" w3363 {
          tunnel: w3367 -> [_ w3377]
          tunnel: w3366 -> [_ w3391]
          tunnel: w3365 -> [_ w3387]
          tunnel: w3364 -> [_ w3386]
          tunnel: w3362 -> [_ w3385]
          tunnel: w3361 -> [_ w3380]
          tunnel: w3360 -> [_ w3379]
          tunnel: w3359 -> [_ w3378]
          tunnel: w3358 -> [_ w3376]
          tunnel: w3357 -> [_ w3374]
          tunnel: w3356 -> [_ w3373]
          tunnel: w3355 -> [_ w3372]
          tunnel: w3354 -> [_ w3371]
          tunnel: w3353 -> [_ w3370]
          tunnel: w3352 -> [_ w3369]
          tunnel: w3351 -> [_ w3368]
          frame False {
          }
          frame True {
            n1969 = Multiply(x=w3377, y=w3376) -> (x*y=→"Time (s)":dbl)
            n1970 = Less Or Equal?(x=w3377, y=w3385) -> (x <= y?=w3389:bool)
            n1971 = Or(x="Stop Saving", y="Abort save 2") -> (x .or. y?=w3381:bool)
            n1972 = Not(x=w3381) -> (.not. x?=w3390:bool)
            n1973 = And(x=w3389, y=w3390) -> (x .and. y?=w3388:bool)
            n1974 = case shown="False" w3388 {
              tunnel: w3391 -> [w3398 w3466]
              tunnel: [0.0 w3469] -> w3384
              tunnel: w3377 -> [_ w3467]
              tunnel: w3385 -> [_ w3468]
              tunnel: w3387 -> [_ w3463]
              tunnel: w3386 -> [_ _]
              tunnel: w3380 -> [w3396 w3456]
              tunnel: w3379 -> [w3395 w3457]
              tunnel: w3378 -> [_ w3455]
              tunnel: w3374 -> [_ w3454]
              tunnel: w3373 -> [_ w3408]
              tunnel: w3372 -> [_ w3447]
              tunnel: w3371 -> [_ w3425]
              tunnel: w3370 -> [w3393 w3406]
              tunnel: w3369 -> [w3394 w3405]
              tunnel: w3368 -> [_ w3402]
              frame False {
                w3392 = FALSE
                n1975 = Close File(refnum=w3398) -> ()  [unwired: 1 in, 2 out]
                n1976 = case shown="True" w3395 {
                  tunnel: w3396 -> [_ w3400]
                  frame False {
                  }
                  frame True {
                    n1977 = Close File(refnum=w3400) -> ()  [unwired: 1 in, 2 out]
                  }
                }
                n1978 = case shown="True" w3393 {
                  tunnel: w3394 -> [_ w3399]
                  frame False {
                  }
                  frame True {
                    n1979 = Close File(refnum=w3399) -> ()  [unwired: 1 in, 2 out]
                  }
                }
                n1980 = local write "Calibrating Trap..."(w3392) -> ()
                n1981 = call <vilib>:"Beep.vi"() -> ()  [unwired: 3 in, 9 out]
                n1982 = local write "Stop Saving"(w3392) -> ()
                n1983 = property on="Raster Scanning..." class="Bool (strict)"("Val(Sgnl)"=w3392) -> ()  [unwired: 2 in, 2 out]
                "Saving..." <- w3392
              }
              frame True {
                n1984 = local read "Calibrating Trap..."() -> (w3458:bool)
                n1985 = case "Write fl. data" shown="True" w3457 {
                  tunnel: w3456 -> [_ w3492]
                  tunnel: w3455 -> [_ w3491]
                  frame False {
                  }
                  frame True {
                    n1986 = Write to Binary File(file (use dialog)=w3492, data=w3491, 5:FALSE ("prepend array or string size? (T)"), 9:T29."big-endian, network order" ("byte order (0:big-endian, network order)")) -> ()  [unwired: 1 in, 4 out]
                  }
                }
                n1987 = Greater?(x="Save ave N", y=1.0) -> (0:w3461:bool)
                n1988 = Not(x=w3458) -> (.not. x?=w3460:bool)
                n1989 = And(x=w3460, y=w3461) -> (x .and. y?=w3403:bool)
                n1990 = case shown="True" w3403 {
                  tunnel: w3402 -> [w3472 w3483]
                  tunnel: [w3472 w3475] -> w3401
                  tunnel: "Save ave N" -> [_ w3476]
                  frame False {
                  }
                  frame True {
                    w3473 = 2 ("dimension size")
                    n1991 = Array Size(array=w3483) -> (size(s)=w3477:i32)
                    n1992 = Divide(x=w3477, y=w3473) -> (x/y=w3481:dbl)
                    n1993 = Reshape Array(w3483, w3481, w3473) -> (w3482:u64[][])
                    n1994 = Transpose 2D Array(2D array=w3482) -> (transposed array=w3480:u64[][])
                    n1995 = for {
                      tunnel: w3480 -> [w3485] mode=indexing
                      tunnel: [w3484] -> w3474 mode=indexing
                      tunnel: w3476 -> [w3486]
                      workers-P: _ -> [_]
                      n1996 = call "downsample 1D array - U64.vi"("Ave N"=w3486, "Array In"=w3485) -> ("Array Out"=w3484:u64[])  [unwired: 1 in]
                    }
                    n1997 = Transpose 2D Array(2D array=w3474) -> (transposed array=w3479:u64[][])
                    n1998 = Divide(x=w3477, y=w3476) -> (x/y=w3478:dbl)
                    n1999 = Reshape Array(w3479, w3478) -> (w3475:u64[])
                  }
                }
                n2000 = case shown="True" w3403 {
                  tunnel: w3463 -> [w3495 w3507]
                  tunnel: [w3495 w3499] -> w3459
                  tunnel: "Save ave N" -> [_ w3500]
                  tunnel: w3454 -> [_ w3498]
                  frame False {
                    # "don't downsample data for trap calibration"
                  }
                  frame True {
                    n2001 = Array Size(array=w3507) -> (size(s)=w3501:i32)
                    n2002 = Array Size(array=w3498) -> (size(s)=w3497:i32)
                    n2003 = Divide(x=w3501, y=w3497) -> (x/y=w3505:dbl)
                    n2004 = Reshape Array(w3507, w3505, w3497) -> (w3506:i16[][])
                    n2005 = Transpose 2D Array(2D array=w3506) -> (transposed array=w3504:i16[][])
                    n2006 = for {
                      tunnel: w3504 -> [w3510] mode=indexing
                      tunnel: [w3509] -> w3496 mode=indexing
                      tunnel: w3500 -> [w3508]
                      workers-P: _ -> [_]
                      n2007 = call "downsample 1D array - I16.vi"("Ave N"=w3508, "Array In"=w3510) -> ("Array Out"=w3509:i16[])  [unwired: 1 out]
                    }
                    n2008 = Transpose 2D Array(2D array=w3496) -> (transposed array=w3503:i16[][])
                    n2009 = Divide(x=w3501, y=w3500) -> (x/y=w3502:dbl)
                    n2010 = Reshape Array(w3503, w3502) -> (w3499:i16[])
                  }
                }
                n2011 = Index Array(array=w3425, index=1) -> (element=w3428:waveform(dbl))
                n2012 = Index Array(array=w3425, index=0) -> (element=w3430:waveform(dbl))
                n2013 = Unbundle By Name(w3428) -> ("Y"=w3432:dbl[])
                n2014 = Unbundle By Name(w3430) -> ("Y"=w3440:dbl[])
                n2015 = case "Write trap pos. data" shown="True" w3406 {
                  tunnel: w3405 -> [_ w3488]
                  tunnel: w3401 -> [_ w3487]
                  frame False {
                  }
                  frame True {
                    n2016 = Write to Binary File(file (use dialog)=w3488, data=w3487, 5:FALSE ("prepend array or string size? (T)"), 9:T29."big-endian, network order" ("byte order (0:big-endian, network order)")) -> ()  [unwired: 1 in, 4 out]
                  }
                }
                n2017 = Write to Binary File(file (use dialog)=w3466, data=w3459, 5:FALSE ("prepend array or string size? (T)"), 9:T29."big-endian, network order" ("byte order (0:big-endian, network order)")) -> ()  [unwired: 1 in, 4 out]
                n2018 = feedback #26(w3432) -> (w3434:dbl[])
                n2019 = Build Array (concatenate)(w3434, w3432) -> (w3433:dbl[])
                n2020 = Select(t=w3432, s=w3408, f=w3433) -> (s? t:f=w3418:dbl[])
                n2021 = feedback-in #26(w3418) -> ()
                n2022 = feedback #27(w3440) -> (w3453:dbl[])
                n2023 = Build Array (concatenate)(w3453, w3440) -> (w3452:dbl[])
                n2024 = Select(t=w3440, s=w3408, f=w3452) -> (s? t:f=w3427:dbl[])
                n2025 = feedback-in #27(w3427) -> ()
                n2026 = Divide(x=w3467, y=w3468) -> (x/y=w3470:dbl)
                n2027 = Multiply(x=w3470, y=100.0) -> (x*y=w3469:dbl)
                n2028 = Build Array(w3427, w3418) -> (→"Saved APD":dbl[][])
                n2029 = Array Size(array=w3427) -> (size(s)=w3445:i32)
                n2030 = Unbundle By Name(w3447) -> ("Y"=w3451:dbl[])
                n2031 = Subtract(x=w3445, y="N pts to average") -> (x-y=w3421:i32)
                n2032 = Multiply(x="N pts to average", y=u16 2) -> (x*y=w3422:u16)
                n2033 = Subtract(x=w3445, y=w3422) -> (x-y=w3420:i32)
                n2034 = feedback #28(w3451) -> (w3450:dbl[])
                n2035 = Build Array (concatenate)(w3450, w3451) -> (w3449:dbl[])
                n2036 = Select(t=w3451, s=w3408, f=w3449) -> (s? t:f=w3448:dbl[])
                "Trap Delta Graph" <- w3448
                n2037 = feedback-in #28(w3448) -> ()
                n2038 = Array Subset(array=w3427, index=w3421, length="N pts to average") -> (w3444:dbl[])
                n2039 = Array Subset(array=w3427, index=w3420, length="N pts to average") -> (w3443:dbl[])
                n2040 = Array Subset(array=w3418, index=w3421, length="N pts to average") -> (w3424:dbl[])
                n2041 = Array Subset(array=w3418, index=w3420, length="N pts to average") -> (w3423:dbl[])
                n2042 = call-poly <vilib>:"Mean.vi"("X"=w3444) -> ("mean"=w3442:dbl)  [unwired: 1 out]
                n2043 = call-poly <vilib>:"Mean.vi"("X"=w3424) -> ("mean"=w3417:dbl)  [unwired: 1 out]
                n2044 = call-poly <vilib>:"Mean.vi"("X"=w3443) -> ("mean"=w3441:dbl)  [unwired: 1 out]
                n2045 = call-poly <vilib>:"Mean.vi"("X"=w3423) -> ("mean"=w3416:dbl)  [unwired: 1 out]
                n2046 = Subtract(x=w3417, y=w3416) -> (x-y=w3407:dbl)
                "Delta Fl. 2" <- w3407
                n2047 = Subtract(x=w3442, y=w3441) -> (x-y=w3439:dbl)
                "Delta Fl. 1" <- w3439
                n2048 = Initialize Array(w3439, 1 ("dimension size")) -> (w3436:dbl[])
                n2049 = Initialize Array(w3407, 1 ("dimension size")) -> (w3413:dbl[])
                n2050 = feedback #29(w3436) -> (w3437:dbl[])
                n2051 = Build Array (concatenate)(w3437, w3436) -> (w3435:dbl[])
                n2052 = feedback #30(w3413) -> (w3414:dbl[])
                n2053 = Build Array (concatenate)(w3414, w3413) -> (w3412:dbl[])
                n2054 = Select(t=w3436, s=w3408, f=w3435) -> (s? t:f=w3411:dbl[])
                n2055 = feedback-in #29(w3411) -> ()
                n2056 = Select(t=w3413, s=w3408, f=w3412) -> (s? t:f=w3410:dbl[])
                n2057 = feedback-in #30(w3410) -> ()
                n2058 = Build Array(w3411, w3410) -> (→"Save APD Deriv":dbl[][])
              }
            }
            "Progress" <- w3384
            "Progress 2" <- w3384
          }
        }
      }
    }
    n2059 = Bundle By Name(cluster=w2128, "Green FB Ch 0"=w2127, "Green FB Ch 1"=w2126) -> (w2106:T48)
    "Green FB Signals (V)" <- w2106
    n2060 = Unbundle By Name(w2106) -> ("Green FB Ch 2"=→"Green FB Plot":dbl)
    n2061 = local read "wait to reset values"() -> (w2198:bool)
    n2062 = Not(x=w2195) -> (.not. x?=w2199:bool)
    n2063 = And(x=w2199, y=w2198) -> (x .and. y?=w2200:bool)
    n2064 = case "Part of MCL raster scanning: returns to initial positions after scan done" shown="True" w2200 {
      tunnel: w2203 -> [w2936 w2943]
      tunnel: [w2936 w2942] -> w2202
      tunnel: w2197 -> [w2935 w2941]
      tunnel: [w2935 w2940] -> w2196
      frame False {
      }
      frame True {
        w2951 = 10.0 ("y")
        w2950 = 32767.0 ("y")
        # "to return scan values\nafter a synchronous \nAOM scan"
        n2065 = local read "AO2"() -> (w2944:dbl)
        n2066 = local read "AO1"() -> (w2945:dbl)
        n2067 = local write "wait to reset values"(FALSE ("wait to reset values")) -> ()
        n2068 = Multiply(x=w2945, y=w2950) -> (x*y=w2947:dbl)
        n2069 = Multiply(x=w2944, y=w2950) -> (x*y=w2949:dbl)
        n2070 = Divide(x=w2947, y=w2951) -> (x/y=w2946:dbl)
        n2071 = Divide(x=w2949, y=w2951) -> (x/y=w2948:dbl)
        n2072 = To Word Integer(number=w2946) -> (16bit integer=w2952:i16)
        n2073 = To Word Integer(number=w2948) -> (16bit integer=w2953:i16)
        n2074 = local read "Total Counts (ticks)"() -> (w2937:u32)
        n2075 = xnode "Read/Write Control"("FPGA VI Reference In"=w2943, "error in"=w2941, "AO1"=w2952, "AO2"=w2953, "MCL count"=w2937) -> ("FPGA VI Reference Out"=w2942:T19, "error out"=w2940:errorcluster)
        n2076 = local read "Scan Range (V)\n(of steps)"() -> (w2938:dbl)
        n2077 = property on="Scan Range (V)\n(of steps)" class="DigNum (strict)"("Val(Sgnl)"=w2938) -> ()  [unwired: 2 in, 2 out]
      }
    }
    n2078 = node-c288() -> ()  [unwired: 2 out]
  }
  n2079 = node-c288(3 ("Processor")) -> (w74:T24)  [unwired: 3 out]
  n2080 = timed-loop "Oscillate AOD (debugging)" {
    tunnel: w24 -> [w3512]
    tunnel: [w3511] -> w36
    timing: w74 -> [_]
    timing-out: [_] -> w73
    stop <- w3511 stop-if-true
    n2081 = node-c288() -> ()  [unwired: 2 out]
    n2082 = event shown="[0] \"Oscillate Set 2\", \"Fish for Tether\": Value Change" {
      selector: _ -> [_ _ _]
      dyn-events: _ -> [_ _ _]
      timeout: _ -> [_ _ _]
      tunnel: w3512 -> [w3519 _ _]
      tunnel: [FALSE ("Stop All") _ w3787] -> w3511
      event "Oscillate Set 2", "Fish for Tether": Value Change {
        n2083 = event-data() -> ()  [unwired: 6 out]
        n2084 = local read "Oscillate Set 2"() -> (w3518:bool)
        n2085 = Or(x=w3518, y="Fish for Tether") -> (x .or. y?=w3516:bool)
        n2086 = case shown="True" w3516 {
          tunnel: w3519 -> [_ w3522]
          tunnel: "Fish for Tether" -> [_ w3521]
          frame False {
          }
          frame True {
            n2087 = case shown="True" w3521 {
              frame False {
              }
              frame True {
                n2088 = local write "Scan axis 2"(TRUE) -> ()
                n2089 = local write "Tether"(FALSE ("Tether")) -> ()
              }
            }
            n2090 = node-c288("Period") -> (w3524:T24)  [unwired: 3 out]
            n2091 = timed-loop "Oscillate AOD" {
              timing: w3524 -> [_]
              timing-out: [_] -> w3523
              tunnel: w3522 -> [w3534]
              tunnel: w3521 -> [w3533]
              i -> [w3536]
              stop <- w3532 stop-if-true
              n2092 = node-c288() -> (w3535:i64)  [unwired: 1 out]
              n2093 = flat-sequence {
                tunnel: w3536 -> [w3562]
                tunnel: w3535 -> [w3561]
                tunnel: w3534 -> [w3545]
                tunnel: w3533 -> [w3547]
                tunnel: [w3547] -> w3531
                tunnel: [w3546] -> w3530
                tunnel: [w3544] -> w3529
                tunnel: [w3541] -> w3527
                tunnel: w3531 -> [w3598]
                tunnel: w3530 -> [w3596]
                tunnel: w3529 -> [w3595]
                tunnel: [w3594] -> w3528
                tunnel: w3527 -> [w3593]
                tunnel: [w3662] -> w3532
                tunnel: w3528 -> [w3660]
                frame #0 {
                  n2094 = Divide(x=w3561, y=i64 1000) -> (x/y=w3556:dbl)
                  n2095 = Multiply(x=w3556, y=w3562) -> (x*y=w3558:dbl)
                  n2096 = Multiply(x="Osc. freq. (Hz)", y=6.283185307179586) -> (x*y=w3559:dbl)
                  n2097 = Multiply(x=w3559, y=w3558) -> (x*y=w3543:dbl)
                  n2098 = local read "BD 1 Frequency 2 (MHz)"() -> (w3540:dbl)
                  n2099 = local read "BD 1 Frequency 1 (MHz)"() -> (w3537:dbl)
                  n2100 = case shown="True" w3547 {
                    tunnel: w3543 -> [w3568 w3575]
                    tunnel: w3540 -> [_ w3585]
                    tunnel: [w3565 w3569] -> w3548
                    tunnel: [FALSE w3578] -> w3544
                    tunnel: [0.0 w3571] -> w3541
                    tunnel: w3537 -> [_ w3570]
                    frame False {
                      n2101 = Sine(x=w3568) -> (sin(x)=w3566:dbl)
                      n2102 = Multiply(x=w3566, y="Osc. amp. (MHz)") -> (x*y=w3565:dbl)
                    }
                    frame True {
                      n2103 = Cosine(x=w3575) -> (cos(x)=w3588:dbl)
                      n2104 = Subtract(x=w3585, y=w3570) -> (x-y=w3584:dbl)
                      n2105 = Decrement(x=w3588) -> (x-1=w3587:dbl)
                      n2106 = Subtract(x=w3584, y="Closest Delta (MHz)") -> (x-y=w3581:dbl)
                      n2107 = Divide(x=w3587, y=2.0) -> (x/y=w3582:dbl)
                      n2108 = Multiply(x=w3582, y=w3581) -> (x*y=w3569:dbl)
                      n2109 = local read "Vec Mean of T1 T2"() -> (w3577:dbl[])
                      n2110 = Greater?(x=w3577, y="Stop F (pN)") -> (0:w3579:bool[])
                      n2111 = Or Array Elements(Boolean array=w3579) -> (logical OR=w3578:bool)
                      n2112 = Divide(x=w3575, y=6.283185307179586) -> (x/y=w3574:dbl)
                      n2113 = Round Toward +Infinity(x=w3574) -> (ceil(x): smallest int >= x=w3571:dbl)
                      "Attempts" <- w3571
                      n2114 = Greater?(x=w3571, y="Attempt Limit") -> (0:w3573:bool)
                      n2115 = case shown="True" w3573 {
                        frame False {
                        }
                        frame True {
                          n2116 = local write "Fish for Tether"(FALSE ("Fish for Tether")) -> ()
                          n2117 = call <vilib>:"Beep.vi"() -> ()  [unwired: 3 in, 9 out]
                          n2118 = local read "Messages"() -> (w3590:string)
                          n2119 = call "Update messages.vi"("Message to add"="Tether fishing timeout." ("Messages"), "Old message string"=w3590) -> ("New message string"=→"Messages":string)
                        }
                      }
                    }
                  }
                  n2120 = local read "Y RF Frequency Limits (MHz)"() -> (w3549:T16)
                  n2121 = local read "X RF Frequency Limits (MHz)"() -> (w3550:T16)
                  n2122 = local read "BD 1 Frequency 3 (MHz)"() -> (w3555:dbl)
                  n2123 = local read "BD 2 Frequency 2 (MHz)"() -> (w3539:dbl)
                  n2124 = Select(t=w3540, s="Scan axis 2", f=w3539) -> (s? t:f=w3551:dbl)
                  n2125 = Add(x=w3548, y=w3551) -> (x+y=w3546:dbl)
                  n2126 = Select(t=w3546, s="Scan axis 2", f=w3540) -> (s? t:f=w3538:dbl)
                  n2127 = Select(t=w3539, s="Scan axis 2", f=w3546) -> (s? t:f=w3553:dbl)
                  n2128 = local read "BD 2 Frequency 3 (MHz)"() -> (w3554:dbl)
                  n2129 = call "set RF board frequency - interlace.vi"("Board 2 Frequency Limits"=w3549, "Board 1 Frequency Limits"=w3550, "FPGA VI Reference In"=w3545, "Board 2 Frequency 3 (MHz)"=w3554, "Board 1 Frequency 3 (MHz)"=w3555, "Board 2 Frequency 2 (MHz)"=w3539, "Board 2 Frequency 1 (MHz)"=w3553, "Board 1 Frequency 2 (MHz)"=w3538, "Board 1 Frequency 1  (MHz)"=w3537) -> ()  [unwired: 1 in, 2 out]
                }
                frame #1 {
                  n2130 = And(x=w3598, y=w3595) -> (x .and. y?=w3597:bool)
                  n2131 = case "Only if were fishing and now formed tether" shown="True" w3597 {
                    tunnel: w3596 -> [w3600 w3612]
                    tunnel: [w3599 w3611] -> w3594
                    tunnel: w3593 -> [_ w3607]
                    frame False {
                      n2132 = local read "Fish for Tether"() -> (w3599:bool)
                      n2133 = case shown="True" w3599 {
                        tunnel: w3600 -> [_ _]
                        frame False {
                        }
                        frame True {
                        }
                      }
                    }
                    frame True {
                      w3611 = FALSE ("Fish for Tether")
                      n2134 = call <vilib>:"Beep.vi"() -> ()  [unwired: 3 in, 9 out]
                      n2135 = Number To Decimal String(number=w3607, width (-)=i16 1) -> (decimal integer string=w3605:string)
                      n2136 = case shown="\"2\", \"3\", \"4\", \"5\", \"6\"" "Then..." {
                        selector: "Then..." -> [_ w3615]
                        tunnel: w3612 -> [w3614 _]
                        frame "1", Default {
                          # "do nothing"
                          n2137 = property on="BD 1 Frequency 1 (MHz)" class="DigNum (strict)"("Val(Sgnl)"=w3614) -> ()  [unwired: 2 in, 2 out]
                        }
                        frame "2", "3", "4", "5", "6" {
                          n2138 = flat-sequence {
                            tunnel: w3615 -> [w3617]
                            frame #0 {
                              n2139 = property on="Trap Delta (MHz)" class="DigNum (strict)"("Val(Sgnl)"="Move to Delta 1 (MHz)") -> ()  [unwired: 2 in, 2 out]
                            }
                            frame #1 {
                              n2140 = case shown="\"5\", \"6\"" w3617 {
                                selector: w3617 -> [w3620 w3630 _]
                                frame "3", "4" {
                                n2141 = flat-sequence {
                                tunnel: w3620 -> [w3621]
                                tunnel: [w3621] -> w3618
                                tunnel: [w3623] -> w3619
                                tunnel: w3618 -> [w3623]
                                tunnel: w3619 -> [w3627]
                                frame #0 {
                                n2142 = property on="Green Laser ON/Interlacing" class="Bool (strict)"("Val(Sgnl)"=TRUE ("Value (Signaling)")) -> ()  [unwired: 2 in, 2 out]
                                }
                                frame #1 {
                                n2143 = Multiply(x="Wait Before Save (s)", y=u32 1000 ("x")) -> (x*y=w3625:u32)
                                n2144 = Wait (ms)(milliseconds to wait=w3625) -> ()  [unwired: 1 out]
                                }
                                frame #2 {
                                n2145 = property on="Start Saving" class="Bool (strict)"("Value"=TRUE ("Start Saving")) -> ()  [unwired: 2 in, 2 out]
                                n2146 = case shown="Default" w3627 {
                                frame Default {
                                }
                                frame "4" {
                                n2147 = property on="Fl. Triggered..." class="Bool (strict)"("Val(Sgnl)"=TRUE ("Value (Signaling)")) -> ()  [unwired: 2 in, 2 out]
                                }
                                }
                                }
                                }
                                }
                                frame "5", "6" {
                                n2148 = stacked-sequence {
                                tunnel: w3630 -> [_ _ _ _ _ _ _ _ w3647 _ _]
                                frame #0 {
                                n2149 = Replace Array Subset(array=u32[] [0] ("Index Values"), new element="Raster Set Upon Tether", index=0) -> (w3631:u32[])
                                n2150 = property on="Saved AOD Raster Scan Parameter Sets" class="Arr (strict)"("Index Values"=w3631) -> ()  [unwired: 2 in, 2 out]
                                }
                                frame #1 {
                                n2151 = Wait (ms)(milliseconds to wait=u32 500) -> ()  [unwired: 1 out]
                                }
                                frame #2 {
                                n2152 = property on="Load parameters" class="Bool (strict)"("Val(Sgnl)"=TRUE ("Value (Signaling)")) -> ()  [unwired: 2 in, 2 out]
                                }
                                frame #3 {
                                n2153 = Wait (ms)(milliseconds to wait=u32 500) -> ()  [unwired: 1 out]
                                }
                                frame #4 {
                                n2154 = property on="Trap Raster Scan" class="Bool (strict)"("Val(Sgnl)"=TRUE ("Value (Signaling)")) -> ()  [unwired: 2 in, 2 out]
                                }
                                frame #5 {
                                n2155 = Wait (ms)(milliseconds to wait=u32 2000) -> ()  [unwired: 1 out]
                                }
                                frame #6 {
                                n2156 = while {
                                stop <- w3642 stop-if-true
                                n2157 = local read "Raster Scanning..."() -> (w3641:bool)
                                n2158 = local read "Saving..."() -> (w3644:bool)
                                n2159 = Wait (ms)(milliseconds to wait=u32 100) -> ()  [unwired: 1 out]
                                n2160 = Not(x=w3644) -> (.not. x?=w3643:bool)
                                n2161 = Not(x=w3641) -> (.not. x?=w3640:bool)
                                n2162 = And(x=w3643, y=w3640) -> (x .and. y?=w3642:bool)
                                }
                                }
                                frame #7 {
                                n2163 = property on="Trap Delta (MHz)" class="DigNum (strict)"("Val(Sgnl)"="Move to Delta 2 (MHz)") -> ()  [unwired: 2 in, 2 out]
                                }
                                frame #8 {
                                n2164 = local read "Tether"() -> (w3648:bool)
                                n2165 = case shown="True" w3648 {
                                tunnel: w3647 -> [_ w3649]
                                frame False {
                                }
                                frame True {
                                n2166 = flat-sequence {
                                tunnel: w3649 -> [w3651]
                                frame #0 {
                                n2167 = Wait (ms)(milliseconds to wait=u32 500) -> ()  [unwired: 1 out]
                                }
                                frame #1 {
                                n2168 = case shown="\"6\"" w3651 {
                                frame Default {
                                }
                                frame "6" {
                                n2169 = property on="Green Laser ON/Interlacing" class="Bool (strict)"("Val(Sgnl)"=TRUE ("Green Laser ON/Interlacing")) -> ()  [unwired: 2 in, 2 out]
                                }
                                }
                                }
                                frame #2 {
                                n2170 = Wait (ms)(milliseconds to wait=u32 500) -> ()  [unwired: 1 out]
                                }
                                frame #3 {
                                n2171 = local write "Start Saving"("Save at end (5, 6)") -> ()
                                }
                                }
                                }
                                }
                                }
                                frame #9 {
                                n2172 = local read "Bead Sep. Int. Time (s)"() -> (w3657:dbl)
                                n2173 = Multiply(x=w3657, y=1000.0) -> (x*y=w3656:dbl)
                                n2174 = Wait (ms)(milliseconds to wait=w3656) -> ()  [unwired: 1 out]
                                }
                                frame #10 {
                                n2175 = property on="Rescale on Mean" class="Bool (strict)"("Val(Sgnl)"=TRUE ("Value (Signaling)")) -> ()  [unwired: 2 in, 2 out]
                                }
                                }
                                }
                                frame "2", Default {
                                }
                              }
                            }
                          }
                        }
                      }
                      n2176 = Concatenate Strings("Formed tether in ", w3605, " attempt(s)." ("string")) -> (w3602:string)
                      n2177 = local read "Messages"() -> (w3609:string)
                      n2178 = local write "Fish for Tether"(w3611) -> ()
                      n2179 = call "Update messages.vi"("Message to add"=w3602, "Old message string"=w3609) -> ("New message string"=w3608:string)
                      n2180 = local write "Messages"(w3608) -> ()
                      n2181 = Get Date/Time In Seconds() -> (seconds since 1Jan1904=→"Time tether formed":timestamp)
                      "Tether" <- "Tether Alarm?"
                    }
                  }
                }
                frame #2 {
                  n2182 = local read "Oscillate Set 2"() -> (w3661:bool)
                  n2183 = local read "Stop All"() -> (w3663:bool)
                  n2184 = Not Or(1:w3660, 2:w3661) -> (0:w3659:bool)
                  n2185 = Compound Arithmetic op=OR(w3663, w3659) -> (w3662:bool)
                }
              }
              n2186 = node-c288() -> ()  [unwired: 2 out]
            }
            n2187 = node-c288(w3523) -> ()  [unwired: 1 out]
          }
        }
      }
      event "Fl. Triggered...": Value Change {
        n2188 = event-data() -> ()  [unwired: 7 out]
        n2189 = case shown="True" "Fl. Triggered..." {
          frame False {
          }
          frame True {
            n2190 = node-c288() -> (w3675:T24)  [unwired: 4 out]
            n2191 = timed-loop {
              timing: w3675 -> [_]
              timing-out: [_] -> w3674
              tunnel: "Action" -> [w3679]
              shift-right: [w3676] -> _
              shift-left: u8 255 -> [w3678]
              stop <- w3680 stop-if-true
              n2192 = node-c288() -> ()  [unwired: 2 out]
              n2193 = flat-sequence {
                tunnel: w3679 -> [w3692]
                tunnel: w3678 -> [w3689]
                tunnel: [w3688] -> w3677
                tunnel: [w3778] -> w3680
                tunnel: w3677 -> [w3777]
                tunnel: [w3777] -> w3676
                frame #0 {
                  n2194 = local read "Delta Fl. 2"() -> (w3683:dbl)
                  n2195 = local read "Delta Fl. 1"() -> (w3684:dbl)
                  n2196 = Select(t=w3684, s="APD to Watch", f=w3683) -> (s? t:f=w3682:dbl)
                  n2197 = Multiply(x="Fl. Delta Thresh. (kHz)", y=1000.0) -> (x*y=w3691:dbl)
                  n2198 = Greater?(x=w3682, y=w3691) -> (0:w3686:bool)
                  n2199 = Or(x="Force Yank", y=w3686) -> (x .or. y?=w3687:bool)
                  n2200 = case shown="True" w3687 {
                    tunnel: w3692 -> [_ w3702]
                    tunnel: w3689 -> [w3694 w3698]
                    tunnel: [w3694 w3695] -> w3688
                    frame False {
                    }
                    frame True {
                      n2201 = flat-sequence {
                        tunnel: w3699 -> [w3708]
                        tunnel: [w3708] -> w3703
                        tunnel: w3702 -> [w3707]
                        tunnel: [w3707] -> w3701
                        tunnel: [w3706] -> w3700
                        tunnel: w3698 -> [w3705]
                        tunnel: [w3704] -> w3697
                        tunnel: w3703 -> [w3733]
                        tunnel: w3701 -> [w3732]
                        tunnel: w3700 -> [w3731]
                        tunnel: w3697 -> [w3730]
                        tunnel: [w3730] -> w3696
                        tunnel: w3696 -> [w3775]
                        tunnel: [w3775] -> w3695
                        frame #0 {
                          n2202 = call <vilib>:"Beep.vi"() -> ()  [unwired: 3 in, 9 out]
                          n2203 = local write "Waiting"(FALSE ("Waiting")) -> ()
                          n2204 = Increment(x=w3705) -> (x+1=w3704:u8)
                          n2205 = case shown="\"Yank\"" w3707 {
                            tunnel: w3704 -> [_ _ w3714]
                            frame "Image" {
                              n2206 = property on="Confocal Image" class="Bool (strict)"("Val(Sgnl)"=TRUE ("Value (Signaling)")) -> ()  [unwired: 2 in, 2 out]
                            }
                            frame "Alarm", Default {
                            }
                            frame "Yank" {
                              n2207 = flat-sequence {
                                tunnel: w3714 -> [w3717]
                                tunnel: [w3716] -> w3713
                                tunnel: ["N Array El"] -> w3712
                                tunnel: w3713 -> [w3727]
                                tunnel: w3712 -> [w3723]
                                frame #0 {
                                n2208 = Multiply(x="Yank Delay (s)", y=1000.0) -> (x*y=w3720:dbl)
                                n2209 = Quotient & Remainder(x=w3717, y="N Array El") -> (x-y*floor(x/y)=w3716:u8)  [unwired: 1 out]
                                n2210 = Wait (ms)(milliseconds to wait=w3720) -> ()  [unwired: 1 out]
                                }
                                frame #1 {
                                n2211 = Random Number (0-1)() -> (number: 0 to 1=w3724:dbl)
                                n2212 = Multiply(x=w3723, y=w3724) -> (x*y=w3722:dbl)
                                n2213 = Round Toward -Infinity(1:w3722) -> (0:w3721:dbl)
                                n2214 = Select(t=w3721, s="Random Choice", f=w3727) -> (s? t:f=w3725:dbl)
                                n2215 = Index Array(array="Yank to Delta Array (MHz)", index=w3725) -> (element=w3728:dbl)
                                n2216 = property on="Trap Delta (MHz)" class="DigNum (strict)"("Val(Sgnl)"=w3728) -> ()  [unwired: 2 in, 2 out]
                                }
                              }
                            }
                          }
                          n2217 = local read "Time (s)"() -> (w3706:dbl)
                          "Fl. High" <- TRUE ("Yanking")
                        }
                        frame #1 {
                          n2218 = node-c288() -> (w3735:T24)  [unwired: 4 out]
                          n2219 = timed-loop {
                            timing: w3735 -> [_]
                            timing-out: [_] -> w3734
                            tunnel: w3733 -> [w3751]
                            tunnel: w3732 -> [w3749]
                            tunnel: w3731 -> [w3748]
                            stop <- w3750 stop-if-true
                            n2220 = node-c288() -> ()  [unwired: 2 out]
                            n2221 = local read "Fl. Delta Thresh. (kHz)"() -> (w3743:dbl)
                            n2222 = local read "Fl. Triggered..."() -> (w3752:bool)
                            n2223 = local read "Delta Fl. 1"() -> (w3739:dbl)
                            n2224 = local read "Delta Fl. 2"() -> (w3737:dbl)
                            n2225 = local read "Stop All"() -> (w3746:bool)
                            n2226 = local read "APD to Watch"() -> (w3738:bool)
                            n2227 = Select(t=w3739, s=w3738, f=w3737) -> (s? t:f=w3736:dbl)
                            n2228 = Not(x=w3752) -> (.not. x?=w3747:bool)
                            n2229 = Multiply(x=w3743, y=1000.0) -> (x*y=w3742:dbl)
                            n2230 = Negate(x=w3742) -> (-x=w3741:dbl)
                            n2231 = Less?(x=w3736, y=w3741) -> (x < y?=w3745:bool)
                            n2232 = Compound Arithmetic op=OR(w3745, w3746, w3747, "Force Reset") -> (w3750:bool)
                            n2233 = case shown="True" w3750 {
                              tunnel: w3751 -> [_ w3763]
                              tunnel: w3749 -> [_ w3762]
                              tunnel: w3748 -> [_ w3760]
                              frame False {
                              }
                              frame True {
                                n2234 = case shown="\"Yank\"" w3762 {
                                tunnel: w3763 -> [_ w3764]
                                frame "Image", Default {
                                }
                                frame "Yank" {
                                n2235 = flat-sequence {
                                tunnel: [w3769] -> w3765
                                tunnel: w3764 -> [w3769]
                                tunnel: w3765 -> [w3770]
                                frame #0 {
                                n2236 = local read "Yank Delay (s)"() -> (w3768:dbl)
                                n2237 = Multiply(x=w3768, y=1000.0) -> (x*y=w3766:dbl)
                                n2238 = Wait (ms)(milliseconds to wait=w3766) -> ()  [unwired: 1 out]
                                }
                                frame #1 {
                                n2239 = property on="Trap Delta (MHz)" class="DigNum (strict)"("Val(Sgnl)"=w3770) -> ()  [unwired: 2 in, 2 out]
                                }
                                }
                                }
                                }
                                n2240 = local read "Time (s)"() -> (w3761:dbl)
                                n2241 = Subtract(x=w3761, y=w3760) -> (x-y=w3757:dbl)
                                "Duration (s)" <- w3757
                                n2242 = Number To Decimal String(number=w3757, width (-)=i16 0) -> (decimal integer string=w3755:string)
                                n2243 = Concatenate Strings(w3755, " s fluorescence event." ("string")) -> (w3753:string)
                                n2244 = local read "Messages"() -> (w3759:string)
                                n2245 = call "Update messages.vi"("Message to add"=w3753, "Old message string"=w3759) -> ("New message string"=w3758:string)
                                n2246 = call <vilib>:"Beep.vi"() -> ()  [unwired: 3 in, 9 out]
                                n2247 = local write "Messages"(w3758) -> ()
                              }
                            }
                            n2248 = node-c288() -> ()  [unwired: 2 out]
                          }
                          n2249 = node-c288(w3734) -> ()  [unwired: 1 out]
                        }
                        frame #2 {
                          n2250 = local write "Fl. High"(FALSE ("Yanking")) -> ()
                        }
                      }
                      n2251 = local read "Trap Delta (MHz)"() -> (w3699:dbl)
                    }
                  }
                }
                frame #1 {
                  n2252 = local read "Stop All"() -> (w3781:bool)
                  n2253 = local read "Fl. Triggered..."() -> (w3779:bool)
                  n2254 = Not(x=w3779) -> (.not. x?=w3780:bool)
                  n2255 = Or(x=w3780, y=w3781) -> (x .or. y?=w3778:bool)
                  n2256 = Not(x=w3778) -> (.not. x?=→"Waiting":bool)
                }
              }
              n2257 = node-c288() -> ()  [unwired: 2 out]
            }
            n2258 = node-c288(w3674) -> ()  [unwired: 1 out]
          }
        }
      }
      event "Stop All": Value Change {
        n2259 = event-data() -> ()  [unwired: 7 out]
        n2260 = local read "Stop All"() -> (w3787:bool)
      }
    }
    n2261 = node-c288() -> ()  [unwired: 2 out]
  }
  n2262 = node-c288(w14) -> ()  [unwired: 1 out]
  n2263 = node-c288(w68) -> ()  [unwired: 1 out]
  n2264 = node-c288(w75) -> ()  [unwired: 1 out]
  n2265 = node-c288(w73) -> ()  [unwired: 1 out]
  n2266 = node-c288(w163) -> ()  [unwired: 1 out]
  n2267 = flat-sequence {
    tunnel: w33 -> [w3792]
    tunnel: [w3791] -> w39
    tunnel: [w3788] -> w38
    tunnel: w37 -> [_]
    tunnel: w36 -> [_]
    tunnel: w35 -> [_]
    tunnel: w34 -> [_]
    tunnel: w32 -> [w3789]
    tunnel: w39 -> [w3795]
    tunnel: w38 -> [w3794]
    frame #0 {
      w3790 = FALSE ("APD to FIFO")
      n2268 = xnode "Read/Write Control"("FPGA VI Reference In"=w3792, "error in"=w3789, "APD to FIFO"=w3790, "AI to FIFO"=w3790) -> ("FPGA VI Reference Out"=w3791:T19, "error out"=w3788:errorcluster)
    }
    frame #1 {
      n2269 = xnode "Invoke Method"("FPGA VI Reference In"=w3795, "error in"=w3794) -> ("FPGA VI Reference Out"=w3793:T19)  [unwired: 1 out]
      n2270 = xnode "Close FPGA VI Reference"("FPGA VI Reference In"=w3793) -> ()  [unwired: 1 in, 1 out]
    }
  }
